vi "Query_source_settings_menu.vi"(8 "error in (no error)":errorcluster) -> (0 "error out":errorcluster, 1 "Cancelled?":bool, 3 "Output cluster":T1={"Integer Timestamp"=0, "Einzel Voltage"=0.0, "Needle Voltage"=0.0, "Frequency"=1.0, "Width (ms) : 0.1 "=0.05, "Desired Amplitude (V)"=0.0, "X Voltage"=0.0, "Y Voltage"=0.0, "Settings ID"="", "ID#"=0} {"Needle Voltage" min=0.0 max=10.0 step=0.01 format="%.2g"; "Y Voltage" min=0.0 max=9.0 step=0.01 format="%.2g"; "X Voltage" min=0.0 max=9.0 step=0.01 format="%.2g"; "Einzel Voltage" min=0.0 max=10.0 step=0.01 format="%.2g"; "Desired Amplitude (V)" min=0.0 max=10.0 step=0.01 format="%5.2f"; "Width (ms) : 0.1" min=0.05 max=5.0 step=0.01 format="%6.2f"; "Frequency" min=1.0 max=100.0 step=0.01 format="%.1f"})   [LabVIEW 2015]
doc: "Displays a standard dialog box that prompts users to enter information, such as a user name and password.\n--------------------\n\nThis Express VI is configured as follows:\n\nMessage to Display to the User:\nThe inputs are: \nNumber: Upper Timestamp Range\nNumber: Lower Timestamp Range\nNumber: Settings ID"
uses:
  Controls/dust_source_control.ctl
  Controls/Source_settings_select.ctl
  <vilib>/Utility/miscctls.llb/LVPointTypeDef.ctl
  <userlib>/_OpenG.lib/array/array.llb/Conditional Auto-Indexing Tunnel (I32)__ogtk.vi
  <vilib>/addons/database/_DB Variant To Data/Database Variant To Data.xnode
panel:
  out "Shooting Freq":dbl
  in  "Last Run Start":bool
  out "Source Control Array":T1[](array[typedef]) {"Needle Voltage" min=0.0 max=10.0 step=0.01 format="%.2g"; "Y Voltage" min=0.0 max=9.0 step=0.01 format="%.2g"; "X Voltage" min=0.0 max=9.0 step=0.01 format="%.2g"; "Einzel Voltage" min=0.0 max=10.0 step=0.01 format="%.2g"; "Desired Amplitude (V)" min=0.0 max=10.0 step=0.01 format="%5.2f"; "Width (ms) : 0.1" min=0.05 max=5.0 step=0.01 format="%6.2f"; "Frequency" min=1.0 max=100.0 step=0.01 format="%.1f"}
  in  "Settings Type":T2
  in  "Clear Filter":bool
  in  "Tag Filter":T3
  in  "Load Settings":bool caption="OK2"
  in  "Cancel":bool
  in  "Settings ID":i32(ring) items=["Automatic Update (DT: Iron-1E+1-3; HV: 2.2; Time: 7/23/2019 9:58:43 AM)"=11777, "Automatic Update (DT: Iron-1E+1-3; HV: 2.2; Time: 7/23/2019 10:03:43 AM)"=11778, "Automatic Update (DT: Iron-1E+1-3; HV: 2.2; Time: 7/23/2019 10:08:43 AM)"=11779, "Automatic Update (DT: Iron-1E+1-3; HV: 2.2; Time: 7/23/2019 10:18:43 AM)"=11780, "Automatic Update (DT: Iron-1E+1-3; HV: 2.2; Time: 7/23/2019 10:28:43 AM)"=11781, "Automatic Update (DT: Iron-1E+1-3; HV: 2.2; Time: 7/23/2019 10:48:43 AM)"=11782, "Automatic Update (DT: Iron-1E+1-3; HV: 2.2; Time: 7/23/2019 2:54:37 PM)"=11783, "Automatic Update (DT: Iron-1E+1-3; HV: 2.2; Time: 7/23/2019 3:03:12 PM)"=11784, "Automatic Update (DT: Iron-1E+1-3; HV: 2.2; Time: 7/23/2019 3:08:12 PM)"=11785, "Automatic Update (DT: Iron-1E+1-3; HV: 2.2; Time: 7/23/2019 3:13:12 PM)"=11786, "Automatic Update (DT: Iron-1E+1-3; HV: 2.2; Time: 7/23/2019 3:18:12 PM)"=11787, "Automatic Update (DT: Iron-1E+1-3; HV: 2.2; Time: 7/23/2019 3:23:13 PM)"=11788, "Automatic Update (DT: Iron-1E+1-3; HV: 2.2; Time: 7/23/2019 3:38:13 PM)"=11789, "Automatic Update (DT: Iron-1E+1-3; HV: 2.2; Time: 7/23/2019 3:53:13 PM)"=11790, "Automatic Update (DT: Iron-1E+1-3; HV: 2.2; Time: 7/23/2019 3:58:13 PM)"=11791, "Automatic Update (DT: Iron-1E+1-3; HV: 2.2; Time: 7/23/2019 4:03:13 PM)"=11792, "Automatic Update (DT: Iron-1E+1-3; HV: 2.2; Time: 7/23/2019 4:43:13 PM)"=11793, "Automatic Update (DT: Iron-1E+1-3; HV: 2.2; Time: 7/23/2019 4:58:13 PM)"=11794, "Automatic Update (DT: Iron-1E+1-3; HV: 2.2; Time: 7/24/2019 3:57:41 PM)"=11795, "Automatic Update (DT: Iron-1E+1-3; HV: 2.2; Time: 7/24/2019 4:02:41 PM)"=11796, "Automatic Update (DT: Iron-1E+1-3; HV: 2.2; Time: 7/24/2019 4:07:41 PM)"=11797, "Automatic Update (DT: Iron-1E+1-3; HV: 2.2; Time: 7/24/2019 4:12:41 PM)"=11798, "Automatic Update (DT: Iron-1E+1-3; HV: 2.2; Time: 7/24/2019 4:17:41 PM)"=11799, "Automatic Update (DT: Iron-1E+1-3; HV: 2.2; Time: 7/24/2019 4:22:41 PM)"=11800, "Automatic Update (DT: Iron-1E+1-3; HV: 2.2; Time: 7/24/2019 4:32:41 PM)"=11801, "Automatic Update (DT: Iron-1E+1-3; HV: 2.2; Time: 7/25/2019 8:48:47 AM)"=11802, "Automatic Update (DT: Iron-1E+1-3; HV: 2.2; Time: 7/25/2019 8:53:47 AM)"=11803, "Automatic Update (DT: Iron-1E+1-3; HV: 2.2; Time: 7/25/2019 9:13:47 AM)"=11804, "Automatic Update (DT: Iron-1E+1-3; HV: 2.2; Time: 7/25/2019 9:18:47 AM)"=11805, "Automatic Update (DT: Iron-1E+1-3; HV: 2.2; Time: 7/25/2019 9:23:47 AM)"=11806, "Automatic Update (DT: Iron-1E+1-3; HV: 2.2; Time: 7/25/2019 9:28:48 AM)"=11807, "Automatic Update (DT: Iron-1E+1-3; HV: 2.2; Time: 7/25/2019 9:38:48 AM)"=11808, "Automatic Update (DT: Iron-1E+1-3; HV: 2.2; Time: 7/25/2019 9:43:48 AM)"=11809, "Automatic Update (DT: Iron-1E+1-3; HV: 2.2; Time: 7/25/2019 9:48:48 AM)"=11810, "Automatic Update (DT: Iron-1E+1-3; HV: 2.2; Time: 7/25/2019 9:53:48 AM)"=11811, "Automatic Update (DT: Iron-1E+1-3; HV: 2.2; Time: 7/25/2019 9:58:48 AM)"=11812, "Automatic Update (DT: Iron-1E+1-3; HV: 2.2; Time: 7/25/2019 10:03:48 AM)"=11813, "Automatic Update (DT: Iron-1E+1-3; HV: 2.2; Time: 7/25/2019 10:13:48 AM)"=11814, "Automatic Update (DT: Iron-1E+1-3; HV: 2.2; Time: 7/25/2019 10:23:48 AM)"=11815, "Automatic Update (DT: Iron-1E+1-3; HV: 2.2; Time: 7/25/2019 10:28:48 AM)"=11816, "Automatic Update (DT: Iron-1E+1-3; HV: 2.2; Time: 7/25/2019 10:33:48 AM)"=11817, "Automatic Update (DT: Iron-1E+1-3; HV: 2.2; Time: 7/25/2019 10:43:49 AM)"=11818, "Automatic Update (DT: Iron-1E+1-3; HV: 2.2; Time: 7/25/2019 10:48:49 AM)"=11819, "Automatic Update (DT: Iron-1E+1-3; HV: 2.2; Time: 7/25/2019 10:53:49 AM)"=11820, "Automatic Update (DT: Iron-1E+1-3; HV: 2.2; Time: 7/25/2019 11:03:49 AM)"=11821, "Automatic Update (DT: Iron-1E+1-3; HV: 2.2; Time: 7/25/2019 11:08:49 AM)"=11822, "Automatic Update (DT: Iron-1E+1-3; HV: 2.2; Time: 8/8/2019 12:53:48 PM)"=11823, "Automatic Update (DT: Iron-1E+1-3; HV: 2.2; Time: 8/8/2019 1:08:48 PM)"=11824, "Automatic Update (DT: Iron-1E+1-3; HV: 2.2; Time: 8/21/2019 10:56:07 AM)"=11825, "Automatic Update (DT: Iron-1E+1-3; HV: 2.2; Time: 8/21/2019 11:01:07 AM)"=11826, "Automatic Update (DT: Iron-1E+1-3; HV: 2.2; Time: 8/21/2019 11:11:11 AM)"=11827, "Automatic Update (DT: Iron-1E+1-3; HV: 2.2; Time: 8/21/2019 11:16:11 AM)"=11828, "Automatic Update (DT: Iron-1E+1-3; HV: 2.2; Time: 8/21/2019 11:26:12 AM)"=11829, "Automatic Update (DT: Iron-1E+1-3; HV: 2.2; Time: 8/21/2019 11:31:12 AM)"=11830, "Automatic Update (DT: Iron-1E+1-3; HV: 2.2; Time: 8/21/2019 11:36:14 AM)"=11831, "Automatic Update (DT: Iron-1E+1-3; HV: 2.2; Time: 8/21/2019 11:41:22 AM)"=11832, "Automatic Update (DT: Iron-1E+1-3; HV: 2.2; Time: 8/21/2019 11:46:23 AM)"=11833, "Automatic Update (DT: Iron-1E+1-3; HV: 2.2; Time: 8/21/2019 12:47:37 PM)"=11834, "Automatic Update (DT: Iron-1E+1-3; HV: 2.2; Time: 8/21/2019 12:52:37 PM)"=11835, "Automatic Update (DT: Iron-1E+1-3; HV: 2.2; Time: 8/21/2019 12:57:37 PM)"=11836, "Automatic Update (DT: Iron-1E+1-3; HV: 2.2; Time: 8/21/2019 1:02:37 PM)"=11837, "Automatic Update (DT: Iron-1E+1-3; HV: 2.2; Time: 8/21/2019 1:07:37 PM)"=11838, "Automatic Update (DT: Iron-1E+1-3; HV: 2.2; Time: 8/21/2019 1:12:37 PM)"=11839, "Automatic Update (DT: Iron-1E+1-3; HV: 2.2; Time: 8/21/2019 1:17:38 PM)"=11840, "Automatic Update (DT: Iron-1E+1-3; HV: 2.2; Time: 8/21/2019 1:22:38 PM)"=11841, "Automatic Update (DT: Iron-1E+1-3; HV: 2.2; Time: 8/21/2019 1:32:38 PM)"=11842, "Automatic Update (DT: Iron-1E+1-3; HV: 2.2; Time: 8/21/2019 1:37:38 PM)"=11843, "Automatic Update (DT: Iron-1E+1-3; HV: 2.2; Time: 8/21/2019 1:42:38 PM)"=11844, "Automatic Update (DT: Iron-1E+1-3; HV: 2.2; Time: 8/21/2019 1:47:38 PM)"=11845, "Automatic Update (DT: Aluminum-4-2; HV: 2.2; Time: 9/3/2019 3:06:52 PM)"=11846, "Automatic Update (DT: Aluminum-4-2; HV: 2.2; Time: 9/3/2019 3:11:52 PM)"=11847, "Automatic Update (DT: Aluminum-4-2; HV: 2.2; Time: 9/3/2019 3:16:52 PM)"=11848, "Automatic Update (DT: Aluminum-4-2; HV: 2.2; Time: 9/9/2019 11:23:47 AM)"=11849, "Automatic Update (DT: Aluminum-4-2; HV: 2.2; Time: 9/9/2019 11:28:49 AM)"=11850, "Automatic Update (DT: Aluminum-4-2; HV: 2.2; Time: 9/9/2019 11:33:49 AM)"=11851, "Automatic Update (DT: Aluminum-4-2; HV: 2.2; Time: 9/9/2019 11:43:49 AM)"=11852, "Automatic Update (DT: Aluminum-4-2; HV: 2.2; Time: 9/9/2019 11:48:49 AM)"=11853, "Automatic Update (DT: Aluminum-4-2; HV: 2.2; Time: 9/9/2019 11:58:49 AM)"=11854, "Automatic Update (DT: Aluminum-4-2; HV: 2.2; Time: 9/9/2019 12:03:50 PM)"=11855, "Automatic Update (DT: Aluminum-4-2; HV: 2.2; Time: 9/9/2019 12:08:50 PM)"=11856, "Automatic Update (DT: Aluminum-4-2; HV: 2.2; Time: 9/9/2019 12:18:50 PM)"=11857, "Automatic Update (DT: Aluminum-4-2; HV: 2.2; Time: 9/9/2019 12:28:50 PM)"=11858, "Automatic Update (DT: Aluminum-4-2; HV: 2.2; Time: 9/9/2019 12:48:50 PM)"=11859, "Automatic Update (DT: Aluminum-4-2; HV: 2.2; Time: 9/9/2019 12:53:50 PM)"=11860, "Automatic Update (DT: Aluminum-4-2; HV: 2.2; Time: 9/9/2019 12:58:51 PM)"=11861, "Automatic Update (DT: Aluminum-4-2; HV: 2.2; Time: 9/9/2019 1:03:51 PM)"=11862, "Automatic Update (DT: Aluminum-4-2; HV: 2.2; Time: 9/9/2019 1:08:57 PM)"=11863, "Automatic Update (DT: Aluminum-4-2; HV: 2.2; Time: 9/9/2019 1:13:57 PM)"=11864, "Automatic Update (DT: Aluminum-4-2; HV: 2.2; Time: 9/9/2019 1:18:58 PM)"=11865, "Automatic Update (DT: Aluminum-4-2; HV: 2.2; Time: 9/9/2019 1:28:58 PM)"=11866, "Automatic Update (DT: Aluminum-4-2; HV: 2.2; Time: 9/9/2019 1:33:58 PM)"=11867, "Automatic Update (DT: Aluminum-4-2; HV: 2.2; Time: 9/13/2019 8:25:20 AM)"=11868, "Automatic Update (DT: Aluminum-4-2; HV: 2.2; Time: 9/13/2019 8:30:20 AM)"=11869, "Automatic Update (DT: Aluminum-4-2; HV: 2.2; Time: 9/13/2019 8:40:20 AM)"=11870, "Automatic Update (DT: Aluminum-4-2; HV: 2.2; Time: 9/13/2019 8:45:20 AM)"=11871, "Automatic Update (DT: Aluminum-4-2; HV: 2.2; Time: 9/13/2019 8:50:21 AM)"=11872, "Automatic Update (DT: Aluminum-4-2; HV: 2.2; Time: 9/13/2019 9:05:21 AM)"=11873, "Automatic Update (DT: Aluminum-4-2; HV: 2.2; Time: 9/13/2019 9:10:21 AM)"=11874, "Automatic Update (DT: Aluminum-4-2; HV: 2.2; Time: 9/13/2019 10:00:21 AM)"=11875, "Automatic Update (DT: Aluminum-4-2; HV: 2.2; Time: 9/13/2019 10:05:21 AM)"=11876, "Automatic Update (DT: Aluminum-4-2; HV: 2.2; Time: 9/13/2019 10:10:21 AM)"=11877, "Automatic Update (DT: Aluminum-4-2; HV: 2.2; Time: 9/13/2019 10:15:22 AM)"=11878, "Automatic Update (DT: Aluminum-4-2; HV: 2.2; Time: 9/13/2019 10:20:22 AM)"=11879, "Automatic Update (DT: Aluminum-4-2; HV: 2.2; Time: 9/13/2019 10:25:22 AM)"=11880, "Automatic Update (DT: Aluminum-4-2; HV: 2.2; Time: 9/13/2019 10:30:22 AM)"=11881, "Automatic Update (DT: Aluminum-4-2; HV: 2.2; Time: 9/13/2019 10:45:22 AM)"=11882, "Automatic Update (DT: Aluminum-4-2; HV: 2.2; Time: 9/13/2019 10:50:22 AM)"=11883, "Automatic Update (DT: Aluminum-4-2; HV: 2.2; Time: 9/13/2019 11:05:23 AM)"=11884, "Automatic Update (DT: Aluminum-4-2; HV: 2.2; Time: 9/13/2019 11:10:23 AM)"=11885, "Automatic Update (DT: Aluminum-4-2; HV: 2.2; Time: 9/13/2019 11:15:23 AM)"=11886, "Automatic Update (DT: Aluminum-4-2; HV: 2.2; Time: 9/13/2019 11:20:23 AM)"=11887, "Automatic Update (DT: Aluminum-4-2; HV: 2.2; Time: 9/13/2019 11:30:23 AM)"=11888, "Automatic Update (DT: Aluminum-4-2; HV: 2.2; Time: 9/13/2019 11:40:23 AM)"=11889, "Automatic Update (DT: Iron-1E+1-3; HV: 2.2; Time: 9/19/2019 11:43:00 AM)"=11890, "Automatic Update (DT: Iron-1E+1-3; HV: 2.2; Time: 9/19/2019 2:59:33 PM)"=11891, "Automatic Update (DT: Iron-1E+1-3; HV: 2.2; Time: 9/19/2019 3:14:33 PM)"=11892, "Automatic Update (DT: Iron-1E+1-3; HV: 2.2; Time: 9/19/2019 3:24:33 PM)"=11893, "Automatic Update (DT: Iron-1E+1-3; HV: 2.2; Time: 9/19/2019 3:29:34 PM)"=11894, "Automatic Update (DT: Iron-1E+1-3; HV: 2.2; Time: 9/19/2019 3:34:34 PM)"=11895, "Automatic Update (DT: Iron-1E+1-3; HV: 2.2; Time: 9/19/2019 3:39:34 PM)"=11896, "Automatic Update (DT: Iron-1E+1-3; HV: 2.2; Time: 9/19/2019 4:00:45 PM)"=11897, "Automatic Update (DT: Iron-1E+1-3; HV: 2.2; Time: 9/19/2019 4:10:45 PM)"=11898, "Automatic Update (DT: Iron-1E+1-3; HV: 2.2; Time: 9/19/2019 4:15:45 PM)"=11899, "Automatic Update (DT: Iron-1E+1-3; HV: 2.2; Time: 9/19/2019 4:50:45 PM)"=11900, "Automatic Update (DT: Iron-1E+1-3; HV: 2.2; Time: 9/19/2019 4:55:45 PM)"=11901, "Automatic Update (DT: Iron-1E+1-3; HV: 2.2; Time: 9/19/2019 5:00:45 PM)"=11902, "Automatic Update (DT: Iron-1E+1-3; HV: 2.2; Time: 9/19/2019 5:15:45 PM)"=11903, "Automatic Update (DT: Iron-1E+1-3; HV: 2.2; Time: 9/20/2019 3:19:41 PM)"=11904, "Automatic Update (DT: Iron-1E+1-3; HV: 2.2; Time: 9/20/2019 3:24:41 PM)"=11905, "Automatic Update (DT: Iron-1E+1-3; HV: 2.2; Time: 9/20/2019 3:29:41 PM)"=11906, "Automatic Update (DT: Iron-1E+1-3; HV: 2.2; Time: 9/20/2019 3:34:41 PM)"=11907, "Automatic Update (DT: Iron-1E+1-3; HV: 2.2; Time: 9/20/2019 3:39:42 PM)"=11908, "Automatic Update (DT: Iron-1E+1-3; HV: 2.2; Time: 9/20/2019 3:44:42 PM)"=11909, "Automatic Update (DT: Iron-1E+1-3; HV: 2.2; Time: 10/22/2019 10:59:09 AM)"=11910, "Automatic Update (DT: Iron-1E+1-3; HV: 2.2; Time: 10/22/2019 3:48:31 PM)"=11911, "Automatic Update (DT: Iron-1E+1-3; HV: 2.2; Time: 10/22/2019 3:53:31 PM)"=11912, "Automatic Update (DT: Iron-1E+1-3; HV: 2.2; Time: 10/30/2019 10:47:14 AM)"=11913, "Automatic Update (DT: Iron-1E+1-3; HV: 2.2; Time: 10/30/2019 10:52:14 AM)"=11914, "Automatic Update (DT: Iron-1E+1-3; HV: 2.2; Time: 10/30/2019 10:57:14 AM)"=11915, "Automatic Update (DT: Iron-1E+1-3; HV: 2.2; Time: 10/30/2019 11:02:14 AM)"=11916, "Automatic Update (DT: Iron-1E+1-3; HV: 2.2; Time: 10/30/2019 11:07:14 AM)"=11917, "Automatic Update (DT: Iron-1E+1-3; HV: 2.2; Time: 11/1/2019 4:11:29 PM)"=11918, "Automatic Update (DT: Iron-1E+1-3; HV: 2.2; Time: 11/1/2019 4:16:29 PM)"=11919, "Automatic Update (DT: Iron-1E+1-3; HV: 2.2; Time: 11/1/2019 4:21:29 PM)"=11920, "Automatic Update (DT: Iron-1E+1-3; HV: 2.2; Time: 11/4/2019 9:42:25 AM)"=11921, "Automatic Update (DT: Iron-1E+1-3; HV: 2.2; Time: 11/4/2019 9:47:25 AM)"=11922, "Automatic Update (DT: Iron-1E+1-3; HV: 2.2; Time: 11/4/2019 9:52:25 AM)"=11923, "Automatic Update (DT: Iron-1E+1-3; HV: 2.2; Time: 11/4/2019 9:57:25 AM)"=11924, "Automatic Update (DT: Iron-1E+1-3; HV: 2.2; Time: 11/4/2019 10:07:25 AM)"=11925, "Automatic Update (DT: Iron-1E+1-3; HV: 2.2; Time: 11/4/2019 10:32:25 AM)"=11926, "Automatic Update (DT: Iron-1E+1-3; HV: 2.2; Time: 11/4/2019 10:37:25 AM)"=11927, "Automatic Update (DT: Iron-1E+1-3; HV: 2.2; Time: 11/4/2019 10:42:25 AM)"=11928, "Automatic Update (DT: Iron-1E+1-3; HV: 2.2; Time: 11/5/2019 3:56:20 PM)"=11929, "Automatic Update (DT: Iron-1E+1-3; HV: 2.2; Time: 11/5/2019 4:01:20 PM)"=11930, "Automatic Update (DT: Iron-1E+1-3; HV: 2.2; Time: 11/5/2019 4:16:20 PM)"=11931, "Automatic Update (DT: Iron-1E+1-3; HV: 2.2; Time: 11/13/2019 5:58:37 PM)"=11932, "Automatic Update (DT: Iron-1E+1-3; HV: 2.2; Time: 11/13/2019 6:13:37 PM)"=11933, "Automatic Update (DT: Iron-1E+1-3; HV: 2.2; Time: 11/13/2019 6:43:38 PM)"=11934, "Automatic Update (DT: Iron-1E+1-3; HV: 2.2; Time: 11/18/2019 9:50:35 AM)"=11935, "Automatic Update (DT: Iron-1E+1-3; HV: 2.2; Time: 11/18/2019 10:00:35 AM)"=11936, "Automatic Update (DT: Iron-1E+1-3; HV: 2.2; Time: 11/18/2019 10:05:35 AM)"=11937, "Automatic Update (DT: Iron-1E+1-3; HV: 2.2; Time: 11/18/2019 10:30:35 AM)"=11938, "Automatic Update (DT: Iron-1E+1-3; HV: 2.2; Time: 11/18/2019 10:35:35 AM)"=11939, "Automatic Update (DT: Iron-1E+1-3; HV: 2.2; Time: 11/18/2019 10:50:36 AM)"=11940, "Automatic Update (DT: Iron-1E+1-3; HV: 2.2; Time: 11/18/2019 10:55:36 AM)"=11941, "Automatic Update (DT: Iron-1E+1-3; HV: 2.2; Time: 11/18/2019 11:05:36 AM)"=11942, "Automatic Update (DT: Iron-1E+1-3; HV: 2.2; Time: 11/18/2019 11:15:36 AM)"=11943, "Automatic Update (DT: Iron-1E+1-3; HV: 2.2; Time: 11/18/2019 11:20:36 AM)"=11944, "Automatic Update (DT: Iron-1E+1-3; HV: 2.2; Time: 11/18/2019 11:25:36 AM)"=11945, "Automatic Update (DT: Iron-1E+1-3; HV: 2.2; Time: 11/18/2019 11:40:37 AM)"=11946, "Automatic Update (DT: Iron-1E+1-3; HV: 2.2; Time: 11/18/2019 11:45:37 AM)"=11947, "Automatic Update (DT: Iron-1E+1-3; HV: 2.2; Time: 11/18/2019 11:50:37 AM)"=11948, "Automatic Update (DT: Iron-1E+1-3; HV: 2.2; Time: 11/18/2019 11:55:37 AM)"=11949, "Automatic Update (DT: Iron-1E+1-3; HV: 2.2; Time: 11/18/2019 12:10:37 PM)"=11950, "Automatic Update (DT: Iron-1E+1-3; HV: 2.2; Time: 11/18/2019 12:15:37 PM)"=11951, "Automatic Update (DT: Iron-1E+1-3; HV: 2.2; Time: 11/18/2019 12:25:37 PM)"=11952, "Automatic Update (DT: Iron-1E+1-3; HV: 2.2; Time: 11/18/2019 12:30:37 PM)"=11953, "Automatic Update (DT: Iron-1E+1-3; HV: 2.2; Time: 11/18/2019 12:40:38 PM)"=11954, "Automatic Update (DT: Iron-1E+1-3; HV: 2.2; Time: 11/18/2019 12:55:38 PM)"=11955, "Automatic Update (DT: Iron-1E+1-3; HV: 2.2; Time: 11/18/2019 1:00:38 PM)"=11956, "Automatic Update (DT: Iron-1E+1-3; HV: 2.2; Time: 11/18/2019 1:10:38 PM)"=11957, "Automatic Update (DT: Iron-1E+1-3; HV: 2.2; Time: 11/18/2019 1:30:38 PM)"=11958, "Automatic Update (DT: Iron-1E+1-3; HV: 2.2; Time: 11/18/2019 1:35:38 PM)"=11959, "Automatic Update (DT: Iron-1E+1-3; HV: 2.2; Time: 11/18/2019 1:45:38 PM)"=11960, "Automatic Update (DT: Iron-1E+1-3; HV: 2.2; Time: 11/19/2019 9:44:18 AM)"=11961, "Automatic Update (DT: Iron-1E+1-3; HV: 2.2; Time: 11/19/2019 9:49:18 AM)"=11962, "Automatic Update (DT: Iron-1E+1-3; HV: 2.2; Time: 11/19/2019 9:54:18 AM)"=11963, "Automatic Update (DT: Iron-1E+1-3; HV: 2.2; Time: 11/19/2019 10:04:18 AM)"=11964, "Automatic Update (DT: Iron-1E+1-3; HV: 2.2; Time: 11/19/2019 10:19:18 AM)"=11965, "Automatic Update (DT: Iron-1E+1-3; HV: 2.2; Time: 11/19/2019 10:29:18 AM)"=11966, "Automatic Update (DT: Iron-1E+1-3; HV: 2.2; Time: 11/19/2019 10:34:18 AM)"=11967, "Automatic Update (DT: Iron-1E+1-3; HV: 2.2; Time: 11/19/2019 10:39:18 AM)"=11968, "Automatic Update (DT: Iron-1E+1-3; HV: 2.2; Time: 11/19/2019 10:44:18 AM)"=11969, "Automatic Update (DT: Iron-1E+1-3; HV: 2.2; Time: 11/19/2019 11:09:18 AM)"=11970, "Automatic Update (DT: Iron-1E+1-3; HV: 2.2; Time: 11/19/2019 11:24:18 AM)"=11971, "Automatic Update (DT: Iron-1E+1-3; HV: 2.2; Time: 11/19/2019 11:29:19 AM)"=11972, "Automatic Update (DT: Iron-1E+1-3; HV: 2.2; Time: 11/19/2019 2:23:10 PM)"=11973, "Automatic Update (DT: Iron-1E+1-3; HV: 2.2; Time: 11/20/2019 11:46:10 AM)"=11974, "Automatic Update (DT: Iron-1E+1-3; HV: 2.2; Time: 11/20/2019 11:56:10 AM)"=11975, "Automatic Update (DT: Iron-1E+1-3; HV: 2.2; Time: 11/20/2019 12:26:10 PM)"=11976, "Automatic Update (DT: Iron-1E+1-3; HV: 2.2; Time: 11/20/2019 12:41:15 PM)"=11977, "Automatic Update (DT: Iron-1E+1-3; HV: 2.2; Time: 11/20/2019 2:44:09 PM)"=11978, "Automatic Update (DT: Iron-1E+1-3; HV: 2.2; Time: 11/20/2019 3:14:10 PM)"=11979, "Automatic Update (DT: Iron-1E+1-3; HV: 2.2; Time: 11/21/2019 10:04:15 AM)"=11980, "Automatic Update (DT: Iron-1E+1-3; HV: 2.2; Time: 11/21/2019 10:09:15 AM)"=11981, "Automatic Update (DT: Iron-1E+1-3; HV: 2.2; Time: 11/21/2019 10:19:15 AM)"=11982, "Automatic Update (DT: Iron-1E+1-3; HV: 2.2; Time: 11/21/2019 10:29:15 AM)"=11983, "Automatic Update (DT: Iron-1E+1-3; HV: 2.2; Time: 11/21/2019 10:34:15 AM)"=11984, "Automatic Update (DT: Iron-1E+1-3; HV: 2.2; Time: 11/21/2019 10:39:15 AM)"=11985, "Automatic Update (DT: Iron-1E+1-3; HV: 2.2; Time: 11/21/2019 10:44:15 AM)"=11986, "Automatic Update (DT: Iron-1E+1-3; HV: 2.2; Time: 11/21/2019 10:49:16 AM)"=11987, "Automatic Update (DT: Iron-1E+1-3; HV: 2.2; Time: 11/21/2019 10:54:16 AM)"=11988, "Automatic Update (DT: Iron-1E+1-3; HV: 2.2; Time: 11/21/2019 11:34:32 AM)"=11989, "Automatic Update (DT: Iron-1E+1-3; HV: 2.2; Time: 11/21/2019 11:39:32 AM)"=11990, "Automatic Update (DT: Iron-1E+1-3; HV: 2.2; Time: 11/21/2019 1:39:16 PM)"=11991, "Automatic Update (DT: Iron-1E+1-3; HV: 2.2; Time: 11/21/2019 1:49:16 PM)"=11992, "Automatic Update (DT: Iron-1E+1-3; HV: 2.2; Time: 11/21/2019 1:54:16 PM)"=11993, "Automatic Update (DT: Iron-1E+1-3; HV: 2.2; Time: 11/21/2019 1:59:16 PM)"=11994, "Automatic Update (DT: Iron-1E+1-3; HV: 2.2; Time: 11/21/2019 2:04:16 PM)"=11995, "Automatic Update (DT: Iron-1E+1-3; HV: 2.2; Time: 11/21/2019 2:09:16 PM)"=11996, "Automatic Update (DT: Iron-1E+1-3; HV: 2.2; Time: 11/21/2019 2:14:16 PM)"=11997, "Automatic Update (DT: Iron-1E+1-3; HV: 2.2; Time: 11/21/2019 2:19:16 PM)"=11998, "Automatic Update (DT: Iron-1E+1-3; HV: 2.2; Time: 11/21/2019 3:24:56 PM)"=11999, "Automatic Update (DT: Iron-1E+1-3; HV: 2.2; Time: 11/21/2019 3:39:56 PM)"=12000, "Automatic Update (DT: Iron-1E+1-3; HV: 2.2; Time: 11/26/2019 11:29:20 AM)"=12001, "Automatic Update (DT: Iron-1E+1-3; HV: 2.2; Time: 11/26/2019 11:39:20 AM)"=12002, "Automatic Update (DT: Iron-1E+1-3; HV: 2.2; Time: 11/26/2019 11:49:21 AM)"=12003, "Automatic Update (DT: Iron-1E+1-3; HV: 2.2; Time: 11/26/2019 11:54:21 AM)"=12004, "Automatic Update (DT: Iron-1E+1-3; HV: 2.2; Time: 11/26/2019 11:59:21 AM)"=12005, "Automatic Update (DT: Iron-1E+1-3; HV: 2.2; Time: 11/26/2019 12:04:21 PM)"=12006, "Automatic Update (DT: Iron-1E+1-3; HV: 2.2; Time: 11/26/2019 12:19:21 PM)"=12007, "Automatic Update (DT: Iron-1E+1-3; HV: 2.2; Time: 11/26/2019 12:49:21 PM)"=12008, "Automatic Update (DT: Iron-1E+1-3; HV: 2.2; Time: 11/27/2019 11:00:10 AM)"=12009, "Automatic Update (DT: Iron-1E+1-3; HV: 2.2; Time: 11/29/2019 4:06:14 PM)"=12010, "Automatic Update (DT: Iron-1E+1-3; HV: 2.2; Time: 11/29/2019 4:11:15 PM)"=12011, "Automatic Update (DT: Iron-1E+1-3; HV: 2.2; Time: 11/29/2019 4:16:15 PM)"=12012, "Automatic Update (DT: Iron-1E+1-3; HV: 2.2; Time: 11/29/2019 4:21:15 PM)"=12013, "Automatic Update (DT: Iron-1E+1-3; HV: 2.2; Time: 12/3/2019 10:05:08 AM)"=12014, "Automatic Update (DT: Iron-1E+1-3; HV: 2.2; Time: 12/3/2019 10:10:08 AM)"=12015, "Automatic Update (DT: Iron-1E+1-3; HV: 2.2; Time: 12/3/2019 10:15:08 AM)"=12016, "Automatic Update (DT: Iron-1E+1-3; HV: 2.2; Time: 12/3/2019 10:25:08 AM)"=12017, "Automatic Update (DT: Iron-1E+1-3; HV: 2.2; Time: 12/3/2019 10:35:08 AM)"=12018, "Automatic Update (DT: Iron-1E+1-3; HV: 2.2; Time: 12/3/2019 10:40:08 AM)"=12019, "Automatic Update (DT: Iron-1E+1-3; HV: 2.2; Time: 12/3/2019 10:55:08 AM)"=12020, "Automatic Update (DT: Iron-1E+1-3; HV: 2.2; Time: 12/3/2019 11:15:09 AM)"=12021, "Automatic Update (DT: Iron-1E+1-3; HV: 2.2; Time: 12/3/2019 11:20:09 AM)"=12022, "Automatic Update (DT: Iron-1E+1-3; HV: 2.2; Time: 12/3/2019 11:50:09 AM)"=12023, "Automatic Update (DT: Iron-1E+1-3; HV: 2.2; Time: 12/3/2019 12:00:09 PM)"=12024, "Automatic Update (DT: Iron-1E+1-3; HV: 2.2; Time: 12/3/2019 12:51:48 PM)"=12025, "Automatic Update (DT: Iron-1E+1-3; HV: 2.2; Time: 12/3/2019 12:56:48 PM)"=12026, "Automatic Update (DT: Iron-1E+1-3; HV: 2.2; Time: 12/3/2019 1:11:48 PM)"=12027, "Automatic Update (DT: Iron-1E+1-3; HV: 2.2; Time: 12/3/2019 1:16:48 PM)"=12028, "Automatic Update (DT: Iron-1E+1-3; HV: 2.2; Time: 12/3/2019 1:41:48 PM)"=12029, "Automatic Update (DT: Iron-1E+1-3; HV: 2.2; Time: 12/3/2019 3:11:49 PM)"=12030, "Automatic Update (DT: Iron-1E+1-3; HV: 2.2; Time: 12/4/2019 8:55:58 AM)"=12031, "Automatic Update (DT: Iron-1E+1-3; HV: 2.2; Time: 12/4/2019 9:00:59 AM)"=12032, "Automatic Update (DT: Iron-1E+1-3; HV: 2.2; Time: 12/4/2019 9:30:59 AM)"=12033, "Automatic Update (DT: Iron-1E+1-3; HV: 2.2; Time: 12/4/2019 10:05:59 AM)"=12034, "Automatic Update (DT: Iron-1E+1-3; HV: 2.2; Time: 12/4/2019 10:10:59 AM)"=12035, "Automatic Update (DT: Iron-1E+1-3; HV: 2.2; Time: 12/4/2019 11:10:59 AM)"=12036, "Automatic Update (DT: Iron-1E+1-3; HV: 2.2; Time: 12/4/2019 11:15:59 AM)"=12037, "Automatic Update (DT: Iron-1E+1-3; HV: 2.2; Time: 12/4/2019 11:50:59 AM)"=12038, "Automatic Update (DT: Iron-1E+1-3; HV: 2.2; Time: 12/4/2019 11:56:00 AM)"=12039, "Automatic Update (DT: Iron-1E+1-3; HV: 2.2; Time: 12/4/2019 12:01:00 PM)"=12040, "Automatic Update (DT: Iron-1E+1-3; HV: 2.2; Time: 12/4/2019 2:04:46 PM)"=12041, "Automatic Update (DT: Iron-1E+1-3; HV: 2.2; Time: 12/4/2019 2:54:46 PM)"=12042, "Automatic Update (DT: Iron-1E+1-3; HV: 2.2; Time: 12/4/2019 3:09:47 PM)"=12043, "Automatic Update (DT: Iron-1E+1-3; HV: 2.2; Time: 12/4/2019 3:14:47 PM)"=12044, "Automatic Update (DT: Iron-1E+1-3; HV: 2.2; Time: 12/4/2019 3:34:47 PM)"=12045, "Automatic Update (DT: Iron-1E+1-3; HV: 2.2; Time: 12/4/2019 3:39:47 PM)"=12046, "Automatic Update (DT: Iron-1E+1-3; HV: 2.2; Time: 12/4/2019 3:44:47 PM)"=12047, "Automatic Update (DT: Iron-1E+1-3; HV: 2.2; Time: 12/5/2019 9:41:35 AM)"=12048, "Automatic Update (DT: Iron-1E+1-3; HV: 2.2; Time: 12/5/2019 10:06:35 AM)"=12049, "Automatic Update (DT: Iron-1E+1-3; HV: 2.2; Time: 12/5/2019 10:31:35 AM)"=12050, "Automatic Update (DT: Iron-1E+1-3; HV: 2.2; Time: 12/5/2019 10:36:36 AM)"=12051, "Automatic Update (DT: Iron-1E+1-3; HV: 2.2; Time: 12/5/2019 11:01:36 AM)"=12052, "Automatic Update (DT: Iron-1E+1-3; HV: 2.2; Time: 12/5/2019 11:16:36 AM)"=12053, "Automatic Update (DT: Iron-1E+1-3; HV: 2.2; Time: 12/5/2019 11:21:36 AM)"=12054, "Automatic Update (DT: Iron-1E+1-3; HV: 2.2; Time: 12/5/2019 1:37:40 PM)"=12055, "Automatic Update (DT: Iron-1E+1-3; HV: 2.2; Time: 12/5/2019 2:57:41 PM)"=12056, "Automatic Update (DT: Iron-1E+1-3; HV: 2.2; Time: 12/5/2019 3:37:41 PM)"=12057, "Automatic Update (DT: Iron-1E+1-3; HV: 2.2; Time: 12/5/2019 3:47:41 PM)"=12058, "Automatic Update (DT: Iron-1E+1-3; HV: 2.2; Time: 12/5/2019 4:07:41 PM)"=12059, "Automatic Update (DT: Iron-1E+1-3; HV: 2.2; Time: 12/5/2019 4:17:41 PM)"=12060, "Automatic Update (DT: Iron-1E+1-3; HV: 2.2; Time: 12/6/2019 9:08:40 AM)"=12061, "Automatic Update (DT: Iron-1E+1-3; HV: 2.2; Time: 12/6/2019 9:48:40 AM)"=12062, "Automatic Update (DT: Iron-1E+1-3; HV: 2.2; Time: 12/6/2019 10:03:40 AM)"=12063, "Automatic Update (DT: Olivine-3-1; HV: 2.2; Time: 12/9/2019 2:38:17 PM)"=12064, "Automatic Update (DT: Olivine-3-1; HV: 2.2; Time: 12/9/2019 2:43:17 PM)"=12065, "Automatic Update (DT: Olivine-3-1; HV: 2.2; Time: 12/9/2019 2:48:17 PM)"=12066, "Automatic Update (DT: Olivine-3-1; HV: 2.2; Time: 12/9/2019 2:53:17 PM)"=12067, "Automatic Update (DT: Olivine-3-1; HV: 2.2; Time: 12/9/2019 2:58:17 PM)"=12068, "Automatic Update (DT: Olivine-3-1; HV: 2.2; Time: 12/9/2019 3:13:13 PM)"=12069, "Automatic Update (DT: Olivine-3-1; HV: 2.2; Time: 12/9/2019 3:18:13 PM)"=12070, "Automatic Update (DT: Olivine-3-1; HV: 2.2; Time: 12/9/2019 3:23:13 PM)"=12071, "Automatic Update (DT: Olivine-3-1; HV: 2.2; Time: 12/9/2019 3:28:13 PM)"=12072, "Automatic Update (DT: Olivine-3-1; HV: 2.2; Time: 12/9/2019 3:33:14 PM)"=12073, "Automatic Update (DT: Olivine-3-1; HV: 2.2; Time: 12/9/2019 3:38:14 PM)"=12074, "Automatic Update (DT: Olivine-3-1; HV: 2.2; Time: 12/9/2019 3:43:14 PM)"=12075, "Automatic Update (DT: Olivine-3-1; HV: 2.2; Time: 12/9/2019 3:48:14 PM)"=12076, "Automatic Update (DT: Olivine-3-1; HV: 2.2; Time: 12/9/2019 3:53:14 PM)"=12077, "Automatic Update (DT: Olivine-3-1; HV: 0.8; Time: 12/13/2019 2:43:54 PM)"=12078, "Automatic Update (DT: Olivine-3-1; HV: 2.2; Time: 12/14/2019 10:23:31 AM)"=12079, "Automatic Update (DT: Olivine-3-1; HV: 2.2; Time: 12/14/2019 10:28:31 AM)"=12080, "Automatic Update (DT: Olivine-3-1; HV: 2.2; Time: 12/14/2019 10:33:31 AM)"=12081, "Automatic Update (DT: Olivine-3-1; HV: 2.2; Time: 12/14/2019 10:38:31 AM)"=12082, "Automatic Update (DT: Olivine-3-1; HV: 2.2; Time: 12/14/2019 10:43:32 AM)"=12083, "Automatic Update (DT: Olivine-3-1; HV: 2.2; Time: 12/14/2019 10:48:32 AM)"=12084, "Automatic Update (DT: Olivine-3-1; HV: 2.2; Time: 12/14/2019 10:53:36 AM)"=12085, "Automatic Update (DT: Olivine-3-1; HV: 2.2; Time: 12/17/2019 9:16:58 AM)"=12086, "Automatic Update (DT: Olivine-3-1; HV: 2.2; Time: 12/17/2019 9:21:58 AM)"=12087, "Automatic Update (DT: Olivine-3-1; HV: 2.2; Time: 12/17/2019 9:31:58 AM)"=12088, "Automatic Update (DT: Olivine-3-1; HV: 2.2; Time: 12/17/2019 9:41:58 AM)"=12089, "Automatic Update (DT: Olivine-3-1; HV: 2.2; Time: 12/17/2019 9:51:58 AM)"=12090, "Automatic Update (DT: Olivine-3-1; HV: 2.2; Time: 12/17/2019 10:01:58 AM)"=12091, "Automatic Update (DT: Olivine-3-1; HV: 2.2; Time: 12/17/2019 10:06:58 AM)"=12092, "Automatic Update (DT: Olivine-3-1; HV: 2.2; Time: 12/17/2019 10:21:58 AM)"=12093, "Automatic Update (DT: Olivine-3-1; HV: 2.2; Time: 12/17/2019 10:26:59 AM)"=12094, "Automatic Update (DT: Olivine-3-1; HV: 2.2; Time: 12/17/2019 10:31:59 AM)"=12095, "Automatic Update (DT: Olivine-3-1; HV: 2.2; Time: 12/17/2019 10:36:59 AM)"=12096, "Automatic Update (DT: Olivine-3-1; HV: 2.2; Time: 12/17/2019 10:56:59 AM)"=12097, "Automatic Update (DT: Olivine-3-1; HV: 2.2; Time: 12/17/2019 11:01:59 AM)"=12098, "Automatic Update (DT: Olivine-3-1; HV: 2.2; Time: 12/17/2019 11:11:59 AM)"=12099, "Automatic Update (DT: Olivine-3-1; HV: 2.2; Time: 12/17/2019 11:16:59 AM)"=12100, "Automatic Update (DT: Olivine-3-1; HV: 2.2; Time: 12/17/2019 11:21:59 AM)"=12101, "Automatic Update (DT: Olivine-3-1; HV: 2.2; Time: 12/17/2019 11:32:00 AM)"=12102, "Automatic Update (DT: Olivine-3-1; HV: 2.2; Time: 12/17/2019 11:37:00 AM)"=12103, "Automatic Update (DT: Olivine-3-1; HV: 2.2; Time: 12/17/2019 12:02:00 PM)"=12104, "Automatic Update (DT: Olivine-3-1; HV: 2.2; Time: 12/17/2019 12:22:00 PM)"=12105, "Automatic Update (DT: Olivine-3-1; HV: 2.2; Time: 12/17/2019 12:37:00 PM)"=12106, "Automatic Update (DT: Olivine-3-1; HV: 2.2; Time: 12/17/2019 12:42:00 PM)"=12107, "Automatic Update (DT: Olivine-3-1; HV: 2.2; Time: 12/17/2019 12:47:00 PM)"=12108, "Automatic Update (DT: Olivine-3-1; HV: 2.2; Time: 12/17/2019 12:52:00 PM)"=12109, "Automatic Update (DT: Olivine-3-1; HV: 2.2; Time: 12/17/2019 1:02:00 PM)"=12110, "Automatic Update (DT: Olivine-3-1; HV: 2.2; Time: 12/17/2019 1:07:00 PM)"=12111, "Automatic Update (DT: Olivine-3-1; HV: 2.2; Time: 12/17/2019 1:12:00 PM)"=12112, "Automatic Update (DT: Olivine-3-1; HV: 2.2; Time: 12/17/2019 1:17:01 PM)"=12113, "Automatic Update (DT: Olivine-3-1; HV: 2.2; Time: 12/17/2019 1:22:01 PM)"=12114, "Automatic Update (DT: Olivine-3-1; HV: 2.2; Time: 12/17/2019 1:27:01 PM)"=12115, "Automatic Update (DT: Olivine-3-1; HV: 2.2; Time: 12/17/2019 1:32:01 PM)"=12116, "Automatic Update (DT: Olivine-3-1; HV: 2.2; Time: 12/17/2019 1:37:01 PM)"=12117, "Automatic Update (DT: Olivine-3-1; HV: 2.2; Time: 12/17/2019 1:42:01 PM)"=12118, "Automatic Update (DT: Olivine-3-1; HV: 2.2; Time: 12/17/2019 1:52:01 PM)"=12119, "Automatic Update (DT: Olivine-3-1; HV: 2.2; Time: 12/17/2019 1:57:01 PM)"=12120, "Automatic Update (DT: Olivine-3-1; HV: 2.2; Time: 12/17/2019 2:02:01 PM)"=12121, "Automatic Update (DT: Olivine-3-1; HV: 2.2; Time: 12/17/2019 2:07:01 PM)"=12122, "Automatic Update (DT: Olivine-3-1; HV: 2.2; Time: 12/17/2019 2:12:01 PM)"=12123, "Automatic Update (DT: Olivine-3-1; HV: 2.2; Time: 12/17/2019 2:17:02 PM)"=12124, "Automatic Update (DT: Olivine-3-1; HV: 2.2; Time: 12/17/2019 2:32:02 PM)"=12125, "Automatic Update (DT: Olivine-3-1; HV: 2.2; Time: 12/17/2019 2:42:02 PM)"=12126, "Automatic Update (DT: Olivine-3-1; HV: 2.2; Time: 12/17/2019 3:22:02 PM)"=12127, "Automatic Update (DT: Olivine-3-1; HV: 2.2; Time: 12/17/2019 3:27:02 PM)"=12128, "Automatic Update (DT: Olivine-3-1; HV: 2.2; Time: 12/17/2019 3:42:02 PM)"=12129, "Automatic Update (DT: Olivine-3-1; HV: 2.2; Time: 12/17/2019 4:07:02 PM)"=12130, "Automatic Update (DT: Olivine-3-1; HV: 2.2; Time: 12/17/2019 4:12:02 PM)"=12131, "Automatic Update (DT: Olivine-3-1; HV: 2.2; Time: 12/17/2019 4:17:02 PM)"=12132, "Automatic Update (DT: Olivine-3-1; HV: 2.2; Time: 12/17/2019 4:27:02 PM)"=12133, "Automatic Update (DT: Olivine-3-1; HV: 2.2; Time: 12/17/2019 4:32:03 PM)"=12134, "Automatic Update (DT: Olivine-3-1; HV: 2.2; Time: 12/17/2019 4:37:03 PM)"=12135, "Automatic Update (DT: Olivine-3-1; HV: 2.2; Time: 12/17/2019 4:52:03 PM)"=12136, "Automatic Update (DT: Olivine-3-1; HV: 2.2; Time: 12/17/2019 4:57:03 PM)"=12137, "Automatic Update (DT: Olivine-3-1; HV: 2.2; Time: 12/17/2019 5:07:03 PM)"=12138, "Automatic Update (DT: Olivine-3-1; HV: 2.2; Time: 12/17/2019 5:12:03 PM)"=12139, "Automatic Update (DT: Olivine-3-1; HV: 2.2; Time: 12/17/2019 5:22:03 PM)"=12140, "Automatic Update (DT: Olivine-3-1; HV: 2.2; Time: 12/17/2019 5:27:04 PM)"=12141, "Automatic Update (DT: Olivine-3-1; HV: 2.2; Time: 12/17/2019 5:42:04 PM)"=12142, "Automatic Update (DT: Olivine-3-1; HV: 2.2; Time: 12/17/2019 5:57:04 PM)"=12143, "Automatic Update (DT: Olivine-3-1; HV: 2.2; Time: 12/17/2019 6:02:04 PM)"=12144, "Automatic Update (DT: Olivine-3-1; HV: 2.2; Time: 12/17/2019 6:37:04 PM)"=12145, "Automatic Update (DT: Olivine-3-1; HV: 2.2; Time: 12/17/2019 7:02:04 PM)"=12146, "Automatic Update (DT: Olivine-3-1; HV: 2.2; Time: 12/17/2019 7:07:04 PM)"=12147, "Automatic Update (DT: Olivine-3-1; HV: 2.2; Time: 12/17/2019 7:12:04 PM)"=12148, "Automatic Update (DT: Olivine-3-1; HV: 2.2; Time: 12/17/2019 7:22:04 PM)"=12149, "Automatic Update (DT: Olivine-3-1; HV: 2.2; Time: 12/17/2019 7:47:05 PM)"=12150, "Automatic Update (DT: Olivine-3-1; HV: 2.2; Time: 12/17/2019 7:52:05 PM)"=12151, "Automatic Update (DT: Olivine-3-1; HV: 2.2; Time: 12/17/2019 8:07:05 PM)"=12152, "Automatic Update (DT: Olivine-3-1; HV: 2.2; Time: 12/17/2019 8:12:05 PM)"=12153, "Automatic Update (DT: Olivine-3-1; HV: 2.2; Time: 12/17/2019 8:22:05 PM)"=12154, "Automatic Update (DT: Olivine-3-1; HV: 2.2; Time: 12/17/2019 8:27:05 PM)"=12155, "Automatic Update (DT: Olivine-3-1; HV: 2.2; Time: 12/17/2019 8:57:05 PM)"=12156, "Automatic Update (DT: Olivine-3-1; HV: 2.2; Time: 12/17/2019 9:17:05 PM)"=12157, "Automatic Update (DT: Olivine-3-1; HV: 2.2; Time: 12/17/2019 9:27:05 PM)"=12158, "Automatic Update (DT: Olivine-3-1; HV: 2.2; Time: 12/17/2019 9:32:06 PM)"=12159, "Automatic Update (DT: Olivine-3-1; HV: 2.2; Time: 12/17/2019 9:37:06 PM)"=12160, "Automatic Update (DT: Olivine-3-1; HV: 2.2; Time: 12/17/2019 9:42:06 PM)"=12161, "Automatic Update (DT: Olivine-3-1; HV: 2.2; Time: 12/17/2019 9:47:06 PM)"=12162, "Automatic Update (DT: Olivine-3-1; HV: 2.2; Time: 12/17/2019 9:52:06 PM)"=12163, "Automatic Update (DT: Olivine-3-1; HV: 2.2; Time: 12/17/2019 9:57:06 PM)"=12164, "Automatic Update (DT: Olivine-3-1; HV: 2.2; Time: 12/17/2019 10:02:06 PM)"=12165, "Automatic Update (DT: Olivine-3-1; HV: 2.2; Time: 12/17/2019 10:12:06 PM)"=12166, "Automatic Update (DT: Olivine-3-1; HV: 2.2; Time: 12/17/2019 10:17:06 PM)"=12167, "Automatic Update (DT: Olivine-3-1; HV: 2.2; Time: 12/17/2019 10:27:07 PM)"=12168, "Automatic Update (DT: Olivine-3-1; HV: 2.2; Time: 12/17/2019 10:32:07 PM)"=12169, "Automatic Update (DT: Olivine-3-1; HV: 2.2; Time: 12/17/2019 10:37:07 PM)"=12170, "Automatic Update (DT: Olivine-3-1; HV: 2.2; Time: 12/17/2019 10:42:07 PM)"=12171, "Automatic Update (DT: Olivine-3-1; HV: 2.2; Time: 12/17/2019 10:47:07 PM)"=12172, "Automatic Update (DT: Olivine-3-1; HV: 2.2; Time: 12/17/2019 10:52:07 PM)"=12173, "Automatic Update (DT: Olivine-3-1; HV: 2.2; Time: 12/17/2019 10:57:07 PM)"=12174, "Automatic Update (DT: Olivine-3-1; HV: 2.2; Time: 12/17/2019 11:02:07 PM)"=12175, "Automatic Update (DT: Olivine-3-1; HV: 2.2; Time: 12/17/2019 11:07:07 PM)"=12176, "Automatic Update (DT: Olivine-3-1; HV: 2.2; Time: 12/17/2019 11:17:08 PM)"=12177, "Automatic Update (DT: Olivine-3-1; HV: 2.2; Time: 12/17/2019 11:22:08 PM)"=12178, "Automatic Update (DT: Olivine-3-1; HV: 2.2; Time: 12/17/2019 11:27:08 PM)"=12179, "Automatic Update (DT: Olivine-3-1; HV: 2.2; Time: 12/17/2019 11:32:08 PM)"=12180, "Automatic Update (DT: Olivine-3-1; HV: 2.2; Time: 12/17/2019 11:37:08 PM)"=12181, "Automatic Update (DT: Olivine-3-1; HV: 2.2; Time: 12/17/2019 11:42:08 PM)"=12182, "Automatic Update (DT: Olivine-3-1; HV: 2.2; Time: 12/17/2019 11:47:09 PM)"=12183, "Automatic Update (DT: Olivine-3-1; HV: 2.2; Time: 12/17/2019 11:52:09 PM)"=12184, "Automatic Update (DT: Olivine-3-1; HV: 2.2; Time: 12/17/2019 11:57:09 PM)"=12185, "Automatic Update (DT: Olivine-3-1; HV: 2.2; Time: 12/18/2019 12:07:09 AM)"=12186, "Automatic Update (DT: Olivine-3-1; HV: 2.2; Time: 12/18/2019 12:12:09 AM)"=12187, "Automatic Update (DT: Olivine-3-1; HV: 2.2; Time: 12/18/2019 12:17:09 AM)"=12188, "Automatic Update (DT: Olivine-3-1; HV: 2.2; Time: 12/18/2019 12:22:09 AM)"=12189, "Automatic Update (DT: Olivine-3-1; HV: 2.2; Time: 12/18/2019 12:27:09 AM)"=12190, "Automatic Update (DT: Olivine-3-1; HV: 2.2; Time: 12/18/2019 12:32:10 AM)"=12191, "Automatic Update (DT: Olivine-3-1; HV: 2.2; Time: 12/18/2019 12:37:10 AM)"=12192, "Automatic Update (DT: Olivine-3-1; HV: 2.2; Time: 12/18/2019 12:42:10 AM)"=12193, "Automatic Update (DT: Olivine-3-1; HV: 2.2; Time: 12/18/2019 12:47:10 AM)"=12194, "Automatic Update (DT: Olivine-3-1; HV: 2.2; Time: 12/18/2019 12:52:10 AM)"=12195, "Automatic Update (DT: Olivine-3-1; HV: 2.2; Time: 12/18/2019 12:57:10 AM)"=12196, "Automatic Update (DT: Olivine-3-1; HV: 2.2; Time: 12/18/2019 1:02:11 AM)"=12197, "Automatic Update (DT: Olivine-3-1; HV: 2.2; Time: 12/18/2019 1:12:24 AM)"=12198, "Automatic Update (DT: Olivine-3-1; HV: 2.2; Time: 12/18/2019 7:24:46 AM)"=12199, "Automatic Update (DT: Olivine-3-1; HV: 2.2; Time: 12/18/2019 7:29:46 AM)"=12200, "Automatic Update (DT: Olivine-3-1; HV: 2.2; Time: 12/18/2019 7:34:46 AM)"=12201, "Automatic Update (DT: Olivine-3-1; HV: 2.2; Time: 12/18/2019 7:39:46 AM)"=12202, "Automatic Update (DT: Olivine-3-1; HV: 2.2; Time: 12/18/2019 7:44:46 AM)"=12203, "Automatic Update (DT: Olivine-3-1; HV: 2.2; Time: 12/18/2019 8:09:47 AM)"=12204, "Automatic Update (DT: Olivine-3-1; HV: 2.2; Time: 12/18/2019 8:19:47 AM)"=12205, "Automatic Update (DT: Olivine-3-1; HV: 2.2; Time: 12/18/2019 8:24:47 AM)"=12206, "Automatic Update (DT: Olivine-3-1; HV: 2.2; Time: 12/18/2019 8:29:47 AM)"=12207, "Automatic Update (DT: Olivine-3-1; HV: 2.2; Time: 12/18/2019 8:34:47 AM)"=12208, "Automatic Update (DT: Olivine-3-1; HV: 2.2; Time: 12/18/2019 8:39:47 AM)"=12209, "Automatic Update (DT: Olivine-3-1; HV: 2.2; Time: 12/18/2019 8:44:47 AM)"=12210, "Automatic Update (DT: Olivine-3-1; HV: 2.2; Time: 12/18/2019 8:49:47 AM)"=12211, "Automatic Update (DT: Olivine-3-1; HV: 2.2; Time: 12/18/2019 8:54:47 AM)"=12212, "Automatic Update (DT: Olivine-3-1; HV: 2.2; Time: 12/18/2019 8:59:47 AM)"=12213, "Automatic Update (DT: Olivine-3-1; HV: 2.2; Time: 12/18/2019 9:04:47 AM)"=12214, "Automatic Update (DT: Olivine-3-1; HV: 2.2; Time: 12/18/2019 9:09:47 AM)"=12215, "Automatic Update (DT: Olivine-3-1; HV: 2.2; Time: 12/18/2019 9:14:48 AM)"=12216, "Automatic Update (DT: Olivine-3-1; HV: 2.2; Time: 12/18/2019 9:19:48 AM)"=12217, "Automatic Update (DT: Olivine-3-1; HV: 2.2; Time: 12/18/2019 9:24:48 AM)"=12218, "Automatic Update (DT: Olivine-3-1; HV: 2.2; Time: 12/18/2019 9:29:48 AM)"=12219, "Automatic Update (DT: Olivine-3-1; HV: 2.2; Time: 12/18/2019 9:34:48 AM)"=12220, "Automatic Update (DT: Olivine-3-1; HV: 2.2; Time: 12/18/2019 9:39:48 AM)"=12221, "Automatic Update (DT: Olivine-3-1; HV: 2.2; Time: 12/18/2019 9:44:48 AM)"=12222, "Automatic Update (DT: Olivine-3-1; HV: 2.2; Time: 1/3/2020 3:35:09 AM)"=12223, "Automatic Update (DT: Olivine-3-1; HV: 2.2; Time: 1/3/2020 3:35:10 AM)"=12224, "Automatic Update (DT: Olivine-3-1; HV: 2.2; Time: 1/3/2020 3:35:12 AM)"=12225, "Automatic Update (DT: Olivine-3-1; HV: 2.2; Time: 1/3/2020 3:35:14 AM)"=12226, "Automatic Update (DT: Olivine-3-1; HV: 2.2; Time: 1/3/2020 3:35:15 AM)"=12227, "Automatic Update (DT: Olivine-3-1; HV: 2.2; Time: 1/3/2020 3:35:16 AM)"=12228, "Automatic Update (DT: Olivine-3-1; HV: 2.2; Time: 1/3/2020 3:35:17 AM)"=12229, "Automatic Update (DT: Olivine-3-1; HV: 2.2; Time: 1/3/2020 3:35:18 AM)"=12230, "Automatic Update (DT: Olivine-3-1; HV: 2.2; Time: 1/3/2020 3:35:19 AM)"=12231, "Automatic Update (DT: Olivine-3-1; HV: 2.2; Time: 1/3/2020 3:35:20 AM)"=12232, "Automatic Update (DT: Olivine-3-1; HV: 2.2; Time: 1/3/2020 3:35:21 AM)"=12233, "Automatic Update (DT: Olivine-3-1; HV: 2.2; Time: 1/3/2020 3:35:22 AM)"=12234, "Automatic Update (DT: Olivine-3-1; HV: 2.2; Time: 1/3/2020 3:35:23 AM)"=12235, "Automatic Update (DT: Olivine-3-1; HV: 2.2; Time: 1/3/2020 3:35:24 AM)"=12236, "Automatic Update (DT: Olivine-3-1; HV: 2.2; Time: 1/3/2020 3:35:25 AM)"=12237, "Automatic Update (DT: Olivine-3-1; HV: 2.2; Time: 1/3/2020 3:35:26 AM)"=12238, "Automatic Update (DT: Olivine-3-1; HV: 2.2; Time: 1/3/2020 3:35:28 AM)"=12239, "Automatic Update (DT: Olivine-3-1; HV: 2.2; Time: 1/3/2020 3:35:29 AM)"=12240, "Automatic Update (DT: Olivine-3-1; HV: 2.2; Time: 1/3/2020 3:35:30 AM)"=12241, "Automatic Update (DT: Olivine-3-1; HV: 2.2; Time: 1/3/2020 3:35:31 AM)"=12242, "Automatic Update (DT: Olivine-3-1; HV: 2.2; Time: 1/3/2020 3:35:32 AM)"=12243, "Automatic Update (DT: Olivine-3-1; HV: 2.2; Time: 1/3/2020 3:35:33 AM)"=12244, "Automatic Update (DT: Olivine-3-1; HV: 2.2; Time: 1/3/2020 3:35:34 AM)"=12245, "Automatic Update (DT: Olivine-3-1; HV: 2.2; Time: 1/3/2020 3:35:35 AM)"=12246, "Automatic Update (DT: Olivine-3-1; HV: 2.2; Time: 1/3/2020 3:35:36 AM)"=12247, "Automatic Update (DT: Olivine-3-1; HV: 2.2; Time: 1/3/2020 3:35:37 AM)"=12248, "Automatic Update (DT: Olivine-3-1; HV: 2.2; Time: 1/3/2020 3:35:38 AM)"=12249, "Automatic Update (DT: Olivine-3-1; HV: 2.2; Time: 1/3/2020 3:35:39 AM)"=12250, "Automatic Update (DT: Olivine-3-1; HV: 2.2; Time: 1/3/2020 3:35:40 AM)"=12251, "Automatic Update (DT: Olivine-3-1; HV: 2.2; Time: 1/3/2020 3:35:41 AM)"=12252, "Automatic Update (DT: Olivine-3-1; HV: 2.2; Time: 1/3/2020 3:35:42 AM)"=12253, "Automatic Update (DT: Olivine-3-1; HV: 2.2; Time: 1/3/2020 3:35:43 AM)"=12254, "Automatic Update (DT: Olivine-3-1; HV: 2.2; Time: 1/3/2020 3:35:44 AM)"=12255, "Automatic Update (DT: Olivine-3-1; HV: 2.2; Time: 1/3/2020 3:35:45 AM)"=12256, "Automatic Update (DT: Olivine-3-1; HV: 2.2; Time: 1/3/2020 3:35:46 AM)"=12257, "Automatic Update (DT: Olivine-3-1; HV: 2.2; Time: 1/3/2020 3:35:47 AM)"=12258, "Automatic Update (DT: Olivine-3-1; HV: 2.2; Time: 1/3/2020 3:35:48 AM)"=12259, "Automatic Update (DT: Olivine-3-1; HV: 2.2; Time: 1/3/2020 3:35:50 AM)"=12260, "Automatic Update (DT: Olivine-3-1; HV: 2.2; Time: 1/3/2020 3:35:51 AM)"=12261, "Automatic Update (DT: Olivine-3-1; HV: 2.2; Time: 1/3/2020 3:35:52 AM)"=12262, "Automatic Update (DT: Olivine-3-1; HV: 2.2; Time: 1/3/2020 3:35:54 AM)"=12263, "Automatic Update (DT: Olivine-3-1; HV: 2.2; Time: 1/3/2020 3:35:55 AM)"=12264, "Automatic Update (DT: Olivine-3-1; HV: 2.2; Time: 1/3/2020 3:35:56 AM)"=12265, "Automatic Update (DT: Olivine-3-1; HV: 2.2; Time: 1/3/2020 3:35:57 AM)"=12266, "Automatic Update (DT: Olivine-3-1; HV: 2.2; Time: 1/3/2020 3:35:58 AM)"=12267, "Automatic Update (DT: Olivine-3-1; HV: 2.2; Time: 1/3/2020 3:35:59 AM)"=12268, "Automatic Update (DT: Olivine-3-1; HV: 2.2; Time: 1/3/2020 3:36:00 AM)"=12269, "Automatic Update (DT: Olivine-3-1; HV: 2.2; Time: 1/3/2020 3:36:01 AM)"=12270, "Automatic Update (DT: Olivine-3-1; HV: 2.2; Time: 1/3/2020 3:36:02 AM)"=12271, "Automatic Update (DT: Olivine-3-1; HV: 2.2; Time: 1/3/2020 3:36:03 AM)"=12272, "Automatic Update (DT: Olivine-3-1; HV: 2.2; Time: 1/3/2020 3:36:04 AM)"=12273, "Automatic Update (DT: Olivine-3-1; HV: 2.2; Time: 1/3/2020 3:36:05 AM)"=12274, "Automatic Update (DT: Olivine-3-1; HV: 2.2; Time: 1/3/2020 3:36:06 AM)"=12275, "Automatic Update (DT: Olivine-3-1; HV: 2.2; Time: 1/3/2020 3:36:07 AM)"=12276, "Automatic Update (DT: Olivine-3-1; HV: 2.2; Time: 1/3/2020 3:36:09 AM)"=12277, "Automatic Update (DT: Olivine-3-1; HV: 2.2; Time: 1/3/2020 3:36:10 AM)"=12278, "Automatic Update (DT: Olivine-3-1; HV: 2.2; Time: 1/3/2020 3:49:45 AM)"=12279, "Automatic Update (DT: Olivine-3-1; HV: 2.2; Time: 1/3/2020 3:49:46 AM)"=12280, "Automatic Update (DT: Olivine-3-1; HV: 2.2; Time: 1/3/2020 3:49:47 AM)"=12281, "Automatic Update (DT: Olivine-3-1; HV: 2.2; Time: 1/3/2020 3:49:48 AM)"=12282, "Automatic Update (DT: Olivine-3-1; HV: 2.2; Time: 1/3/2020 3:49:49 AM)"=12283, "Automatic Update (DT: Olivine-3-1; HV: 2.2; Time: 1/3/2020 3:49:50 AM)"=12284, "Automatic Update (DT: Olivine-3-1; HV: 2.2; Time: 1/3/2020 3:49:51 AM)"=12285, "Automatic Update (DT: Olivine-3-1; HV: 2.2; Time: 1/3/2020 3:49:52 AM)"=12286, "Automatic Update (DT: Olivine-3-1; HV: 2.2; Time: 1/3/2020 3:49:53 AM)"=12287, "Automatic Update (DT: Olivine-3-1; HV: 2.2; Time: 1/3/2020 3:49:54 AM)"=12288, "Automatic Update (DT: Olivine-3-1; HV: 2.2; Time: 1/3/2020 3:49:55 AM)"=12289, "Automatic Update (DT: Olivine-3-1; HV: 2.2; Time: 1/3/2020 3:49:56 AM)"=12290, "Automatic Update (DT: Olivine-3-1; HV: 2.2; Time: 1/3/2020 3:49:57 AM)"=12291, "Automatic Update (DT: Olivine-3-1; HV: 2.2; Time: 1/3/2020 3:51:13 AM)"=12292, "Automatic Update (DT: Olivine-3-1; HV: 2.2; Time: 1/3/2020 3:51:14 AM)"=12293, "Automatic Update (DT: Olivine-3-1; HV: 2.2; Time: 1/3/2020 3:51:15 AM)"=12294, "Automatic Update (DT: Olivine-3-1; HV: 2.2; Time: 1/3/2020 3:51:16 AM)"=12295, "Automatic Update (DT: Olivine-3-1; HV: 2.2; Time: 1/3/2020 3:51:17 AM)"=12296, "Automatic Update (DT: Olivine-3-1; HV: 2.2; Time: 1/3/2020 3:51:18 AM)"=12297, "Automatic Update (DT: Olivine-3-1; HV: 2.2; Time: 1/3/2020 3:51:19 AM)"=12298, "Automatic Update (DT: Olivine-3-1; HV: 2.2; Time: 1/3/2020 3:51:20 AM)"=12299, "Automatic Update (DT: Olivine-3-1; HV: 2.2; Time: 1/3/2020 3:51:21 AM)"=12300, "Automatic Update (DT: Olivine-3-1; HV: 2.2; Time: 1/3/2020 3:51:22 AM)"=12301, "Automatic Update (DT: Olivine-3-1; HV: 2.2; Time: 1/3/2020 3:51:23 AM)"=12302, "Automatic Update (DT: Olivine-3-1; HV: 2.2; Time: 1/3/2020 3:51:24 AM)"=12303, "Automatic Update (DT: Olivine-3-1; HV: 2.2; Time: 1/3/2020 3:51:25 AM)"=12304, "Automatic Update (DT: Olivine-3-1; HV: 2.2; Time: 1/3/2020 3:51:27 AM)"=12305, "Automatic Update (DT: Olivine-3-1; HV: 2.2; Time: 1/3/2020 3:51:28 AM)"=12306, "Automatic Update (DT: Olivine-3-1; HV: 2.2; Time: 1/3/2020 3:51:29 AM)"=12307, "Automatic Update (DT: Olivine-3-1; HV: 2.2; Time: 1/3/2020 3:51:30 AM)"=12308, "Automatic Update (DT: Olivine-3-1; HV: 2.2; Time: 1/3/2020 3:51:31 AM)"=12309, "Automatic Update (DT: Olivine-3-1; HV: 2.2; Time: 1/3/2020 3:51:32 AM)"=12310, "Automatic Update (DT: Olivine-3-1; HV: 2.2; Time: 1/3/2020 3:51:34 AM)"=12311, "Automatic Update (DT: Olivine-3-1; HV: 2.2; Time: 1/3/2020 3:51:35 AM)"=12312, "Automatic Update (DT: Olivine-3-1; HV: 2.2; Time: 1/3/2020 3:51:36 AM)"=12313, "Automatic Update (DT: Olivine-3-1; HV: 2.2; Time: 1/3/2020 3:51:37 AM)"=12314, "Automatic Update (DT: Olivine-3-1; HV: 2.2; Time: 1/3/2020 3:51:38 AM)"=12315, "Automatic Update (DT: Olivine-3-1; HV: 2.2; Time: 1/3/2020 3:51:39 AM)"=12316, "Automatic Update (DT: Olivine-3-1; HV: 2.2; Time: 1/3/2020 3:51:40 AM)"=12317, "Automatic Update (DT: Olivine-3-1; HV: 2.2; Time: 1/3/2020 3:51:41 AM)"=12318, "Automatic Update (DT: Olivine-3-1; HV: 2.2; Time: 1/3/2020 3:51:42 AM)"=12319, "Automatic Update (DT: Olivine-3-1; HV: 2.2; Time: 1/3/2020 3:51:43 AM)"=12320, "Automatic Update (DT: Olivine-3-1; HV: 2.2; Time: 1/3/2020 3:51:44 AM)"=12321, "Automatic Update (DT: Olivine-3-1; HV: 2.2; Time: 1/3/2020 3:51:45 AM)"=12322, "Automatic Update (DT: Olivine-3-1; HV: 2.2; Time: 1/3/2020 3:51:46 AM)"=12323, "Automatic Update (DT: Olivine-3-1; HV: 2.2; Time: 1/3/2020 3:51:47 AM)"=12324, "Automatic Update (DT: Olivine-3-1; HV: 2.2; Time: 1/3/2020 3:51:48 AM)"=12325, "Automatic Update (DT: Olivine-3-1; HV: 2.2; Time: 1/3/2020 3:51:49 AM)"=12326, "Automatic Update (DT: Olivine-3-1; HV: 2.2; Time: 1/3/2020 3:51:50 AM)"=12327, "Automatic Update (DT: Olivine-3-1; HV: 2.2; Time: 1/3/2020 3:51:51 AM)"=12328, "Automatic Update (DT: Olivine-3-1; HV: 2.2; Time: 1/3/2020 3:51:52 AM)"=12329, "Automatic Update (DT: Olivine-3-1; HV: 2.2; Time: 1/3/2020 3:51:53 AM)"=12330, "Automatic Update (DT: Olivine-3-1; HV: 2.2; Time: 1/3/2020 3:51:54 AM)"=12331, "Automatic Update (DT: Olivine-3-1; HV: 2.2; Time: 1/3/2020 3:51:55 AM)"=12332, "Automatic Update (DT: Olivine-3-1; HV: 2.2; Time: 1/3/2020 3:51:57 AM)"=12333, "Automatic Update (DT: Olivine-3-1; HV: 2.2; Time: 1/3/2020 3:51:58 AM)"=12334, "Automatic Update (DT: Olivine-3-1; HV: 2.2; Time: 1/3/2020 3:51:59 AM)"=12335, "Automatic Update (DT: Olivine-3-1; HV: 2.2; Time: 1/3/2020 3:52:00 AM)"=12336, "Automatic Update (DT: Olivine-3-1; HV: 2.2; Time: 1/3/2020 3:52:01 AM)"=12337, "Automatic Update (DT: Olivine-3-1; HV: 2.2; Time: 1/3/2020 3:52:02 AM)"=12338, "Automatic Update (DT: Olivine-3-1; HV: 2.2; Time: 1/3/2020 3:52:03 AM)"=12339, "Automatic Update (DT: Olivine-3-1; HV: 2.2; Time: 1/3/2020 3:52:04 AM)"=12340, "Automatic Update (DT: Olivine-3-1; HV: 2.2; Time: 1/3/2020 3:52:07 AM)"=12341, "Automatic Update (DT: Olivine-3-1; HV: 2.2; Time: 1/3/2020 3:52:08 AM)"=12342, "Automatic Update (DT: Olivine-3-1; HV: 2.2; Time: 1/3/2020 3:52:09 AM)"=12343, "Automatic Update (DT: Olivine-3-1; HV: 2.2; Time: 1/3/2020 3:52:10 AM)"=12344, "Automatic Update (DT: Olivine-3-1; HV: 2.2; Time: 1/3/2020 3:52:11 AM)"=12345, "Automatic Update (DT: Olivine-3-1; HV: 2.2; Time: 1/3/2020 3:52:12 AM)"=12346, "Automatic Update (DT: Olivine-3-1; HV: 2.2; Time: 1/3/2020 3:52:13 AM)"=12347, "Automatic Update (DT: Olivine-3-1; HV: 2.2; Time: 1/3/2020 3:52:14 AM)"=12348, "Automatic Update (DT: Olivine-3-1; HV: 2.2; Time: 1/3/2020 3:52:15 AM)"=12349, "Automatic Update (DT: Olivine-3-1; HV: 2.2; Time: 1/3/2020 3:52:17 AM)"=12350, "Automatic Update (DT: Olivine-3-1; HV: 2.2; Time: 1/3/2020 3:52:18 AM)"=12351, "Automatic Update (DT: Olivine-3-1; HV: 2.2; Time: 1/3/2020 3:52:21 AM)"=12352, "Automatic Update (DT: Olivine-3-1; HV: 2.2; Time: 1/3/2020 3:52:22 AM)"=12353, "Automatic Update (DT: Olivine-3-1; HV: 2.2; Time: 1/3/2020 3:52:23 AM)"=12354, "Automatic Update (DT: Olivine-3-1; HV: 2.2; Time: 1/3/2020 3:52:24 AM)"=12355, "Automatic Update (DT: Olivine-3-1; HV: 2.2; Time: 1/3/2020 3:52:25 AM)"=12356, "Automatic Update (DT: Olivine-3-1; HV: 2.2; Time: 1/3/2020 3:52:26 AM)"=12357, "Automatic Update (DT: Olivine-3-1; HV: 2.2; Time: 1/3/2020 3:52:27 AM)"=12358, "Automatic Update (DT: Olivine-3-1; HV: 2.2; Time: 1/3/2020 3:52:28 AM)"=12359, "Automatic Update (DT: Olivine-3-1; HV: 2.2; Time: 1/3/2020 3:52:29 AM)"=12360, "Automatic Update (DT: Olivine-3-1; HV: 2.2; Time: 1/3/2020 3:52:30 AM)"=12361, "Automatic Update (DT: Olivine-3-1; HV: 2.2; Time: 1/3/2020 3:52:31 AM)"=12362, "Automatic Update (DT: Olivine-3-1; HV: 2.2; Time: 1/3/2020 3:52:32 AM)"=12363, "Automatic Update (DT: Olivine-3-1; HV: 2.2; Time: 1/3/2020 3:52:33 AM)"=12364, "Automatic Update (DT: Olivine-3-1; HV: 2.2; Time: 1/3/2020 3:52:34 AM)"=12365, "Automatic Update (DT: Olivine-3-1; HV: 2.2; Time: 1/3/2020 3:52:35 AM)"=12366, "Automatic Update (DT: Olivine-3-1; HV: 2.2; Time: 1/3/2020 3:52:36 AM)"=12367, "Automatic Update (DT: Olivine-3-1; HV: 2.2; Time: 1/3/2020 3:52:37 AM)"=12368, "Automatic Update (DT: Olivine-3-1; HV: 2.2; Time: 1/3/2020 3:52:41 AM)"=12369, "Automatic Update (DT: Olivine-3-1; HV: 2.2; Time: 1/3/2020 3:52:42 AM)"=12370, "Automatic Update (DT: Olivine-3-1; HV: 2.2; Time: 1/3/2020 3:52:43 AM)"=12371, "Automatic Update (DT: Olivine-3-1; HV: 2.2; Time: 1/3/2020 3:52:44 AM)"=12372, "Automatic Update (DT: Olivine-3-1; HV: 2.2; Time: 1/3/2020 3:52:45 AM)"=12373, "Automatic Update (DT: Olivine-3-1; HV: 2.2; Time: 1/3/2020 3:52:46 AM)"=12374, "Automatic Update (DT: Olivine-3-1; HV: 2.2; Time: 1/3/2020 3:52:47 AM)"=12375, "Automatic Update (DT: Olivine-3-1; HV: 2.2; Time: 1/3/2020 3:52:48 AM)"=12376, "Automatic Update (DT: Olivine-3-1; HV: 2.2; Time: 1/3/2020 3:52:49 AM)"=12377, "Automatic Update (DT: Olivine-3-1; HV: 2.2; Time: 1/3/2020 3:52:50 AM)"=12378, "Automatic Update (DT: Olivine-3-1; HV: 2.2; Time: 1/3/2020 3:52:51 AM)"=12379, "Automatic Update (DT: Olivine-3-1; HV: 2.2; Time: 1/3/2020 3:52:52 AM)"=12380, "Automatic Update (DT: Olivine-3-1; HV: 2.2; Time: 1/3/2020 3:52:53 AM)"=12381, "Automatic Update (DT: Olivine-3-1; HV: 2.2; Time: 1/3/2020 3:52:54 AM)"=12382, "Automatic Update (DT: Olivine-3-1; HV: 2.2; Time: 1/3/2020 3:52:55 AM)"=12383, "Automatic Update (DT: Olivine-3-1; HV: 2.2; Time: 1/3/2020 3:53:00 AM)"=12384, "Automatic Update (DT: Olivine-3-1; HV: 2.2; Time: 1/3/2020 3:53:01 AM)"=12385, "Automatic Update (DT: Olivine-3-1; HV: 2.2; Time: 1/3/2020 3:53:02 AM)"=12386, "Automatic Update (DT: Olivine-3-1; HV: 2.2; Time: 1/3/2020 3:53:03 AM)"=12387, "Automatic Update (DT: Olivine-3-1; HV: 2.2; Time: 1/3/2020 3:53:04 AM)"=12388, "Automatic Update (DT: Olivine-3-1; HV: 2.2; Time: 1/3/2020 3:53:06 AM)"=12389, "Automatic Update (DT: Olivine-3-1; HV: 2.2; Time: 1/3/2020 3:53:07 AM)"=12390, "Automatic Update (DT: Olivine-3-1; HV: 2.2; Time: 1/3/2020 3:53:08 AM)"=12391, "Automatic Update (DT: Olivine-3-1; HV: 2.2; Time: 1/3/2020 3:53:09 AM)"=12392, "Automatic Update (DT: Olivine-3-1; HV: 2.2; Time: 1/3/2020 3:53:10 AM)"=12393, "Automatic Update (DT: Olivine-3-1; HV: 2.2; Time: 1/3/2020 3:53:11 AM)"=12394, "Automatic Update (DT: Olivine-3-1; HV: 2.2; Time: 1/3/2020 3:53:12 AM)"=12395, "Automatic Update (DT: Olivine-3-1; HV: 2.2; Time: 1/3/2020 3:53:13 AM)"=12396, "Automatic Update (DT: Olivine-3-1; HV: 2.2; Time: 1/3/2020 3:53:14 AM)"=12397, "Automatic Update (DT: Olivine-3-1; HV: 2.2; Time: 1/3/2020 3:53:15 AM)"=12398, "Automatic Update (DT: Olivine-3-1; HV: 2.2; Time: 1/3/2020 3:53:16 AM)"=12399, "Automatic Update (DT: Olivine-3-1; HV: 2.2; Time: 1/3/2020 3:53:18 AM)"=12400, "Automatic Update (DT: Olivine-3-1; HV: 2.2; Time: 1/3/2020 3:53:19 AM)"=12401, "Automatic Update (DT: Olivine-3-1; HV: 2.2; Time: 1/3/2020 3:53:20 AM)"=12402, "Automatic Update (DT: Olivine-3-1; HV: 2.2; Time: 1/3/2020 3:53:21 AM)"=12403, "Automatic Update (DT: Olivine-3-1; HV: 2.2; Time: 1/3/2020 3:53:22 AM)"=12404, "Automatic Update (DT: Olivine-3-1; HV: 2.2; Time: 1/3/2020 3:53:23 AM)"=12405, "Automatic Update (DT: Olivine-3-1; HV: 2.2; Time: 1/3/2020 3:53:24 AM)"=12406, "Automatic Update (DT: Olivine-3-1; HV: 2.2; Time: 1/3/2020 3:53:26 AM)"=12407, "Automatic Update (DT: Olivine-3-1; HV: 2.2; Time: 1/3/2020 3:53:27 AM)"=12408, "Automatic Update (DT: Olivine-3-1; HV: 2.2; Time: 1/3/2020 3:53:28 AM)"=12409, "Automatic Update (DT: Olivine-3-1; HV: 2.2; Time: 1/3/2020 3:53:29 AM)"=12410, "Automatic Update (DT: Olivine-3-1; HV: 2.2; Time: 1/3/2020 3:53:31 AM)"=12411, "Automatic Update (DT: Olivine-3-1; HV: 2.2; Time: 1/3/2020 3:53:32 AM)"=12412, "Automatic Update (DT: Olivine-3-1; HV: 2.2; Time: 1/3/2020 3:53:33 AM)"=12413, "Automatic Update (DT: Olivine-3-1; HV: 2.2; Time: 1/3/2020 3:53:34 AM)"=12414, "Automatic Update (DT: Olivine-3-1; HV: 2.2; Time: 1/3/2020 3:53:35 AM)"=12415, "Automatic Update (DT: Olivine-3-1; HV: 2.2; Time: 1/3/2020 3:53:36 AM)"=12416, "Automatic Update (DT: Olivine-3-1; HV: 2.2; Time: 1/3/2020 3:53:42 AM)"=12417, "Automatic Update (DT: Olivine-3-1; HV: 2.2; Time: 1/3/2020 3:53:43 AM)"=12418, "Automatic Update (DT: Olivine-3-1; HV: 2.2; Time: 1/3/2020 3:53:44 AM)"=12419, "Automatic Update (DT: Olivine-3-1; HV: 2.2; Time: 1/3/2020 3:53:45 AM)"=12420, "Automatic Update (DT: Olivine-3-1; HV: 2.2; Time: 1/3/2020 3:53:46 AM)"=12421, "Automatic Update (DT: Olivine-3-1; HV: 2.2; Time: 1/3/2020 3:53:47 AM)"=12422, "Automatic Update (DT: Olivine-3-1; HV: 2.2; Time: 1/3/2020 3:53:48 AM)"=12423, "Automatic Update (DT: Olivine-3-1; HV: 2.2; Time: 1/3/2020 3:53:49 AM)"=12424, "Automatic Update (DT: Olivine-3-1; HV: 2.2; Time: 1/3/2020 3:53:50 AM)"=12425, "Automatic Update (DT: Olivine-3-1; HV: 2.2; Time: 1/3/2020 3:53:51 AM)"=12426, "Automatic Update (DT: Olivine-3-1; HV: 2.2; Time: 1/3/2020 3:53:52 AM)"=12427, "Automatic Update (DT: Olivine-3-1; HV: 2.2; Time: 1/3/2020 3:53:53 AM)"=12428, "Automatic Update (DT: Olivine-3-1; HV: 2.2; Time: 1/3/2020 3:53:54 AM)"=12429, "Automatic Update (DT: Olivine-3-1; HV: 2.2; Time: 1/3/2020 3:53:56 AM)"=12430, "Automatic Update (DT: Olivine-3-1; HV: 2.2; Time: 1/3/2020 3:53:57 AM)"=12431, "Automatic Update (DT: Olivine-3-1; HV: 2.2; Time: 1/3/2020 3:53:59 AM)"=12432, "Automatic Update (DT: Olivine-3-1; HV: 2.2; Time: 1/3/2020 3:54:00 AM)"=12433, "Automatic Update (DT: Olivine-3-1; HV: 2.2; Time: 1/3/2020 3:54:01 AM)"=12434, "Automatic Update (DT: Olivine-3-1; HV: 2.2; Time: 1/3/2020 3:54:02 AM)"=12435, "Automatic Update (DT: Olivine-3-1; HV: 2.2; Time: 1/3/2020 3:54:05 AM)"=12436, "Automatic Update (DT: Olivine-3-1; HV: 2.2; Time: 1/3/2020 3:54:06 AM)"=12437, "Automatic Update (DT: Olivine-3-1; HV: 2.2; Time: 1/3/2020 3:54:07 AM)"=12438, "Automatic Update (DT: Olivine-3-1; HV: 2.2; Time: 1/3/2020 3:54:08 AM)"=12439, "Automatic Update (DT: Olivine-3-1; HV: 2.2; Time: 1/3/2020 3:54:09 AM)"=12440, "Automatic Update (DT: Olivine-3-1; HV: 2.2; Time: 1/3/2020 3:54:10 AM)"=12441, "Automatic Update (DT: Olivine-3-1; HV: 2.2; Time: 1/3/2020 3:54:11 AM)"=12442, "Automatic Update (DT: Olivine-3-1; HV: 2.2; Time: 1/3/2020 3:54:12 AM)"=12443, "Automatic Update (DT: Olivine-3-1; HV: 2.2; Time: 1/3/2020 3:54:13 AM)"=12444, "Automatic Update (DT: Olivine-3-1; HV: 2.2; Time: 1/3/2020 3:54:14 AM)"=12445, "Automatic Update (DT: Olivine-3-1; HV: 2.2; Time: 1/3/2020 3:54:15 AM)"=12446, "Automatic Update (DT: Olivine-3-1; HV: 2.2; Time: 1/3/2020 3:54:16 AM)"=12447, "Automatic Update (DT: Olivine-3-1; HV: 2.2; Time: 1/3/2020 3:54:17 AM)"=12448, "Automatic Update (DT: Olivine-3-1; HV: 2.2; Time: 1/3/2020 3:54:18 AM)"=12449, "Automatic Update (DT: Olivine-3-1; HV: 2.2; Time: 1/3/2020 3:54:19 AM)"=12450, "Automatic Update (DT: Olivine-3-1; HV: 2.2; Time: 1/3/2020 3:54:20 AM)"=12451, "Automatic Update (DT: Olivine-3-1; HV: 2.2; Time: 1/3/2020 3:54:22 AM)"=12452, "Automatic Update (DT: Olivine-3-1; HV: 2.2; Time: 1/3/2020 3:54:23 AM)"=12453, "Automatic Update (DT: Olivine-3-1; HV: 2.2; Time: 1/3/2020 3:54:24 AM)"=12454, "Automatic Update (DT: Olivine-3-1; HV: 2.2; Time: 1/3/2020 3:54:25 AM)"=12455, "Automatic Update (DT: Olivine-3-1; HV: 2.2; Time: 1/3/2020 3:54:26 AM)"=12456, "Automatic Update (DT: Olivine-3-1; HV: 2.2; Time: 1/3/2020 3:54:27 AM)"=12457, "Automatic Update (DT: Olivine-3-1; HV: 2.2; Time: 1/3/2020 3:54:28 AM)"=12458, "Automatic Update (DT: Olivine-3-1; HV: 2.2; Time: 1/3/2020 3:54:29 AM)"=12459, "Automatic Update (DT: Olivine-3-1; HV: 2.2; Time: 1/3/2020 3:54:30 AM)"=12460, "Automatic Update (DT: Olivine-3-1; HV: 2.2; Time: 1/3/2020 3:54:31 AM)"=12461, "Automatic Update (DT: Olivine-3-1; HV: 2.2; Time: 1/3/2020 3:54:32 AM)"=12462, "Automatic Update (DT: Olivine-3-1; HV: 2.2; Time: 1/3/2020 3:54:33 AM)"=12463, "Automatic Update (DT: Olivine-3-1; HV: 2.2; Time: 1/3/2020 3:54:34 AM)"=12464, "Automatic Update (DT: Olivine-3-1; HV: 2.2; Time: 1/3/2020 3:54:35 AM)"=12465, "Automatic Update (DT: Olivine-3-1; HV: 2.2; Time: 1/3/2020 3:54:36 AM)"=12466, "Automatic Update (DT: Olivine-3-1; HV: 2.2; Time: 1/3/2020 3:54:37 AM)"=12467, "Automatic Update (DT: Olivine-3-1; HV: 2.2; Time: 1/3/2020 3:54:38 AM)"=12468, "Automatic Update (DT: Olivine-3-1; HV: 2.2; Time: 1/3/2020 3:54:39 AM)"=12469, "Automatic Update (DT: Olivine-3-1; HV: 2.2; Time: 1/3/2020 3:54:40 AM)"=12470, "Automatic Update (DT: Olivine-3-1; HV: 2.2; Time: 1/3/2020 3:54:46 AM)"=12471, "Automatic Update (DT: Olivine-3-1; HV: 2.2; Time: 1/3/2020 3:54:47 AM)"=12472, "Automatic Update (DT: Olivine-3-1; HV: 2.2; Time: 1/3/2020 3:54:49 AM)"=12473, "Automatic Update (DT: Olivine-3-1; HV: 2.2; Time: 1/3/2020 3:55:37 AM)"=12474, "Automatic Update (DT: Olivine-3-1; HV: 2.2; Time: 1/3/2020 3:55:38 AM)"=12475, "Automatic Update (DT: Olivine-3-1; HV: 2.2; Time: 1/3/2020 3:55:39 AM)"=12476, "Automatic Update (DT: Olivine-3-1; HV: 2.2; Time: 1/3/2020 3:55:40 AM)"=12477, "Automatic Update (DT: Olivine-3-1; HV: 2.2; Time: 1/3/2020 3:55:41 AM)"=12478, "Automatic Update (DT: Olivine-3-1; HV: 2.2; Time: 1/3/2020 3:55:42 AM)"=12479, "Automatic Update (DT: Olivine-3-1; HV: 2.2; Time: 1/3/2020 3:55:43 AM)"=12480, "Automatic Update (DT: Olivine-3-1; HV: 2.2; Time: 1/3/2020 3:55:49 AM)"=12481, "Automatic Update (DT: Olivine-3-1; HV: 2.2; Time: 1/3/2020 3:55:50 AM)"=12482, "Automatic Update (DT: Olivine-3-1; HV: 2.2; Time: 1/3/2020 3:55:51 AM)"=12483, "Automatic Update (DT: Olivine-3-1; HV: 2.2; Time: 1/3/2020 3:55:52 AM)"=12484, "Automatic Update (DT: Olivine-3-1; HV: 2.2; Time: 1/3/2020 3:55:53 AM)"=12485, "Automatic Update (DT: Olivine-3-1; HV: 2.2; Time: 1/3/2020 3:55:54 AM)"=12486, "Automatic Update (DT: Olivine-3-1; HV: 2.2; Time: 1/3/2020 3:55:56 AM)"=12487, "Automatic Update (DT: Olivine-3-1; HV: 2.2; Time: 1/3/2020 3:55:57 AM)"=12488, "Automatic Update (DT: Olivine-3-1; HV: 2.2; Time: 1/3/2020 3:55:58 AM)"=12489, "Automatic Update (DT: Olivine-3-1; HV: 2.2; Time: 1/3/2020 3:55:59 AM)"=12490, "Automatic Update (DT: Olivine-3-1; HV: 2.2; Time: 1/3/2020 3:56:00 AM)"=12491, "Automatic Update (DT: Olivine-3-1; HV: 2.2; Time: 1/3/2020 3:56:01 AM)"=12492, "Automatic Update (DT: Olivine-3-1; HV: 2.2; Time: 1/3/2020 3:56:02 AM)"=12493, "Automatic Update (DT: Olivine-3-1; HV: 2.2; Time: 1/3/2020 3:56:04 AM)"=12494, "Automatic Update (DT: Olivine-3-1; HV: 2.2; Time: 1/3/2020 3:56:05 AM)"=12495, "Automatic Update (DT: Olivine-3-1; HV: 2.2; Time: 1/3/2020 3:56:06 AM)"=12496, "Automatic Update (DT: Olivine-3-1; HV: 2.2; Time: 1/3/2020 3:56:07 AM)"=12497, "Automatic Update (DT: Olivine-3-1; HV: 2.2; Time: 1/3/2020 3:56:08 AM)"=12498, "Automatic Update (DT: Olivine-3-1; HV: 2.2; Time: 1/3/2020 3:56:09 AM)"=12499, "Automatic Update (DT: Olivine-3-1; HV: 2.2; Time: 1/3/2020 3:56:10 AM)"=12500, "Automatic Update (DT: Olivine-3-1; HV: 2.2; Time: 1/3/2020 3:56:11 AM)"=12501, "Automatic Update (DT: Olivine-3-1; HV: 2.2; Time: 1/3/2020 3:56:12 AM)"=12502, "Automatic Update (DT: Olivine-3-1; HV: 2.2; Time: 1/3/2020 3:56:13 AM)"=12503, "Automatic Update (DT: Olivine-3-1; HV: 2.2; Time: 1/3/2020 3:56:14 AM)"=12504, "Automatic Update (DT: Olivine-3-1; HV: 2.2; Time: 1/3/2020 3:56:15 AM)"=12505, "Automatic Update (DT: Olivine-3-1; HV: 2.2; Time: 1/3/2020 3:56:16 AM)"=12506, "Automatic Update (DT: Olivine-3-1; HV: 2.2; Time: 1/3/2020 3:56:17 AM)"=12507, "Automatic Update (DT: Olivine-3-1; HV: 2.2; Time: 1/3/2020 3:56:18 AM)"=12508, "Automatic Update (DT: Olivine-3-1; HV: 2.2; Time: 1/3/2020 3:56:19 AM)"=12509, "Automatic Update (DT: Olivine-3-1; HV: 2.2; Time: 1/3/2020 3:56:20 AM)"=12510, "Automatic Update (DT: Olivine-3-1; HV: 2.2; Time: 1/3/2020 3:56:22 AM)"=12511, "Automatic Update (DT: Olivine-3-1; HV: 2.2; Time: 1/3/2020 3:56:23 AM)"=12512, "Automatic Update (DT: Olivine-3-1; HV: 2.2; Time: 1/3/2020 3:56:25 AM)"=12513, "Automatic Update (DT: Olivine-3-1; HV: 2.2; Time: 1/3/2020 3:56:26 AM)"=12514, "Automatic Update (DT: Olivine-3-1; HV: 2.2; Time: 1/3/2020 3:56:27 AM)"=12515, "Automatic Update (DT: Olivine-3-1; HV: 2.2; Time: 1/3/2020 3:56:28 AM)"=12516, "Automatic Update (DT: Olivine-3-1; HV: 2.2; Time: 1/3/2020 3:56:29 AM)"=12517, "Automatic Update (DT: Olivine-3-1; HV: 2.2; Time: 1/3/2020 3:56:30 AM)"=12518, "Automatic Update (DT: Olivine-3-1; HV: 2.2; Time: 1/3/2020 3:56:31 AM)"=12519, "Automatic Update (DT: Olivine-3-1; HV: 2.2; Time: 1/3/2020 3:56:32 AM)"=12520, "Automatic Update (DT: Olivine-3-1; HV: 2.2; Time: 1/3/2020 3:56:33 AM)"=12521, "Automatic Update (DT: Olivine-3-1; HV: 2.2; Time: 1/3/2020 3:56:34 AM)"=12522, "Automatic Update (DT: Olivine-3-1; HV: 2.2; Time: 1/3/2020 3:56:35 AM)"=12523, "Automatic Update (DT: Olivine-3-1; HV: 2.2; Time: 1/3/2020 3:56:36 AM)"=12524, "Automatic Update (DT: Olivine-3-1; HV: 2.2; Time: 1/3/2020 3:56:38 AM)"=12525, "Automatic Update (DT: Olivine-3-1; HV: 2.2; Time: 1/3/2020 3:56:39 AM)"=12526, "Automatic Update (DT: Olivine-3-1; HV: 2.2; Time: 1/3/2020 3:56:42 AM)"=12527, "Automatic Update (DT: Olivine-3-1; HV: 2.2; Time: 1/3/2020 3:56:43 AM)"=12528, "Automatic Update (DT: Olivine-3-1; HV: 2.2; Time: 1/3/2020 3:56:44 AM)"=12529, "Automatic Update (DT: Olivine-3-1; HV: 2.2; Time: 1/3/2020 3:56:47 AM)"=12530, "Automatic Update (DT: Olivine-3-1; HV: 2.2; Time: 1/3/2020 3:56:48 AM)"=12531, "Automatic Update (DT: Olivine-3-1; HV: 2.2; Time: 1/3/2020 3:56:49 AM)"=12532, "Automatic Update (DT: Olivine-3-1; HV: 2.2; Time: 1/3/2020 3:56:51 AM)"=12533, "Automatic Update (DT: Olivine-3-1; HV: 2.2; Time: 1/3/2020 3:56:52 AM)"=12534, "Automatic Update (DT: Olivine-3-1; HV: 2.2; Time: 1/3/2020 3:56:53 AM)"=12535, "Automatic Update (DT: Olivine-3-1; HV: 2.2; Time: 1/3/2020 3:56:54 AM)"=12536, "Automatic Update (DT: Olivine-3-1; HV: 2.2; Time: 1/3/2020 3:56:55 AM)"=12537, "Automatic Update (DT: Olivine-3-1; HV: 2.2; Time: 1/3/2020 3:56:56 AM)"=12538, "Automatic Update (DT: Olivine-3-1; HV: 2.2; Time: 1/3/2020 3:56:57 AM)"=12539, "Automatic Update (DT: Olivine-3-1; HV: 2.2; Time: 1/3/2020 3:56:58 AM)"=12540, "Automatic Update (DT: Olivine-3-1; HV: 2.2; Time: 1/3/2020 3:56:59 AM)"=12541, "Automatic Update (DT: Olivine-3-1; HV: 2.2; Time: 1/3/2020 3:57:00 AM)"=12542, "Automatic Update (DT: Olivine-3-1; HV: 2.2; Time: 1/3/2020 3:57:02 AM)"=12543, "Automatic Update (DT: Olivine-3-1; HV: 2.2; Time: 1/3/2020 3:57:03 AM)"=12544, "Automatic Update (DT: Olivine-3-1; HV: 2.2; Time: 1/3/2020 3:57:04 AM)"=12545, "Automatic Update (DT: Olivine-3-1; HV: 2.2; Time: 1/3/2020 3:57:05 AM)"=12546, "Automatic Update (DT: Olivine-3-1; HV: 2.2; Time: 1/3/2020 3:57:06 AM)"=12547, "Automatic Update (DT: Olivine-3-1; HV: 2.2; Time: 1/3/2020 3:57:10 AM)"=12548, "Automatic Update (DT: Olivine-3-1; HV: 2.2; Time: 1/3/2020 3:57:12 AM)"=12549, "Automatic Update (DT: Olivine-3-1; HV: 2.2; Time: 1/3/2020 3:57:14 AM)"=12550, "Automatic Update (DT: Olivine-3-1; HV: 2.2; Time: 1/3/2020 3:57:15 AM)"=12551, "Automatic Update (DT: Olivine-3-1; HV: 2.2; Time: 1/3/2020 3:57:16 AM)"=12552, "Automatic Update (DT: Olivine-3-1; HV: 2.2; Time: 1/3/2020 3:57:18 AM)"=12553, "Automatic Update (DT: Olivine-3-1; HV: 2.2; Time: 1/3/2020 3:57:19 AM)"=12554, "Automatic Update (DT: Olivine-3-1; HV: 2.2; Time: 1/3/2020 3:57:21 AM)"=12555, "Automatic Update (DT: Olivine-3-1; HV: 2.2; Time: 1/3/2020 3:57:24 AM)"=12556, "Automatic Update (DT: Olivine-3-1; HV: 2.2; Time: 1/3/2020 3:57:25 AM)"=12557, "Automatic Update (DT: Olivine-3-1; HV: 2.2; Time: 1/3/2020 3:57:26 AM)"=12558, "Automatic Update (DT: Olivine-3-1; HV: 2.2; Time: 1/3/2020 3:57:27 AM)"=12559, "Automatic Update (DT: Olivine-3-1; HV: 2.2; Time: 1/3/2020 3:57:28 AM)"=12560, "Automatic Update (DT: Olivine-3-1; HV: 2.2; Time: 1/3/2020 3:57:29 AM)"=12561, "Automatic Update (DT: Olivine-3-1; HV: 2.2; Time: 1/3/2020 3:57:30 AM)"=12562, "Automatic Update (DT: Olivine-3-1; HV: 2.2; Time: 1/3/2020 3:57:31 AM)"=12563, "Automatic Update (DT: Olivine-3-1; HV: 2.2; Time: 1/3/2020 3:57:32 AM)"=12564, "Automatic Update (DT: Olivine-3-1; HV: 2.2; Time: 1/3/2020 3:57:33 AM)"=12565, "Automatic Update (DT: Olivine-3-1; HV: 2.2; Time: 1/3/2020 3:57:34 AM)"=12566, "Automatic Update (DT: Olivine-3-1; HV: 2.2; Time: 1/3/2020 3:57:35 AM)"=12567, "Automatic Update (DT: Olivine-3-1; HV: 2.2; Time: 1/3/2020 3:57:36 AM)"=12568, "Automatic Update (DT: Olivine-3-1; HV: 2.2; Time: 1/3/2020 3:57:37 AM)"=12569, "Automatic Update (DT: Olivine-3-1; HV: 2.2; Time: 1/3/2020 3:57:38 AM)"=12570, "Automatic Update (DT: Olivine-3-1; HV: 2.2; Time: 1/3/2020 3:57:39 AM)"=12571, "Automatic Update (DT: Olivine-3-1; HV: 2.2; Time: 1/3/2020 3:57:40 AM)"=12572, "Automatic Update (DT: Olivine-3-1; HV: 2.2; Time: 1/3/2020 3:57:41 AM)"=12573, "Automatic Update (DT: Olivine-3-1; HV: 2.2; Time: 1/3/2020 3:57:42 AM)"=12574, "Automatic Update (DT: Olivine-3-1; HV: 2.2; Time: 1/3/2020 3:57:44 AM)"=12575, "Automatic Update (DT: Olivine-3-1; HV: 2.2; Time: 1/3/2020 3:57:45 AM)"=12576, "Automatic Update (DT: Olivine-3-1; HV: 2.2; Time: 1/3/2020 3:57:46 AM)"=12577, "Automatic Update (DT: Olivine-3-1; HV: 2.2; Time: 1/3/2020 3:57:47 AM)"=12578, "Automatic Update (DT: Olivine-3-1; HV: 2.2; Time: 1/3/2020 3:57:48 AM)"=12579, "Automatic Update (DT: Olivine-3-1; HV: 2.2; Time: 1/3/2020 3:57:49 AM)"=12580, "Automatic Update (DT: Olivine-3-1; HV: 2.2; Time: 1/3/2020 3:57:52 AM)"=12581, "Automatic Update (DT: Olivine-3-1; HV: 2.2; Time: 1/3/2020 3:57:53 AM)"=12582, "Automatic Update (DT: Olivine-3-1; HV: 2.2; Time: 1/3/2020 3:57:54 AM)"=12583, "Automatic Update (DT: Olivine-3-1; HV: 2.2; Time: 1/3/2020 3:57:55 AM)"=12584, "Automatic Update (DT: Olivine-3-1; HV: 2.2; Time: 1/3/2020 3:57:56 AM)"=12585, "Automatic Update (DT: Olivine-3-1; HV: 2.2; Time: 1/3/2020 3:57:57 AM)"=12586, "Automatic Update (DT: Olivine-3-1; HV: 2.2; Time: 1/3/2020 3:57:58 AM)"=12587, "Automatic Update (DT: Olivine-3-1; HV: 2.2; Time: 1/3/2020 3:57:59 AM)"=12588, "Automatic Update (DT: Olivine-3-1; HV: 2.2; Time: 1/3/2020 3:58:00 AM)"=12589, "Automatic Update (DT: Olivine-3-1; HV: 2.2; Time: 1/3/2020 3:58:01 AM)"=12590, "Automatic Update (DT: Olivine-3-1; HV: 2.2; Time: 1/3/2020 3:58:02 AM)"=12591, "Automatic Update (DT: Olivine-3-1; HV: 2.2; Time: 1/3/2020 3:58:03 AM)"=12592, "Automatic Update (DT: Olivine-3-1; HV: 2.2; Time: 1/3/2020 3:58:04 AM)"=12593, "Automatic Update (DT: Olivine-3-1; HV: 2.2; Time: 1/3/2020 3:58:06 AM)"=12594, "Automatic Update (DT: Olivine-3-1; HV: 2.2; Time: 1/3/2020 3:58:07 AM)"=12595, "Automatic Update (DT: Olivine-3-1; HV: 2.2; Time: 1/3/2020 3:58:08 AM)"=12596, "Automatic Update (DT: Olivine-3-1; HV: 2.2; Time: 1/3/2020 3:58:09 AM)"=12597, "Automatic Update (DT: Olivine-3-1; HV: 2.2; Time: 1/3/2020 3:58:10 AM)"=12598, "Automatic Update (DT: Olivine-3-1; HV: 2.2; Time: 1/3/2020 3:58:11 AM)"=12599, "Automatic Update (DT: Olivine-3-1; HV: 2.2; Time: 1/3/2020 3:58:12 AM)"=12600, "Automatic Update (DT: Olivine-3-1; HV: 2.2; Time: 1/3/2020 3:58:13 AM)"=12601, "Automatic Update (DT: Olivine-3-1; HV: 2.2; Time: 1/3/2020 3:58:14 AM)"=12602, "Automatic Update (DT: Olivine-3-1; HV: 2.2; Time: 1/3/2020 3:58:15 AM)"=12603, "Automatic Update (DT: Olivine-3-1; HV: 2.2; Time: 1/3/2020 3:58:16 AM)"=12604, "Automatic Update (DT: Olivine-3-1; HV: 2.2; Time: 1/3/2020 3:58:17 AM)"=12605, "Automatic Update (DT: Olivine-3-1; HV: 2.2; Time: 1/3/2020 3:58:18 AM)"=12606, "Automatic Update (DT: Olivine-3-1; HV: 2.2; Time: 1/3/2020 3:58:19 AM)"=12607, "Automatic Update (DT: Olivine-3-1; HV: 2.2; Time: 1/3/2020 3:58:20 AM)"=12608, "Automatic Update (DT: Olivine-3-1; HV: 2.2; Time: 1/3/2020 3:58:21 AM)"=12609, "Automatic Update (DT: Olivine-3-1; HV: 2.2; Time: 1/3/2020 3:58:22 AM)"=12610, "Automatic Update (DT: Olivine-3-1; HV: 2.2; Time: 1/3/2020 3:58:23 AM)"=12611, "Automatic Update (DT: Olivine-3-1; HV: 2.2; Time: 1/3/2020 3:58:24 AM)"=12612, "Automatic Update (DT: Olivine-3-1; HV: 2.2; Time: 1/3/2020 3:58:25 AM)"=12613, "Automatic Update (DT: Olivine-3-1; HV: 2.2; Time: 1/3/2020 3:58:26 AM)"=12614, "Automatic Update (DT: Olivine-3-1; HV: 2.2; Time: 1/3/2020 3:58:28 AM)"=12615, "Automatic Update (DT: Olivine-3-1; HV: 2.2; Time: 1/3/2020 3:58:29 AM)"=12616, "Automatic Update (DT: Olivine-3-1; HV: 2.2; Time: 1/3/2020 3:58:30 AM)"=12617, "Automatic Update (DT: Olivine-3-1; HV: 2.2; Time: 1/3/2020 3:58:31 AM)"=12618, "Automatic Update (DT: Olivine-3-1; HV: 2.2; Time: 1/3/2020 3:58:32 AM)"=12619, "Automatic Update (DT: Olivine-3-1; HV: 2.2; Time: 1/3/2020 3:58:33 AM)"=12620, "Automatic Update (DT: Olivine-3-1; HV: 2.2; Time: 1/3/2020 3:58:35 AM)"=12621, "Automatic Update (DT: Olivine-3-1; HV: 2.2; Time: 1/3/2020 3:58:37 AM)"=12622, "Automatic Update (DT: Olivine-3-1; HV: 2.2; Time: 1/3/2020 3:58:38 AM)"=12623, "Automatic Update (DT: Olivine-3-1; HV: 2.2; Time: 1/3/2020 3:58:39 AM)"=12624, "Automatic Update (DT: Olivine-3-1; HV: 2.2; Time: 1/3/2020 3:58:40 AM)"=12625, "Automatic Update (DT: Olivine-3-1; HV: 2.2; Time: 1/3/2020 3:58:45 AM)"=12626, "Automatic Update (DT: Olivine-3-1; HV: 2.2; Time: 1/3/2020 3:58:46 AM)"=12627, "Automatic Update (DT: Olivine-3-1; HV: 2.2; Time: 1/3/2020 3:58:47 AM)"=12628, "Automatic Update (DT: Olivine-3-1; HV: 2.2; Time: 1/3/2020 3:58:48 AM)"=12629, "Automatic Update (DT: Olivine-3-1; HV: 2.2; Time: 1/3/2020 3:58:49 AM)"=12630, "Automatic Update (DT: Olivine-3-1; HV: 2.2; Time: 1/3/2020 3:58:50 AM)"=12631, "Automatic Update (DT: Olivine-3-1; HV: 2.2; Time: 1/3/2020 3:58:51 AM)"=12632, "Automatic Update (DT: Olivine-3-1; HV: 2.2; Time: 1/3/2020 3:58:52 AM)"=12633, "Automatic Update (DT: Olivine-3-1; HV: 2.2; Time: 1/3/2020 3:58:53 AM)"=12634, "Automatic Update (DT: Olivine-3-1; HV: 2.2; Time: 1/3/2020 3:58:54 AM)"=12635, "Automatic Update (DT: Olivine-3-1; HV: 2.2; Time: 1/3/2020 3:58:55 AM)"=12636, "Automatic Update (DT: Olivine-3-1; HV: 2.2; Time: 1/3/2020 3:59:48 AM)"=12637, "Automatic Update (DT: Olivine-3-1; HV: 2.2; Time: 1/3/2020 3:59:49 AM)"=12638, "Automatic Update (DT: Olivine-3-1; HV: 2.2; Time: 1/3/2020 3:59:50 AM)"=12639, "Automatic Update (DT: Olivine-3-1; HV: 2.2; Time: 1/3/2020 3:59:51 AM)"=12640, "Automatic Update (DT: Olivine-3-1; HV: 2.2; Time: 1/3/2020 3:59:52 AM)"=12641, "Automatic Update (DT: Olivine-3-1; HV: 2.2; Time: 1/3/2020 3:59:53 AM)"=12642, "Automatic Update (DT: Olivine-3-1; HV: 2.2; Time: 1/3/2020 3:59:54 AM)"=12643, "Automatic Update (DT: Olivine-3-1; HV: 2.2; Time: 1/3/2020 3:59:55 AM)"=12644, "Automatic Update (DT: Olivine-3-1; HV: 2.2; Time: 1/3/2020 3:59:56 AM)"=12645, "Automatic Update (DT: Olivine-3-1; HV: 2.2; Time: 1/3/2020 3:59:57 AM)"=12646, "Automatic Update (DT: Olivine-3-1; HV: 2.2; Time: 1/3/2020 3:59:58 AM)"=12647, "Automatic Update (DT: Olivine-3-1; HV: 2.2; Time: 1/3/2020 4:00:00 AM)"=12648, "Automatic Update (DT: Olivine-3-1; HV: 2.2; Time: 1/3/2020 4:00:01 AM)"=12649, "Automatic Update (DT: Olivine-3-1; HV: 2.2; Time: 1/3/2020 4:00:02 AM)"=12650, "Automatic Update (DT: Olivine-3-1; HV: 2.2; Time: 1/3/2020 4:00:03 AM)"=12651, "Automatic Update (DT: Olivine-3-1; HV: 2.2; Time: 1/3/2020 4:00:04 AM)"=12652, "Automatic Update (DT: Olivine-3-1; HV: 2.2; Time: 1/3/2020 4:00:05 AM)"=12653, "Automatic Update (DT: Olivine-3-1; HV: 2.2; Time: 1/3/2020 4:00:08 AM)"=12654, "Automatic Update (DT: Olivine-3-1; HV: 2.2; Time: 1/3/2020 4:00:09 AM)"=12655, "Automatic Update (DT: Olivine-3-1; HV: 2.2; Time: 1/3/2020 4:00:10 AM)"=12656, "Automatic Update (DT: Olivine-3-1; HV: 2.2; Time: 1/3/2020 4:00:11 AM)"=12657, "Automatic Update (DT: Olivine-3-1; HV: 2.2; Time: 1/3/2020 4:00:12 AM)"=12658, "Automatic Update (DT: Olivine-3-1; HV: 2.2; Time: 1/3/2020 4:00:14 AM)"=12659, "Automatic Update (DT: Olivine-3-1; HV: 2.2; Time: 1/3/2020 4:00:15 AM)"=12660, "Automatic Update (DT: Olivine-3-1; HV: 2.2; Time: 1/3/2020 4:00:16 AM)"=12661, "Automatic Update (DT: Olivine-3-1; HV: 2.2; Time: 1/3/2020 4:00:17 AM)"=12662, "Automatic Update (DT: Olivine-3-1; HV: 2.2; Time: 1/3/2020 4:00:18 AM)"=12663, "Automatic Update (DT: Olivine-3-1; HV: 2.2; Time: 1/3/2020 4:00:19 AM)"=12664, "Automatic Update (DT: Olivine-3-1; HV: 2.2; Time: 1/3/2020 4:00:20 AM)"=12665, "Automatic Update (DT: Olivine-3-1; HV: 2.2; Time: 1/3/2020 4:00:21 AM)"=12666, "Automatic Update (DT: Olivine-3-1; HV: 2.2; Time: 1/3/2020 4:00:22 AM)"=12667, "Automatic Update (DT: Olivine-3-1; HV: 2.2; Time: 1/3/2020 4:00:23 AM)"=12668, "Automatic Update (DT: Olivine-3-1; HV: 2.2; Time: 1/3/2020 4:00:24 AM)"=12669, "Automatic Update (DT: Olivine-3-1; HV: 2.2; Time: 1/3/2020 4:00:25 AM)"=12670, "Automatic Update (DT: Olivine-3-1; HV: 2.2; Time: 1/3/2020 4:00:26 AM)"=12671, "Automatic Update (DT: Olivine-3-1; HV: 2.2; Time: 1/3/2020 4:00:27 AM)"=12672, "Automatic Update (DT: Olivine-3-1; HV: 2.2; Time: 1/3/2020 4:00:28 AM)"=12673, "Automatic Update (DT: Olivine-3-1; HV: 2.2; Time: 1/3/2020 4:00:29 AM)"=12674, "Automatic Update (DT: Olivine-3-1; HV: 2.2; Time: 1/3/2020 4:00:30 AM)"=12675, "Automatic Update (DT: Olivine-3-1; HV: 2.2; Time: 1/3/2020 4:00:31 AM)"=12676, "Automatic Update (DT: Olivine-3-1; HV: 2.2; Time: 1/3/2020 4:00:32 AM)"=12677, "Automatic Update (DT: Olivine-3-1; HV: 2.2; Time: 1/3/2020 4:00:33 AM)"=12678, "Automatic Update (DT: Olivine-3-1; HV: 2.2; Time: 1/3/2020 4:00:35 AM)"=12679, "Automatic Update (DT: Olivine-3-1; HV: 2.2; Time: 1/3/2020 4:00:36 AM)"=12680, "Automatic Update (DT: Olivine-3-1; HV: 2.2; Time: 1/3/2020 4:00:38 AM)"=12681, "Automatic Update (DT: Olivine-3-1; HV: 2.2; Time: 1/3/2020 4:00:39 AM)"=12682, "Automatic Update (DT: Olivine-3-1; HV: 2.2; Time: 1/3/2020 4:00:42 AM)"=12683, "Automatic Update (DT: Olivine-3-1; HV: 2.2; Time: 1/3/2020 4:00:43 AM)"=12684, "Automatic Update (DT: Olivine-3-1; HV: 2.2; Time: 1/3/2020 4:00:44 AM)"=12685, "Automatic Update (DT: Olivine-3-1; HV: 2.2; Time: 1/3/2020 4:00:45 AM)"=12686, "Automatic Update (DT: Olivine-3-1; HV: 2.2; Time: 1/3/2020 4:00:46 AM)"=12687, "Automatic Update (DT: Olivine-3-1; HV: 2.2; Time: 1/3/2020 4:00:47 AM)"=12688, "Automatic Update (DT: Olivine-3-1; HV: 2.2; Time: 1/3/2020 4:00:48 AM)"=12689, "Automatic Update (DT: Olivine-3-1; HV: 2.2; Time: 1/3/2020 4:00:49 AM)"=12690, "Automatic Update (DT: Olivine-3-1; HV: 2.2; Time: 1/3/2020 4:00:50 AM)"=12691, "Automatic Update (DT: Olivine-3-1; HV: 2.2; Time: 1/3/2020 4:00:51 AM)"=12692, "Automatic Update (DT: Olivine-3-1; HV: 2.2; Time: 1/3/2020 4:00:52 AM)"=12693, "Automatic Update (DT: Olivine-3-1; HV: 2.2; Time: 1/3/2020 4:00:53 AM)"=12694, "Automatic Update (DT: Olivine-3-1; HV: 2.2; Time: 1/3/2020 4:00:54 AM)"=12695, "Automatic Update (DT: Olivine-3-1; HV: 2.2; Time: 1/3/2020 4:00:55 AM)"=12696, "Automatic Update (DT: Olivine-3-1; HV: 2.2; Time: 1/3/2020 4:00:57 AM)"=12697, "Automatic Update (DT: Olivine-3-1; HV: 2.2; Time: 1/3/2020 4:00:58 AM)"=12698, "Automatic Update (DT: Olivine-3-1; HV: 2.2; Time: 1/3/2020 4:00:59 AM)"=12699, "Automatic Update (DT: Olivine-3-1; HV: 2.2; Time: 1/3/2020 4:01:00 AM)"=12700, "Automatic Update (DT: Olivine-3-1; HV: 2.2; Time: 1/3/2020 4:01:01 AM)"=12701, "Automatic Update (DT: Olivine-3-1; HV: 2.2; Time: 1/3/2020 4:01:03 AM)"=12702, "Automatic Update (DT: Olivine-3-1; HV: 2.2; Time: 1/3/2020 4:01:04 AM)"=12703, "Automatic Update (DT: Olivine-3-1; HV: 2.2; Time: 1/3/2020 4:01:05 AM)"=12704, "Automatic Update (DT: Olivine-3-1; HV: 2.2; Time: 1/3/2020 4:01:06 AM)"=12705, "Automatic Update (DT: Olivine-3-1; HV: 2.2; Time: 1/3/2020 4:01:08 AM)"=12706, "Automatic Update (DT: Olivine-3-1; HV: 2.2; Time: 1/3/2020 4:01:10 AM)"=12707, "Automatic Update (DT: Olivine-3-1; HV: 2.2; Time: 1/3/2020 4:01:11 AM)"=12708, "Automatic Update (DT: Olivine-3-1; HV: 2.2; Time: 1/3/2020 4:01:12 AM)"=12709, "Automatic Update (DT: Olivine-3-1; HV: 2.2; Time: 1/3/2020 4:01:13 AM)"=12710, "Automatic Update (DT: Olivine-3-1; HV: 2.2; Time: 1/3/2020 4:01:14 AM)"=12711, "Automatic Update (DT: Olivine-3-1; HV: 2.2; Time: 1/3/2020 4:01:15 AM)"=12712, "Automatic Update (DT: Olivine-3-1; HV: 2.2; Time: 1/3/2020 4:01:16 AM)"=12713, "Automatic Update (DT: Olivine-3-1; HV: 2.2; Time: 1/3/2020 4:01:17 AM)"=12714, "Automatic Update (DT: Olivine-3-1; HV: 2.2; Time: 1/3/2020 4:01:18 AM)"=12715, "Automatic Update (DT: Olivine-3-1; HV: 2.2; Time: 1/3/2020 4:01:19 AM)"=12716, "Automatic Update (DT: Olivine-3-1; HV: 2.2; Time: 1/3/2020 4:01:20 AM)"=12717, "Automatic Update (DT: Olivine-3-1; HV: 2.2; Time: 1/3/2020 4:01:21 AM)"=12718, "Automatic Update (DT: Olivine-3-1; HV: 2.2; Time: 1/3/2020 4:01:22 AM)"=12719, "Automatic Update (DT: Olivine-3-1; HV: 2.2; Time: 1/3/2020 4:01:23 AM)"=12720, "Automatic Update (DT: Olivine-3-1; HV: 2.2; Time: 1/3/2020 4:01:24 AM)"=12721, "Automatic Update (DT: Olivine-3-1; HV: 2.2; Time: 1/3/2020 4:01:27 AM)"=12722, "Automatic Update (DT: Olivine-3-1; HV: 2.2; Time: 1/3/2020 4:01:28 AM)"=12723, "Automatic Update (DT: Olivine-3-1; HV: 2.2; Time: 1/3/2020 4:01:29 AM)"=12724, "Automatic Update (DT: Olivine-3-1; HV: 2.2; Time: 1/3/2020 4:01:31 AM)"=12725, "Automatic Update (DT: Olivine-3-1; HV: 2.2; Time: 1/3/2020 4:01:32 AM)"=12726, "Automatic Update (DT: Olivine-3-1; HV: 2.2; Time: 1/3/2020 4:01:33 AM)"=12727, "Automatic Update (DT: Olivine-3-1; HV: 2.2; Time: 1/3/2020 4:01:34 AM)"=12728, "Automatic Update (DT: Olivine-3-1; HV: 2.2; Time: 1/3/2020 4:01:36 AM)"=12729, "Automatic Update (DT: Olivine-3-1; HV: 2.2; Time: 1/3/2020 4:01:38 AM)"=12730, "Automatic Update (DT: Olivine-3-1; HV: 2.2; Time: 1/3/2020 4:01:39 AM)"=12731, "Automatic Update (DT: Olivine-3-1; HV: 2.2; Time: 1/3/2020 4:01:40 AM)"=12732, "Automatic Update (DT: Olivine-3-1; HV: 2.2; Time: 1/3/2020 4:01:41 AM)"=12733, "Automatic Update (DT: Olivine-3-1; HV: 2.2; Time: 1/3/2020 4:01:42 AM)"=12734, "Automatic Update (DT: Olivine-3-1; HV: 2.2; Time: 1/3/2020 4:01:43 AM)"=12735, "Automatic Update (DT: Olivine-3-1; HV: 2.2; Time: 1/3/2020 4:01:44 AM)"=12736, "Automatic Update (DT: Olivine-3-1; HV: 2.2; Time: 1/3/2020 4:01:45 AM)"=12737, "Automatic Update (DT: Olivine-3-1; HV: 2.2; Time: 1/3/2020 4:01:46 AM)"=12738, "Automatic Update (DT: Olivine-3-1; HV: 2.2; Time: 1/3/2020 4:01:47 AM)"=12739, "Automatic Update (DT: Olivine-3-1; HV: 2.2; Time: 1/3/2020 4:01:48 AM)"=12740, "Automatic Update (DT: Olivine-3-1; HV: 2.2; Time: 1/3/2020 4:01:50 AM)"=12741, "Automatic Update (DT: Olivine-3-1; HV: 2.2; Time: 1/3/2020 4:01:51 AM)"=12742, "Automatic Update (DT: Olivine-3-1; HV: 2.2; Time: 1/3/2020 4:01:52 AM)"=12743, "Automatic Update (DT: Olivine-3-1; HV: 2.2; Time: 1/3/2020 4:01:53 AM)"=12744, "Automatic Update (DT: Olivine-3-1; HV: 2.2; Time: 1/3/2020 4:01:54 AM)"=12745, "Automatic Update (DT: Olivine-3-1; HV: 2.2; Time: 1/3/2020 4:01:55 AM)"=12746, "Automatic Update (DT: Olivine-3-1; HV: 2.2; Time: 1/3/2020 4:01:56 AM)"=12747, "Automatic Update (DT: Olivine-3-1; HV: 2.2; Time: 1/3/2020 4:01:57 AM)"=12748, "Automatic Update (DT: Olivine-3-1; HV: 2.2; Time: 1/3/2020 4:01:58 AM)"=12749, "Automatic Update (DT: Olivine-3-1; HV: 2.2; Time: 1/3/2020 4:01:59 AM)"=12750, "Automatic Update (DT: Olivine-3-1; HV: 2.2; Time: 1/3/2020 4:02:01 AM)"=12751, "Automatic Update (DT: Olivine-3-1; HV: 2.2; Time: 1/3/2020 4:02:02 AM)"=12752, "Automatic Update (DT: Olivine-3-1; HV: 2.2; Time: 1/3/2020 4:02:03 AM)"=12753, "Automatic Update (DT: Olivine-3-1; HV: 2.2; Time: 1/3/2020 4:02:04 AM)"=12754, "Automatic Update (DT: Olivine-3-1; HV: 2.2; Time: 1/3/2020 4:02:05 AM)"=12755, "Automatic Update (DT: Olivine-3-1; HV: 2.2; Time: 1/3/2020 4:02:06 AM)"=12756, "Automatic Update (DT: Olivine-3-1; HV: 2.2; Time: 1/3/2020 4:02:07 AM)"=12757, "Automatic Update (DT: Olivine-3-1; HV: 2.2; Time: 1/3/2020 4:02:08 AM)"=12758, "Automatic Update (DT: Olivine-3-1; HV: 2.2; Time: 1/3/2020 4:02:09 AM)"=12759, "Automatic Update (DT: Olivine-3-1; HV: 2.2; Time: 1/3/2020 4:02:10 AM)"=12760, "Automatic Update (DT: Olivine-3-1; HV: 2.2; Time: 1/3/2020 4:02:11 AM)"=12761, "Automatic Update (DT: Olivine-3-1; HV: 2.2; Time: 1/3/2020 4:02:13 AM)"=12762, "Automatic Update (DT: Olivine-3-1; HV: 2.2; Time: 1/3/2020 4:02:14 AM)"=12763, "Automatic Update (DT: Olivine-3-1; HV: 2.2; Time: 1/3/2020 4:02:15 AM)"=12764, "Automatic Update (DT: Olivine-3-1; HV: 2.2; Time: 1/3/2020 4:02:16 AM)"=12765, "Automatic Update (DT: Olivine-3-1; HV: 2.2; Time: 1/3/2020 4:02:17 AM)"=12766, "Automatic Update (DT: Olivine-3-1; HV: 2.2; Time: 1/3/2020 4:02:18 AM)"=12767, "Automatic Update (DT: Olivine-3-1; HV: 2.2; Time: 1/3/2020 4:02:19 AM)"=12768, "Automatic Update (DT: Olivine-3-1; HV: 2.2; Time: 1/3/2020 4:02:20 AM)"=12769, "Automatic Update (DT: Olivine-3-1; HV: 2.2; Time: 1/3/2020 4:02:21 AM)"=12770, "Automatic Update (DT: Olivine-3-1; HV: 2.2; Time: 1/3/2020 4:02:22 AM)"=12771, "Automatic Update (DT: Olivine-3-1; HV: 2.2; Time: 1/3/2020 4:02:23 AM)"=12772, "Automatic Update (DT: Olivine-3-1; HV: 2.2; Time: 1/3/2020 4:02:24 AM)"=12773, "Automatic Update (DT: Olivine-3-1; HV: 2.2; Time: 1/3/2020 4:02:25 AM)"=12774, "Automatic Update (DT: Olivine-3-1; HV: 2.2; Time: 1/3/2020 4:02:26 AM)"=12775, "Automatic Update (DT: Olivine-3-1; HV: 2.2; Time: 1/3/2020 4:02:27 AM)"=12776, "Automatic Update (DT: Olivine-3-1; HV: 2.2; Time: 1/3/2020 4:02:28 AM)"=12777, "Automatic Update (DT: Olivine-3-1; HV: 2.2; Time: 1/3/2020 4:02:29 AM)"=12778, "Automatic Update (DT: Olivine-3-1; HV: 2.2; Time: 1/3/2020 4:02:30 AM)"=12779, "Automatic Update (DT: Olivine-3-1; HV: 2.2; Time: 1/3/2020 4:02:31 AM)"=12780, "Automatic Update (DT: Olivine-3-1; HV: 2.2; Time: 1/3/2020 4:02:33 AM)"=12781, "Automatic Update (DT: Olivine-3-1; HV: 2.2; Time: 1/3/2020 4:02:34 AM)"=12782, "Automatic Update (DT: Olivine-3-1; HV: 2.2; Time: 1/3/2020 4:02:35 AM)"=12783, "Automatic Update (DT: Olivine-3-1; HV: 2.2; Time: 1/3/2020 4:02:36 AM)"=12784, "Automatic Update (DT: Olivine-3-1; HV: 2.2; Time: 1/3/2020 4:02:37 AM)"=12785, "Automatic Update (DT: Olivine-3-1; HV: 2.2; Time: 1/3/2020 4:02:38 AM)"=12786, "Automatic Update (DT: Olivine-3-1; HV: 2.2; Time: 1/3/2020 4:02:39 AM)"=12787, "Automatic Update (DT: Olivine-3-1; HV: 2.2; Time: 1/3/2020 4:02:40 AM)"=12788, "Automatic Update (DT: Olivine-3-1; HV: 2.2; Time: 1/3/2020 4:02:44 AM)"=12789, "Automatic Update (DT: Olivine-3-1; HV: 2.2; Time: 1/3/2020 4:02:45 AM)"=12790, "Automatic Update (DT: Olivine-3-1; HV: 2.2; Time: 1/3/2020 4:02:46 AM)"=12791, "Automatic Update (DT: Olivine-3-1; HV: 2.2; Time: 1/3/2020 4:02:47 AM)"=12792, "Automatic Update (DT: Olivine-3-1; HV: 2.2; Time: 1/3/2020 4:02:48 AM)"=12793, "Automatic Update (DT: Olivine-3-1; HV: 2.2; Time: 1/3/2020 4:02:49 AM)"=12794, "Automatic Update (DT: Olivine-3-1; HV: 2.2; Time: 1/3/2020 4:02:50 AM)"=12795, "Automatic Update (DT: Olivine-3-1; HV: 2.2; Time: 1/3/2020 4:02:51 AM)"=12796, "Automatic Update (DT: Olivine-3-1; HV: 2.2; Time: 1/3/2020 4:02:52 AM)"=12797, "Automatic Update (DT: Olivine-3-1; HV: 2.2; Time: 1/3/2020 4:02:53 AM)"=12798, "Automatic Update (DT: Olivine-3-1; HV: 2.2; Time: 1/3/2020 4:02:55 AM)"=12799, "Automatic Update (DT: Olivine-3-1; HV: 2.2; Time: 1/3/2020 4:02:56 AM)"=12800, "Automatic Update (DT: Olivine-3-1; HV: 2.2; Time: 1/3/2020 4:02:57 AM)"=12801, "Automatic Update (DT: Olivine-3-1; HV: 2.2; Time: 1/3/2020 4:02:58 AM)"=12802, "Automatic Update (DT: Olivine-3-1; HV: 2.2; Time: 1/3/2020 4:02:59 AM)"=12803, "Automatic Update (DT: Olivine-3-1; HV: 2.2; Time: 1/3/2020 4:03:00 AM)"=12804, "Automatic Update (DT: Olivine-3-1; HV: 2.2; Time: 1/3/2020 4:03:01 AM)"=12805, "Automatic Update (DT: Olivine-3-1; HV: 2.2; Time: 1/3/2020 4:03:02 AM)"=12806, "Automatic Update (DT: Olivine-3-1; HV: 2.2; Time: 1/3/2020 4:03:03 AM)"=12807, "Automatic Update (DT: Olivine-3-1; HV: 2.2; Time: 1/3/2020 4:03:04 AM)"=12808, "Automatic Update (DT: Olivine-3-1; HV: 2.2; Time: 1/3/2020 4:03:05 AM)"=12809, "Automatic Update (DT: Olivine-3-1; HV: 2.2; Time: 1/3/2020 4:03:06 AM)"=12810, "Automatic Update (DT: Olivine-3-1; HV: 2.2; Time: 1/3/2020 4:03:07 AM)"=12811, "Automatic Update (DT: Olivine-3-1; HV: 2.2; Time: 1/3/2020 4:03:08 AM)"=12812, "Automatic Update (DT: Olivine-3-1; HV: 2.2; Time: 1/3/2020 4:03:09 AM)"=12813, "Automatic Update (DT: Olivine-3-1; HV: 2.2; Time: 1/3/2020 4:03:10 AM)"=12814, "Automatic Update (DT: Olivine-3-1; HV: 2.2; Time: 1/3/2020 4:03:11 AM)"=12815, "Automatic Update (DT: Olivine-3-1; HV: 2.2; Time: 1/3/2020 4:03:12 AM)"=12816, "Automatic Update (DT: Olivine-3-1; HV: 2.2; Time: 1/3/2020 4:03:14 AM)"=12817, "Automatic Update (DT: Olivine-3-1; HV: 2.2; Time: 1/3/2020 4:03:15 AM)"=12818, "Automatic Update (DT: Olivine-3-1; HV: 2.2; Time: 1/3/2020 4:03:16 AM)"=12819, "Automatic Update (DT: Olivine-3-1; HV: 2.2; Time: 1/3/2020 4:03:17 AM)"=12820, "Automatic Update (DT: Olivine-3-1; HV: 2.2; Time: 1/3/2020 4:03:18 AM)"=12821, "Automatic Update (DT: Olivine-3-1; HV: 2.2; Time: 1/3/2020 4:03:19 AM)"=12822, "Automatic Update (DT: Olivine-3-1; HV: 2.2; Time: 1/3/2020 4:03:20 AM)"=12823, "Automatic Update (DT: Olivine-3-1; HV: 2.2; Time: 1/3/2020 4:03:21 AM)"=12824, "Automatic Update (DT: Olivine-3-1; HV: 2.2; Time: 1/3/2020 4:03:22 AM)"=12825, "Automatic Update (DT: Olivine-3-1; HV: 2.2; Time: 1/3/2020 4:03:23 AM)"=12826, "Automatic Update (DT: Olivine-3-1; HV: 2.2; Time: 1/3/2020 4:03:24 AM)"=12827, "Automatic Update (DT: Olivine-3-1; HV: 2.2; Time: 1/3/2020 4:03:25 AM)"=12828, "Automatic Update (DT: Olivine-3-1; HV: 2.2; Time: 1/3/2020 4:03:26 AM)"=12829, "Automatic Update (DT: Olivine-3-1; HV: 2.2; Time: 1/3/2020 4:03:27 AM)"=12830, "Automatic Update (DT: Olivine-3-1; HV: 2.2; Time: 1/3/2020 4:03:28 AM)"=12831, "Automatic Update (DT: Olivine-3-1; HV: 2.2; Time: 1/3/2020 4:03:29 AM)"=12832, "Automatic Update (DT: Olivine-3-1; HV: 2.2; Time: 1/3/2020 4:03:30 AM)"=12833, "Automatic Update (DT: Olivine-3-1; HV: 2.2; Time: 1/3/2020 4:03:31 AM)"=12834, "Automatic Update (DT: Olivine-3-1; HV: 2.2; Time: 1/3/2020 4:03:33 AM)"=12835, "Automatic Update (DT: Olivine-3-1; HV: 2.2; Time: 1/3/2020 4:03:34 AM)"=12836, "Automatic Update (DT: Olivine-3-1; HV: 2.2; Time: 1/3/2020 4:03:35 AM)"=12837, "Automatic Update (DT: Olivine-3-1; HV: 2.2; Time: 1/3/2020 4:03:36 AM)"=12838, "Automatic Update (DT: Olivine-3-1; HV: 2.2; Time: 1/3/2020 4:03:37 AM)"=12839, "Automatic Update (DT: Olivine-3-1; HV: 2.2; Time: 1/3/2020 4:03:38 AM)"=12840, "Automatic Update (DT: Olivine-3-1; HV: 2.2; Time: 1/3/2020 4:03:39 AM)"=12841, "Automatic Update (DT: Olivine-3-1; HV: 2.2; Time: 1/3/2020 4:03:40 AM)"=12842, "Automatic Update (DT: Olivine-3-1; HV: 2.2; Time: 1/3/2020 4:03:41 AM)"=12843, "Automatic Update (DT: Olivine-3-1; HV: 2.2; Time: 1/3/2020 4:03:42 AM)"=12844, "Automatic Update (DT: Olivine-3-1; HV: 2.2; Time: 1/3/2020 4:03:43 AM)"=12845, "Automatic Update (DT: Olivine-3-1; HV: 2.2; Time: 1/3/2020 4:03:44 AM)"=12846, "Automatic Update (DT: Olivine-3-1; HV: 2.2; Time: 1/3/2020 4:03:45 AM)"=12847, "Automatic Update (DT: Olivine-3-1; HV: 2.2; Time: 1/3/2020 4:03:46 AM)"=12848, "Automatic Update (DT: Olivine-3-1; HV: 2.2; Time: 1/3/2020 4:03:47 AM)"=12849, "Automatic Update (DT: Olivine-3-1; HV: 2.2; Time: 1/3/2020 4:03:48 AM)"=12850, "Automatic Update (DT: Olivine-3-1; HV: 2.2; Time: 1/3/2020 4:03:54 AM)"=12851, "Automatic Update (DT: Olivine-3-1; HV: 2.2; Time: 1/3/2020 4:03:55 AM)"=12852, "Automatic Update (DT: Olivine-3-1; HV: 2.2; Time: 1/3/2020 4:03:56 AM)"=12853, "Automatic Update (DT: Olivine-3-1; HV: 2.2; Time: 1/3/2020 4:04:05 AM)"=12854, "Automatic Update (DT: Olivine-3-1; HV: 2.2; Time: 1/3/2020 4:04:07 AM)"=12855, "Automatic Update (DT: Olivine-3-1; HV: 2.2; Time: 1/3/2020 4:04:08 AM)"=12856, "Automatic Update (DT: Olivine-3-1; HV: 2.2; Time: 1/3/2020 4:04:10 AM)"=12857, "Automatic Update (DT: Olivine-3-1; HV: 2.2; Time: 1/3/2020 4:04:11 AM)"=12858, "Automatic Update (DT: Olivine-3-1; HV: 2.2; Time: 1/3/2020 4:04:12 AM)"=12859, "Automatic Update (DT: Olivine-3-1; HV: 2.2; Time: 1/3/2020 4:04:13 AM)"=12860, "Automatic Update (DT: Olivine-3-1; HV: 2.2; Time: 1/3/2020 4:04:14 AM)"=12861, "Automatic Update (DT: Olivine-3-1; HV: 2.2; Time: 1/3/2020 4:04:15 AM)"=12862, "Automatic Update (DT: Olivine-3-1; HV: 2.2; Time: 1/3/2020 4:04:17 AM)"=12863, "Automatic Update (DT: Olivine-3-1; HV: 2.2; Time: 1/3/2020 4:04:18 AM)"=12864, "Automatic Update (DT: Olivine-3-1; HV: 2.2; Time: 1/3/2020 4:04:19 AM)"=12865, "Automatic Update (DT: Olivine-3-1; HV: 2.2; Time: 1/3/2020 4:04:20 AM)"=12866, "Automatic Update (DT: Olivine-3-1; HV: 2.2; Time: 1/3/2020 4:04:21 AM)"=12867, "Automatic Update (DT: Olivine-3-1; HV: 2.2; Time: 1/3/2020 4:04:22 AM)"=12868, "Automatic Update (DT: Olivine-3-1; HV: 2.2; Time: 1/3/2020 4:04:23 AM)"=12869, "Automatic Update (DT: Olivine-3-1; HV: 2.2; Time: 1/3/2020 4:04:24 AM)"=12870, "Automatic Update (DT: Olivine-3-1; HV: 2.2; Time: 1/3/2020 4:04:25 AM)"=12871, "Automatic Update (DT: Olivine-3-1; HV: 2.2; Time: 1/3/2020 4:04:27 AM)"=12872, "Automatic Update (DT: Olivine-3-1; HV: 2.2; Time: 1/3/2020 4:04:28 AM)"=12873, "Automatic Update (DT: Olivine-3-1; HV: 2.2; Time: 1/3/2020 4:04:29 AM)"=12874, "Automatic Update (DT: Olivine-3-1; HV: 2.2; Time: 1/3/2020 4:04:31 AM)"=12875, "Automatic Update (DT: Olivine-3-1; HV: 2.2; Time: 1/3/2020 4:04:32 AM)"=12876, "Automatic Update (DT: Olivine-3-1; HV: 2.2; Time: 1/3/2020 4:04:34 AM)"=12877, "Automatic Update (DT: Olivine-3-1; HV: 2.2; Time: 1/3/2020 4:04:35 AM)"=12878, "Automatic Update (DT: Olivine-3-1; HV: 2.2; Time: 1/3/2020 4:04:36 AM)"=12879, "Automatic Update (DT: Olivine-3-1; HV: 2.2; Time: 1/3/2020 4:04:37 AM)"=12880, "Automatic Update (DT: Olivine-3-1; HV: 2.2; Time: 1/3/2020 4:04:38 AM)"=12881, "Automatic Update (DT: Olivine-3-1; HV: 2.2; Time: 1/3/2020 4:04:40 AM)"=12882, "Automatic Update (DT: Olivine-3-1; HV: 2.2; Time: 1/3/2020 4:04:41 AM)"=12883, "Automatic Update (DT: Olivine-3-1; HV: 2.2; Time: 1/3/2020 4:04:42 AM)"=12884, "Automatic Update (DT: Olivine-3-1; HV: 2.2; Time: 1/3/2020 4:04:43 AM)"=12885, "Automatic Update (DT: Olivine-3-1; HV: 2.2; Time: 1/3/2020 4:04:44 AM)"=12886, "Automatic Update (DT: Olivine-3-1; HV: 2.2; Time: 1/3/2020 4:04:46 AM)"=12887, "Automatic Update (DT: Olivine-3-1; HV: 2.2; Time: 1/3/2020 4:04:47 AM)"=12888, "Automatic Update (DT: Olivine-3-1; HV: 2.2; Time: 1/3/2020 4:04:49 AM)"=12889, "Automatic Update (DT: Olivine-3-1; HV: 2.2; Time: 1/3/2020 4:04:50 AM)"=12890, "Automatic Update (DT: Olivine-3-1; HV: 2.2; Time: 1/3/2020 4:04:52 AM)"=12891, "Automatic Update (DT: Olivine-3-1; HV: 2.2; Time: 1/3/2020 4:05:03 AM)"=12892, "Automatic Update (DT: Olivine-3-1; HV: 2.2; Time: 1/3/2020 4:05:04 AM)"=12893, "Automatic Update (DT: Olivine-3-1; HV: 2.2; Time: 1/3/2020 4:05:05 AM)"=12894, "Automatic Update (DT: Olivine-3-1; HV: 2.2; Time: 1/3/2020 4:05:07 AM)"=12895, "Automatic Update (DT: Olivine-3-1; HV: 2.2; Time: 1/3/2020 4:05:08 AM)"=12896, "Automatic Update (DT: Olivine-3-1; HV: 2.2; Time: 1/3/2020 4:05:09 AM)"=12897, "Automatic Update (DT: Olivine-3-1; HV: 2.2; Time: 1/3/2020 4:05:13 AM)"=12898, "Automatic Update (DT: Olivine-3-1; HV: 2.2; Time: 1/3/2020 4:05:17 AM)"=12899, "Automatic Update (DT: Olivine-3-1; HV: 2.2; Time: 1/3/2020 4:05:18 AM)"=12900, "Automatic Update (DT: Olivine-3-1; HV: 2.2; Time: 1/3/2020 4:05:24 AM)"=12901, "Automatic Update (DT: Olivine-3-1; HV: 2.2; Time: 1/3/2020 4:05:26 AM)"=12902, "Automatic Update (DT: Olivine-3-1; HV: 2.2; Time: 1/3/2020 4:05:29 AM)"=12903, "Automatic Update (DT: Olivine-3-1; HV: 2.2; Time: 1/3/2020 4:05:31 AM)"=12904, "Automatic Update (DT: Olivine-3-1; HV: 2.2; Time: 1/3/2020 4:05:32 AM)"=12905, "Automatic Update (DT: Olivine-3-1; HV: 2.2; Time: 1/3/2020 4:05:33 AM)"=12906, "Automatic Update (DT: Olivine-3-1; HV: 2.2; Time: 1/3/2020 4:05:38 AM)"=12907, "Automatic Update (DT: Olivine-3-1; HV: 2.2; Time: 1/3/2020 4:05:39 AM)"=12908, "Automatic Update (DT: Olivine-3-1; HV: 2.2; Time: 1/3/2020 4:05:42 AM)"=12909, "Automatic Update (DT: Olivine-3-1; HV: 2.2; Time: 1/3/2020 4:05:45 AM)"=12910, "Automatic Update (DT: Olivine-3-1; HV: 2.2; Time: 1/3/2020 4:05:46 AM)"=12911, "Automatic Update (DT: Olivine-3-1; HV: 2.2; Time: 1/3/2020 4:05:47 AM)"=12912, "Automatic Update (DT: Olivine-3-1; HV: 2.2; Time: 1/3/2020 4:05:55 AM)"=12913, "Automatic Update (DT: Olivine-3-1; HV: 2.2; Time: 1/3/2020 4:05:56 AM)"=12914, "Automatic Update (DT: Olivine-3-1; HV: 2.2; Time: 1/3/2020 4:05:58 AM)"=12915, "Automatic Update (DT: Olivine-3-1; HV: 2.2; Time: 1/3/2020 4:06:00 AM)"=12916, "Automatic Update (DT: Olivine-3-1; HV: 2.2; Time: 1/3/2020 4:06:01 AM)"=12917, "Automatic Update (DT: Olivine-3-1; HV: 2.2; Time: 1/3/2020 4:06:02 AM)"=12918, "Automatic Update (DT: Olivine-3-1; HV: 2.2; Time: 1/3/2020 4:06:03 AM)"=12919, "Automatic Update (DT: Olivine-3-1; HV: 2.2; Time: 1/3/2020 4:06:04 AM)"=12920, "Automatic Update (DT: Olivine-3-1; HV: 2.2; Time: 1/3/2020 4:06:05 AM)"=12921, "Automatic Update (DT: Olivine-3-1; HV: 2.2; Time: 1/3/2020 4:06:06 AM)"=12922, "Automatic Update (DT: Olivine-3-1; HV: 2.2; Time: 1/3/2020 4:06:07 AM)"=12923, "Automatic Update (DT: Olivine-3-1; HV: 2.2; Time: 1/3/2020 4:06:08 AM)"=12924, "Automatic Update (DT: Olivine-3-1; HV: 2.2; Time: 1/3/2020 4:06:09 AM)"=12925, "Automatic Update (DT: Olivine-3-1; HV: 2.2; Time: 1/3/2020 4:06:10 AM)"=12926, "Automatic Update (DT: Olivine-3-1; HV: 2.2; Time: 1/3/2020 4:06:11 AM)"=12927, "Automatic Update (DT: Olivine-3-1; HV: 2.2; Time: 1/3/2020 4:06:12 AM)"=12928, "Automatic Update (DT: Olivine-3-1; HV: 2.2; Time: 1/3/2020 4:06:14 AM)"=12929, "Automatic Update (DT: Olivine-3-1; HV: 2.2; Time: 1/3/2020 4:06:15 AM)"=12930, "Automatic Update (DT: Olivine-3-1; HV: 2.2; Time: 1/3/2020 4:06:16 AM)"=12931, "Automatic Update (DT: Olivine-3-1; HV: 2.2; Time: 1/3/2020 4:06:17 AM)"=12932, "Automatic Update (DT: Olivine-3-1; HV: 2.2; Time: 1/3/2020 4:06:18 AM)"=12933, "Automatic Update (DT: Olivine-3-1; HV: 2.2; Time: 1/3/2020 4:06:19 AM)"=12934, "Automatic Update (DT: Olivine-3-1; HV: 2.2; Time: 1/3/2020 4:06:21 AM)"=12935, "Automatic Update (DT: Olivine-3-1; HV: 2.2; Time: 1/3/2020 4:06:22 AM)"=12936, "Automatic Update (DT: Olivine-3-1; HV: 2.2; Time: 1/3/2020 4:06:27 AM)"=12937, "Automatic Update (DT: Olivine-3-1; HV: 2.2; Time: 1/3/2020 4:06:28 AM)"=12938, "Automatic Update (DT: Olivine-3-1; HV: 2.2; Time: 1/3/2020 4:06:29 AM)"=12939, "Automatic Update (DT: Olivine-3-1; HV: 2.2; Time: 1/3/2020 4:06:30 AM)"=12940, "Automatic Update (DT: Olivine-3-1; HV: 2.2; Time: 1/3/2020 4:06:31 AM)"=12941, "Automatic Update (DT: Olivine-3-1; HV: 2.2; Time: 1/3/2020 4:06:32 AM)"=12942, "Automatic Update (DT: Olivine-3-1; HV: 2.2; Time: 1/3/2020 4:06:33 AM)"=12943, "Automatic Update (DT: Olivine-3-1; HV: 2.2; Time: 1/3/2020 4:06:34 AM)"=12944, "Automatic Update (DT: Olivine-3-1; HV: 2.2; Time: 1/3/2020 4:06:35 AM)"=12945, "Automatic Update (DT: Olivine-3-1; HV: 2.2; Time: 1/3/2020 4:06:36 AM)"=12946, "Automatic Update (DT: Olivine-3-1; HV: 2.2; Time: 1/3/2020 4:06:37 AM)"=12947, "Automatic Update (DT: Olivine-3-1; HV: 2.2; Time: 1/3/2020 4:06:38 AM)"=12948, "Automatic Update (DT: Olivine-3-1; HV: 2.2; Time: 1/3/2020 4:06:41 AM)"=12949, "Automatic Update (DT: Olivine-3-1; HV: 2.2; Time: 1/3/2020 4:06:42 AM)"=12950, "Automatic Update (DT: Olivine-3-1; HV: 2.2; Time: 1/3/2020 4:06:43 AM)"=12951, "Automatic Update (DT: Olivine-3-1; HV: 2.2; Time: 1/3/2020 4:06:44 AM)"=12952, "Automatic Update (DT: Olivine-3-1; HV: 2.2; Time: 1/3/2020 4:06:45 AM)"=12953, "Automatic Update (DT: Olivine-3-1; HV: 2.2; Time: 1/3/2020 4:06:46 AM)"=12954, "Automatic Update (DT: Olivine-3-1; HV: 2.2; Time: 1/3/2020 4:06:47 AM)"=12955, "Automatic Update (DT: Olivine-3-1; HV: 2.2; Time: 1/3/2020 4:06:48 AM)"=12956, "Automatic Update (DT: Olivine-3-1; HV: 2.2; Time: 1/3/2020 4:06:50 AM)"=12957, "Automatic Update (DT: Olivine-3-1; HV: 2.2; Time: 1/3/2020 4:06:51 AM)"=12958, "Automatic Update (DT: Olivine-3-1; HV: 2.2; Time: 1/3/2020 4:06:52 AM)"=12959, "Automatic Update (DT: Olivine-3-1; HV: 2.2; Time: 1/3/2020 4:06:53 AM)"=12960, "Automatic Update (DT: Olivine-3-1; HV: 2.2; Time: 1/3/2020 4:06:54 AM)"=12961, "Automatic Update (DT: Olivine-3-1; HV: 2.2; Time: 1/3/2020 4:06:55 AM)"=12962, "Automatic Update (DT: Olivine-3-1; HV: 2.2; Time: 1/3/2020 4:06:56 AM)"=12963, "Automatic Update (DT: Olivine-3-1; HV: 2.2; Time: 1/3/2020 4:06:57 AM)"=12964, "Automatic Update (DT: Olivine-3-1; HV: 2.2; Time: 1/3/2020 4:06:58 AM)"=12965, "Automatic Update (DT: Olivine-3-1; HV: 2.2; Time: 1/3/2020 4:06:59 AM)"=12966, "Automatic Update (DT: Olivine-3-1; HV: 2.2; Time: 1/3/2020 4:07:00 AM)"=12967, "Automatic Update (DT: Olivine-3-1; HV: 2.2; Time: 1/3/2020 4:07:01 AM)"=12968, "Automatic Update (DT: Olivine-3-1; HV: 2.2; Time: 1/3/2020 4:07:02 AM)"=12969, "Automatic Update (DT: Olivine-3-1; HV: 2.2; Time: 1/3/2020 4:07:03 AM)"=12970, "Automatic Update (DT: Olivine-3-1; HV: 2.2; Time: 1/3/2020 4:07:04 AM)"=12971, "Automatic Update (DT: Olivine-3-1; HV: 2.2; Time: 1/3/2020 4:07:05 AM)"=12972, "Automatic Update (DT: Olivine-3-1; HV: 2.2; Time: 1/3/2020 4:07:06 AM)"=12973, "Automatic Update (DT: Olivine-3-1; HV: 2.2; Time: 1/3/2020 4:07:07 AM)"=12974, "Automatic Update (DT: Olivine-3-1; HV: 2.2; Time: 1/3/2020 4:07:08 AM)"=12975, "Automatic Update (DT: Olivine-3-1; HV: 2.2; Time: 1/3/2020 4:07:13 AM)"=12976, "Automatic Update (DT: Olivine-3-1; HV: 2.2; Time: 1/3/2020 4:07:15 AM)"=12977, "Automatic Update (DT: Olivine-3-1; HV: 2.2; Time: 1/3/2020 4:07:16 AM)"=12978, "Automatic Update (DT: Olivine-3-1; HV: 2.2; Time: 1/3/2020 4:07:19 AM)"=12979, "Automatic Update (DT: Olivine-3-1; HV: 2.2; Time: 1/3/2020 4:07:20 AM)"=12980, "Automatic Update (DT: Olivine-3-1; HV: 2.2; Time: 1/3/2020 4:07:21 AM)"=12981, "Automatic Update (DT: Olivine-3-1; HV: 2.2; Time: 1/3/2020 4:07:22 AM)"=12982, "Automatic Update (DT: Olivine-3-1; HV: 2.2; Time: 1/3/2020 4:07:23 AM)"=12983, "Automatic Update (DT: Olivine-3-1; HV: 2.2; Time: 1/3/2020 4:07:24 AM)"=12984, "Automatic Update (DT: Olivine-3-1; HV: 2.2; Time: 1/3/2020 4:07:25 AM)"=12985, "Automatic Update (DT: Olivine-3-1; HV: 2.2; Time: 1/3/2020 4:07:26 AM)"=12986, "Automatic Update (DT: Olivine-3-1; HV: 2.2; Time: 1/3/2020 4:07:27 AM)"=12987, "Automatic Update (DT: Olivine-3-1; HV: 2.2; Time: 1/3/2020 4:07:29 AM)"=12988, "Automatic Update (DT: Olivine-3-1; HV: 2.2; Time: 1/3/2020 4:07:30 AM)"=12989, "Automatic Update (DT: Olivine-3-1; HV: 2.2; Time: 1/3/2020 4:07:31 AM)"=12990, "Automatic Update (DT: Olivine-3-1; HV: 2.2; Time: 1/3/2020 4:07:32 AM)"=12991, "Automatic Update (DT: Olivine-3-1; HV: 2.2; Time: 1/3/2020 4:07:33 AM)"=12992, "Automatic Update (DT: Olivine-3-1; HV: 2.2; Time: 1/3/2020 4:07:34 AM)"=12993, "Automatic Update (DT: Olivine-3-1; HV: 2.2; Time: 1/3/2020 4:07:35 AM)"=12994, "Automatic Update (DT: Olivine-3-1; HV: 2.2; Time: 1/3/2020 4:07:36 AM)"=12995, "Automatic Update (DT: Olivine-3-1; HV: 2.2; Time: 1/3/2020 4:07:37 AM)"=12996, "Automatic Update (DT: Olivine-3-1; HV: 2.2; Time: 1/3/2020 4:07:39 AM)"=12997, "Automatic Update (DT: Olivine-3-1; HV: 2.2; Time: 1/3/2020 4:07:40 AM)"=12998, "Automatic Update (DT: Olivine-3-1; HV: 2.2; Time: 1/3/2020 4:07:41 AM)"=12999, "Automatic Update (DT: Olivine-3-1; HV: 2.2; Time: 1/3/2020 4:07:42 AM)"=13000, "Automatic Update (DT: Olivine-3-1; HV: 2.2; Time: 1/3/2020 4:07:44 AM)"=13001, "Automatic Update (DT: Olivine-3-1; HV: 2.2; Time: 1/3/2020 4:07:45 AM)"=13002, "Automatic Update (DT: Olivine-3-1; HV: 2.2; Time: 1/3/2020 4:07:46 AM)"=13003, "Automatic Update (DT: Olivine-3-1; HV: 2.2; Time: 1/3/2020 4:07:47 AM)"=13004, "Automatic Update (DT: Olivine-3-1; HV: 2.2; Time: 1/3/2020 4:07:48 AM)"=13005, "Automatic Update (DT: Olivine-3-1; HV: 2.2; Time: 1/3/2020 4:07:49 AM)"=13006, "Automatic Update (DT: Olivine-3-1; HV: 2.2; Time: 1/3/2020 4:07:50 AM)"=13007, "Automatic Update (DT: Olivine-3-1; HV: 2.2; Time: 1/3/2020 4:07:51 AM)"=13008, "Automatic Update (DT: Olivine-3-1; HV: 2.2; Time: 1/3/2020 4:07:52 AM)"=13009, "Automatic Update (DT: Olivine-3-1; HV: 2.2; Time: 1/3/2020 4:07:53 AM)"=13010, "Automatic Update (DT: Olivine-3-1; HV: 2.2; Time: 1/3/2020 4:07:54 AM)"=13011, "Automatic Update (DT: Olivine-3-1; HV: 2.2; Time: 1/3/2020 4:07:55 AM)"=13012, "Automatic Update (DT: Olivine-3-1; HV: 2.2; Time: 1/3/2020 4:07:56 AM)"=13013, "Automatic Update (DT: Olivine-3-1; HV: 2.2; Time: 1/3/2020 4:07:57 AM)"=13014, "Automatic Update (DT: Olivine-3-1; HV: 2.2; Time: 1/3/2020 4:07:58 AM)"=13015, "Automatic Update (DT: Olivine-3-1; HV: 2.2; Time: 1/3/2020 4:07:59 AM)"=13016, "Automatic Update (DT: Olivine-3-1; HV: 2.2; Time: 1/3/2020 4:08:00 AM)"=13017, "Automatic Update (DT: Olivine-3-1; HV: 2.2; Time: 1/3/2020 4:08:01 AM)"=13018, "Automatic Update (DT: Olivine-3-1; HV: 2.2; Time: 1/3/2020 4:08:04 AM)"=13019, "Automatic Update (DT: Olivine-3-1; HV: 2.2; Time: 1/3/2020 4:08:05 AM)"=13020, "Automatic Update (DT: Olivine-3-1; HV: 2.2; Time: 1/3/2020 4:08:07 AM)"=13021, "Automatic Update (DT: Olivine-3-1; HV: 2.2; Time: 1/3/2020 4:08:08 AM)"=13022, "Automatic Update (DT: Olivine-3-1; HV: 2.2; Time: 1/3/2020 4:08:09 AM)"=13023, "Automatic Update (DT: Olivine-3-1; HV: 2.2; Time: 1/3/2020 4:08:10 AM)"=13024, "Automatic Update (DT: Olivine-3-1; HV: 2.2; Time: 1/3/2020 4:08:12 AM)"=13025, "Automatic Update (DT: Olivine-3-1; HV: 2.2; Time: 1/3/2020 4:08:13 AM)"=13026, "Automatic Update (DT: Olivine-3-1; HV: 2.2; Time: 1/3/2020 4:08:14 AM)"=13027, "Automatic Update (DT: Olivine-3-1; HV: 2.2; Time: 1/3/2020 4:08:15 AM)"=13028, "Automatic Update (DT: Olivine-3-1; HV: 2.2; Time: 1/3/2020 4:08:16 AM)"=13029, "Automatic Update (DT: Olivine-3-1; HV: 2.2; Time: 1/3/2020 4:08:17 AM)"=13030, "Automatic Update (DT: Olivine-3-1; HV: 2.2; Time: 1/3/2020 4:08:18 AM)"=13031, "Automatic Update (DT: Olivine-3-1; HV: 2.2; Time: 1/3/2020 4:08:19 AM)"=13032, "Automatic Update (DT: Olivine-3-1; HV: 2.2; Time: 1/3/2020 4:08:20 AM)"=13033, "Automatic Update (DT: Olivine-3-1; HV: 2.2; Time: 1/3/2020 4:08:23 AM)"=13034, "Automatic Update (DT: Olivine-3-1; HV: 2.2; Time: 1/3/2020 4:08:24 AM)"=13035, "Automatic Update (DT: Olivine-3-1; HV: 2.2; Time: 1/3/2020 4:08:25 AM)"=13036, "Automatic Update (DT: Olivine-3-1; HV: 2.2; Time: 1/3/2020 4:08:26 AM)"=13037, "Automatic Update (DT: Olivine-3-1; HV: 2.2; Time: 1/3/2020 4:08:27 AM)"=13038, "Automatic Update (DT: Olivine-3-1; HV: 2.2; Time: 1/3/2020 4:08:33 AM)"=13039, "Automatic Update (DT: Olivine-3-1; HV: 2.2; Time: 1/3/2020 4:08:34 AM)"=13040, "Automatic Update (DT: Olivine-3-1; HV: 2.2; Time: 1/3/2020 4:08:35 AM)"=13041, "Automatic Update (DT: Olivine-3-1; HV: 2.2; Time: 1/3/2020 4:08:36 AM)"=13042, "Automatic Update (DT: Olivine-3-1; HV: 2.2; Time: 1/3/2020 4:08:38 AM)"=13043, "Automatic Update (DT: Olivine-3-1; HV: 2.2; Time: 1/3/2020 4:08:40 AM)"=13044, "Automatic Update (DT: Olivine-3-1; HV: 2.2; Time: 1/3/2020 4:08:42 AM)"=13045, "Automatic Update (DT: Olivine-3-1; HV: 2.2; Time: 1/3/2020 4:08:44 AM)"=13046, "Automatic Update (DT: Olivine-3-1; HV: 2.2; Time: 1/3/2020 4:08:45 AM)"=13047, "Automatic Update (DT: Olivine-3-1; HV: 2.2; Time: 1/3/2020 4:08:47 AM)"=13048, "Automatic Update (DT: Olivine-3-1; HV: 2.2; Time: 1/3/2020 4:08:48 AM)"=13049, "Automatic Update (DT: Olivine-3-1; HV: 2.2; Time: 1/3/2020 4:08:50 AM)"=13050, "Automatic Update (DT: Olivine-3-1; HV: 2.2; Time: 1/3/2020 4:08:51 AM)"=13051, "Automatic Update (DT: Olivine-3-1; HV: 2.2; Time: 1/3/2020 4:08:53 AM)"=13052, "Automatic Update (DT: Olivine-3-1; HV: 2.2; Time: 1/3/2020 4:08:54 AM)"=13053, "Automatic Update (DT: Olivine-3-1; HV: 2.2; Time: 1/3/2020 4:08:55 AM)"=13054, "Automatic Update (DT: Olivine-3-1; HV: 2.2; Time: 1/3/2020 4:08:56 AM)"=13055, "Automatic Update (DT: Olivine-3-1; HV: 2.2; Time: 1/3/2020 4:08:57 AM)"=13056, "Automatic Update (DT: Olivine-3-1; HV: 2.2; Time: 1/3/2020 4:08:58 AM)"=13057, "Automatic Update (DT: Olivine-3-1; HV: 2.2; Time: 1/3/2020 4:08:59 AM)"=13058, "Automatic Update (DT: Olivine-3-1; HV: 2.2; Time: 1/3/2020 4:09:01 AM)"=13059, "Automatic Update (DT: Olivine-3-1; HV: 2.2; Time: 1/3/2020 4:09:02 AM)"=13060, "Automatic Update (DT: Olivine-3-1; HV: 2.2; Time: 1/3/2020 4:09:03 AM)"=13061, "Automatic Update (DT: Olivine-3-1; HV: 2.2; Time: 1/3/2020 4:09:04 AM)"=13062, "Automatic Update (DT: Olivine-3-1; HV: 2.2; Time: 1/3/2020 4:09:05 AM)"=13063, "Automatic Update (DT: Olivine-3-1; HV: 2.2; Time: 1/3/2020 4:09:06 AM)"=13064, "Automatic Update (DT: Olivine-3-1; HV: 2.2; Time: 1/3/2020 4:09:07 AM)"=13065, "Automatic Update (DT: Olivine-3-1; HV: 2.2; Time: 1/3/2020 4:09:08 AM)"=13066, "Automatic Update (DT: Olivine-3-1; HV: 2.2; Time: 1/3/2020 4:09:09 AM)"=13067, "Automatic Update (DT: Olivine-3-1; HV: 2.2; Time: 1/3/2020 4:09:10 AM)"=13068, "Automatic Update (DT: Olivine-3-1; HV: 2.2; Time: 1/3/2020 4:09:11 AM)"=13069, "Automatic Update (DT: Olivine-3-1; HV: 2.2; Time: 1/3/2020 4:09:12 AM)"=13070, "Automatic Update (DT: Olivine-3-1; HV: 2.2; Time: 1/3/2020 4:09:13 AM)"=13071, "Automatic Update (DT: Olivine-3-1; HV: 2.2; Time: 1/3/2020 4:09:14 AM)"=13072, "Automatic Update (DT: Olivine-3-1; HV: 2.2; Time: 1/3/2020 4:09:15 AM)"=13073, "Automatic Update (DT: Olivine-3-1; HV: 2.2; Time: 1/3/2020 4:09:16 AM)"=13074, "Automatic Update (DT: Olivine-3-1; HV: 2.2; Time: 1/3/2020 4:09:17 AM)"=13075, "Automatic Update (DT: Olivine-3-1; HV: 2.2; Time: 1/3/2020 4:09:18 AM)"=13076, "Automatic Update (DT: Olivine-3-1; HV: 2.2; Time: 1/3/2020 4:09:19 AM)"=13077, "Automatic Update (DT: Olivine-3-1; HV: 2.2; Time: 1/3/2020 4:09:20 AM)"=13078, "Automatic Update (DT: Olivine-3-1; HV: 2.2; Time: 1/3/2020 4:09:22 AM)"=13079, "Automatic Update (DT: Olivine-3-1; HV: 2.2; Time: 1/3/2020 4:09:24 AM)"=13080, "Automatic Update (DT: Olivine-3-1; HV: 2.2; Time: 1/3/2020 4:09:25 AM)"=13081, "Automatic Update (DT: Olivine-3-1; HV: 2.2; Time: 1/3/2020 4:09:26 AM)"=13082, "Automatic Update (DT: Olivine-3-1; HV: 2.2; Time: 1/3/2020 4:09:27 AM)"=13083, "Automatic Update (DT: Olivine-3-1; HV: 2.2; Time: 1/3/2020 4:09:28 AM)"=13084, "Automatic Update (DT: Olivine-3-1; HV: 2.2; Time: 1/3/2020 4:09:29 AM)"=13085, "Automatic Update (DT: Olivine-3-1; HV: 2.2; Time: 1/3/2020 4:09:30 AM)"=13086, "Automatic Update (DT: Olivine-3-1; HV: 2.2; Time: 1/3/2020 4:09:31 AM)"=13087, "Automatic Update (DT: Olivine-3-1; HV: 2.2; Time: 1/3/2020 4:09:32 AM)"=13088, "Automatic Update (DT: Olivine-3-1; HV: 2.2; Time: 1/3/2020 4:09:34 AM)"=13089, "Automatic Update (DT: Olivine-3-1; HV: 2.2; Time: 1/3/2020 4:09:35 AM)"=13090, "Automatic Update (DT: Olivine-3-1; HV: 2.2; Time: 1/3/2020 4:09:36 AM)"=13091, "Automatic Update (DT: Olivine-3-1; HV: 2.2; Time: 1/3/2020 4:09:37 AM)"=13092, "Automatic Update (DT: Olivine-3-1; HV: 2.2; Time: 1/3/2020 4:09:38 AM)"=13093, "Automatic Update (DT: Olivine-3-1; HV: 2.2; Time: 1/3/2020 4:09:39 AM)"=13094, "Automatic Update (DT: Olivine-3-1; HV: 2.2; Time: 1/3/2020 4:09:40 AM)"=13095, "Automatic Update (DT: Olivine-3-1; HV: 2.2; Time: 1/3/2020 4:09:41 AM)"=13096, "Automatic Update (DT: Olivine-3-1; HV: 2.2; Time: 1/3/2020 4:09:42 AM)"=13097, "Automatic Update (DT: Olivine-3-1; HV: 2.2; Time: 1/3/2020 4:09:43 AM)"=13098, "Automatic Update (DT: Olivine-3-1; HV: 2.2; Time: 1/3/2020 4:09:44 AM)"=13099, "Automatic Update (DT: Olivine-3-1; HV: 2.2; Time: 1/3/2020 4:09:46 AM)"=13100, "Automatic Update (DT: Olivine-3-1; HV: 2.2; Time: 1/3/2020 4:09:47 AM)"=13101, "Automatic Update (DT: Olivine-3-1; HV: 2.2; Time: 1/3/2020 4:09:48 AM)"=13102, "Automatic Update (DT: Olivine-3-1; HV: 2.2; Time: 1/3/2020 4:09:49 AM)"=13103, "Automatic Update (DT: Olivine-3-1; HV: 2.2; Time: 1/3/2020 4:09:50 AM)"=13104, "Automatic Update (DT: Olivine-3-1; HV: 2.2; Time: 1/3/2020 4:09:51 AM)"=13105, "Automatic Update (DT: Olivine-3-1; HV: 2.2; Time: 1/3/2020 4:09:52 AM)"=13106, "Automatic Update (DT: Olivine-3-1; HV: 2.2; Time: 1/3/2020 4:09:53 AM)"=13107, "Automatic Update (DT: Olivine-3-1; HV: 2.2; Time: 1/3/2020 4:09:54 AM)"=13108, "Automatic Update (DT: Olivine-3-1; HV: 2.2; Time: 1/3/2020 4:09:55 AM)"=13109, "Automatic Update (DT: Olivine-3-1; HV: 2.2; Time: 1/3/2020 4:09:56 AM)"=13110, "Automatic Update (DT: Olivine-3-1; HV: 2.2; Time: 1/3/2020 4:09:57 AM)"=13111, "Automatic Update (DT: Olivine-3-1; HV: 2.2; Time: 1/3/2020 4:09:58 AM)"=13112, "Automatic Update (DT: Olivine-3-1; HV: 2.2; Time: 1/3/2020 4:09:59 AM)"=13113, "Automatic Update (DT: Olivine-3-1; HV: 2.2; Time: 1/3/2020 4:10:00 AM)"=13114, "Automatic Update (DT: Olivine-3-1; HV: 2.2; Time: 1/3/2020 4:10:01 AM)"=13115, "Automatic Update (DT: Olivine-3-1; HV: 2.2; Time: 1/3/2020 4:10:02 AM)"=13116, "Automatic Update (DT: Olivine-3-1; HV: 2.2; Time: 1/3/2020 4:10:03 AM)"=13117, "Automatic Update (DT: Olivine-3-1; HV: 2.2; Time: 1/3/2020 4:10:04 AM)"=13118, "Automatic Update (DT: Olivine-3-1; HV: 2.2; Time: 1/3/2020 4:10:05 AM)"=13119, "Automatic Update (DT: Olivine-3-1; HV: 2.2; Time: 1/3/2020 4:10:07 AM)"=13120, "Automatic Update (DT: Olivine-3-1; HV: 2.2; Time: 1/3/2020 4:10:09 AM)"=13121, "Automatic Update (DT: Olivine-3-1; HV: 2.2; Time: 1/3/2020 4:10:10 AM)"=13122, "Automatic Update (DT: Olivine-3-1; HV: 2.2; Time: 1/3/2020 4:10:11 AM)"=13123, "Automatic Update (DT: Olivine-3-1; HV: 2.2; Time: 1/3/2020 4:10:12 AM)"=13124, "Automatic Update (DT: Olivine-3-1; HV: 2.2; Time: 1/3/2020 4:10:13 AM)"=13125, "Automatic Update (DT: Olivine-3-1; HV: 2.2; Time: 1/3/2020 4:10:14 AM)"=13126, "Automatic Update (DT: Olivine-3-1; HV: 2.2; Time: 1/3/2020 4:10:15 AM)"=13127, "Automatic Update (DT: Olivine-3-1; HV: 2.2; Time: 1/3/2020 4:10:16 AM)"=13128, "Automatic Update (DT: Olivine-3-1; HV: 2.2; Time: 1/3/2020 4:10:17 AM)"=13129, "Automatic Update (DT: Olivine-3-1; HV: 2.2; Time: 1/3/2020 4:10:18 AM)"=13130, "Automatic Update (DT: Olivine-3-1; HV: 2.2; Time: 1/3/2020 4:10:20 AM)"=13131, "Automatic Update (DT: Olivine-3-1; HV: 2.2; Time: 1/3/2020 4:10:21 AM)"=13132, "Automatic Update (DT: Olivine-3-1; HV: 2.2; Time: 1/3/2020 4:10:22 AM)"=13133, "Automatic Update (DT: Olivine-3-1; HV: 2.2; Time: 1/3/2020 4:10:23 AM)"=13134, "Automatic Update (DT: Olivine-3-1; HV: 2.2; Time: 1/3/2020 4:10:28 AM)"=13135, "Automatic Update (DT: Olivine-3-1; HV: 2.2; Time: 1/3/2020 4:10:29 AM)"=13136, "Automatic Update (DT: Olivine-3-1; HV: 2.2; Time: 1/3/2020 4:10:30 AM)"=13137, "Automatic Update (DT: Olivine-3-1; HV: 2.2; Time: 1/3/2020 4:10:33 AM)"=13138, "Automatic Update (DT: Olivine-3-1; HV: 2.2; Time: 1/3/2020 4:10:34 AM)"=13139, "Automatic Update (DT: Olivine-3-1; HV: 2.2; Time: 1/3/2020 4:10:35 AM)"=13140, "Automatic Update (DT: Olivine-3-1; HV: 2.2; Time: 1/3/2020 4:10:37 AM)"=13141, "Automatic Update (DT: Olivine-3-1; HV: 2.2; Time: 1/3/2020 4:10:38 AM)"=13142, "Automatic Update (DT: Olivine-3-1; HV: 2.2; Time: 1/3/2020 4:10:40 AM)"=13143, "Automatic Update (DT: Olivine-3-1; HV: 2.2; Time: 1/3/2020 4:10:42 AM)"=13144, "Automatic Update (DT: Olivine-3-1; HV: 2.2; Time: 1/3/2020 4:10:43 AM)"=13145, "Automatic Update (DT: Olivine-3-1; HV: 2.2; Time: 1/3/2020 4:10:44 AM)"=13146, "Automatic Update (DT: Olivine-3-1; HV: 2.2; Time: 1/3/2020 4:10:46 AM)"=13147, "Automatic Update (DT: Olivine-3-1; HV: 2.2; Time: 1/3/2020 4:10:47 AM)"=13148, "Automatic Update (DT: Olivine-3-1; HV: 2.2; Time: 1/3/2020 4:10:48 AM)"=13149, "Automatic Update (DT: Olivine-3-1; HV: 2.2; Time: 1/3/2020 4:10:49 AM)"=13150, "Automatic Update (DT: Olivine-3-1; HV: 2.2; Time: 1/3/2020 4:10:50 AM)"=13151, "Automatic Update (DT: Olivine-3-1; HV: 2.2; Time: 1/3/2020 4:10:51 AM)"=13152, "Automatic Update (DT: Olivine-3-1; HV: 2.2; Time: 1/3/2020 4:10:52 AM)"=13153, "Automatic Update (DT: Olivine-3-1; HV: 2.2; Time: 1/3/2020 4:10:53 AM)"=13154, "Automatic Update (DT: Olivine-3-1; HV: 2.2; Time: 1/3/2020 4:10:54 AM)"=13155, "Automatic Update (DT: Olivine-3-1; HV: 2.2; Time: 1/3/2020 4:10:55 AM)"=13156, "Automatic Update (DT: Olivine-3-1; HV: 2.2; Time: 1/3/2020 4:10:56 AM)"=13157, "Automatic Update (DT: Olivine-3-1; HV: 2.2; Time: 1/3/2020 4:10:57 AM)"=13158, "Automatic Update (DT: Olivine-3-1; HV: 2.2; Time: 1/3/2020 4:10:58 AM)"=13159, "Automatic Update (DT: Olivine-3-1; HV: 2.2; Time: 1/3/2020 4:10:59 AM)"=13160, "Automatic Update (DT: Olivine-3-1; HV: 2.2; Time: 1/3/2020 4:11:00 AM)"=13161, "Automatic Update (DT: Olivine-3-1; HV: 2.2; Time: 1/3/2020 4:11:01 AM)"=13162, "Automatic Update (DT: Olivine-3-1; HV: 2.2; Time: 1/3/2020 4:11:03 AM)"=13163, "Automatic Update (DT: Olivine-3-1; HV: 2.2; Time: 1/3/2020 4:11:04 AM)"=13164, "Automatic Update (DT: Olivine-3-1; HV: 2.2; Time: 1/3/2020 4:11:05 AM)"=13165, "Automatic Update (DT: Olivine-3-1; HV: 2.2; Time: 1/3/2020 4:11:07 AM)"=13166, "Automatic Update (DT: Olivine-3-1; HV: 2.2; Time: 1/3/2020 4:11:08 AM)"=13167, "Automatic Update (DT: Olivine-3-1; HV: 2.2; Time: 1/3/2020 4:11:09 AM)"=13168, "Automatic Update (DT: Olivine-3-1; HV: 2.2; Time: 1/3/2020 4:11:10 AM)"=13169, "Automatic Update (DT: Olivine-3-1; HV: 2.2; Time: 1/3/2020 4:11:11 AM)"=13170, "Automatic Update (DT: Olivine-3-1; HV: 2.2; Time: 1/3/2020 4:11:12 AM)"=13171, "Automatic Update (DT: Olivine-3-1; HV: 2.2; Time: 1/3/2020 4:11:13 AM)"=13172, "Automatic Update (DT: Olivine-3-1; HV: 2.2; Time: 1/3/2020 4:11:14 AM)"=13173, "Automatic Update (DT: Olivine-3-1; HV: 2.2; Time: 1/3/2020 4:11:15 AM)"=13174, "Automatic Update (DT: Olivine-3-1; HV: 2.2; Time: 1/3/2020 4:11:16 AM)"=13175, "Automatic Update (DT: Olivine-3-1; HV: 2.2; Time: 1/3/2020 4:11:17 AM)"=13176, "Automatic Update (DT: Olivine-3-1; HV: 2.2; Time: 1/3/2020 4:11:18 AM)"=13177, "Automatic Update (DT: Olivine-3-1; HV: 2.2; Time: 1/3/2020 4:11:19 AM)"=13178, "Automatic Update (DT: Olivine-3-1; HV: 2.2; Time: 1/3/2020 4:11:20 AM)"=13179, "Automatic Update (DT: Olivine-3-1; HV: 2.2; Time: 1/3/2020 4:11:21 AM)"=13180, "Automatic Update (DT: Olivine-3-1; HV: 2.2; Time: 1/3/2020 4:11:22 AM)"=13181, "Automatic Update (DT: Olivine-3-1; HV: 2.2; Time: 1/3/2020 4:11:23 AM)"=13182, "Automatic Update (DT: Olivine-3-1; HV: 2.2; Time: 1/3/2020 4:11:25 AM)"=13183, "Automatic Update (DT: Olivine-3-1; HV: 2.2; Time: 1/3/2020 4:11:26 AM)"=13184, "Automatic Update (DT: Olivine-3-1; HV: 2.2; Time: 1/3/2020 4:11:27 AM)"=13185, "Automatic Update (DT: Olivine-3-1; HV: 2.2; Time: 1/3/2020 4:11:28 AM)"=13186, "Automatic Update (DT: Olivine-3-1; HV: 2.2; Time: 1/3/2020 4:11:29 AM)"=13187, "Automatic Update (DT: Olivine-3-1; HV: 2.2; Time: 1/3/2020 4:11:30 AM)"=13188, "Automatic Update (DT: Olivine-3-1; HV: 2.2; Time: 1/3/2020 4:11:31 AM)"=13189, "Automatic Update (DT: Olivine-3-1; HV: 2.2; Time: 1/3/2020 4:11:32 AM)"=13190, "Automatic Update (DT: Olivine-3-1; HV: 2.2; Time: 1/3/2020 4:11:33 AM)"=13191, "Automatic Update (DT: Olivine-3-1; HV: 2.2; Time: 1/3/2020 4:11:34 AM)"=13192, "Automatic Update (DT: Olivine-3-1; HV: 2.2; Time: 1/3/2020 4:11:35 AM)"=13193, "Automatic Update (DT: Olivine-3-1; HV: 2.2; Time: 1/3/2020 4:11:36 AM)"=13194, "Automatic Update (DT: Olivine-3-1; HV: 2.2; Time: 1/3/2020 4:11:37 AM)"=13195, "Automatic Update (DT: Olivine-3-1; HV: 2.2; Time: 1/3/2020 4:11:38 AM)"=13196, "Automatic Update (DT: Olivine-3-1; HV: 2.2; Time: 1/3/2020 4:11:40 AM)"=13197, "Automatic Update (DT: Olivine-3-1; HV: 2.2; Time: 1/3/2020 4:11:41 AM)"=13198, "Automatic Update (DT: Olivine-3-1; HV: 2.2; Time: 1/3/2020 4:11:42 AM)"=13199, "Automatic Update (DT: Olivine-3-1; HV: 2.2; Time: 1/3/2020 4:11:43 AM)"=13200, "Automatic Update (DT: Olivine-3-1; HV: 2.2; Time: 1/3/2020 4:11:44 AM)"=13201, "Automatic Update (DT: Olivine-3-1; HV: 2.2; Time: 1/3/2020 4:11:45 AM)"=13202, "Automatic Update (DT: Olivine-3-1; HV: 2.2; Time: 1/3/2020 4:11:46 AM)"=13203, "Automatic Update (DT: Olivine-3-1; HV: 2.2; Time: 1/3/2020 4:11:48 AM)"=13204, "Automatic Update (DT: Olivine-3-1; HV: 2.2; Time: 1/3/2020 4:11:49 AM)"=13205, "Automatic Update (DT: Olivine-3-1; HV: 2.2; Time: 1/3/2020 4:11:58 AM)"=13206, "Automatic Update (DT: Olivine-3-1; HV: 2.2; Time: 1/3/2020 4:11:59 AM)"=13207, "Automatic Update (DT: Olivine-3-1; HV: 2.2; Time: 1/3/2020 4:12:00 AM)"=13208, "Automatic Update (DT: Olivine-3-1; HV: 2.2; Time: 1/3/2020 4:12:02 AM)"=13209, "Automatic Update (DT: Olivine-3-1; HV: 2.2; Time: 1/3/2020 4:12:03 AM)"=13210, "Automatic Update (DT: Olivine-3-1; HV: 2.2; Time: 1/3/2020 4:13:05 AM)"=13211, "Automatic Update (DT: Olivine-3-1; HV: 2.2; Time: 1/3/2020 4:13:06 AM)"=13212, "Automatic Update (DT: Olivine-3-1; HV: 2.2; Time: 1/3/2020 4:13:07 AM)"=13213, "Automatic Update (DT: Olivine-3-1; HV: 2.2; Time: 1/3/2020 4:13:08 AM)"=13214, "Automatic Update (DT: Olivine-3-1; HV: 2.2; Time: 1/3/2020 4:13:09 AM)"=13215, "Automatic Update (DT: Olivine-3-1; HV: 2.2; Time: 1/3/2020 4:13:10 AM)"=13216, "Automatic Update (DT: Olivine-3-1; HV: 2.2; Time: 1/3/2020 4:13:11 AM)"=13217, "Automatic Update (DT: Olivine-3-1; HV: 2.2; Time: 1/3/2020 4:13:12 AM)"=13218, "Automatic Update (DT: Olivine-3-1; HV: 2.2; Time: 1/3/2020 4:13:13 AM)"=13219, "Automatic Update (DT: Olivine-3-1; HV: 2.2; Time: 1/3/2020 4:13:14 AM)"=13220, "Automatic Update (DT: Olivine-3-1; HV: 2.2; Time: 1/3/2020 4:13:15 AM)"=13221, "Automatic Update (DT: Olivine-3-1; HV: 2.2; Time: 1/3/2020 4:13:16 AM)"=13222, "Automatic Update (DT: Olivine-3-1; HV: 2.2; Time: 1/3/2020 4:13:17 AM)"=13223, "Automatic Update (DT: Olivine-3-1; HV: 2.2; Time: 1/3/2020 4:13:18 AM)"=13224, "Automatic Update (DT: Olivine-3-1; HV: 2.2; Time: 1/3/2020 4:13:19 AM)"=13225, "Automatic Update (DT: Olivine-3-1; HV: 2.2; Time: 1/3/2020 4:13:21 AM)"=13226, "Automatic Update (DT: Olivine-3-1; HV: 2.2; Time: 1/3/2020 4:13:22 AM)"=13227, "Automatic Update (DT: Olivine-3-1; HV: 2.2; Time: 1/3/2020 4:13:23 AM)"=13228, "Automatic Update (DT: Olivine-3-1; HV: 2.2; Time: 1/3/2020 4:13:24 AM)"=13229, "Automatic Update (DT: Olivine-3-1; HV: 2.2; Time: 1/3/2020 4:13:25 AM)"=13230, "Automatic Update (DT: Olivine-3-1; HV: 2.2; Time: 1/3/2020 4:13:26 AM)"=13231, "Automatic Update (DT: Olivine-3-1; HV: 2.2; Time: 1/3/2020 4:13:27 AM)"=13232, "Automatic Update (DT: Olivine-3-1; HV: 2.2; Time: 1/3/2020 4:13:28 AM)"=13233, "Automatic Update (DT: Olivine-3-1; HV: 2.2; Time: 1/3/2020 4:13:29 AM)"=13234, "Automatic Update (DT: Olivine-3-1; HV: 2.2; Time: 1/3/2020 4:13:30 AM)"=13235, "Automatic Update (DT: Olivine-3-1; HV: 2.2; Time: 1/3/2020 4:13:31 AM)"=13236, "Automatic Update (DT: Olivine-3-1; HV: 2.2; Time: 1/3/2020 4:13:32 AM)"=13237, "Automatic Update (DT: Olivine-3-1; HV: 2.2; Time: 1/3/2020 4:13:33 AM)"=13238, "Automatic Update (DT: Olivine-3-1; HV: 2.2; Time: 1/3/2020 4:13:34 AM)"=13239, "Automatic Update (DT: Olivine-3-1; HV: 2.2; Time: 1/3/2020 4:13:35 AM)"=13240, "Automatic Update (DT: Olivine-3-1; HV: 2.2; Time: 1/3/2020 4:13:36 AM)"=13241, "Automatic Update (DT: Olivine-3-1; HV: 2.2; Time: 1/3/2020 4:13:37 AM)"=13242, "Automatic Update (DT: Olivine-3-1; HV: 2.2; Time: 1/3/2020 4:13:38 AM)"=13243, "Automatic Update (DT: Olivine-3-1; HV: 2.2; Time: 1/3/2020 4:13:47 AM)"=13244, "Automatic Update (DT: Olivine-3-1; HV: 2.2; Time: 1/3/2020 4:13:48 AM)"=13245, "Automatic Update (DT: Olivine-3-1; HV: 2.2; Time: 1/3/2020 4:13:49 AM)"=13246, "Automatic Update (DT: Olivine-3-1; HV: 2.2; Time: 1/3/2020 4:13:51 AM)"=13247, "Automatic Update (DT: Olivine-3-1; HV: 2.2; Time: 1/3/2020 4:13:53 AM)"=13248, "Automatic Update (DT: Olivine-3-1; HV: 2.2; Time: 1/3/2020 4:13:57 AM)"=13249, "Automatic Update (DT: Olivine-3-1; HV: 2.2; Time: 1/3/2020 4:13:58 AM)"=13250, "Automatic Update (DT: Olivine-3-1; HV: 2.2; Time: 1/3/2020 4:13:59 AM)"=13251, "Automatic Update (DT: Olivine-3-1; HV: 2.2; Time: 1/3/2020 4:14:00 AM)"=13252, "Automatic Update (DT: Olivine-3-1; HV: 2.2; Time: 1/3/2020 4:14:01 AM)"=13253, "Automatic Update (DT: Olivine-3-1; HV: 2.2; Time: 1/3/2020 4:14:02 AM)"=13254, "Automatic Update (DT: Olivine-3-1; HV: 2.2; Time: 1/3/2020 4:14:03 AM)"=13255, "Automatic Update (DT: Olivine-3-1; HV: 2.2; Time: 1/3/2020 4:14:04 AM)"=13256, "Automatic Update (DT: Olivine-3-1; HV: 2.2; Time: 1/3/2020 4:14:05 AM)"=13257, "Automatic Update (DT: Olivine-3-1; HV: 2.2; Time: 1/3/2020 4:14:06 AM)"=13258, "Automatic Update (DT: Olivine-3-1; HV: 2.2; Time: 1/3/2020 4:14:08 AM)"=13259, "Automatic Update (DT: Olivine-3-1; HV: 2.2; Time: 1/3/2020 4:14:09 AM)"=13260, "Automatic Update (DT: Olivine-3-1; HV: 2.2; Time: 1/3/2020 4:14:10 AM)"=13261, "Automatic Update (DT: Olivine-3-1; HV: 2.2; Time: 1/3/2020 4:14:11 AM)"=13262, "Automatic Update (DT: Olivine-3-1; HV: 2.2; Time: 1/3/2020 4:14:12 AM)"=13263, "Automatic Update (DT: Olivine-3-1; HV: 2.2; Time: 1/3/2020 4:14:13 AM)"=13264, "Automatic Update (DT: Olivine-3-1; HV: 2.2; Time: 1/3/2020 4:14:14 AM)"=13265, "Automatic Update (DT: Olivine-3-1; HV: 2.2; Time: 1/3/2020 4:14:15 AM)"=13266, "Automatic Update (DT: Olivine-3-1; HV: 2.2; Time: 1/3/2020 4:14:16 AM)"=13267, "Automatic Update (DT: Olivine-3-1; HV: 2.2; Time: 1/3/2020 4:14:22 AM)"=13268, "Automatic Update (DT: Olivine-3-1; HV: 2.2; Time: 1/3/2020 4:14:24 AM)"=13269, "Automatic Update (DT: Olivine-3-1; HV: 2.2; Time: 1/3/2020 4:14:25 AM)"=13270, "Automatic Update (DT: Olivine-3-1; HV: 2.2; Time: 1/3/2020 4:14:26 AM)"=13271, "Automatic Update (DT: Olivine-3-1; HV: 2.2; Time: 1/3/2020 4:14:30 AM)"=13272, "Automatic Update (DT: Olivine-3-1; HV: 2.2; Time: 1/3/2020 4:14:31 AM)"=13273, "Automatic Update (DT: Olivine-3-1; HV: 2.2; Time: 1/3/2020 4:14:32 AM)"=13274, "Automatic Update (DT: Olivine-3-1; HV: 2.2; Time: 1/3/2020 4:14:33 AM)"=13275, "Automatic Update (DT: Olivine-3-1; HV: 2.2; Time: 1/3/2020 4:14:35 AM)"=13276, "Automatic Update (DT: Olivine-3-1; HV: 2.2; Time: 1/3/2020 4:14:36 AM)"=13277, "Automatic Update (DT: Olivine-3-1; HV: 2.2; Time: 1/3/2020 4:14:37 AM)"=13278, "Automatic Update (DT: Olivine-3-1; HV: 2.2; Time: 1/3/2020 4:14:39 AM)"=13279, "Automatic Update (DT: Olivine-3-1; HV: 2.2; Time: 1/3/2020 4:14:40 AM)"=13280, "Automatic Update (DT: Olivine-3-1; HV: 2.2; Time: 1/3/2020 4:14:41 AM)"=13281, "Automatic Update (DT: Olivine-3-1; HV: 2.2; Time: 1/3/2020 4:14:50 AM)"=13282, "Automatic Update (DT: Olivine-3-1; HV: 2.2; Time: 1/3/2020 4:14:54 AM)"=13283, "Automatic Update (DT: Olivine-3-1; HV: 2.2; Time: 1/3/2020 4:14:55 AM)"=13284, "Automatic Update (DT: Olivine-3-1; HV: 2.2; Time: 1/3/2020 4:14:57 AM)"=13285, "Automatic Update (DT: Olivine-3-1; HV: 2.2; Time: 1/3/2020 4:14:58 AM)"=13286, "Automatic Update (DT: Olivine-3-1; HV: 2.2; Time: 1/3/2020 4:14:59 AM)"=13287, "Automatic Update (DT: Olivine-3-1; HV: 2.2; Time: 1/3/2020 4:15:00 AM)"=13288, "Automatic Update (DT: Olivine-3-1; HV: 2.2; Time: 1/3/2020 4:15:21 AM)"=13289, "Automatic Update (DT: Olivine-3-1; HV: 2.2; Time: 1/3/2020 4:15:24 AM)"=13290, "Automatic Update (DT: Olivine-3-1; HV: 2.2; Time: 1/3/2020 4:15:27 AM)"=13291, "Automatic Update (DT: Olivine-3-1; HV: 2.2; Time: 1/3/2020 4:15:28 AM)"=13292, "Automatic Update (DT: Olivine-3-1; HV: 2.2; Time: 1/3/2020 4:15:29 AM)"=13293, "Automatic Update (DT: Olivine-3-1; HV: 2.2; Time: 1/3/2020 4:15:30 AM)"=13294, "Automatic Update (DT: Olivine-3-1; HV: 2.2; Time: 1/3/2020 4:15:31 AM)"=13295, "Automatic Update (DT: Olivine-3-1; HV: 2.2; Time: 1/3/2020 4:15:39 AM)"=13296, "Automatic Update (DT: Olivine-3-1; HV: 2.2; Time: 1/3/2020 4:15:40 AM)"=13297, "Automatic Update (DT: Olivine-3-1; HV: 2.2; Time: 1/3/2020 4:15:41 AM)"=13298, "Automatic Update (DT: Olivine-3-1; HV: 2.2; Time: 1/3/2020 4:15:43 AM)"=13299, "Automatic Update (DT: Olivine-3-1; HV: 2.2; Time: 1/3/2020 4:15:44 AM)"=13300, "Automatic Update (DT: Olivine-3-1; HV: 2.2; Time: 1/3/2020 4:15:45 AM)"=13301, "Automatic Update (DT: Olivine-3-1; HV: 2.2; Time: 1/3/2020 4:15:47 AM)"=13302, "Automatic Update (DT: Olivine-3-1; HV: 2.2; Time: 1/3/2020 4:15:48 AM)"=13303, "Automatic Update (DT: Olivine-3-1; HV: 2.2; Time: 1/3/2020 4:15:49 AM)"=13304, "Automatic Update (DT: Olivine-3-1; HV: 2.2; Time: 1/3/2020 4:15:50 AM)"=13305, "Automatic Update (DT: Olivine-3-1; HV: 2.2; Time: 1/3/2020 4:15:51 AM)"=13306, "Automatic Update (DT: Olivine-3-1; HV: 2.2; Time: 1/3/2020 4:15:52 AM)"=13307, "Automatic Update (DT: Olivine-3-1; HV: 2.2; Time: 1/3/2020 4:15:53 AM)"=13308, "Automatic Update (DT: Olivine-3-1; HV: 2.2; Time: 1/3/2020 4:15:54 AM)"=13309, "Automatic Update (DT: Olivine-3-1; HV: 2.2; Time: 1/3/2020 4:15:56 AM)"=13310, "Automatic Update (DT: Olivine-3-1; HV: 2.2; Time: 1/3/2020 4:15:57 AM)"=13311, "Automatic Update (DT: Olivine-3-1; HV: 2.2; Time: 1/3/2020 4:15:58 AM)"=13312, "Automatic Update (DT: Olivine-3-1; HV: 2.2; Time: 1/3/2020 4:15:59 AM)"=13313, "Automatic Update (DT: Olivine-3-1; HV: 2.2; Time: 1/3/2020 4:16:00 AM)"=13314, "Automatic Update (DT: Olivine-3-1; HV: 2.2; Time: 1/3/2020 4:16:01 AM)"=13315, "Automatic Update (DT: Olivine-3-1; HV: 2.2; Time: 1/3/2020 4:16:02 AM)"=13316, "Automatic Update (DT: Olivine-3-1; HV: 2.2; Time: 1/3/2020 4:17:10 AM)"=13317, "Automatic Update (DT: Olivine-3-1; HV: 2.2; Time: 1/3/2020 4:17:11 AM)"=13318, "Automatic Update (DT: Olivine-3-1; HV: 2.2; Time: 1/3/2020 4:17:12 AM)"=13319, "Automatic Update (DT: Olivine-3-1; HV: 2.2; Time: 1/3/2020 4:17:13 AM)"=13320, "Automatic Update (DT: Olivine-3-1; HV: 2.2; Time: 1/3/2020 4:17:14 AM)"=13321, "Automatic Update (DT: Olivine-3-1; HV: 2.2; Time: 1/3/2020 4:17:15 AM)"=13322, "Automatic Update (DT: Olivine-3-1; HV: 2.2; Time: 1/3/2020 4:17:16 AM)"=13323, "Automatic Update (DT: Olivine-3-1; HV: 2.2; Time: 1/3/2020 4:17:17 AM)"=13324, "Automatic Update (DT: Olivine-3-1; HV: 2.2; Time: 1/3/2020 4:17:18 AM)"=13325, "Automatic Update (DT: Olivine-3-1; HV: 2.2; Time: 1/3/2020 4:17:19 AM)"=13326, "Automatic Update (DT: Olivine-3-1; HV: 2.2; Time: 1/3/2020 4:17:20 AM)"=13327, "Automatic Update (DT: Olivine-3-1; HV: 2.2; Time: 1/3/2020 4:17:21 AM)"=13328, "Automatic Update (DT: Olivine-3-1; HV: 2.2; Time: 1/3/2020 4:17:22 AM)"=13329, "Automatic Update (DT: Olivine-3-1; HV: 2.2; Time: 1/3/2020 4:17:23 AM)"=13330, "Automatic Update (DT: Olivine-3-1; HV: 2.2; Time: 1/3/2020 4:17:25 AM)"=13331, "Automatic Update (DT: Olivine-3-1; HV: 2.2; Time: 1/3/2020 4:17:26 AM)"=13332, "Automatic Update (DT: Olivine-3-1; HV: 2.2; Time: 1/3/2020 4:17:27 AM)"=13333, "Automatic Update (DT: Olivine-3-1; HV: 2.2; Time: 1/3/2020 4:17:28 AM)"=13334, "Automatic Update (DT: Olivine-3-1; HV: 2.2; Time: 1/3/2020 4:17:29 AM)"=13335, "Automatic Update (DT: Olivine-3-1; HV: 2.2; Time: 1/3/2020 4:17:30 AM)"=13336, "Automatic Update (DT: Olivine-3-1; HV: 2.2; Time: 1/3/2020 4:17:31 AM)"=13337, "Automatic Update (DT: Olivine-3-1; HV: 2.2; Time: 1/3/2020 4:17:32 AM)"=13338, "Automatic Update (DT: Olivine-3-1; HV: 2.2; Time: 1/3/2020 4:17:34 AM)"=13339, "Automatic Update (DT: Olivine-3-1; HV: 2.2; Time: 1/3/2020 4:17:35 AM)"=13340, "Automatic Update (DT: Olivine-3-1; HV: 2.2; Time: 1/3/2020 4:17:36 AM)"=13341, "Automatic Update (DT: Olivine-3-1; HV: 2.2; Time: 1/3/2020 4:17:37 AM)"=13342, "Automatic Update (DT: Olivine-3-1; HV: 2.2; Time: 1/3/2020 4:17:38 AM)"=13343, "Automatic Update (DT: Olivine-3-1; HV: 2.2; Time: 1/3/2020 4:17:39 AM)"=13344, "Automatic Update (DT: Olivine-3-1; HV: 2.2; Time: 1/3/2020 4:17:40 AM)"=13345, "Automatic Update (DT: Olivine-3-1; HV: 2.2; Time: 1/3/2020 4:17:41 AM)"=13346, "Automatic Update (DT: Olivine-3-1; HV: 2.2; Time: 1/3/2020 4:17:42 AM)"=13347, "Automatic Update (DT: Olivine-3-1; HV: 2.2; Time: 1/3/2020 4:17:43 AM)"=13348, "Automatic Update (DT: Olivine-3-1; HV: 2.2; Time: 1/3/2020 4:17:44 AM)"=13349, "Automatic Update (DT: Olivine-3-1; HV: 2.2; Time: 1/3/2020 4:17:45 AM)"=13350, "Automatic Update (DT: Olivine-3-1; HV: 2.2; Time: 1/3/2020 4:17:46 AM)"=13351, "Automatic Update (DT: Olivine-3-1; HV: 2.2; Time: 1/3/2020 4:17:48 AM)"=13352, "Automatic Update (DT: Olivine-3-1; HV: 2.2; Time: 1/3/2020 4:17:49 AM)"=13353, "Automatic Update (DT: Olivine-3-1; HV: 2.2; Time: 1/3/2020 4:17:50 AM)"=13354, "Automatic Update (DT: Olivine-3-1; HV: 2.2; Time: 1/3/2020 4:17:53 AM)"=13355, "Automatic Update (DT: Olivine-3-1; HV: 2.2; Time: 1/3/2020 4:17:54 AM)"=13356, "Automatic Update (DT: Olivine-3-1; HV: 2.2; Time: 1/3/2020 4:17:59 AM)"=13357, "Automatic Update (DT: Olivine-3-1; HV: 2.2; Time: 1/3/2020 4:18:00 AM)"=13358, "Automatic Update (DT: Olivine-3-1; HV: 2.2; Time: 1/3/2020 4:18:01 AM)"=13359, "Automatic Update (DT: Olivine-3-1; HV: 2.2; Time: 1/3/2020 4:18:02 AM)"=13360, "Automatic Update (DT: Olivine-3-1; HV: 2.2; Time: 1/3/2020 4:18:03 AM)"=13361, "Automatic Update (DT: Olivine-3-1; HV: 2.2; Time: 1/3/2020 4:18:04 AM)"=13362, "Automatic Update (DT: Olivine-3-1; HV: 2.2; Time: 1/3/2020 4:18:05 AM)"=13363, "Automatic Update (DT: Olivine-3-1; HV: 2.2; Time: 1/3/2020 4:18:06 AM)"=13364, "Automatic Update (DT: Olivine-3-1; HV: 2.2; Time: 1/3/2020 4:18:07 AM)"=13365, "Automatic Update (DT: Olivine-3-1; HV: 2.2; Time: 1/3/2020 4:18:08 AM)"=13366, "Automatic Update (DT: Olivine-3-1; HV: 2.2; Time: 1/3/2020 4:18:09 AM)"=13367, "Automatic Update (DT: Olivine-3-1; HV: 2.2; Time: 1/3/2020 4:18:10 AM)"=13368, "Automatic Update (DT: Olivine-3-1; HV: 2.2; Time: 1/3/2020 4:18:11 AM)"=13369, "Automatic Update (DT: Olivine-3-1; HV: 2.2; Time: 1/3/2020 4:18:12 AM)"=13370, "Automatic Update (DT: Olivine-3-1; HV: 2.2; Time: 1/3/2020 4:18:13 AM)"=13371, "Automatic Update (DT: Olivine-3-1; HV: 2.2; Time: 1/3/2020 4:18:14 AM)"=13372, "Automatic Update (DT: Olivine-3-1; HV: 2.2; Time: 1/3/2020 4:18:15 AM)"=13373, "Automatic Update (DT: Olivine-3-1; HV: 2.2; Time: 1/3/2020 4:18:16 AM)"=13374, "Automatic Update (DT: Olivine-3-1; HV: 2.2; Time: 1/3/2020 4:18:18 AM)"=13375, "Automatic Update (DT: Olivine-3-1; HV: 2.2; Time: 1/3/2020 4:18:19 AM)"=13376, "Automatic Update (DT: Olivine-3-1; HV: 2.2; Time: 1/3/2020 4:18:20 AM)"=13377, "Automatic Update (DT: Olivine-3-1; HV: 2.2; Time: 1/3/2020 4:18:22 AM)"=13378, "Automatic Update (DT: Olivine-3-1; HV: 2.2; Time: 1/3/2020 4:18:23 AM)"=13379, "Automatic Update (DT: Olivine-3-1; HV: 2.2; Time: 1/3/2020 4:18:24 AM)"=13380, "Automatic Update (DT: Olivine-3-1; HV: 2.2; Time: 1/3/2020 4:18:25 AM)"=13381, "Automatic Update (DT: Olivine-3-1; HV: 2.2; Time: 1/3/2020 4:18:26 AM)"=13382, "Automatic Update (DT: Olivine-3-1; HV: 2.2; Time: 1/3/2020 4:18:27 AM)"=13383, "Automatic Update (DT: Olivine-3-1; HV: 2.2; Time: 1/3/2020 4:18:28 AM)"=13384, "Automatic Update (DT: Olivine-3-1; HV: 2.2; Time: 1/3/2020 4:18:29 AM)"=13385, "Automatic Update (DT: Olivine-3-1; HV: 2.2; Time: 1/3/2020 4:18:30 AM)"=13386, "Automatic Update (DT: Olivine-3-1; HV: 2.2; Time: 1/3/2020 4:18:31 AM)"=13387, "Automatic Update (DT: Olivine-3-1; HV: 2.2; Time: 1/3/2020 4:18:32 AM)"=13388, "Automatic Update (DT: Olivine-3-1; HV: 2.2; Time: 1/3/2020 4:18:34 AM)"=13389, "Automatic Update (DT: Olivine-3-1; HV: 2.2; Time: 1/3/2020 4:18:35 AM)"=13390, "Automatic Update (DT: Olivine-3-1; HV: 2.2; Time: 1/3/2020 4:18:37 AM)"=13391, "Automatic Update (DT: Olivine-3-1; HV: 2.2; Time: 1/3/2020 4:18:38 AM)"=13392, "Automatic Update (DT: Olivine-3-1; HV: 2.2; Time: 1/3/2020 4:18:39 AM)"=13393, "Automatic Update (DT: Olivine-3-1; HV: 2.2; Time: 1/3/2020 4:18:40 AM)"=13394, "Automatic Update (DT: Olivine-3-1; HV: 2.2; Time: 1/3/2020 4:18:41 AM)"=13395, "Automatic Update (DT: Olivine-3-1; HV: 2.2; Time: 1/3/2020 4:18:43 AM)"=13396, "Automatic Update (DT: Olivine-3-1; HV: 2.2; Time: 1/3/2020 4:18:45 AM)"=13397, "Automatic Update (DT: Olivine-3-1; HV: 2.2; Time: 1/3/2020 4:18:46 AM)"=13398, "Automatic Update (DT: Olivine-3-1; HV: 2.2; Time: 1/3/2020 4:18:48 AM)"=13399, "Automatic Update (DT: Olivine-3-1; HV: 2.2; Time: 1/3/2020 4:18:49 AM)"=13400, "Automatic Update (DT: Olivine-3-1; HV: 2.2; Time: 1/3/2020 4:18:51 AM)"=13401, "Automatic Update (DT: Olivine-3-1; HV: 2.2; Time: 1/3/2020 4:18:52 AM)"=13402, "Automatic Update (DT: Olivine-3-1; HV: 2.2; Time: 1/3/2020 4:18:53 AM)"=13403, "Automatic Update (DT: Olivine-3-1; HV: 2.2; Time: 1/3/2020 4:18:54 AM)"=13404, "Automatic Update (DT: Olivine-3-1; HV: 2.2; Time: 1/3/2020 4:18:55 AM)"=13405, "Automatic Update (DT: Olivine-3-1; HV: 2.2; Time: 1/3/2020 4:18:56 AM)"=13406, "Automatic Update (DT: Olivine-3-1; HV: 2.2; Time: 1/3/2020 4:18:57 AM)"=13407, "Automatic Update (DT: Olivine-3-1; HV: 2.2; Time: 1/3/2020 4:18:58 AM)"=13408, "Automatic Update (DT: Olivine-3-1; HV: 2.2; Time: 1/3/2020 4:18:59 AM)"=13409, "Automatic Update (DT: Olivine-3-1; HV: 2.2; Time: 1/3/2020 4:19:00 AM)"=13410, "Automatic Update (DT: Olivine-3-1; HV: 2.2; Time: 1/3/2020 4:19:02 AM)"=13411, "Automatic Update (DT: Olivine-3-1; HV: 2.2; Time: 1/3/2020 4:19:03 AM)"=13412, "Automatic Update (DT: Olivine-3-1; HV: 2.2; Time: 1/3/2020 4:19:05 AM)"=13413, "Automatic Update (DT: Olivine-3-1; HV: 2.2; Time: 1/3/2020 4:19:06 AM)"=13414, "Automatic Update (DT: Olivine-3-1; HV: 2.2; Time: 1/3/2020 4:19:07 AM)"=13415, "Automatic Update (DT: Olivine-3-1; HV: 2.2; Time: 1/3/2020 4:19:08 AM)"=13416, "Automatic Update (DT: Olivine-3-1; HV: 2.2; Time: 1/3/2020 4:19:10 AM)"=13417, "Automatic Update (DT: Olivine-3-1; HV: 2.2; Time: 1/3/2020 4:19:11 AM)"=13418, "Automatic Update (DT: Olivine-3-1; HV: 2.2; Time: 1/3/2020 4:19:12 AM)"=13419, "Automatic Update (DT: Olivine-3-1; HV: 2.2; Time: 1/3/2020 4:19:13 AM)"=13420, "Automatic Update (DT: Olivine-3-1; HV: 2.2; Time: 1/3/2020 4:19:24 AM)"=13421, "Automatic Update (DT: Olivine-3-1; HV: 2.2; Time: 1/3/2020 4:19:25 AM)"=13422, "Automatic Update (DT: Olivine-3-1; HV: 2.2; Time: 1/3/2020 4:19:26 AM)"=13423, "Automatic Update (DT: Olivine-3-1; HV: 2.2; Time: 1/3/2020 4:19:29 AM)"=13424, "Automatic Update (DT: Olivine-3-1; HV: 2.2; Time: 1/3/2020 4:19:30 AM)"=13425, "Automatic Update (DT: Olivine-3-1; HV: 2.2; Time: 1/3/2020 4:19:31 AM)"=13426, "Automatic Update (DT: Olivine-3-1; HV: 2.2; Time: 1/3/2020 4:19:32 AM)"=13427, "Automatic Update (DT: Olivine-3-1; HV: 2.2; Time: 1/3/2020 4:19:33 AM)"=13428, "Automatic Update (DT: Olivine-3-1; HV: 2.2; Time: 1/3/2020 4:19:34 AM)"=13429, "Automatic Update (DT: Olivine-3-1; HV: 2.2; Time: 1/3/2020 4:19:35 AM)"=13430, "Automatic Update (DT: Olivine-3-1; HV: 2.2; Time: 1/3/2020 4:19:36 AM)"=13431, "Automatic Update (DT: Olivine-3-1; HV: 2.2; Time: 1/3/2020 4:19:38 AM)"=13432, "Automatic Update (DT: Olivine-3-1; HV: 2.2; Time: 1/3/2020 4:19:39 AM)"=13433, "Automatic Update (DT: Olivine-3-1; HV: 2.2; Time: 1/3/2020 4:19:40 AM)"=13434, "Automatic Update (DT: Olivine-3-1; HV: 2.2; Time: 1/3/2020 4:19:41 AM)"=13435, "Automatic Update (DT: Olivine-3-1; HV: 2.2; Time: 1/3/2020 4:19:42 AM)"=13436, "Automatic Update (DT: Olivine-3-1; HV: 2.2; Time: 1/3/2020 4:19:43 AM)"=13437, "Automatic Update (DT: Olivine-3-1; HV: 2.2; Time: 1/3/2020 4:19:44 AM)"=13438, "Automatic Update (DT: Olivine-3-1; HV: 2.2; Time: 1/3/2020 4:19:45 AM)"=13439, "Automatic Update (DT: Olivine-3-1; HV: 2.2; Time: 1/3/2020 4:19:46 AM)"=13440, "Automatic Update (DT: Olivine-3-1; HV: 2.2; Time: 1/3/2020 4:19:47 AM)"=13441, "Automatic Update (DT: Olivine-3-1; HV: 2.2; Time: 1/3/2020 4:19:48 AM)"=13442, "Automatic Update (DT: Olivine-3-1; HV: 2.2; Time: 1/3/2020 4:19:49 AM)"=13443, "Automatic Update (DT: Olivine-3-1; HV: 2.2; Time: 1/3/2020 4:19:50 AM)"=13444, "Automatic Update (DT: Olivine-3-1; HV: 2.2; Time: 1/3/2020 4:19:51 AM)"=13445, "Automatic Update (DT: Olivine-3-1; HV: 2.2; Time: 1/3/2020 4:19:52 AM)"=13446, "Automatic Update (DT: Olivine-3-1; HV: 2.2; Time: 1/3/2020 4:19:53 AM)"=13447, "Automatic Update (DT: Olivine-3-1; HV: 2.2; Time: 1/3/2020 4:19:54 AM)"=13448, "Automatic Update (DT: Olivine-3-1; HV: 2.2; Time: 1/3/2020 4:19:55 AM)"=13449, "Automatic Update (DT: Olivine-3-1; HV: 2.2; Time: 1/3/2020 4:19:56 AM)"=13450, "Automatic Update (DT: Olivine-3-1; HV: 2.2; Time: 1/3/2020 4:19:57 AM)"=13451, "Automatic Update (DT: Olivine-3-1; HV: 2.2; Time: 1/3/2020 4:19:58 AM)"=13452, "Automatic Update (DT: Olivine-3-1; HV: 2.2; Time: 1/3/2020 4:19:59 AM)"=13453, "Automatic Update (DT: Olivine-3-1; HV: 2.2; Time: 1/3/2020 4:20:01 AM)"=13454, "Automatic Update (DT: Olivine-3-1; HV: 2.2; Time: 1/3/2020 4:20:02 AM)"=13455, "Automatic Update (DT: Olivine-3-1; HV: 2.2; Time: 1/3/2020 4:20:03 AM)"=13456, "Automatic Update (DT: Olivine-3-1; HV: 2.2; Time: 1/3/2020 4:20:04 AM)"=13457, "Automatic Update (DT: Olivine-3-1; HV: 2.2; Time: 1/3/2020 4:20:05 AM)"=13458, "Automatic Update (DT: Olivine-3-1; HV: 2.2; Time: 1/3/2020 4:20:06 AM)"=13459, "Automatic Update (DT: Olivine-3-1; HV: 2.2; Time: 1/3/2020 4:20:07 AM)"=13460, "Automatic Update (DT: Olivine-3-1; HV: 2.2; Time: 1/3/2020 4:20:08 AM)"=13461, "Automatic Update (DT: Olivine-3-1; HV: 2.2; Time: 1/3/2020 4:20:09 AM)"=13462, "Automatic Update (DT: Olivine-3-1; HV: 2.2; Time: 1/3/2020 4:20:10 AM)"=13463, "Automatic Update (DT: Olivine-3-1; HV: 2.2; Time: 1/3/2020 4:20:11 AM)"=13464, "Automatic Update (DT: Olivine-3-1; HV: 2.2; Time: 1/3/2020 4:20:12 AM)"=13465, "Automatic Update (DT: Olivine-3-1; HV: 2.2; Time: 1/3/2020 4:20:13 AM)"=13466, "Automatic Update (DT: Olivine-3-1; HV: 2.2; Time: 1/3/2020 4:20:14 AM)"=13467, "Automatic Update (DT: Olivine-3-1; HV: 2.2; Time: 1/3/2020 4:20:15 AM)"=13468, "Automatic Update (DT: Olivine-3-1; HV: 2.2; Time: 1/3/2020 4:20:16 AM)"=13469, "Automatic Update (DT: Olivine-3-1; HV: 2.2; Time: 1/3/2020 4:20:17 AM)"=13470, "Automatic Update (DT: Olivine-3-1; HV: 2.2; Time: 1/3/2020 4:20:18 AM)"=13471, "Automatic Update (DT: Olivine-3-1; HV: 2.2; Time: 1/3/2020 4:20:19 AM)"=13472, "Automatic Update (DT: Olivine-3-1; HV: 2.2; Time: 1/3/2020 4:20:20 AM)"=13473, "Automatic Update (DT: Olivine-3-1; HV: 2.2; Time: 1/3/2020 4:20:22 AM)"=13474, "Automatic Update (DT: Olivine-3-1; HV: 2.2; Time: 1/3/2020 4:20:24 AM)"=13475, "Automatic Update (DT: Olivine-3-1; HV: 2.2; Time: 1/3/2020 4:20:25 AM)"=13476, "Automatic Update (DT: Olivine-3-1; HV: 2.2; Time: 1/3/2020 4:20:26 AM)"=13477, "Automatic Update (DT: Olivine-3-1; HV: 2.2; Time: 1/3/2020 4:20:27 AM)"=13478, "Automatic Update (DT: Olivine-3-1; HV: 2.2; Time: 1/3/2020 4:20:28 AM)"=13479, "Automatic Update (DT: Olivine-3-1; HV: 2.2; Time: 1/3/2020 4:20:29 AM)"=13480, "Automatic Update (DT: Olivine-3-1; HV: 2.2; Time: 1/3/2020 4:20:30 AM)"=13481, "Automatic Update (DT: Olivine-3-1; HV: 2.2; Time: 1/3/2020 4:20:31 AM)"=13482, "Automatic Update (DT: Olivine-3-1; HV: 2.2; Time: 1/3/2020 4:20:32 AM)"=13483, "Automatic Update (DT: Olivine-3-1; HV: 2.2; Time: 1/3/2020 4:20:33 AM)"=13484, "Automatic Update (DT: Olivine-3-1; HV: 2.2; Time: 1/3/2020 4:20:34 AM)"=13485, "Automatic Update (DT: Olivine-3-1; HV: 2.2; Time: 1/3/2020 4:20:35 AM)"=13486, "Automatic Update (DT: Olivine-3-1; HV: 2.2; Time: 1/3/2020 4:20:36 AM)"=13487, "Automatic Update (DT: Olivine-3-1; HV: 2.2; Time: 1/3/2020 4:20:37 AM)"=13488, "Automatic Update (DT: Olivine-3-1; HV: 2.2; Time: 1/3/2020 4:20:38 AM)"=13489, "Automatic Update (DT: Olivine-3-1; HV: 2.2; Time: 1/3/2020 4:20:39 AM)"=13490, "Automatic Update (DT: Olivine-3-1; HV: 2.2; Time: 1/3/2020 4:20:40 AM)"=13491, "Automatic Update (DT: Olivine-3-1; HV: 2.2; Time: 1/3/2020 4:20:41 AM)"=13492, "Automatic Update (DT: Olivine-3-1; HV: 2.2; Time: 1/3/2020 4:20:42 AM)"=13493, "Automatic Update (DT: Olivine-3-1; HV: 2.2; Time: 1/3/2020 4:20:43 AM)"=13494, "Automatic Update (DT: Olivine-3-1; HV: 2.2; Time: 1/3/2020 4:20:44 AM)"=13495, "Automatic Update (DT: Olivine-3-1; HV: 2.2; Time: 1/3/2020 4:20:45 AM)"=13496, "Automatic Update (DT: Olivine-3-1; HV: 2.2; Time: 1/3/2020 4:20:47 AM)"=13497, "Automatic Update (DT: Olivine-3-1; HV: 2.2; Time: 1/3/2020 4:20:48 AM)"=13498, "Automatic Update (DT: Olivine-3-1; HV: 2.2; Time: 1/3/2020 4:20:49 AM)"=13499, "Automatic Update (DT: Olivine-3-1; HV: 2.2; Time: 1/3/2020 4:20:50 AM)"=13500, "Automatic Update (DT: Olivine-3-1; HV: 2.2; Time: 1/3/2020 4:20:51 AM)"=13501, "Automatic Update (DT: Olivine-3-1; HV: 2.2; Time: 1/3/2020 4:20:52 AM)"=13502, "Automatic Update (DT: Olivine-3-1; HV: 2.2; Time: 1/3/2020 4:20:53 AM)"=13503, "Automatic Update (DT: Olivine-3-1; HV: 2.2; Time: 1/3/2020 4:20:54 AM)"=13504, "Automatic Update (DT: Olivine-3-1; HV: 2.2; Time: 1/3/2020 4:20:55 AM)"=13505, "Automatic Update (DT: Olivine-3-1; HV: 2.2; Time: 1/3/2020 4:20:56 AM)"=13506, "Automatic Update (DT: Olivine-3-1; HV: 2.2; Time: 1/3/2020 4:20:57 AM)"=13507, "Automatic Update (DT: Olivine-3-1; HV: 2.2; Time: 1/3/2020 4:20:58 AM)"=13508, "Automatic Update (DT: Olivine-3-1; HV: 2.2; Time: 1/3/2020 4:20:59 AM)"=13509, "Automatic Update (DT: Olivine-3-1; HV: 2.2; Time: 1/3/2020 4:21:00 AM)"=13510, "Automatic Update (DT: Olivine-3-1; HV: 2.2; Time: 1/3/2020 4:21:01 AM)"=13511, "Automatic Update (DT: Olivine-3-1; HV: 2.2; Time: 1/3/2020 4:21:02 AM)"=13512, "Automatic Update (DT: Olivine-3-1; HV: 2.2; Time: 1/3/2020 4:21:03 AM)"=13513, "Automatic Update (DT: Olivine-3-1; HV: 2.2; Time: 1/3/2020 4:21:04 AM)"=13514, "Automatic Update (DT: Olivine-3-1; HV: 2.2; Time: 1/3/2020 4:21:05 AM)"=13515, "Automatic Update (DT: Olivine-3-1; HV: 2.2; Time: 1/3/2020 4:21:07 AM)"=13516, "Automatic Update (DT: Olivine-3-1; HV: 2.2; Time: 1/3/2020 4:21:08 AM)"=13517, "Automatic Update (DT: Olivine-3-1; HV: 2.2; Time: 1/3/2020 4:21:09 AM)"=13518, "Automatic Update (DT: Olivine-3-1; HV: 2.2; Time: 1/3/2020 4:21:14 AM)"=13519, "Automatic Update (DT: Olivine-3-1; HV: 2.2; Time: 1/3/2020 4:21:15 AM)"=13520, "Automatic Update (DT: Olivine-3-1; HV: 2.2; Time: 1/3/2020 4:21:16 AM)"=13521, "Automatic Update (DT: Olivine-3-1; HV: 2.2; Time: 1/3/2020 4:21:18 AM)"=13522, "Automatic Update (DT: Olivine-3-1; HV: 2.2; Time: 1/3/2020 4:21:19 AM)"=13523, "Automatic Update (DT: Olivine-3-1; HV: 2.2; Time: 1/3/2020 4:21:20 AM)"=13524, "Automatic Update (DT: Olivine-3-1; HV: 2.2; Time: 1/3/2020 4:21:21 AM)"=13525, "Automatic Update (DT: Olivine-3-1; HV: 2.2; Time: 1/3/2020 4:21:22 AM)"=13526, "Automatic Update (DT: Olivine-3-1; HV: 2.2; Time: 1/3/2020 4:21:23 AM)"=13527, "Automatic Update (DT: Olivine-3-1; HV: 2.2; Time: 1/3/2020 4:21:24 AM)"=13528, "Automatic Update (DT: Olivine-3-1; HV: 2.2; Time: 1/3/2020 4:21:25 AM)"=13529, "Automatic Update (DT: Olivine-3-1; HV: 2.2; Time: 1/3/2020 4:21:26 AM)"=13530, "Automatic Update (DT: Olivine-3-1; HV: 2.2; Time: 1/3/2020 4:21:27 AM)"=13531, "Automatic Update (DT: Olivine-3-1; HV: 2.2; Time: 1/3/2020 4:21:28 AM)"=13532, "Automatic Update (DT: Olivine-3-1; HV: 2.2; Time: 1/3/2020 4:21:29 AM)"=13533, "Automatic Update (DT: Olivine-3-1; HV: 2.2; Time: 1/3/2020 4:21:30 AM)"=13534, "Automatic Update (DT: Olivine-3-1; HV: 2.2; Time: 1/3/2020 4:21:31 AM)"=13535, "Automatic Update (DT: Olivine-3-1; HV: 2.2; Time: 1/3/2020 4:21:33 AM)"=13536, "Automatic Update (DT: Olivine-3-1; HV: 2.2; Time: 1/3/2020 4:21:34 AM)"=13537, "Automatic Update (DT: Olivine-3-1; HV: 2.2; Time: 1/3/2020 4:21:35 AM)"=13538, "Automatic Update (DT: Olivine-3-1; HV: 2.2; Time: 1/3/2020 4:21:36 AM)"=13539, "Automatic Update (DT: Olivine-3-1; HV: 2.2; Time: 1/3/2020 4:21:37 AM)"=13540, "Automatic Update (DT: Olivine-3-1; HV: 2.2; Time: 1/3/2020 4:21:38 AM)"=13541, "Automatic Update (DT: Olivine-3-1; HV: 2.2; Time: 1/3/2020 4:21:39 AM)"=13542, "Automatic Update (DT: Olivine-3-1; HV: 2.2; Time: 1/3/2020 4:21:40 AM)"=13543, "Automatic Update (DT: Olivine-3-1; HV: 2.2; Time: 1/3/2020 4:21:41 AM)"=13544, "Automatic Update (DT: Olivine-3-1; HV: 2.2; Time: 1/3/2020 4:21:42 AM)"=13545, "Automatic Update (DT: Olivine-3-1; HV: 2.2; Time: 1/3/2020 4:21:43 AM)"=13546, "Automatic Update (DT: Olivine-3-1; HV: 2.2; Time: 1/3/2020 4:21:44 AM)"=13547, "Automatic Update (DT: Olivine-3-1; HV: 2.2; Time: 1/3/2020 4:21:45 AM)"=13548, "Automatic Update (DT: Olivine-3-1; HV: 2.2; Time: 1/3/2020 4:21:46 AM)"=13549, "Automatic Update (DT: Olivine-3-1; HV: 2.2; Time: 1/3/2020 4:21:47 AM)"=13550, "Automatic Update (DT: Olivine-3-1; HV: 2.2; Time: 1/3/2020 4:21:48 AM)"=13551, "Automatic Update (DT: Olivine-3-1; HV: 2.2; Time: 1/3/2020 4:21:49 AM)"=13552, "Automatic Update (DT: Olivine-3-1; HV: 2.2; Time: 1/3/2020 4:21:50 AM)"=13553, "Automatic Update (DT: Olivine-3-1; HV: 2.2; Time: 1/3/2020 4:21:51 AM)"=13554, "Automatic Update (DT: Olivine-3-1; HV: 2.2; Time: 1/3/2020 4:21:52 AM)"=13555, "Automatic Update (DT: Olivine-3-1; HV: 2.2; Time: 1/3/2020 4:21:53 AM)"=13556, "Automatic Update (DT: Olivine-3-1; HV: 2.2; Time: 1/3/2020 4:21:55 AM)"=13557, "Automatic Update (DT: Olivine-3-1; HV: 2.2; Time: 1/3/2020 4:21:56 AM)"=13558, "Automatic Update (DT: Olivine-3-1; HV: 2.2; Time: 1/3/2020 4:21:57 AM)"=13559, "Automatic Update (DT: Olivine-3-1; HV: 2.2; Time: 1/3/2020 4:21:58 AM)"=13560, "Automatic Update (DT: Olivine-3-1; HV: 2.2; Time: 1/3/2020 4:21:59 AM)"=13561, "Automatic Update (DT: Olivine-3-1; HV: 2.2; Time: 1/3/2020 4:22:00 AM)"=13562, "Automatic Update (DT: Olivine-3-1; HV: 2.2; Time: 1/3/2020 4:22:01 AM)"=13563, "Automatic Update (DT: Olivine-3-1; HV: 2.2; Time: 1/3/2020 4:22:02 AM)"=13564, "Automatic Update (DT: Olivine-3-1; HV: 2.2; Time: 1/3/2020 4:22:03 AM)"=13565, "Automatic Update (DT: Olivine-3-1; HV: 2.2; Time: 1/3/2020 4:22:04 AM)"=13566, "Automatic Update (DT: Olivine-3-1; HV: 2.2; Time: 1/3/2020 4:22:05 AM)"=13567, "Automatic Update (DT: Olivine-3-1; HV: 2.2; Time: 1/3/2020 4:22:08 AM)"=13568, "Automatic Update (DT: Olivine-3-1; HV: 2.2; Time: 1/3/2020 4:22:09 AM)"=13569, "Automatic Update (DT: Olivine-3-1; HV: 2.2; Time: 1/3/2020 4:22:10 AM)"=13570, "Automatic Update (DT: Olivine-3-1; HV: 2.2; Time: 1/3/2020 4:22:11 AM)"=13571, "Automatic Update (DT: Olivine-3-1; HV: 2.2; Time: 1/3/2020 4:22:12 AM)"=13572, "Automatic Update (DT: Olivine-3-1; HV: 2.2; Time: 1/3/2020 4:22:13 AM)"=13573, "Automatic Update (DT: Olivine-3-1; HV: 2.2; Time: 1/3/2020 4:22:15 AM)"=13574, "Automatic Update (DT: Olivine-3-1; HV: 2.2; Time: 1/3/2020 4:22:16 AM)"=13575, "Automatic Update (DT: Olivine-3-1; HV: 2.2; Time: 1/3/2020 4:22:18 AM)"=13576, "Automatic Update (DT: Olivine-3-1; HV: 2.2; Time: 1/3/2020 4:22:19 AM)"=13577, "Automatic Update (DT: Olivine-3-1; HV: 2.2; Time: 1/3/2020 4:22:21 AM)"=13578, "Automatic Update (DT: Olivine-3-1; HV: 2.2; Time: 1/3/2020 4:22:22 AM)"=13579, "Automatic Update (DT: Olivine-3-1; HV: 2.2; Time: 1/3/2020 4:22:23 AM)"=13580, "Automatic Update (DT: Olivine-3-1; HV: 2.2; Time: 1/3/2020 4:22:24 AM)"=13581, "Automatic Update (DT: Olivine-3-1; HV: 2.2; Time: 1/3/2020 4:22:25 AM)"=13582, "Automatic Update (DT: Olivine-3-1; HV: 2.2; Time: 1/3/2020 4:22:26 AM)"=13583, "Automatic Update (DT: Olivine-3-1; HV: 2.2; Time: 1/3/2020 4:22:27 AM)"=13584, "Automatic Update (DT: Olivine-3-1; HV: 2.2; Time: 1/3/2020 4:22:28 AM)"=13585, "Automatic Update (DT: Olivine-3-1; HV: 2.2; Time: 1/3/2020 4:22:29 AM)"=13586, "Automatic Update (DT: Olivine-3-1; HV: 2.2; Time: 1/3/2020 4:22:30 AM)"=13587, "Automatic Update (DT: Olivine-3-1; HV: 2.2; Time: 1/3/2020 4:22:31 AM)"=13588, "Automatic Update (DT: Olivine-3-1; HV: 2.2; Time: 1/3/2020 4:22:32 AM)"=13589, "Automatic Update (DT: Olivine-3-1; HV: 2.2; Time: 1/3/2020 4:22:33 AM)"=13590, "Automatic Update (DT: Olivine-3-1; HV: 2.2; Time: 1/3/2020 4:22:34 AM)"=13591, "Automatic Update (DT: Olivine-3-1; HV: 2.2; Time: 1/3/2020 4:22:35 AM)"=13592, "Automatic Update (DT: Olivine-3-1; HV: 2.2; Time: 1/3/2020 4:22:36 AM)"=13593, "Automatic Update (DT: Olivine-3-1; HV: 2.2; Time: 1/3/2020 4:22:37 AM)"=13594, "Automatic Update (DT: Olivine-3-1; HV: 2.2; Time: 1/3/2020 4:22:38 AM)"=13595, "Automatic Update (DT: Olivine-3-1; HV: 2.2; Time: 1/3/2020 4:22:39 AM)"=13596, "Automatic Update (DT: Olivine-3-1; HV: 2.2; Time: 1/3/2020 4:22:41 AM)"=13597, "Automatic Update (DT: Olivine-3-1; HV: 2.2; Time: 1/3/2020 4:22:42 AM)"=13598, "Automatic Update (DT: Olivine-3-1; HV: 2.2; Time: 1/3/2020 4:22:43 AM)"=13599, "Automatic Update (DT: Olivine-3-1; HV: 2.2; Time: 1/3/2020 4:22:44 AM)"=13600, "Automatic Update (DT: Olivine-3-1; HV: 2.2; Time: 1/3/2020 4:22:45 AM)"=13601, "Automatic Update (DT: Olivine-3-1; HV: 2.2; Time: 1/3/2020 4:22:46 AM)"=13602, "Automatic Update (DT: Olivine-3-1; HV: 2.2; Time: 1/3/2020 4:22:47 AM)"=13603, "Automatic Update (DT: Olivine-3-1; HV: 2.2; Time: 1/3/2020 4:22:48 AM)"=13604, "Automatic Update (DT: Olivine-3-1; HV: 2.2; Time: 1/3/2020 4:22:49 AM)"=13605, "Automatic Update (DT: Olivine-3-1; HV: 2.2; Time: 1/3/2020 4:22:50 AM)"=13606, "Automatic Update (DT: Olivine-3-1; HV: 2.2; Time: 1/3/2020 4:22:51 AM)"=13607, "Automatic Update (DT: Olivine-3-1; HV: 2.2; Time: 1/3/2020 4:22:52 AM)"=13608, "Automatic Update (DT: Olivine-3-1; HV: 2.2; Time: 1/3/2020 4:22:53 AM)"=13609, "Automatic Update (DT: Olivine-3-1; HV: 2.2; Time: 1/3/2020 4:22:54 AM)"=13610, "Automatic Update (DT: Olivine-3-1; HV: 2.2; Time: 1/3/2020 4:22:55 AM)"=13611, "Automatic Update (DT: Olivine-3-1; HV: 2.2; Time: 1/3/2020 4:22:56 AM)"=13612, "Automatic Update (DT: Olivine-3-1; HV: 2.2; Time: 1/3/2020 4:22:57 AM)"=13613, "Automatic Update (DT: Olivine-3-1; HV: 2.2; Time: 1/3/2020 4:22:58 AM)"=13614, "Automatic Update (DT: Olivine-3-1; HV: 2.2; Time: 1/3/2020 4:22:59 AM)"=13615, "Automatic Update (DT: Olivine-3-1; HV: 2.2; Time: 1/3/2020 4:23:00 AM)"=13616, "Automatic Update (DT: Olivine-3-1; HV: 2.2; Time: 1/3/2020 4:23:01 AM)"=13617, "Automatic Update (DT: Olivine-3-1; HV: 2.2; Time: 1/3/2020 4:23:02 AM)"=13618, "Automatic Update (DT: Olivine-3-1; HV: 2.2; Time: 1/3/2020 4:23:04 AM)"=13619, "Automatic Update (DT: Olivine-3-1; HV: 2.2; Time: 1/3/2020 4:23:05 AM)"=13620, "Automatic Update (DT: Olivine-3-1; HV: 2.2; Time: 1/3/2020 4:23:06 AM)"=13621, "Automatic Update (DT: Olivine-3-1; HV: 2.2; Time: 1/3/2020 4:23:07 AM)"=13622, "Automatic Update (DT: Olivine-3-1; HV: 2.2; Time: 1/3/2020 4:23:08 AM)"=13623, "Automatic Update (DT: Olivine-3-1; HV: 2.2; Time: 1/3/2020 4:23:09 AM)"=13624, "Automatic Update (DT: Olivine-3-1; HV: 2.2; Time: 1/3/2020 4:23:10 AM)"=13625, "Automatic Update (DT: Olivine-3-1; HV: 2.2; Time: 1/3/2020 4:23:11 AM)"=13626, "Automatic Update (DT: Olivine-3-1; HV: 2.2; Time: 1/3/2020 4:23:12 AM)"=13627, "Automatic Update (DT: Olivine-3-1; HV: 2.2; Time: 1/3/2020 4:23:13 AM)"=13628, "Automatic Update (DT: Olivine-3-1; HV: 2.2; Time: 1/3/2020 4:23:28 AM)"=13629, "Automatic Update (DT: Olivine-3-1; HV: 2.2; Time: 1/3/2020 10:09:46 AM)"=13630, "Automatic Update (DT: Olivine-3-1; HV: 2.2; Time: 1/3/2020 10:09:53 AM)"=13631, "Automatic Update (DT: Olivine-3-1; HV: 2.2; Time: 1/3/2020 10:09:56 AM)"=13632, "Automatic Update (DT: Olivine-3-1; HV: 2.2; Time: 1/3/2020 10:10:15 AM)"=13633, "Automatic Update (DT: Olivine-3-1; HV: 2.2; Time: 1/3/2020 10:10:24 AM)"=13634, "Automatic Update (DT: Olivine-3-1; HV: 2.2; Time: 1/3/2020 10:10:28 AM)"=13635, "Automatic Update (DT: Olivine-3-1; HV: 2.2; Time: 1/3/2020 10:10:30 AM)"=13636, "Automatic Update (DT: Olivine-3-1; HV: 2.2; Time: 1/3/2020 10:10:32 AM)"=13637, "Automatic Update (DT: Olivine-3-1; HV: 2.2; Time: 1/3/2020 10:10:34 AM)"=13638, "Automatic Update (DT: Olivine-3-1; HV: 2.2; Time: 1/3/2020 10:10:36 AM)"=13639, "Automatic Update (DT: Olivine-3-1; HV: 2.2; Time: 1/3/2020 10:10:37 AM)"=13640, "Automatic Update (DT: Olivine-3-1; HV: 2.2; Time: 1/3/2020 10:10:39 AM)"=13641, "Automatic Update (DT: Olivine-3-1; HV: 2.2; Time: 1/3/2020 10:10:41 AM)"=13642, "Automatic Update (DT: Olivine-3-1; HV: 2.2; Time: 1/3/2020 10:10:42 AM)"=13643, "Automatic Update (DT: Olivine-3-1; HV: 2.2; Time: 1/3/2020 10:10:43 AM)"=13644, "Automatic Update (DT: Olivine-3-1; HV: 2.2; Time: 1/3/2020 10:10:47 AM)"=13645, "Automatic Update (DT: Olivine-3-1; HV: 2.2; Time: 1/3/2020 10:10:49 AM)"=13646, "Automatic Update (DT: Olivine-3-1; HV: 2.2; Time: 1/3/2020 10:10:50 AM)"=13647, "Automatic Update (DT: Olivine-3-1; HV: 2.2; Time: 1/3/2020 10:10:52 AM)"=13648, "Automatic Update (DT: Olivine-3-1; HV: 2.2; Time: 1/3/2020 10:10:55 AM)"=13649, "Automatic Update (DT: Olivine-3-1; HV: 2.2; Time: 1/3/2020 10:10:58 AM)"=13650, "Automatic Update (DT: Olivine-3-1; HV: 2.2; Time: 1/3/2020 10:11:00 AM)"=13651, "Automatic Update (DT: Olivine-3-1; HV: 2.2; Time: 1/3/2020 10:11:01 AM)"=13652, "Automatic Update (DT: Olivine-3-1; HV: 2.2; Time: 1/3/2020 10:11:03 AM)"=13653, "Automatic Update (DT: Olivine-3-1; HV: 2.2; Time: 1/3/2020 10:11:05 AM)"=13654, "Automatic Update (DT: Olivine-3-1; HV: 2.2; Time: 1/3/2020 10:11:08 AM)"=13655, "Automatic Update (DT: Olivine-3-1; HV: 2.2; Time: 1/3/2020 10:11:09 AM)"=13656, "Automatic Update (DT: Olivine-3-1; HV: 2.2; Time: 1/3/2020 10:11:10 AM)"=13657, "Automatic Update (DT: Olivine-3-1; HV: 2.2; Time: 1/3/2020 10:11:11 AM)"=13658, "Automatic Update (DT: Olivine-3-1; HV: 2.2; Time: 1/3/2020 10:11:12 AM)"=13659, "Automatic Update (DT: Olivine-3-1; HV: 2.2; Time: 1/3/2020 10:11:13 AM)"=13660, "Automatic Update (DT: Olivine-3-1; HV: 2.2; Time: 1/3/2020 10:11:15 AM)"=13661, "Automatic Update (DT: Olivine-3-1; HV: 2.2; Time: 1/3/2020 10:11:16 AM)"=13662, "Automatic Update (DT: Olivine-3-1; HV: 2.2; Time: 1/3/2020 10:11:17 AM)"=13663, "Automatic Update (DT: Olivine-3-1; HV: 2.2; Time: 1/3/2020 10:11:18 AM)"=13664, "Automatic Update (DT: Olivine-3-1; HV: 2.2; Time: 1/3/2020 10:11:19 AM)"=13665, "Automatic Update (DT: Olivine-3-1; HV: 2.2; Time: 1/3/2020 10:11:20 AM)"=13666, "Automatic Update (DT: Olivine-3-1; HV: 2.2; Time: 1/3/2020 10:11:21 AM)"=13667, "Automatic Update (DT: Olivine-3-1; HV: 2.2; Time: 1/3/2020 10:11:22 AM)"=13668, "Automatic Update (DT: Olivine-3-1; HV: 2.2; Time: 1/3/2020 10:11:23 AM)"=13669, "Automatic Update (DT: Olivine-3-1; HV: 2.2; Time: 1/3/2020 10:11:24 AM)"=13670, "Automatic Update (DT: Olivine-3-1; HV: 2.2; Time: 1/3/2020 10:11:25 AM)"=13671, "Automatic Update (DT: Olivine-3-1; HV: 2.2; Time: 1/3/2020 10:11:26 AM)"=13672, "Automatic Update (DT: Olivine-3-1; HV: 2.2; Time: 1/3/2020 10:11:27 AM)"=13673, "Automatic Update (DT: Olivine-3-1; HV: 2.2; Time: 1/3/2020 10:11:28 AM)"=13674, "Automatic Update (DT: Olivine-3-1; HV: 2.2; Time: 1/3/2020 10:11:29 AM)"=13675, "Automatic Update (DT: Olivine-3-1; HV: 2.2; Time: 1/3/2020 10:11:30 AM)"=13676, "Automatic Update (DT: Olivine-3-1; HV: 2.2; Time: 1/3/2020 10:11:31 AM)"=13677, "Automatic Update (DT: Olivine-3-1; HV: 2.2; Time: 1/3/2020 10:11:32 AM)"=13678, "Automatic Update (DT: Olivine-3-1; HV: 2.2; Time: 1/3/2020 10:11:34 AM)"=13679, "Automatic Update (DT: Olivine-3-1; HV: 2.2; Time: 1/3/2020 10:11:35 AM)"=13680, "Automatic Update (DT: Olivine-3-1; HV: 2.2; Time: 1/3/2020 10:11:36 AM)"=13681, "Automatic Update (DT: Olivine-3-1; HV: 2.2; Time: 1/3/2020 10:11:37 AM)"=13682, "Automatic Update (DT: Olivine-3-1; HV: 2.2; Time: 1/3/2020 10:11:39 AM)"=13683, "Automatic Update (DT: Olivine-3-1; HV: 2.2; Time: 1/3/2020 10:11:40 AM)"=13684, "Automatic Update (DT: Olivine-3-1; HV: 2.2; Time: 1/3/2020 10:11:41 AM)"=13685, "Automatic Update (DT: Olivine-3-1; HV: 2.2; Time: 1/3/2020 10:11:42 AM)"=13686, "Automatic Update (DT: Olivine-3-1; HV: 2.2; Time: 1/3/2020 10:11:43 AM)"=13687, "Automatic Update (DT: Olivine-3-1; HV: 2.2; Time: 1/3/2020 10:11:44 AM)"=13688, "Automatic Update (DT: Olivine-3-1; HV: 2.2; Time: 1/3/2020 10:11:45 AM)"=13689, "Automatic Update (DT: Olivine-3-1; HV: 2.2; Time: 1/3/2020 10:11:50 AM)"=13690, "Automatic Update (DT: Olivine-3-1; HV: 2.2; Time: 1/3/2020 10:11:52 AM)"=13691, "Automatic Update (DT: Olivine-3-1; HV: 2.2; Time: 1/3/2020 10:11:56 AM)"=13692, "Automatic Update (DT: Olivine-3-1; HV: 2.2; Time: 1/3/2020 10:11:57 AM)"=13693, "Automatic Update (DT: Olivine-3-1; HV: 2.2; Time: 1/3/2020 10:11:58 AM)"=13694, "Automatic Update (DT: Olivine-3-1; HV: 2.2; Time: 1/3/2020 10:11:59 AM)"=13695, "Automatic Update (DT: Olivine-3-1; HV: 2.2; Time: 1/3/2020 10:12:00 AM)"=13696, "Automatic Update (DT: Olivine-3-1; HV: 2.2; Time: 1/3/2020 10:12:01 AM)"=13697, "Automatic Update (DT: Olivine-3-1; HV: 2.2; Time: 1/3/2020 10:12:02 AM)"=13698, "Automatic Update (DT: Olivine-3-1; HV: 2.2; Time: 1/3/2020 10:12:03 AM)"=13699, "Automatic Update (DT: Olivine-3-1; HV: 2.2; Time: 1/3/2020 10:12:04 AM)"=13700, "Automatic Update (DT: Olivine-3-1; HV: 2.2; Time: 1/3/2020 10:12:05 AM)"=13701, "Automatic Update (DT: Olivine-3-1; HV: 2.2; Time: 1/3/2020 10:12:06 AM)"=13702, "Automatic Update (DT: Olivine-3-1; HV: 2.2; Time: 1/3/2020 10:12:08 AM)"=13703, "Automatic Update (DT: Olivine-3-1; HV: 2.2; Time: 1/3/2020 10:12:09 AM)"=13704, "Automatic Update (DT: Olivine-3-1; HV: 2.2; Time: 1/3/2020 10:12:10 AM)"=13705, "Automatic Update (DT: Olivine-3-1; HV: 2.2; Time: 1/3/2020 10:12:12 AM)"=13706, "Automatic Update (DT: Olivine-3-1; HV: 2.2; Time: 1/3/2020 10:12:13 AM)"=13707, "Automatic Update (DT: Olivine-3-1; HV: 2.2; Time: 1/3/2020 10:12:19 AM)"=13708, "Automatic Update (DT: Olivine-3-1; HV: 2.2; Time: 1/3/2020 10:12:25 AM)"=13709, "Automatic Update (DT: Olivine-3-1; HV: 2.2; Time: 1/3/2020 10:12:28 AM)"=13710, "Automatic Update (DT: Olivine-3-1; HV: 2.2; Time: 1/3/2020 10:12:30 AM)"=13711, "Automatic Update (DT: Olivine-3-1; HV: 2.2; Time: 1/3/2020 10:12:34 AM)"=13712, "Automatic Update (DT: Olivine-3-1; HV: 2.2; Time: 1/3/2020 10:12:47 AM)"=13713, "Automatic Update (DT: Olivine-3-1; HV: 2.2; Time: 1/3/2020 10:12:48 AM)"=13714, "Automatic Update (DT: Olivine-3-1; HV: 2.2; Time: 1/3/2020 10:12:49 AM)"=13715, "Automatic Update (DT: Olivine-3-1; HV: 2.2; Time: 1/3/2020 10:12:50 AM)"=13716, "Automatic Update (DT: Olivine-3-1; HV: 2.2; Time: 1/3/2020 10:12:51 AM)"=13717, "Automatic Update (DT: Olivine-3-1; HV: 2.2; Time: 1/3/2020 10:12:52 AM)"=13718, "Automatic Update (DT: Olivine-3-1; HV: 2.2; Time: 1/3/2020 10:12:53 AM)"=13719, "Automatic Update (DT: Olivine-3-1; HV: 2.2; Time: 1/3/2020 10:12:54 AM)"=13720, "Automatic Update (DT: Olivine-3-1; HV: 2.2; Time: 1/3/2020 10:12:55 AM)"=13721, "Automatic Update (DT: Olivine-3-1; HV: 2.2; Time: 1/3/2020 10:12:58 AM)"=13722, "Automatic Update (DT: Olivine-3-1; HV: 2.2; Time: 1/3/2020 10:12:59 AM)"=13723, "Automatic Update (DT: Olivine-3-1; HV: 2.2; Time: 1/3/2020 10:13:00 AM)"=13724, "Automatic Update (DT: Olivine-3-1; HV: 2.2; Time: 1/3/2020 10:13:01 AM)"=13725, "Automatic Update (DT: Olivine-3-1; HV: 2.2; Time: 1/3/2020 10:13:02 AM)"=13726, "Automatic Update (DT: Olivine-3-1; HV: 2.2; Time: 1/3/2020 10:13:03 AM)"=13727, "Automatic Update (DT: Olivine-3-1; HV: 2.2; Time: 1/3/2020 10:13:04 AM)"=13728, "Automatic Update (DT: Olivine-3-1; HV: 2.2; Time: 1/3/2020 10:13:05 AM)"=13729, "Automatic Update (DT: Olivine-3-1; HV: 2.2; Time: 1/3/2020 10:13:06 AM)"=13730, "Automatic Update (DT: Olivine-3-1; HV: 2.2; Time: 1/3/2020 10:13:07 AM)"=13731, "Automatic Update (DT: Olivine-3-1; HV: 2.2; Time: 1/3/2020 10:13:08 AM)"=13732, "Automatic Update (DT: Olivine-3-1; HV: 2.2; Time: 1/3/2020 10:13:09 AM)"=13733, "Automatic Update (DT: Olivine-3-1; HV: 2.2; Time: 1/3/2020 10:13:11 AM)"=13734, "Automatic Update (DT: Olivine-3-1; HV: 2.2; Time: 1/3/2020 10:13:12 AM)"=13735, "Automatic Update (DT: Olivine-3-1; HV: 2.2; Time: 1/3/2020 10:13:13 AM)"=13736, "Automatic Update (DT: Olivine-3-1; HV: 2.2; Time: 1/3/2020 10:13:14 AM)"=13737, "Automatic Update (DT: Olivine-3-1; HV: 2.2; Time: 1/3/2020 10:13:16 AM)"=13738, "Automatic Update (DT: Olivine-3-1; HV: 2.2; Time: 1/3/2020 10:13:17 AM)"=13739, "Automatic Update (DT: Olivine-3-1; HV: 2.2; Time: 1/3/2020 10:13:18 AM)"=13740, "Automatic Update (DT: Olivine-3-1; HV: 2.2; Time: 1/3/2020 10:13:19 AM)"=13741, "Automatic Update (DT: Olivine-3-1; HV: 2.2; Time: 1/3/2020 10:13:20 AM)"=13742, "Automatic Update (DT: Olivine-3-1; HV: 2.2; Time: 1/3/2020 10:13:21 AM)"=13743, "Automatic Update (DT: Olivine-3-1; HV: 2.2; Time: 1/3/2020 10:13:23 AM)"=13744, "Automatic Update (DT: Olivine-3-1; HV: 2.2; Time: 1/3/2020 10:13:24 AM)"=13745, "Automatic Update (DT: Olivine-3-1; HV: 2.2; Time: 1/3/2020 10:13:25 AM)"=13746, "Automatic Update (DT: Olivine-3-1; HV: 2.2; Time: 1/3/2020 10:13:26 AM)"=13747, "Automatic Update (DT: Olivine-3-1; HV: 2.2; Time: 1/3/2020 10:13:27 AM)"=13748, "Automatic Update (DT: Olivine-3-1; HV: 2.2; Time: 1/3/2020 10:13:28 AM)"=13749, "Automatic Update (DT: Olivine-3-1; HV: 2.2; Time: 1/3/2020 10:13:29 AM)"=13750, "Automatic Update (DT: Olivine-3-1; HV: 2.2; Time: 1/3/2020 10:13:30 AM)"=13751, "Automatic Update (DT: Olivine-3-1; HV: 2.2; Time: 1/3/2020 10:13:31 AM)"=13752, "Automatic Update (DT: Olivine-3-1; HV: 2.2; Time: 1/3/2020 10:13:32 AM)"=13753, "Automatic Update (DT: Olivine-3-1; HV: 2.2; Time: 1/3/2020 10:13:33 AM)"=13754, "Automatic Update (DT: Olivine-3-1; HV: 2.2; Time: 1/3/2020 10:13:34 AM)"=13755, "Automatic Update (DT: Olivine-3-1; HV: 2.2; Time: 1/3/2020 10:13:35 AM)"=13756, "Automatic Update (DT: Olivine-3-1; HV: 2.2; Time: 1/3/2020 10:13:37 AM)"=13757, "Automatic Update (DT: Olivine-3-1; HV: 2.2; Time: 1/3/2020 10:13:41 AM)"=13758, "Automatic Update (DT: Olivine-3-1; HV: 2.2; Time: 1/3/2020 10:13:42 AM)"=13759, "Automatic Update (DT: Olivine-3-1; HV: 2.2; Time: 1/3/2020 10:13:43 AM)"=13760, "Automatic Update (DT: Olivine-3-1; HV: 2.2; Time: 1/3/2020 10:13:49 AM)"=13761, "Automatic Update (DT: Olivine-3-1; HV: 2.2; Time: 1/3/2020 10:13:50 AM)"=13762, "Automatic Update (DT: Olivine-3-1; HV: 2.2; Time: 1/3/2020 10:13:51 AM)"=13763, "Automatic Update (DT: Olivine-3-1; HV: 2.2; Time: 1/3/2020 10:13:53 AM)"=13764, "Automatic Update (DT: Olivine-3-1; HV: 2.2; Time: 1/3/2020 10:13:58 AM)"=13765, "Automatic Update (DT: Olivine-3-1; HV: 2.2; Time: 1/3/2020 10:13:59 AM)"=13766, "Automatic Update (DT: Olivine-3-1; HV: 2.2; Time: 1/3/2020 10:14:00 AM)"=13767, "Automatic Update (DT: Olivine-3-1; HV: 2.2; Time: 1/3/2020 10:14:01 AM)"=13768, "Automatic Update (DT: Olivine-3-1; HV: 2.2; Time: 1/3/2020 10:14:04 AM)"=13769, "Automatic Update (DT: Olivine-3-1; HV: 2.2; Time: 1/3/2020 10:14:05 AM)"=13770, "Automatic Update (DT: Olivine-3-1; HV: 2.2; Time: 1/3/2020 10:14:06 AM)"=13771, "Automatic Update (DT: Olivine-3-1; HV: 2.2; Time: 1/3/2020 10:14:07 AM)"=13772, "Automatic Update (DT: Olivine-3-1; HV: 2.2; Time: 1/3/2020 10:14:28 AM)"=13773, "Automatic Update (DT: Olivine-3-1; HV: 2.2; Time: 1/3/2020 10:14:29 AM)"=13774, "Automatic Update (DT: Olivine-3-1; HV: 2.2; Time: 1/3/2020 10:14:30 AM)"=13775, "Automatic Update (DT: Olivine-3-1; HV: 2.2; Time: 1/3/2020 10:14:37 AM)"=13776, "Automatic Update (DT: Olivine-3-1; HV: 2.2; Time: 1/3/2020 10:14:38 AM)"=13777, "Automatic Update (DT: Olivine-3-1; HV: 2.2; Time: 1/3/2020 10:14:39 AM)"=13778, "Automatic Update (DT: Olivine-3-1; HV: 2.2; Time: 1/3/2020 10:14:40 AM)"=13779, "Automatic Update (DT: Olivine-3-1; HV: 2.2; Time: 1/3/2020 10:14:43 AM)"=13780, "Automatic Update (DT: Olivine-3-1; HV: 2.2; Time: 1/3/2020 10:14:44 AM)"=13781, "Automatic Update (DT: Olivine-3-1; HV: 2.2; Time: 1/3/2020 10:14:45 AM)"=13782, "Automatic Update (DT: Olivine-3-1; HV: 2.2; Time: 1/3/2020 10:14:46 AM)"=13783, "Automatic Update (DT: Olivine-3-1; HV: 2.2; Time: 1/3/2020 10:14:49 AM)"=13784, "Automatic Update (DT: Olivine-3-1; HV: 2.2; Time: 1/3/2020 10:14:50 AM)"=13785, "Automatic Update (DT: Olivine-3-1; HV: 2.2; Time: 1/3/2020 10:14:51 AM)"=13786, "Automatic Update (DT: Olivine-3-1; HV: 2.2; Time: 1/3/2020 10:14:52 AM)"=13787, "Automatic Update (DT: Olivine-3-1; HV: 2.2; Time: 1/3/2020 10:15:02 AM)"=13788, "Automatic Update (DT: Olivine-3-1; HV: 2.2; Time: 1/3/2020 10:15:03 AM)"=13789, "Automatic Update (DT: Olivine-3-1; HV: 2.2; Time: 1/3/2020 10:15:04 AM)"=13790, "Automatic Update (DT: Olivine-3-1; HV: 2.2; Time: 1/3/2020 10:15:14 AM)"=13791, "Automatic Update (DT: Olivine-3-1; HV: 2.2; Time: 1/3/2020 10:15:15 AM)"=13792, "Automatic Update (DT: Olivine-3-1; HV: 2.2; Time: 1/3/2020 10:15:16 AM)"=13793, "Automatic Update (DT: Olivine-3-1; HV: 2.2; Time: 1/3/2020 10:15:17 AM)"=13794, "Automatic Update (DT: Olivine-3-1; HV: 2.2; Time: 1/3/2020 10:15:21 AM)"=13795, "Automatic Update (DT: Olivine-3-1; HV: 2.2; Time: 1/3/2020 10:15:22 AM)"=13796, "Automatic Update (DT: Olivine-3-1; HV: 2.2; Time: 1/3/2020 10:15:23 AM)"=13797, "Automatic Update (DT: Olivine-3-1; HV: 2.2; Time: 1/3/2020 10:15:24 AM)"=13798, "Automatic Update (DT: Olivine-3-1; HV: 2.2; Time: 1/3/2020 10:15:25 AM)"=13799, "Automatic Update (DT: Olivine-3-1; HV: 2.2; Time: 1/3/2020 10:15:26 AM)"=13800, "Automatic Update (DT: Olivine-3-1; HV: 2.2; Time: 1/3/2020 10:15:27 AM)"=13801, "Automatic Update (DT: Olivine-3-1; HV: 2.2; Time: 1/3/2020 10:15:28 AM)"=13802, "Automatic Update (DT: Olivine-3-1; HV: 2.2; Time: 1/3/2020 10:15:29 AM)"=13803, "Automatic Update (DT: Olivine-3-1; HV: 2.2; Time: 1/3/2020 10:15:31 AM)"=13804, "Automatic Update (DT: Olivine-3-1; HV: 2.2; Time: 1/3/2020 10:15:32 AM)"=13805, "Automatic Update (DT: Olivine-3-1; HV: 2.2; Time: 1/3/2020 10:15:33 AM)"=13806, "Automatic Update (DT: Olivine-3-1; HV: 2.2; Time: 1/3/2020 10:15:34 AM)"=13807, "Automatic Update (DT: Olivine-3-1; HV: 2.2; Time: 1/3/2020 10:15:38 AM)"=13808, "Automatic Update (DT: Olivine-3-1; HV: 2.2; Time: 1/3/2020 10:15:39 AM)"=13809, "Automatic Update (DT: Olivine-3-1; HV: 2.2; Time: 1/3/2020 10:15:40 AM)"=13810, "Automatic Update (DT: Olivine-3-1; HV: 2.2; Time: 1/3/2020 10:15:41 AM)"=13811, "Automatic Update (DT: Olivine-3-1; HV: 2.2; Time: 1/3/2020 10:15:42 AM)"=13812, "Automatic Update (DT: Olivine-3-1; HV: 2.2; Time: 1/3/2020 10:15:43 AM)"=13813, "Automatic Update (DT: Olivine-3-1; HV: 2.2; Time: 1/3/2020 10:15:44 AM)"=13814, "Automatic Update (DT: Olivine-3-1; HV: 2.2; Time: 1/3/2020 10:15:45 AM)"=13815, "Automatic Update (DT: Olivine-3-1; HV: 2.2; Time: 1/3/2020 10:15:46 AM)"=13816, "Automatic Update (DT: Olivine-3-1; HV: 2.2; Time: 1/3/2020 10:15:47 AM)"=13817, "Automatic Update (DT: Olivine-3-1; HV: 2.2; Time: 1/3/2020 10:15:48 AM)"=13818, "Automatic Update (DT: Olivine-3-1; HV: 2.2; Time: 1/3/2020 10:15:49 AM)"=13819, "Automatic Update (DT: Olivine-3-1; HV: 2.2; Time: 1/3/2020 10:15:50 AM)"=13820, "Automatic Update (DT: Olivine-3-1; HV: 2.2; Time: 1/3/2020 10:15:52 AM)"=13821, "Automatic Update (DT: Olivine-3-1; HV: 2.2; Time: 1/3/2020 10:15:53 AM)"=13822, "Automatic Update (DT: Olivine-3-1; HV: 2.2; Time: 1/3/2020 10:15:54 AM)"=13823, "Automatic Update (DT: Olivine-3-1; HV: 2.2; Time: 1/3/2020 10:15:55 AM)"=13824, "Automatic Update (DT: Olivine-3-1; HV: 2.2; Time: 1/3/2020 10:15:57 AM)"=13825, "Automatic Update (DT: Olivine-3-1; HV: 2.2; Time: 1/3/2020 10:15:58 AM)"=13826, "Automatic Update (DT: Olivine-3-1; HV: 2.2; Time: 1/3/2020 10:16:05 AM)"=13827, "Automatic Update (DT: Olivine-3-1; HV: 2.2; Time: 1/3/2020 10:16:06 AM)"=13828, "Automatic Update (DT: Olivine-3-1; HV: 2.2; Time: 1/3/2020 10:16:07 AM)"=13829, "Automatic Update (DT: Olivine-3-1; HV: 2.2; Time: 1/3/2020 10:16:08 AM)"=13830, "Automatic Update (DT: Olivine-3-1; HV: 2.2; Time: 1/3/2020 10:16:09 AM)"=13831, "Automatic Update (DT: Olivine-3-1; HV: 2.2; Time: 1/3/2020 10:16:10 AM)"=13832, "Automatic Update (DT: Olivine-3-1; HV: 2.2; Time: 1/3/2020 10:16:11 AM)"=13833, "Automatic Update (DT: Olivine-3-1; HV: 2.2; Time: 1/3/2020 10:16:12 AM)"=13834, "Automatic Update (DT: Olivine-3-1; HV: 2.2; Time: 1/3/2020 10:16:13 AM)"=13835, "Automatic Update (DT: Olivine-3-1; HV: 2.2; Time: 1/3/2020 10:16:14 AM)"=13836, "Automatic Update (DT: Olivine-3-1; HV: 2.2; Time: 1/3/2020 10:16:15 AM)"=13837, "Automatic Update (DT: Olivine-3-1; HV: 2.2; Time: 1/3/2020 10:16:16 AM)"=13838, "Automatic Update (DT: Olivine-3-1; HV: 2.2; Time: 1/3/2020 10:16:17 AM)"=13839, "Automatic Update (DT: Olivine-3-1; HV: 2.2; Time: 1/3/2020 10:16:21 AM)"=13840, "Automatic Update (DT: Olivine-3-1; HV: 2.2; Time: 1/3/2020 10:16:22 AM)"=13841, "Automatic Update (DT: Olivine-3-1; HV: 2.2; Time: 1/3/2020 10:16:23 AM)"=13842, "Automatic Update (DT: Olivine-3-1; HV: 2.2; Time: 1/3/2020 10:16:24 AM)"=13843, "Automatic Update (DT: Olivine-3-1; HV: 2.2; Time: 1/3/2020 10:16:27 AM)"=13844, "Automatic Update (DT: Olivine-3-1; HV: 2.2; Time: 1/3/2020 10:16:28 AM)"=13845, "Automatic Update (DT: Olivine-3-1; HV: 2.2; Time: 1/3/2020 10:16:30 AM)"=13846, "Automatic Update (DT: Olivine-3-1; HV: 2.2; Time: 1/3/2020 10:16:55 AM)"=13847, "Automatic Update (DT: Olivine-3-1; HV: 2.2; Time: 1/3/2020 10:16:56 AM)"=13848, "Automatic Update (DT: Olivine-3-1; HV: 2.2; Time: 1/3/2020 10:16:57 AM)"=13849, "Automatic Update (DT: Olivine-3-1; HV: 2.2; Time: 1/3/2020 10:17:04 AM)"=13850, "Automatic Update (DT: Olivine-3-1; HV: 2.2; Time: 1/3/2020 10:17:05 AM)"=13851, "Automatic Update (DT: Olivine-3-1; HV: 2.2; Time: 1/3/2020 10:17:06 AM)"=13852, "Automatic Update (DT: Olivine-3-1; HV: 2.2; Time: 1/3/2020 10:17:08 AM)"=13853, "Automatic Update (DT: Olivine-3-1; HV: 2.2; Time: 1/3/2020 10:17:09 AM)"=13854, "Automatic Update (DT: Olivine-3-1; HV: 2.2; Time: 1/3/2020 10:17:34 AM)"=13855, "Automatic Update (DT: Olivine-3-1; HV: 2.2; Time: 1/3/2020 10:17:35 AM)"=13856, "Automatic Update (DT: Olivine-3-1; HV: 2.2; Time: 1/3/2020 10:17:36 AM)"=13857, "Automatic Update (DT: Olivine-3-1; HV: 2.2; Time: 1/3/2020 10:17:47 AM)"=13858, "Automatic Update (DT: Olivine-3-1; HV: 2.2; Time: 1/3/2020 10:17:48 AM)"=13859, "Automatic Update (DT: Olivine-3-1; HV: 2.2; Time: 1/3/2020 10:17:49 AM)"=13860, "Automatic Update (DT: Olivine-3-1; HV: 2.2; Time: 1/3/2020 10:17:50 AM)"=13861, "Automatic Update (DT: Olivine-3-1; HV: 2.2; Time: 1/3/2020 10:17:51 AM)"=13862, "Automatic Update (DT: Olivine-3-1; HV: 2.2; Time: 1/3/2020 10:17:52 AM)"=13863, "Automatic Update (DT: Olivine-3-1; HV: 2.2; Time: 1/3/2020 10:17:53 AM)"=13864, "Automatic Update (DT: Olivine-3-1; HV: 2.2; Time: 1/3/2020 10:17:55 AM)"=13865, "Automatic Update (DT: Olivine-3-1; HV: 2.2; Time: 1/3/2020 10:18:06 AM)"=13866, "Automatic Update (DT: Olivine-3-1; HV: 2.2; Time: 1/3/2020 10:18:33 AM)"=13867, "Automatic Update (DT: Olivine-3-1; HV: 2.2; Time: 1/3/2020 10:18:34 AM)"=13868, "Automatic Update (DT: Olivine-3-1; HV: 2.2; Time: 1/3/2020 10:18:35 AM)"=13869, "Automatic Update (DT: Olivine-3-1; HV: 2.2; Time: 1/3/2020 10:18:36 AM)"=13870, "Automatic Update (DT: Olivine-3-1; HV: 2.2; Time: 1/3/2020 10:18:37 AM)"=13871, "Automatic Update (DT: Olivine-3-1; HV: 2.2; Time: 1/3/2020 10:18:38 AM)"=13872, "Automatic Update (DT: Olivine-3-1; HV: 2.2; Time: 1/3/2020 10:18:39 AM)"=13873, "Automatic Update (DT: Olivine-3-1; HV: 2.2; Time: 1/3/2020 10:18:40 AM)"=13874, "Automatic Update (DT: Olivine-3-1; HV: 2.2; Time: 1/3/2020 10:18:41 AM)"=13875, "Automatic Update (DT: Olivine-3-1; HV: 2.2; Time: 1/3/2020 10:19:30 AM)"=13876, "Automatic Update (DT: Olivine-3-1; HV: 2.2; Time: 1/3/2020 10:19:32 AM)"=13877, "Automatic Update (DT: Olivine-3-1; HV: 2.2; Time: 1/3/2020 10:19:33 AM)"=13878, "Automatic Update (DT: Olivine-3-1; HV: 2.2; Time: 1/3/2020 10:19:35 AM)"=13879, "Automatic Update (DT: Olivine-3-1; HV: 2.2; Time: 1/3/2020 10:19:36 AM)"=13880, "Automatic Update (DT: Olivine-3-1; HV: 2.2; Time: 1/3/2020 10:19:43 AM)"=13881, "Automatic Update (DT: Olivine-3-1; HV: 2.2; Time: 1/3/2020 10:19:44 AM)"=13882, "Automatic Update (DT: Olivine-3-1; HV: 2.2; Time: 1/3/2020 10:19:45 AM)"=13883, "Automatic Update (DT: Olivine-3-1; HV: 2.2; Time: 1/3/2020 10:19:46 AM)"=13884, "Automatic Update (DT: Olivine-3-1; HV: 2.2; Time: 1/3/2020 10:19:47 AM)"=13885, "Automatic Update (DT: Olivine-3-1; HV: 2.2; Time: 1/3/2020 10:19:48 AM)"=13886, "Automatic Update (DT: Olivine-3-1; HV: 2.2; Time: 1/3/2020 10:19:50 AM)"=13887, "Automatic Update (DT: Olivine-3-1; HV: 2.2; Time: 1/3/2020 10:19:51 AM)"=13888, "Automatic Update (DT: Olivine-3-1; HV: 2.2; Time: 1/3/2020 10:19:52 AM)"=13889, "Automatic Update (DT: Olivine-3-1; HV: 2.2; Time: 1/3/2020 10:19:54 AM)"=13890, "Automatic Update (DT: Olivine-3-1; HV: 2.2; Time: 1/3/2020 10:19:55 AM)"=13891, "Automatic Update (DT: Olivine-3-1; HV: 2.2; Time: 1/3/2020 10:19:56 AM)"=13892, "Automatic Update (DT: Olivine-3-1; HV: 2.2; Time: 1/3/2020 10:19:57 AM)"=13893, "Automatic Update (DT: Olivine-3-1; HV: 2.2; Time: 1/3/2020 10:19:58 AM)"=13894, "Automatic Update (DT: Olivine-3-1; HV: 2.2; Time: 1/3/2020 10:20:00 AM)"=13895, "Automatic Update (DT: Olivine-3-1; HV: 2.2; Time: 1/3/2020 10:20:18 AM)"=13896, "Automatic Update (DT: Olivine-3-1; HV: 2.2; Time: 1/3/2020 10:20:19 AM)"=13897, "Automatic Update (DT: Olivine-3-1; HV: 2.2; Time: 1/3/2020 10:20:31 AM)"=13898, "Automatic Update (DT: Olivine-3-1; HV: 2.2; Time: 1/3/2020 10:20:32 AM)"=13899, "Automatic Update (DT: Olivine-3-1; HV: 2.2; Time: 1/3/2020 10:20:33 AM)"=13900, "Automatic Update (DT: Olivine-3-1; HV: 2.2; Time: 1/3/2020 10:20:34 AM)"=13901, "Automatic Update (DT: Olivine-3-1; HV: 2.2; Time: 1/3/2020 10:20:42 AM)"=13902, "Automatic Update (DT: Olivine-3-1; HV: 2.2; Time: 1/3/2020 10:20:43 AM)"=13903, "Automatic Update (DT: Olivine-3-1; HV: 2.2; Time: 1/3/2020 10:21:00 AM)"=13904, "Automatic Update (DT: Olivine-3-1; HV: 2.2; Time: 1/3/2020 10:21:04 AM)"=13905, "Automatic Update (DT: Olivine-3-1; HV: 2.2; Time: 1/3/2020 10:21:05 AM)"=13906, "Automatic Update (DT: Olivine-3-1; HV: 2.2; Time: 1/3/2020 10:21:07 AM)"=13907, "Automatic Update (DT: Olivine-3-1; HV: 2.2; Time: 1/3/2020 10:21:31 AM)"=13908, "Automatic Update (DT: Olivine-3-1; HV: 2.2; Time: 1/3/2020 10:21:32 AM)"=13909, "Automatic Update (DT: Olivine-3-1; HV: 2.2; Time: 1/3/2020 10:21:33 AM)"=13910, "Automatic Update (DT: Olivine-3-1; HV: 2.2; Time: 1/3/2020 10:21:34 AM)"=13911, "Automatic Update (DT: Olivine-3-1; HV: 2.2; Time: 1/3/2020 10:21:35 AM)"=13912, "Automatic Update (DT: Olivine-3-1; HV: 2.2; Time: 1/3/2020 10:21:36 AM)"=13913, "Automatic Update (DT: Olivine-3-1; HV: 2.2; Time: 1/3/2020 10:21:38 AM)"=13914, "Automatic Update (DT: Olivine-3-1; HV: 2.2; Time: 1/3/2020 10:21:40 AM)"=13915, "Automatic Update (DT: Olivine-3-1; HV: 2.2; Time: 1/3/2020 10:21:41 AM)"=13916, "Automatic Update (DT: Olivine-3-1; HV: 2.2; Time: 1/3/2020 10:21:51 AM)"=13917, "Automatic Update (DT: Olivine-3-1; HV: 2.2; Time: 1/3/2020 10:21:52 AM)"=13918, "Automatic Update (DT: Olivine-3-1; HV: 2.2; Time: 1/3/2020 10:21:53 AM)"=13919, "Automatic Update (DT: Olivine-3-1; HV: 2.2; Time: 1/3/2020 10:21:59 AM)"=13920, "Automatic Update (DT: Olivine-3-1; HV: 2.2; Time: 1/3/2020 10:22:00 AM)"=13921, "Automatic Update (DT: Olivine-3-1; HV: 2.2; Time: 1/3/2020 10:22:01 AM)"=13922, "Automatic Update (DT: Olivine-3-1; HV: 2.2; Time: 1/3/2020 10:22:02 AM)"=13923, "Automatic Update (DT: Olivine-3-1; HV: 2.2; Time: 1/3/2020 10:22:03 AM)"=13924, "Automatic Update (DT: Olivine-3-1; HV: 2.2; Time: 1/3/2020 10:22:04 AM)"=13925, "Automatic Update (DT: Olivine-3-1; HV: 2.2; Time: 1/3/2020 10:22:07 AM)"=13926, "Automatic Update (DT: Olivine-3-1; HV: 2.2; Time: 1/3/2020 10:22:08 AM)"=13927, "Automatic Update (DT: Olivine-3-1; HV: 2.2; Time: 1/3/2020 10:22:09 AM)"=13928, "Automatic Update (DT: Olivine-3-1; HV: 2.2; Time: 1/3/2020 10:22:10 AM)"=13929, "Automatic Update (DT: Olivine-3-1; HV: 2.2; Time: 1/3/2020 10:22:11 AM)"=13930, "Automatic Update (DT: Olivine-3-1; HV: 2.2; Time: 1/3/2020 10:22:12 AM)"=13931, "Automatic Update (DT: Olivine-3-1; HV: 2.2; Time: 1/3/2020 10:22:13 AM)"=13932, "Automatic Update (DT: Olivine-3-1; HV: 2.2; Time: 1/3/2020 10:22:14 AM)"=13933, "Automatic Update (DT: Olivine-3-1; HV: 2.2; Time: 1/3/2020 10:22:15 AM)"=13934, "Automatic Update (DT: Olivine-3-1; HV: 2.2; Time: 1/3/2020 10:22:16 AM)"=13935, "Automatic Update (DT: Olivine-3-1; HV: 2.2; Time: 1/3/2020 10:22:17 AM)"=13936, "Automatic Update (DT: Olivine-3-1; HV: 2.2; Time: 1/3/2020 10:22:18 AM)"=13937, "Automatic Update (DT: Olivine-3-1; HV: 2.2; Time: 1/3/2020 10:22:19 AM)"=13938, "Automatic Update (DT: Olivine-3-1; HV: 2.2; Time: 1/3/2020 10:22:25 AM)"=13939, "Automatic Update (DT: Olivine-3-1; HV: 2.2; Time: 1/3/2020 10:22:26 AM)"=13940, "Automatic Update (DT: Olivine-3-1; HV: 2.2; Time: 1/3/2020 10:22:29 AM)"=13941, "Automatic Update (DT: Olivine-3-1; HV: 2.2; Time: 1/3/2020 10:22:30 AM)"=13942, "Automatic Update (DT: Olivine-3-1; HV: 2.2; Time: 1/3/2020 10:22:32 AM)"=13943, "Automatic Update (DT: Olivine-3-1; HV: 2.2; Time: 1/3/2020 10:22:34 AM)"=13944, "Automatic Update (DT: Olivine-3-1; HV: 2.2; Time: 1/3/2020 10:22:48 AM)"=13945, "Automatic Update (DT: Olivine-3-1; HV: 2.2; Time: 1/3/2020 10:22:49 AM)"=13946, "Automatic Update (DT: Olivine-3-1; HV: 2.2; Time: 1/3/2020 10:22:55 AM)"=13947, "Automatic Update (DT: Olivine-3-1; HV: 2.2; Time: 1/3/2020 10:23:00 AM)"=13948, "Automatic Update (DT: Olivine-3-1; HV: 2.2; Time: 1/3/2020 10:23:01 AM)"=13949, "Automatic Update (DT: Olivine-3-1; HV: 2.2; Time: 1/3/2020 10:23:02 AM)"=13950, "Automatic Update (DT: Olivine-3-1; HV: 2.2; Time: 1/3/2020 10:23:03 AM)"=13951, "Automatic Update (DT: Olivine-3-1; HV: 2.2; Time: 1/3/2020 10:23:04 AM)"=13952, "Automatic Update (DT: Olivine-3-1; HV: 2.2; Time: 1/3/2020 10:23:05 AM)"=13953, "Automatic Update (DT: Olivine-3-1; HV: 2.2; Time: 1/3/2020 10:23:06 AM)"=13954, "Automatic Update (DT: Olivine-3-1; HV: 2.2; Time: 1/3/2020 10:23:07 AM)"=13955, "Automatic Update (DT: Olivine-3-1; HV: 2.2; Time: 1/3/2020 10:23:08 AM)"=13956, "Automatic Update (DT: Olivine-3-1; HV: 2.2; Time: 1/3/2020 10:23:10 AM)"=13957, "Automatic Update (DT: Olivine-3-1; HV: 2.2; Time: 1/3/2020 10:23:11 AM)"=13958, "Automatic Update (DT: Olivine-3-1; HV: 2.2; Time: 1/3/2020 10:23:12 AM)"=13959, "Automatic Update (DT: Olivine-3-1; HV: 2.2; Time: 1/3/2020 10:23:27 AM)"=13960, "Automatic Update (DT: Olivine-3-1; HV: 2.2; Time: 1/3/2020 10:23:28 AM)"=13961, "Automatic Update (DT: Olivine-3-1; HV: 2.2; Time: 1/3/2020 10:23:29 AM)"=13962, "Automatic Update (DT: Olivine-3-1; HV: 2.2; Time: 1/3/2020 10:23:30 AM)"=13963, "Automatic Update (DT: Olivine-3-1; HV: 2.2; Time: 1/3/2020 10:23:32 AM)"=13964, "Automatic Update (DT: Olivine-3-1; HV: 2.2; Time: 1/3/2020 10:23:33 AM)"=13965, "Automatic Update (DT: Olivine-3-1; HV: 2.2; Time: 1/3/2020 10:23:34 AM)"=13966, "Automatic Update (DT: Olivine-3-1; HV: 2.2; Time: 1/3/2020 10:23:35 AM)"=13967, "Automatic Update (DT: Olivine-3-1; HV: 2.2; Time: 1/3/2020 10:23:36 AM)"=13968, "Automatic Update (DT: Olivine-3-1; HV: 2.2; Time: 1/3/2020 10:23:39 AM)"=13969, "Automatic Update (DT: Olivine-3-1; HV: 2.2; Time: 1/3/2020 10:23:40 AM)"=13970, "Automatic Update (DT: Olivine-3-1; HV: 2.2; Time: 1/3/2020 10:23:41 AM)"=13971, "Automatic Update (DT: Olivine-3-1; HV: 2.2; Time: 1/3/2020 10:23:42 AM)"=13972, "Automatic Update (DT: Olivine-3-1; HV: 2.2; Time: 1/3/2020 10:23:43 AM)"=13973, "Automatic Update (DT: Olivine-3-1; HV: 2.2; Time: 1/3/2020 10:24:24 AM)"=13974, "Automatic Update (DT: Olivine-3-1; HV: 0.8; Time: 1/7/2020 10:53:34 AM)"=13975, "Automatic Update (DT: Olivine-3-1; HV: 0.8; Time: 1/7/2020 10:53:36 AM)"=13976, "Automatic Update (DT: Olivine-3-1; HV: 0.8; Time: 1/7/2020 11:24:52 AM)"=13977, "Automatic Update (DT: Olivine-3-1; HV: 0.8; Time: 1/7/2020 11:24:56 AM)"=13978, "Automatic Update (DT: Olivine-3-1; HV: 0.8; Time: 1/7/2020 11:25:00 AM)"=13979, "Automatic Update (DT: Olivine-3-1; HV: 0.8; Time: 1/7/2020 11:25:17 AM)"=13980, "Automatic Update (DT: Olivine-3-1; HV: 0.8; Time: 1/7/2020 11:25:23 AM)"=13981, "Automatic Update (DT: Olivine-3-1; HV: 0.8; Time: 1/7/2020 11:25:34 AM)"=13982, "Automatic Update (DT: Olivine-3-1; HV: 0.8; Time: 1/7/2020 11:25:35 AM)"=13983, "Automatic Update (DT: Olivine-3-1; HV: 0.8; Time: 1/7/2020 11:25:36 AM)"=13984, "Automatic Update (DT: Olivine-3-1; HV: 0.8; Time: 1/7/2020 11:25:37 AM)"=13985, "Automatic Update (DT: Olivine-3-1; HV: 0.8; Time: 1/7/2020 11:25:38 AM)"=13986, "Automatic Update (DT: Olivine-3-1; HV: 0.8; Time: 1/7/2020 11:25:39 AM)"=13987, "Automatic Update (DT: Olivine-3-1; HV: 0.8; Time: 1/7/2020 11:25:41 AM)"=13988, "Automatic Update (DT: Olivine-3-1; HV: 0.8; Time: 1/7/2020 11:26:00 AM)"=13989, "Automatic Update (DT: Olivine-3-1; HV: 2.2; Time: 1/9/2020 1:24:14 PM)"=13990, "Automatic Update (DT: Olivine-3-1; HV: 2.2; Time: 1/9/2020 1:24:20 PM)"=13991, "Automatic Update (DT: Olivine-3-1; HV: 2.2; Time: 1/9/2020 1:24:26 PM)"=13992, "Automatic Update (DT: Olivine-3-1; HV: 2.2; Time: 1/9/2020 1:24:30 PM)"=13993, "Automatic Update (DT: Olivine-3-1; HV: 2.2; Time: 1/9/2020 1:24:33 PM)"=13994, "Automatic Update (DT: Olivine-3-1; HV: 2.2; Time: 1/9/2020 1:24:37 PM)"=13995, "Automatic Update (DT: Olivine-3-1; HV: 2.2; Time: 1/9/2020 1:24:41 PM)"=13996, "Automatic Update (DT: Olivine-3-1; HV: 2.2; Time: 1/9/2020 1:24:45 PM)"=13997, "Automatic Update (DT: Olivine-3-1; HV: 2.2; Time: 1/9/2020 1:24:48 PM)"=13998, "Automatic Update (DT: Olivine-3-1; HV: 2.2; Time: 1/9/2020 1:24:50 PM)"=13999, "Automatic Update (DT: Olivine-3-1; HV: 2.2; Time: 1/9/2020 1:24:54 PM)"=14000, "Automatic Update (DT: Olivine-3-1; HV: 2.2; Time: 1/9/2020 1:24:57 PM)"=14001, "Automatic Update (DT: Olivine-3-1; HV: 2.2; Time: 1/9/2020 1:24:59 PM)"=14002, "Automatic Update (DT: Olivine-3-1; HV: 2.2; Time: 1/9/2020 1:25:00 PM)"=14003, "Automatic Update (DT: Olivine-3-1; HV: 2.2; Time: 1/9/2020 1:25:03 PM)"=14004, "Automatic Update (DT: Olivine-3-1; HV: 2.2; Time: 1/9/2020 1:25:04 PM)"=14005, "Automatic Update (DT: Olivine-3-1; HV: 2.2; Time: 1/9/2020 1:25:05 PM)"=14006, "Automatic Update (DT: Olivine-3-1; HV: 2.2; Time: 1/9/2020 1:25:07 PM)"=14007, "Automatic Update (DT: Olivine-3-1; HV: 2.2; Time: 1/9/2020 1:25:08 PM)"=14008, "Automatic Update (DT: Olivine-3-1; HV: 2.2; Time: 1/9/2020 1:25:10 PM)"=14009, "Automatic Update (DT: Olivine-3-1; HV: 2.2; Time: 1/9/2020 1:25:12 PM)"=14010, "Automatic Update (DT: Olivine-3-1; HV: 2.2; Time: 1/9/2020 1:25:13 PM)"=14011, "Automatic Update (DT: Olivine-3-1; HV: 2.2; Time: 1/9/2020 1:25:14 PM)"=14012, "Automatic Update (DT: Olivine-3-1; HV: 2.2; Time: 1/9/2020 1:25:15 PM)"=14013, "Automatic Update (DT: Olivine-3-1; HV: 2.2; Time: 1/9/2020 1:25:16 PM)"=14014, "Automatic Update (DT: Olivine-3-1; HV: 2.2; Time: 1/9/2020 1:25:17 PM)"=14015, "Automatic Update (DT: Olivine-3-1; HV: 2.2; Time: 1/9/2020 1:25:18 PM)"=14016, "Automatic Update (DT: Olivine-3-1; HV: 2.2; Time: 1/9/2020 1:25:20 PM)"=14017, "Automatic Update (DT: Olivine-3-1; HV: 2.2; Time: 1/9/2020 1:25:21 PM)"=14018, "Automatic Update (DT: Olivine-3-1; HV: 2.2; Time: 1/9/2020 1:25:22 PM)"=14019, "Automatic Update (DT: Olivine-3-1; HV: 2.2; Time: 1/9/2020 1:25:23 PM)"=14020, "Automatic Update (DT: Olivine-3-1; HV: 2.2; Time: 1/9/2020 1:25:24 PM)"=14021, "Automatic Update (DT: Olivine-3-1; HV: 2.2; Time: 1/9/2020 1:25:25 PM)"=14022, "Automatic Update (DT: Olivine-3-1; HV: 2.2; Time: 1/9/2020 1:25:26 PM)"=14023, "Automatic Update (DT: Olivine-3-1; HV: 2.2; Time: 1/9/2020 1:25:27 PM)"=14024, "Automatic Update (DT: Olivine-3-1; HV: 2.2; Time: 1/9/2020 1:25:28 PM)"=14025, "Automatic Update (DT: Olivine-3-1; HV: 2.2; Time: 1/9/2020 1:25:29 PM)"=14026, "Automatic Update (DT: Olivine-3-1; HV: 2.2; Time: 1/9/2020 1:25:30 PM)"=14027, "Automatic Update (DT: Olivine-3-1; HV: 2.2; Time: 1/9/2020 1:25:31 PM)"=14028, "Automatic Update (DT: Olivine-3-1; HV: 2.2; Time: 1/9/2020 1:25:32 PM)"=14029, "Automatic Update (DT: Olivine-3-1; HV: 2.2; Time: 1/9/2020 1:25:34 PM)"=14030, "Automatic Update (DT: Olivine-3-1; HV: 2.2; Time: 1/9/2020 1:25:35 PM)"=14031, "Automatic Update (DT: Olivine-3-1; HV: 2.2; Time: 1/9/2020 1:25:36 PM)"=14032, "Automatic Update (DT: Olivine-3-1; HV: 2.2; Time: 1/9/2020 1:25:37 PM)"=14033, "Automatic Update (DT: Olivine-3-1; HV: 2.2; Time: 1/9/2020 1:25:38 PM)"=14034, "Automatic Update (DT: Olivine-3-1; HV: 2.2; Time: 1/9/2020 1:25:39 PM)"=14035, "Automatic Update (DT: Olivine-3-1; HV: 2.2; Time: 1/9/2020 1:25:40 PM)"=14036, "Automatic Update (DT: Olivine-3-1; HV: 2.2; Time: 1/9/2020 1:25:41 PM)"=14037, "Automatic Update (DT: Olivine-3-1; HV: 2.2; Time: 1/9/2020 1:25:42 PM)"=14038, "Automatic Update (DT: Olivine-3-1; HV: 2.2; Time: 1/9/2020 1:25:44 PM)"=14039, "Automatic Update (DT: Olivine-3-1; HV: 2.2; Time: 1/9/2020 1:25:46 PM)"=14040, "Automatic Update (DT: Olivine-3-1; HV: 2.2; Time: 1/9/2020 1:25:47 PM)"=14041, "Automatic Update (DT: Olivine-3-1; HV: 2.2; Time: 1/9/2020 1:25:48 PM)"=14042, "Automatic Update (DT: Olivine-3-1; HV: 2.2; Time: 1/9/2020 1:25:49 PM)"=14043, "Automatic Update (DT: Olivine-3-1; HV: 2.2; Time: 1/9/2020 1:25:51 PM)"=14044, "Automatic Update (DT: Olivine-3-1; HV: 2.2; Time: 1/9/2020 1:25:52 PM)"=14045, "Automatic Update (DT: Olivine-3-1; HV: 2.2; Time: 1/9/2020 1:25:53 PM)"=14046, "Automatic Update (DT: Olivine-3-1; HV: 2.2; Time: 1/9/2020 1:25:54 PM)"=14047, "Automatic Update (DT: Olivine-3-1; HV: 2.2; Time: 1/9/2020 1:25:55 PM)"=14048, "Automatic Update (DT: Olivine-3-1; HV: 2.2; Time: 1/9/2020 1:25:56 PM)"=14049, "Automatic Update (DT: Olivine-3-1; HV: 2.2; Time: 1/9/2020 1:26:00 PM)"=14050, "Automatic Update (DT: Olivine-3-1; HV: 2.2; Time: 1/9/2020 1:26:01 PM)"=14051, "Automatic Update (DT: Olivine-3-1; HV: 2.2; Time: 1/9/2020 1:26:02 PM)"=14052, "Automatic Update (DT: Olivine-3-1; HV: 2.2; Time: 1/9/2020 1:26:03 PM)"=14053, "Automatic Update (DT: Olivine-3-1; HV: 2.2; Time: 1/9/2020 1:26:04 PM)"=14054, "Automatic Update (DT: Olivine-3-1; HV: 2.2; Time: 1/9/2020 1:26:06 PM)"=14055, "Automatic Update (DT: Olivine-3-1; HV: 2.2; Time: 1/9/2020 1:26:08 PM)"=14056, "Automatic Update (DT: Olivine-3-1; HV: 2.2; Time: 1/9/2020 1:26:09 PM)"=14057, "Automatic Update (DT: Olivine-3-1; HV: 2.2; Time: 1/9/2020 1:26:10 PM)"=14058, "Automatic Update (DT: Olivine-3-1; HV: 2.2; Time: 1/9/2020 1:26:11 PM)"=14059, "Automatic Update (DT: Olivine-3-1; HV: 2.2; Time: 1/9/2020 1:26:12 PM)"=14060, "Automatic Update (DT: Olivine-3-1; HV: 2.2; Time: 1/9/2020 1:26:13 PM)"=14061, "Automatic Update (DT: Olivine-3-1; HV: 2.2; Time: 1/9/2020 1:26:14 PM)"=14062, "Automatic Update (DT: Olivine-3-1; HV: 2.2; Time: 1/9/2020 1:26:15 PM)"=14063, "Automatic Update (DT: Olivine-3-1; HV: 2.2; Time: 1/9/2020 1:26:16 PM)"=14064, "Automatic Update (DT: Olivine-3-1; HV: 2.2; Time: 1/9/2020 1:26:17 PM)"=14065, "Automatic Update (DT: Olivine-3-1; HV: 2.2; Time: 1/9/2020 1:26:18 PM)"=14066, "Automatic Update (DT: Olivine-3-1; HV: 2.2; Time: 1/9/2020 1:26:22 PM)"=14067, "Automatic Update (DT: Olivine-3-1; HV: 2.2; Time: 1/9/2020 1:26:23 PM)"=14068, "Automatic Update (DT: Olivine-3-1; HV: 2.2; Time: 1/9/2020 1:26:24 PM)"=14069, "Automatic Update (DT: Olivine-3-1; HV: 2.2; Time: 1/9/2020 1:26:25 PM)"=14070, "Automatic Update (DT: Olivine-3-1; HV: 2.2; Time: 1/9/2020 1:26:26 PM)"=14071, "Automatic Update (DT: Olivine-3-1; HV: 2.2; Time: 1/9/2020 1:26:27 PM)"=14072, "Automatic Update (DT: Olivine-3-1; HV: 2.2; Time: 1/9/2020 1:26:28 PM)"=14073, "Automatic Update (DT: Olivine-3-1; HV: 2.2; Time: 1/9/2020 1:26:29 PM)"=14074, "Automatic Update (DT: Olivine-3-1; HV: 2.2; Time: 1/9/2020 1:26:30 PM)"=14075, "Automatic Update (DT: Olivine-3-1; HV: 2.2; Time: 1/9/2020 1:26:31 PM)"=14076, "Automatic Update (DT: Olivine-3-1; HV: 2.2; Time: 1/9/2020 1:26:32 PM)"=14077, "Automatic Update (DT: Olivine-3-1; HV: 2.2; Time: 1/9/2020 1:26:33 PM)"=14078, "Automatic Update (DT: Olivine-3-1; HV: 2.2; Time: 1/9/2020 1:26:34 PM)"=14079, "Automatic Update (DT: Olivine-3-1; HV: 2.2; Time: 1/9/2020 1:26:36 PM)"=14080, "Automatic Update (DT: Olivine-3-1; HV: 2.2; Time: 1/9/2020 1:26:37 PM)"=14081, "Automatic Update (DT: Olivine-3-1; HV: 2.2; Time: 1/9/2020 1:26:38 PM)"=14082, "Automatic Update (DT: Olivine-3-1; HV: 2.2; Time: 1/9/2020 1:26:39 PM)"=14083, "Automatic Update (DT: Olivine-3-1; HV: 2.2; Time: 1/9/2020 1:26:43 PM)"=14084, "Automatic Update (DT: Olivine-3-1; HV: 2.2; Time: 1/9/2020 1:26:45 PM)"=14085, "Automatic Update (DT: Olivine-3-1; HV: 2.2; Time: 1/9/2020 1:26:46 PM)"=14086, "Automatic Update (DT: Olivine-3-1; HV: 2.2; Time: 1/9/2020 1:26:47 PM)"=14087, "Automatic Update (DT: Olivine-3-1; HV: 2.2; Time: 1/9/2020 1:26:51 PM)"=14088, "Automatic Update (DT: Olivine-3-1; HV: 2.2; Time: 1/9/2020 1:26:52 PM)"=14089, "Automatic Update (DT: Olivine-3-1; HV: 2.2; Time: 1/9/2020 1:26:53 PM)"=14090, "Automatic Update (DT: Olivine-3-1; HV: 2.2; Time: 1/9/2020 1:26:54 PM)"=14091, "Automatic Update (DT: Olivine-3-1; HV: 2.2; Time: 1/9/2020 1:26:55 PM)"=14092, "Automatic Update (DT: Olivine-3-1; HV: 2.2; Time: 1/9/2020 1:26:56 PM)"=14093, "Automatic Update (DT: Olivine-3-1; HV: 2.2; Time: 1/9/2020 1:26:57 PM)"=14094, "Automatic Update (DT: Olivine-3-1; HV: 2.2; Time: 1/9/2020 1:26:58 PM)"=14095, "Automatic Update (DT: Olivine-3-1; HV: 2.2; Time: 1/9/2020 1:26:59 PM)"=14096, "Automatic Update (DT: Olivine-3-1; HV: 2.2; Time: 1/9/2020 1:27:00 PM)"=14097, "Automatic Update (DT: Olivine-3-1; HV: 2.2; Time: 1/9/2020 1:27:01 PM)"=14098, "Automatic Update (DT: Olivine-3-1; HV: 2.2; Time: 1/9/2020 1:27:02 PM)"=14099, "Automatic Update (DT: Olivine-3-1; HV: 2.2; Time: 1/9/2020 1:27:04 PM)"=14100, "Automatic Update (DT: Olivine-3-1; HV: 2.2; Time: 1/9/2020 1:27:05 PM)"=14101, "Automatic Update (DT: Olivine-3-1; HV: 2.2; Time: 1/9/2020 1:27:07 PM)"=14102, "Automatic Update (DT: Olivine-3-1; HV: 2.2; Time: 1/9/2020 1:27:08 PM)"=14103, "Automatic Update (DT: Olivine-3-1; HV: 2.2; Time: 1/9/2020 1:27:09 PM)"=14104, "Automatic Update (DT: Olivine-3-1; HV: 2.2; Time: 1/9/2020 1:27:10 PM)"=14105, "Automatic Update (DT: Olivine-3-1; HV: 2.2; Time: 1/9/2020 1:27:11 PM)"=14106, "Automatic Update (DT: Olivine-3-1; HV: 2.2; Time: 1/9/2020 1:27:12 PM)"=14107, "Automatic Update (DT: Olivine-3-1; HV: 2.2; Time: 1/9/2020 1:27:14 PM)"=14108, "Automatic Update (DT: Olivine-3-1; HV: 2.2; Time: 1/9/2020 1:27:15 PM)"=14109, "Automatic Update (DT: Olivine-3-1; HV: 2.2; Time: 1/9/2020 1:27:16 PM)"=14110, "Automatic Update (DT: Olivine-3-1; HV: 2.2; Time: 1/9/2020 1:27:17 PM)"=14111, "Automatic Update (DT: Olivine-3-1; HV: 2.2; Time: 1/9/2020 1:27:18 PM)"=14112, "Automatic Update (DT: Olivine-3-1; HV: 2.2; Time: 1/9/2020 1:27:19 PM)"=14113, "Automatic Update (DT: Olivine-3-1; HV: 2.2; Time: 1/9/2020 1:27:20 PM)"=14114, "Automatic Update (DT: Olivine-3-1; HV: 2.2; Time: 1/9/2020 1:27:21 PM)"=14115, "Automatic Update (DT: Olivine-3-1; HV: 2.2; Time: 1/9/2020 1:27:22 PM)"=14116, "Automatic Update (DT: Olivine-3-1; HV: 2.2; Time: 1/9/2020 1:27:23 PM)"=14117, "Automatic Update (DT: Olivine-3-1; HV: 2.2; Time: 1/9/2020 1:27:24 PM)"=14118, "Automatic Update (DT: Olivine-3-1; HV: 2.2; Time: 1/9/2020 1:27:29 PM)"=14119, "Automatic Update (DT: Olivine-3-1; HV: 2.2; Time: 1/9/2020 1:27:31 PM)"=14120, "Automatic Update (DT: Olivine-3-1; HV: 2.2; Time: 1/9/2020 1:27:32 PM)"=14121, "Automatic Update (DT: Olivine-3-1; HV: 2.2; Time: 1/9/2020 1:27:33 PM)"=14122, "Automatic Update (DT: Olivine-3-1; HV: 2.2; Time: 1/9/2020 1:27:34 PM)"=14123, "Automatic Update (DT: Olivine-3-1; HV: 2.2; Time: 1/9/2020 1:27:35 PM)"=14124, "Automatic Update (DT: Olivine-3-1; HV: 2.2; Time: 1/9/2020 1:27:36 PM)"=14125, "Automatic Update (DT: Olivine-3-1; HV: 2.2; Time: 1/9/2020 1:27:37 PM)"=14126, "Automatic Update (DT: Olivine-3-1; HV: 2.2; Time: 1/9/2020 1:27:38 PM)"=14127, "Automatic Update (DT: Olivine-3-1; HV: 2.2; Time: 1/9/2020 1:27:39 PM)"=14128, "Automatic Update (DT: Olivine-3-1; HV: 2.2; Time: 1/9/2020 1:27:40 PM)"=14129, "Automatic Update (DT: Olivine-3-1; HV: 2.2; Time: 1/9/2020 1:27:41 PM)"=14130, "Automatic Update (DT: Olivine-3-1; HV: 2.2; Time: 1/9/2020 1:27:44 PM)"=14131, "Automatic Update (DT: Olivine-3-1; HV: 2.2; Time: 1/9/2020 1:27:45 PM)"=14132, "Automatic Update (DT: Olivine-3-1; HV: 2.2; Time: 1/9/2020 1:27:46 PM)"=14133, "Automatic Update (DT: Olivine-3-1; HV: 2.2; Time: 1/9/2020 1:27:47 PM)"=14134, "Automatic Update (DT: Olivine-3-1; HV: 2.2; Time: 1/9/2020 1:27:48 PM)"=14135, "Automatic Update (DT: Olivine-3-1; HV: 2.2; Time: 1/9/2020 1:27:52 PM)"=14136, "Automatic Update (DT: Olivine-3-1; HV: 2.2; Time: 1/9/2020 1:27:53 PM)"=14137, "Automatic Update (DT: Olivine-3-1; HV: 2.2; Time: 1/9/2020 1:27:54 PM)"=14138, "Automatic Update (DT: Olivine-3-1; HV: 2.2; Time: 1/9/2020 1:27:55 PM)"=14139, "Automatic Update (DT: Olivine-3-1; HV: 2.2; Time: 1/9/2020 1:27:57 PM)"=14140, "Automatic Update (DT: Olivine-3-1; HV: 2.2; Time: 1/9/2020 1:27:58 PM)"=14141, "Automatic Update (DT: Olivine-3-1; HV: 2.2; Time: 1/9/2020 1:27:59 PM)"=14142, "Automatic Update (DT: Olivine-3-1; HV: 2.2; Time: 1/9/2020 1:28:01 PM)"=14143, "Automatic Update (DT: Olivine-3-1; HV: 2.2; Time: 1/9/2020 1:28:02 PM)"=14144, "Automatic Update (DT: Olivine-3-1; HV: 2.2; Time: 1/9/2020 1:28:03 PM)"=14145, "Automatic Update (DT: Olivine-3-1; HV: 2.2; Time: 1/9/2020 1:28:04 PM)"=14146, "Automatic Update (DT: Olivine-3-1; HV: 2.2; Time: 1/9/2020 1:28:05 PM)"=14147, "Automatic Update (DT: Olivine-3-1; HV: 2.2; Time: 1/9/2020 1:28:06 PM)"=14148, "Automatic Update (DT: Olivine-3-1; HV: 2.2; Time: 1/9/2020 1:28:07 PM)"=14149, "Automatic Update (DT: Olivine-3-1; HV: 2.2; Time: 1/9/2020 1:28:08 PM)"=14150, "Automatic Update (DT: Olivine-3-1; HV: 2.2; Time: 1/9/2020 1:28:09 PM)"=14151, "Automatic Update (DT: Olivine-3-1; HV: 2.2; Time: 1/9/2020 1:28:10 PM)"=14152, "Automatic Update (DT: Olivine-3-1; HV: 2.2; Time: 1/9/2020 1:28:11 PM)"=14153, "Automatic Update (DT: Olivine-3-1; HV: 2.2; Time: 1/9/2020 1:28:21 PM)"=14154, "Automatic Update (DT: Olivine-3-1; HV: 2.2; Time: 1/9/2020 1:28:22 PM)"=14155, "Automatic Update (DT: Olivine-3-1; HV: 2.2; Time: 1/9/2020 1:28:23 PM)"=14156, "Automatic Update (DT: Olivine-3-1; HV: 2.2; Time: 1/9/2020 1:28:24 PM)"=14157, "Automatic Update (DT: Olivine-3-1; HV: 2.2; Time: 1/9/2020 1:29:16 PM)"=14158, "Automatic Update (DT: Olivine-3-1; HV: 2.2; Time: 1/9/2020 1:29:17 PM)"=14159, "Automatic Update (DT: Olivine-3-1; HV: 2.2; Time: 1/9/2020 1:29:19 PM)"=14160, "Automatic Update (DT: Olivine-3-1; HV: 2.2; Time: 1/9/2020 1:29:20 PM)"=14161, "Automatic Update (DT: Olivine-3-1; HV: 2.2; Time: 1/9/2020 1:29:21 PM)"=14162, "Automatic Update (DT: Olivine-3-1; HV: 2.2; Time: 1/9/2020 1:29:23 PM)"=14163, "Automatic Update (DT: Olivine-3-1; HV: 2.2; Time: 1/9/2020 1:29:26 PM)"=14164, "Automatic Update (DT: Olivine-3-1; HV: 2.2; Time: 1/9/2020 1:29:44 PM)"=14165, "Automatic Update (DT: Olivine-3-1; HV: 2.2; Time: 1/9/2020 1:29:45 PM)"=14166, "Automatic Update (DT: Olivine-3-1; HV: 2.2; Time: 1/9/2020 1:29:46 PM)"=14167, "Automatic Update (DT: Olivine-3-1; HV: 2.2; Time: 1/9/2020 1:29:50 PM)"=14168, "Automatic Update (DT: Olivine-3-1; HV: 2.2; Time: 1/9/2020 1:29:51 PM)"=14169, "Automatic Update (DT: Olivine-3-1; HV: 2.2; Time: 1/9/2020 1:29:52 PM)"=14170, "Automatic Update (DT: Olivine-3-1; HV: 2.2; Time: 1/9/2020 1:29:57 PM)"=14171, "Automatic Update (DT: Olivine-3-1; HV: 2.2; Time: 1/9/2020 1:29:58 PM)"=14172, "Automatic Update (DT: Olivine-3-1; HV: 2.2; Time: 1/9/2020 1:29:59 PM)"=14173, "Automatic Update (DT: Olivine-3-1; HV: 2.2; Time: 1/9/2020 1:30:00 PM)"=14174, "Automatic Update (DT: Olivine-3-1; HV: 2.2; Time: 1/9/2020 1:30:02 PM)"=14175, "Automatic Update (DT: Olivine-3-1; HV: 2.2; Time: 1/9/2020 1:30:03 PM)"=14176, "Automatic Update (DT: Olivine-3-1; HV: 2.2; Time: 1/9/2020 1:30:09 PM)"=14177, "Automatic Update (DT: Olivine-3-1; HV: 2.2; Time: 1/9/2020 1:30:10 PM)"=14178, "Automatic Update (DT: Olivine-3-1; HV: 2.2; Time: 1/9/2020 1:30:11 PM)"=14179, "Automatic Update (DT: Olivine-3-1; HV: 2.2; Time: 1/9/2020 1:30:12 PM)"=14180, "Automatic Update (DT: Olivine-3-1; HV: 2.2; Time: 1/9/2020 1:30:13 PM)"=14181, "Automatic Update (DT: Olivine-3-1; HV: 2.2; Time: 1/9/2020 1:30:14 PM)"=14182, "Automatic Update (DT: Olivine-3-1; HV: 2.2; Time: 1/9/2020 1:30:15 PM)"=14183, "Automatic Update (DT: Olivine-3-1; HV: 2.2; Time: 1/9/2020 1:30:16 PM)"=14184, "Automatic Update (DT: Olivine-3-1; HV: 2.2; Time: 1/9/2020 1:30:18 PM)"=14185, "Automatic Update (DT: Olivine-3-1; HV: 2.2; Time: 1/9/2020 1:30:19 PM)"=14186, "Automatic Update (DT: Olivine-3-1; HV: 2.2; Time: 1/9/2020 1:30:20 PM)"=14187, "Automatic Update (DT: Olivine-3-1; HV: 2.2; Time: 1/9/2020 1:30:21 PM)"=14188, "Automatic Update (DT: Olivine-3-1; HV: 2.2; Time: 1/9/2020 1:30:22 PM)"=14189, "Automatic Update (DT: Olivine-3-1; HV: 2.2; Time: 1/9/2020 1:30:25 PM)"=14190, "Automatic Update (DT: Olivine-3-1; HV: 2.2; Time: 1/9/2020 1:30:26 PM)"=14191, "Automatic Update (DT: Olivine-3-1; HV: 2.2; Time: 1/9/2020 1:30:27 PM)"=14192, "Automatic Update (DT: Olivine-3-1; HV: 2.2; Time: 1/9/2020 1:30:28 PM)"=14193, "Automatic Update (DT: Olivine-3-1; HV: 2.2; Time: 1/9/2020 1:30:29 PM)"=14194, "Automatic Update (DT: Olivine-3-1; HV: 2.2; Time: 1/9/2020 1:30:30 PM)"=14195, "Automatic Update (DT: Olivine-3-1; HV: 2.2; Time: 1/9/2020 1:30:31 PM)"=14196, "Automatic Update (DT: Olivine-3-1; HV: 2.2; Time: 1/9/2020 1:30:32 PM)"=14197, "Automatic Update (DT: Olivine-3-1; HV: 2.2; Time: 1/9/2020 1:30:33 PM)"=14198, "Automatic Update (DT: Olivine-3-1; HV: 2.2; Time: 1/9/2020 1:30:34 PM)"=14199, "Automatic Update (DT: Olivine-3-1; HV: 2.2; Time: 1/9/2020 1:30:35 PM)"=14200, "Automatic Update (DT: Olivine-3-1; HV: 2.2; Time: 1/9/2020 1:30:37 PM)"=14201, "Automatic Update (DT: Olivine-3-1; HV: 2.2; Time: 1/9/2020 1:30:44 PM)"=14202, "Automatic Update (DT: Olivine-3-1; HV: 2.2; Time: 1/9/2020 1:30:45 PM)"=14203, "Automatic Update (DT: Olivine-3-1; HV: 2.2; Time: 1/9/2020 1:30:46 PM)"=14204, "Automatic Update (DT: Olivine-3-1; HV: 2.2; Time: 1/9/2020 1:30:48 PM)"=14205, "Automatic Update (DT: Olivine-3-1; HV: 2.2; Time: 1/9/2020 1:30:49 PM)"=14206, "Automatic Update (DT: Olivine-3-1; HV: 2.2; Time: 1/9/2020 1:30:50 PM)"=14207, "Automatic Update (DT: Olivine-3-1; HV: 2.2; Time: 1/9/2020 1:30:55 PM)"=14208, "Automatic Update (DT: Olivine-3-1; HV: 2.2; Time: 1/9/2020 1:30:56 PM)"=14209, "Automatic Update (DT: Olivine-3-1; HV: 2.2; Time: 1/9/2020 1:30:57 PM)"=14210, "Automatic Update (DT: Olivine-3-1; HV: 2.2; Time: 1/9/2020 1:30:58 PM)"=14211, "Automatic Update (DT: Olivine-3-1; HV: 2.2; Time: 1/9/2020 1:30:59 PM)"=14212, "Automatic Update (DT: Olivine-3-1; HV: 2.2; Time: 1/9/2020 1:31:00 PM)"=14213, "Automatic Update (DT: Olivine-3-1; HV: 2.2; Time: 1/9/2020 1:31:01 PM)"=14214, "Automatic Update (DT: Olivine-3-1; HV: 2.2; Time: 1/9/2020 1:31:02 PM)"=14215, "Automatic Update (DT: Olivine-3-1; HV: 2.2; Time: 1/9/2020 1:31:03 PM)"=14216, "Automatic Update (DT: Olivine-3-1; HV: 2.2; Time: 1/9/2020 1:31:04 PM)"=14217, "Automatic Update (DT: Olivine-3-1; HV: 2.2; Time: 1/9/2020 1:31:05 PM)"=14218, "Automatic Update (DT: Olivine-3-1; HV: 2.2; Time: 1/9/2020 1:31:14 PM)"=14219, "Automatic Update (DT: Olivine-3-1; HV: 2.2; Time: 1/9/2020 1:31:25 PM)"=14220, "Automatic Update (DT: Olivine-3-1; HV: 2.2; Time: 1/9/2020 1:31:29 PM)"=14221, "Automatic Update (DT: Olivine-3-1; HV: 2.2; Time: 1/9/2020 1:31:38 PM)"=14222, "Automatic Update (DT: Olivine-3-1; HV: 2.2; Time: 1/9/2020 1:31:45 PM)"=14223, "Automatic Update (DT: Olivine-3-1; HV: 2.2; Time: 1/9/2020 1:31:46 PM)"=14224, "Automatic Update (DT: Olivine-3-1; HV: 2.2; Time: 1/9/2020 1:31:47 PM)"=14225, "Automatic Update (DT: Olivine-3-1; HV: 2.2; Time: 1/9/2020 1:31:49 PM)"=14226, "Automatic Update (DT: Olivine-3-1; HV: 2.2; Time: 1/9/2020 1:31:50 PM)"=14227, "Automatic Update (DT: Olivine-3-1; HV: 2.2; Time: 1/9/2020 1:31:51 PM)"=14228, "Automatic Update (DT: Olivine-3-1; HV: 2.2; Time: 1/9/2020 1:31:52 PM)"=14229, "Automatic Update (DT: Olivine-3-1; HV: 2.2; Time: 1/9/2020 1:32:07 PM)"=14230, "Automatic Update (DT: Olivine-3-1; HV: 2.2; Time: 1/9/2020 3:00:21 PM)"=14231, "Automatic Update (DT: Olivine-3-1; HV: 2.2; Time: 1/9/2020 3:00:22 PM)"=14232, "Automatic Update (DT: Olivine-3-1; HV: 2.2; Time: 1/9/2020 3:00:23 PM)"=14233, "Automatic Update (DT: Olivine-3-1; HV: 2.2; Time: 1/9/2020 3:00:24 PM)"=14234, "Automatic Update (DT: Olivine-3-1; HV: 2.2; Time: 1/9/2020 3:00:25 PM)"=14235, "Automatic Update (DT: Olivine-3-1; HV: 2.2; Time: 1/9/2020 3:00:26 PM)"=14236, "Automatic Update (DT: Olivine-3-1; HV: 2.2; Time: 1/9/2020 3:00:28 PM)"=14237, "Automatic Update (DT: Olivine-3-1; HV: 2.2; Time: 1/9/2020 3:00:29 PM)"=14238, "Automatic Update (DT: Olivine-3-1; HV: 2.2; Time: 1/9/2020 3:00:30 PM)"=14239, "Automatic Update (DT: Olivine-3-1; HV: 2.2; Time: 1/9/2020 3:00:31 PM)"=14240, "Automatic Update (DT: Olivine-3-1; HV: 2.2; Time: 1/9/2020 3:00:32 PM)"=14241, "Automatic Update (DT: Olivine-3-1; HV: 2.2; Time: 1/9/2020 3:00:33 PM)"=14242, "Automatic Update (DT: Olivine-3-1; HV: 2.2; Time: 1/9/2020 3:00:34 PM)"=14243, "Automatic Update (DT: Olivine-3-1; HV: 2.2; Time: 1/9/2020 3:00:35 PM)"=14244, "Automatic Update (DT: Olivine-3-1; HV: 2.2; Time: 1/9/2020 3:00:36 PM)"=14245, "Automatic Update (DT: Olivine-3-1; HV: 2.2; Time: 1/9/2020 3:00:42 PM)"=14246, "Automatic Update (DT: Olivine-3-1; HV: 2.2; Time: 1/9/2020 3:00:44 PM)"=14247, "Automatic Update (DT: Olivine-3-1; HV: 2.2; Time: 1/9/2020 3:00:45 PM)"=14248, "Automatic Update (DT: Olivine-3-1; HV: 2.2; Time: 1/9/2020 3:00:46 PM)"=14249, "Automatic Update (DT: Olivine-3-1; HV: 2.2; Time: 1/9/2020 3:00:47 PM)"=14250, "Automatic Update (DT: Olivine-3-1; HV: 2.2; Time: 1/9/2020 3:00:48 PM)"=14251, "Automatic Update (DT: Olivine-3-1; HV: 2.2; Time: 1/9/2020 3:00:49 PM)"=14252, "Automatic Update (DT: Olivine-3-1; HV: 2.2; Time: 1/9/2020 3:00:50 PM)"=14253, "Automatic Update (DT: Olivine-3-1; HV: 2.2; Time: 1/9/2020 3:00:51 PM)"=14254, "Automatic Update (DT: Olivine-3-1; HV: 2.2; Time: 1/9/2020 3:00:52 PM)"=14255, "Automatic Update (DT: Olivine-3-1; HV: 2.2; Time: 1/9/2020 3:00:53 PM)"=14256, "Automatic Update (DT: Olivine-3-1; HV: 2.2; Time: 1/9/2020 3:00:54 PM)"=14257, "Automatic Update (DT: Olivine-3-1; HV: 2.2; Time: 1/9/2020 3:00:57 PM)"=14258, "Automatic Update (DT: Olivine-3-1; HV: 2.2; Time: 1/9/2020 3:00:58 PM)"=14259, "Automatic Update (DT: Olivine-3-1; HV: 2.2; Time: 1/9/2020 3:00:59 PM)"=14260, "Automatic Update (DT: Olivine-3-1; HV: 2.2; Time: 1/9/2020 3:01:00 PM)"=14261, "Automatic Update (DT: Olivine-3-1; HV: 2.2; Time: 1/9/2020 3:01:01 PM)"=14262, "Automatic Update (DT: Olivine-3-1; HV: 2.2; Time: 1/9/2020 3:01:02 PM)"=14263, "Automatic Update (DT: Olivine-3-1; HV: 2.2; Time: 1/9/2020 3:01:03 PM)"=14264, "Automatic Update (DT: Olivine-3-1; HV: 2.2; Time: 1/9/2020 3:01:04 PM)"=14265, "Automatic Update (DT: Olivine-3-1; HV: 2.2; Time: 1/9/2020 3:01:05 PM)"=14266, "Automatic Update (DT: Olivine-3-1; HV: 2.2; Time: 1/9/2020 3:01:06 PM)"=14267, "Automatic Update (DT: Olivine-3-1; HV: 2.2; Time: 1/9/2020 3:01:07 PM)"=14268, "Automatic Update (DT: Olivine-3-1; HV: 2.2; Time: 1/9/2020 3:01:08 PM)"=14269, "Automatic Update (DT: Olivine-3-1; HV: 2.2; Time: 1/9/2020 3:01:10 PM)"=14270, "Automatic Update (DT: Olivine-3-1; HV: 2.2; Time: 1/9/2020 3:01:16 PM)"=14271, "Automatic Update (DT: Olivine-3-1; HV: 2.2; Time: 1/9/2020 3:01:17 PM)"=14272, "Automatic Update (DT: Olivine-3-1; HV: 2.2; Time: 1/9/2020 3:01:18 PM)"=14273, "Automatic Update (DT: Olivine-3-1; HV: 2.2; Time: 1/9/2020 3:01:19 PM)"=14274, "Automatic Update (DT: Olivine-3-1; HV: 2.2; Time: 1/9/2020 3:01:20 PM)"=14275, "Automatic Update (DT: Olivine-3-1; HV: 2.2; Time: 1/9/2020 3:01:21 PM)"=14276, "Automatic Update (DT: Olivine-3-1; HV: 2.2; Time: 1/9/2020 3:01:22 PM)"=14277, "Automatic Update (DT: Olivine-3-1; HV: 2.2; Time: 1/9/2020 3:01:23 PM)"=14278, "Automatic Update (DT: Olivine-3-1; HV: 2.2; Time: 1/9/2020 3:01:24 PM)"=14279, "Automatic Update (DT: Olivine-3-1; HV: 2.2; Time: 1/9/2020 3:01:25 PM)"=14280, "Automatic Update (DT: Olivine-3-1; HV: 2.2; Time: 1/9/2020 3:01:26 PM)"=14281, "Automatic Update (DT: Olivine-3-1; HV: 2.2; Time: 1/9/2020 3:01:30 PM)"=14282, "Automatic Update (DT: Olivine-3-1; HV: 2.2; Time: 1/9/2020 3:01:31 PM)"=14283, "Automatic Update (DT: Olivine-3-1; HV: 2.2; Time: 1/9/2020 3:01:32 PM)"=14284, "Automatic Update (DT: Olivine-3-1; HV: 2.2; Time: 1/9/2020 3:01:33 PM)"=14285, "Automatic Update (DT: Olivine-3-1; HV: 2.2; Time: 1/9/2020 3:01:34 PM)"=14286, "Automatic Update (DT: Olivine-3-1; HV: 2.2; Time: 1/9/2020 3:01:35 PM)"=14287, "Automatic Update (DT: Olivine-3-1; HV: 2.2; Time: 1/9/2020 3:01:36 PM)"=14288, "Automatic Update (DT: Olivine-3-1; HV: 2.2; Time: 1/9/2020 3:01:37 PM)"=14289, "Automatic Update (DT: Olivine-3-1; HV: 2.2; Time: 1/9/2020 3:01:39 PM)"=14290, "Automatic Update (DT: Olivine-3-1; HV: 2.2; Time: 1/9/2020 3:01:40 PM)"=14291, "Automatic Update (DT: Olivine-3-1; HV: 2.2; Time: 1/9/2020 3:01:41 PM)"=14292, "Automatic Update (DT: Olivine-3-1; HV: 2.2; Time: 1/9/2020 3:01:43 PM)"=14293, "Automatic Update (DT: Olivine-3-1; HV: 2.2; Time: 1/9/2020 3:01:44 PM)"=14294, "Automatic Update (DT: Olivine-3-1; HV: 2.2; Time: 1/9/2020 3:01:45 PM)"=14295, "Automatic Update (DT: Olivine-3-1; HV: 2.2; Time: 1/9/2020 3:01:46 PM)"=14296, "Automatic Update (DT: Olivine-3-1; HV: 2.2; Time: 1/9/2020 3:01:47 PM)"=14297, "Automatic Update (DT: Olivine-3-1; HV: 2.2; Time: 1/9/2020 3:01:48 PM)"=14298, "Automatic Update (DT: Olivine-3-1; HV: 2.2; Time: 1/9/2020 3:01:49 PM)"=14299, "Automatic Update (DT: Olivine-3-1; HV: 2.2; Time: 1/9/2020 3:01:50 PM)"=14300, "Automatic Update (DT: Olivine-3-1; HV: 2.2; Time: 1/9/2020 3:01:54 PM)"=14301, "Automatic Update (DT: Olivine-3-1; HV: 2.2; Time: 1/9/2020 3:01:55 PM)"=14302, "Automatic Update (DT: Olivine-3-1; HV: 2.2; Time: 1/9/2020 3:01:56 PM)"=14303, "Automatic Update (DT: Olivine-3-1; HV: 2.2; Time: 1/9/2020 3:01:57 PM)"=14304, "Automatic Update (DT: Olivine-3-1; HV: 2.2; Time: 1/9/2020 3:01:58 PM)"=14305, "Automatic Update (DT: Olivine-3-1; HV: 2.2; Time: 1/9/2020 3:02:00 PM)"=14306, "Automatic Update (DT: Olivine-3-1; HV: 2.2; Time: 1/9/2020 3:02:01 PM)"=14307, "Automatic Update (DT: Olivine-3-1; HV: 2.2; Time: 1/9/2020 3:02:02 PM)"=14308, "Automatic Update (DT: Olivine-3-1; HV: 2.2; Time: 1/9/2020 3:02:03 PM)"=14309, "Automatic Update (DT: Olivine-3-1; HV: 2.2; Time: 1/9/2020 3:02:04 PM)"=14310, "Automatic Update (DT: Olivine-3-1; HV: 2.2; Time: 1/9/2020 3:02:05 PM)"=14311, "Automatic Update (DT: Olivine-3-1; HV: 2.2; Time: 1/9/2020 3:02:06 PM)"=14312, "Automatic Update (DT: Olivine-3-1; HV: 2.2; Time: 1/9/2020 3:02:07 PM)"=14313, "Automatic Update (DT: Olivine-3-1; HV: 2.2; Time: 1/9/2020 3:02:08 PM)"=14314, "Automatic Update (DT: Olivine-3-1; HV: 2.2; Time: 1/9/2020 3:02:09 PM)"=14315, "Automatic Update (DT: Olivine-3-1; HV: 2.2; Time: 1/9/2020 3:02:11 PM)"=14316, "Automatic Update (DT: Olivine-3-1; HV: 2.2; Time: 1/9/2020 3:02:12 PM)"=14317, "Automatic Update (DT: Olivine-3-1; HV: 2.2; Time: 1/9/2020 3:02:14 PM)"=14318, "Automatic Update (DT: Olivine-3-1; HV: 2.2; Time: 1/9/2020 3:02:15 PM)"=14319, "Automatic Update (DT: Olivine-3-1; HV: 2.2; Time: 1/9/2020 3:02:16 PM)"=14320, "Automatic Update (DT: Olivine-3-1; HV: 2.2; Time: 1/9/2020 3:02:17 PM)"=14321, "Automatic Update (DT: Olivine-3-1; HV: 2.2; Time: 1/9/2020 3:02:18 PM)"=14322, "Automatic Update (DT: Olivine-3-1; HV: 2.2; Time: 1/9/2020 3:02:19 PM)"=14323, "Automatic Update (DT: Olivine-3-1; HV: 2.2; Time: 1/9/2020 3:02:20 PM)"=14324, "Automatic Update (DT: Olivine-3-1; HV: 2.2; Time: 1/9/2020 3:02:21 PM)"=14325, "Automatic Update (DT: Olivine-3-1; HV: 2.2; Time: 1/9/2020 3:02:22 PM)"=14326, "Automatic Update (DT: Olivine-3-1; HV: 2.2; Time: 1/9/2020 3:02:23 PM)"=14327, "Automatic Update (DT: Olivine-3-1; HV: 2.2; Time: 1/9/2020 3:02:24 PM)"=14328, "Automatic Update (DT: Olivine-3-1; HV: 2.2; Time: 1/9/2020 3:02:25 PM)"=14329, "Automatic Update (DT: Olivine-3-1; HV: 2.2; Time: 1/9/2020 3:02:26 PM)"=14330, "Automatic Update (DT: Olivine-3-1; HV: 2.2; Time: 1/9/2020 3:02:27 PM)"=14331, "Automatic Update (DT: Olivine-3-1; HV: 2.2; Time: 1/9/2020 3:02:28 PM)"=14332, "Automatic Update (DT: Olivine-3-1; HV: 2.2; Time: 1/9/2020 3:02:29 PM)"=14333, "Automatic Update (DT: Olivine-3-1; HV: 2.2; Time: 1/9/2020 3:02:41 PM)"=14334, "Automatic Update (DT: Olivine-3-1; HV: 2.2; Time: 1/9/2020 3:02:42 PM)"=14335, "Automatic Update (DT: Olivine-3-1; HV: 2.2; Time: 1/9/2020 3:02:43 PM)"=14336, "Automatic Update (DT: Olivine-3-1; HV: 2.2; Time: 1/9/2020 3:02:45 PM)"=14337, "Automatic Update (DT: Olivine-3-1; HV: 2.2; Time: 1/9/2020 3:02:46 PM)"=14338, "Automatic Update (DT: Olivine-3-1; HV: 2.2; Time: 1/9/2020 3:02:47 PM)"=14339, "Automatic Update (DT: Olivine-3-1; HV: 2.2; Time: 1/9/2020 3:02:48 PM)"=14340, "Automatic Update (DT: Olivine-3-1; HV: 2.2; Time: 1/9/2020 3:02:49 PM)"=14341, "Automatic Update (DT: Olivine-3-1; HV: 2.2; Time: 1/9/2020 3:02:50 PM)"=14342, "Automatic Update (DT: Olivine-3-1; HV: 2.2; Time: 1/9/2020 3:02:51 PM)"=14343, "Automatic Update (DT: Olivine-3-1; HV: 2.2; Time: 1/9/2020 3:02:52 PM)"=14344, "Automatic Update (DT: Olivine-3-1; HV: 2.2; Time: 1/9/2020 3:02:53 PM)"=14345, "Automatic Update (DT: Olivine-3-1; HV: 2.2; Time: 1/9/2020 3:02:54 PM)"=14346, "Automatic Update (DT: Olivine-3-1; HV: 2.2; Time: 1/9/2020 3:02:55 PM)"=14347, "Automatic Update (DT: Olivine-3-1; HV: 2.2; Time: 1/9/2020 3:02:56 PM)"=14348, "Automatic Update (DT: Olivine-3-1; HV: 2.2; Time: 1/9/2020 3:02:57 PM)"=14349, "Automatic Update (DT: Olivine-3-1; HV: 2.2; Time: 1/9/2020 3:02:58 PM)"=14350, "Automatic Update (DT: Olivine-3-1; HV: 2.2; Time: 1/9/2020 3:02:59 PM)"=14351, "Automatic Update (DT: Olivine-3-1; HV: 2.2; Time: 1/9/2020 3:03:00 PM)"=14352, "Automatic Update (DT: Olivine-3-1; HV: 2.2; Time: 1/9/2020 3:03:01 PM)"=14353, "Automatic Update (DT: Olivine-3-1; HV: 2.2; Time: 1/9/2020 3:03:02 PM)"=14354, "Automatic Update (DT: Olivine-3-1; HV: 2.2; Time: 1/9/2020 3:03:03 PM)"=14355, "Automatic Update (DT: Olivine-3-1; HV: 2.2; Time: 1/9/2020 3:03:04 PM)"=14356, "Automatic Update (DT: Olivine-3-1; HV: 2.2; Time: 1/9/2020 3:03:05 PM)"=14357, "Automatic Update (DT: Olivine-3-1; HV: 2.2; Time: 1/9/2020 3:03:06 PM)"=14358, "Automatic Update (DT: Olivine-3-1; HV: 2.2; Time: 1/9/2020 3:04:10 PM)"=14359, "Automatic Update (DT: Olivine-3-1; HV: 2.2; Time: 1/9/2020 3:04:11 PM)"=14360, "Automatic Update (DT: Olivine-3-1; HV: 2.2; Time: 1/9/2020 3:04:12 PM)"=14361, "Automatic Update (DT: Olivine-3-1; HV: 2.2; Time: 1/9/2020 3:04:13 PM)"=14362, "Automatic Update (DT: Olivine-3-1; HV: 2.2; Time: 1/9/2020 3:04:14 PM)"=14363, "Automatic Update (DT: Olivine-3-1; HV: 2.2; Time: 1/9/2020 3:04:15 PM)"=14364, "Automatic Update (DT: Olivine-3-1; HV: 2.2; Time: 1/9/2020 3:04:16 PM)"=14365, "Automatic Update (DT: Olivine-3-1; HV: 2.2; Time: 1/9/2020 3:04:17 PM)"=14366, "Automatic Update (DT: Olivine-3-1; HV: 2.2; Time: 1/9/2020 3:04:18 PM)"=14367, "Automatic Update (DT: Olivine-3-1; HV: 2.2; Time: 1/9/2020 3:04:19 PM)"=14368, "Automatic Update (DT: Olivine-3-1; HV: 2.2; Time: 1/9/2020 3:04:20 PM)"=14369, "Automatic Update (DT: Olivine-3-1; HV: 2.2; Time: 1/9/2020 3:04:21 PM)"=14370, "Automatic Update (DT: Olivine-3-1; HV: 2.2; Time: 1/9/2020 3:04:22 PM)"=14371, "Automatic Update (DT: Olivine-3-1; HV: 2.2; Time: 1/9/2020 3:04:23 PM)"=14372, "Automatic Update (DT: Olivine-3-1; HV: 2.2; Time: 1/9/2020 3:04:24 PM)"=14373, "Automatic Update (DT: Olivine-3-1; HV: 2.2; Time: 1/9/2020 3:04:25 PM)"=14374, "Automatic Update (DT: Olivine-3-1; HV: 2.2; Time: 1/9/2020 3:04:26 PM)"=14375, "Automatic Update (DT: Olivine-3-1; HV: 2.2; Time: 1/9/2020 3:04:28 PM)"=14376, "Automatic Update (DT: Olivine-3-1; HV: 2.2; Time: 1/9/2020 3:04:29 PM)"=14377, "Automatic Update (DT: Olivine-3-1; HV: 2.2; Time: 1/9/2020 3:04:30 PM)"=14378, "Automatic Update (DT: Olivine-3-1; HV: 2.2; Time: 1/9/2020 3:04:31 PM)"=14379, "Automatic Update (DT: Olivine-3-1; HV: 2.2; Time: 1/9/2020 3:04:35 PM)"=14380, "Automatic Update (DT: Olivine-3-1; HV: 2.2; Time: 1/9/2020 3:04:36 PM)"=14381, "Automatic Update (DT: Olivine-3-1; HV: 2.2; Time: 1/9/2020 3:04:37 PM)"=14382, "Automatic Update (DT: Olivine-3-1; HV: 2.2; Time: 1/9/2020 3:04:38 PM)"=14383, "Automatic Update (DT: Olivine-3-1; HV: 2.2; Time: 1/9/2020 3:04:39 PM)"=14384, "Automatic Update (DT: Olivine-3-1; HV: 2.2; Time: 1/9/2020 3:04:40 PM)"=14385, "Automatic Update (DT: Olivine-3-1; HV: 2.2; Time: 1/9/2020 3:04:41 PM)"=14386, "Automatic Update (DT: Olivine-3-1; HV: 2.2; Time: 1/9/2020 3:04:42 PM)"=14387, "Automatic Update (DT: Olivine-3-1; HV: 2.2; Time: 1/9/2020 3:04:44 PM)"=14388, "Automatic Update (DT: Olivine-3-1; HV: 2.2; Time: 1/9/2020 3:04:46 PM)"=14389, "Automatic Update (DT: Olivine-3-1; HV: 2.2; Time: 1/9/2020 3:04:47 PM)"=14390, "Automatic Update (DT: Olivine-3-1; HV: 2.2; Time: 1/9/2020 3:04:48 PM)"=14391, "Automatic Update (DT: Olivine-3-1; HV: 2.2; Time: 1/9/2020 3:04:49 PM)"=14392, "Automatic Update (DT: Olivine-3-1; HV: 2.2; Time: 1/9/2020 3:04:56 PM)"=14393, "Automatic Update (DT: Olivine-3-1; HV: 2.2; Time: 1/9/2020 3:04:57 PM)"=14394, "Automatic Update (DT: Olivine-3-1; HV: 2.2; Time: 1/9/2020 3:04:58 PM)"=14395, "Automatic Update (DT: Olivine-3-1; HV: 2.2; Time: 1/9/2020 3:04:59 PM)"=14396, "Automatic Update (DT: Olivine-3-1; HV: 2.2; Time: 1/9/2020 3:05:01 PM)"=14397, "Automatic Update (DT: Olivine-3-1; HV: 2.2; Time: 1/9/2020 3:05:02 PM)"=14398, "Automatic Update (DT: Olivine-3-1; HV: 2.2; Time: 1/9/2020 3:05:03 PM)"=14399, "Automatic Update (DT: Olivine-3-1; HV: 2.2; Time: 1/9/2020 3:05:04 PM)"=14400, "Automatic Update (DT: Olivine-3-1; HV: 2.2; Time: 1/9/2020 3:05:09 PM)"=14401, "Automatic Update (DT: Olivine-3-1; HV: 2.2; Time: 1/9/2020 3:05:10 PM)"=14402, "Automatic Update (DT: Olivine-3-1; HV: 2.2; Time: 1/9/2020 3:05:11 PM)"=14403, "Automatic Update (DT: Olivine-3-1; HV: 2.2; Time: 1/9/2020 3:05:12 PM)"=14404, "Automatic Update (DT: Olivine-3-1; HV: 2.2; Time: 1/9/2020 3:05:13 PM)"=14405, "Automatic Update (DT: Olivine-3-1; HV: 2.2; Time: 1/9/2020 3:05:14 PM)"=14406, "Automatic Update (DT: Olivine-3-1; HV: 2.2; Time: 1/9/2020 3:05:15 PM)"=14407, "Automatic Update (DT: Olivine-3-1; HV: 2.2; Time: 1/9/2020 3:05:19 PM)"=14408, "Automatic Update (DT: Olivine-3-1; HV: 2.2; Time: 1/9/2020 3:05:20 PM)"=14409, "Automatic Update (DT: Olivine-3-1; HV: 2.2; Time: 1/9/2020 3:05:21 PM)"=14410, "Automatic Update (DT: Olivine-3-1; HV: 2.2; Time: 1/9/2020 3:05:22 PM)"=14411, "Automatic Update (DT: Olivine-3-1; HV: 2.2; Time: 1/9/2020 3:05:23 PM)"=14412, "Automatic Update (DT: Olivine-3-1; HV: 2.2; Time: 1/9/2020 3:05:24 PM)"=14413, "Automatic Update (DT: Olivine-3-1; HV: 2.2; Time: 1/9/2020 3:05:25 PM)"=14414, "Automatic Update (DT: Olivine-3-1; HV: 2.2; Time: 1/9/2020 3:05:26 PM)"=14415, "Automatic Update (DT: Olivine-3-1; HV: 2.2; Time: 1/9/2020 3:05:27 PM)"=14416, "Automatic Update (DT: Olivine-3-1; HV: 2.2; Time: 1/9/2020 3:05:28 PM)"=14417, "Automatic Update (DT: Olivine-3-1; HV: 2.2; Time: 1/9/2020 3:05:29 PM)"=14418, "Automatic Update (DT: Olivine-3-1; HV: 2.2; Time: 1/9/2020 3:05:31 PM)"=14419, "Automatic Update (DT: Olivine-3-1; HV: 2.2; Time: 1/9/2020 3:05:36 PM)"=14420, "Automatic Update (DT: Olivine-3-1; HV: 2.2; Time: 1/9/2020 3:05:37 PM)"=14421, "Automatic Update (DT: Olivine-3-1; HV: 2.2; Time: 1/9/2020 3:05:38 PM)"=14422, "Automatic Update (DT: Olivine-3-1; HV: 2.2; Time: 1/9/2020 3:05:41 PM)"=14423, "Automatic Update (DT: Olivine-3-1; HV: 2.2; Time: 1/9/2020 3:05:42 PM)"=14424, "Automatic Update (DT: Olivine-3-1; HV: 2.2; Time: 1/9/2020 3:05:43 PM)"=14425, "Automatic Update (DT: Olivine-3-1; HV: 2.2; Time: 1/9/2020 3:05:53 PM)"=14426, "Automatic Update (DT: Olivine-3-1; HV: 2.2; Time: 1/9/2020 3:05:54 PM)"=14427, "Automatic Update (DT: Olivine-3-1; HV: 2.2; Time: 1/9/2020 3:05:55 PM)"=14428, "Automatic Update (DT: Olivine-3-1; HV: 2.2; Time: 1/9/2020 3:05:56 PM)"=14429, "Automatic Update (DT: Olivine-3-1; HV: 2.2; Time: 1/9/2020 3:06:12 PM)"=14430, "Automatic Update (DT: Olivine-3-1; HV: 2.2; Time: 1/9/2020 3:06:13 PM)"=14431, "Automatic Update (DT: Olivine-3-1; HV: 2.2; Time: 1/9/2020 3:06:14 PM)"=14432, "Automatic Update (DT: Olivine-3-1; HV: 2.2; Time: 1/9/2020 3:06:15 PM)"=14433, "Automatic Update (DT: Olivine-3-1; HV: 2.2; Time: 1/9/2020 3:06:22 PM)"=14434, "Automatic Update (DT: Olivine-3-1; HV: 2.2; Time: 1/9/2020 3:06:23 PM)"=14435, "Automatic Update (DT: Olivine-3-1; HV: 2.2; Time: 1/9/2020 3:06:27 PM)"=14436, "Automatic Update (DT: Olivine-3-1; HV: 2.2; Time: 1/9/2020 3:06:28 PM)"=14437, "Automatic Update (DT: Olivine-3-1; HV: 2.2; Time: 1/9/2020 3:06:29 PM)"=14438, "Automatic Update (DT: Olivine-3-1; HV: 2.2; Time: 1/9/2020 3:06:34 PM)"=14439, "Automatic Update (DT: Olivine-3-1; HV: 2.2; Time: 1/9/2020 3:06:35 PM)"=14440, "Automatic Update (DT: Olivine-3-1; HV: 2.2; Time: 1/9/2020 3:06:36 PM)"=14441, "Automatic Update (DT: Olivine-3-1; HV: 2.2; Time: 1/9/2020 3:06:44 PM)"=14442, "Automatic Update (DT: Olivine-3-1; HV: 2.2; Time: 1/9/2020 3:06:45 PM)"=14443, "Automatic Update (DT: Olivine-3-1; HV: 2.2; Time: 1/9/2020 3:06:46 PM)"=14444, "Automatic Update (DT: Olivine-3-1; HV: 2.2; Time: 1/9/2020 3:06:47 PM)"=14445, "Automatic Update (DT: Olivine-3-1; HV: 2.2; Time: 1/9/2020 3:06:55 PM)"=14446, "Automatic Update (DT: Olivine-3-1; HV: 2.2; Time: 1/9/2020 3:06:56 PM)"=14447, "Automatic Update (DT: Olivine-3-1; HV: 2.2; Time: 1/9/2020 3:07:00 PM)"=14448, "Automatic Update (DT: Olivine-3-1; HV: 2.2; Time: 1/9/2020 3:07:11 PM)"=14449, "Automatic Update (DT: Olivine-3-1; HV: 2.2; Time: 1/9/2020 3:07:12 PM)"=14450, "Automatic Update (DT: Olivine-3-1; HV: 2.2; Time: 1/9/2020 3:10:06 PM)"=14451, "Automatic Update (DT: Olivine-3-1; HV: 2.2; Time: 1/9/2020 3:10:07 PM)"=14452, "Automatic Update (DT: Olivine-3-1; HV: 2.2; Time: 1/9/2020 3:10:08 PM)"=14453, "Automatic Update (DT: Olivine-3-1; HV: 2.2; Time: 1/9/2020 3:10:09 PM)"=14454, "Automatic Update (DT: Olivine-3-1; HV: 2.2; Time: 1/9/2020 3:10:12 PM)"=14455, "Automatic Update (DT: Olivine-3-1; HV: 2.2; Time: 1/9/2020 3:10:13 PM)"=14456, "Automatic Update (DT: Olivine-3-1; HV: 2.2; Time: 1/9/2020 3:10:24 PM)"=14457, "Automatic Update (DT: Olivine-3-1; HV: 2.2; Time: 1/10/2020 12:59:22 AM)"=14458, "Automatic Update (DT: Olivine-3-1; HV: 2.2; Time: 1/10/2020 12:59:23 AM)"=14459, "Automatic Update (DT: Olivine-3-1; HV: 2.2; Time: 1/10/2020 12:59:24 AM)"=14460, "Automatic Update (DT: Olivine-3-1; HV: 2.2; Time: 1/10/2020 12:59:25 AM)"=14461, "Automatic Update (DT: Olivine-3-1; HV: 2.2; Time: 1/10/2020 12:59:27 AM)"=14462, "Automatic Update (DT: Olivine-3-1; HV: 2.2; Time: 1/10/2020 12:59:28 AM)"=14463, "Automatic Update (DT: Olivine-3-1; HV: 2.2; Time: 1/10/2020 12:59:29 AM)"=14464, "Automatic Update (DT: Olivine-3-1; HV: 2.2; Time: 1/10/2020 12:59:30 AM)"=14465, "Automatic Update (DT: Olivine-3-1; HV: 2.2; Time: 1/10/2020 12:59:31 AM)"=14466, "Automatic Update (DT: Olivine-3-1; HV: 2.2; Time: 1/10/2020 12:59:32 AM)"=14467, "Automatic Update (DT: Olivine-3-1; HV: 2.2; Time: 1/10/2020 12:59:33 AM)"=14468, "Automatic Update (DT: Olivine-3-1; HV: 2.2; Time: 1/10/2020 12:59:34 AM)"=14469, "Automatic Update (DT: Olivine-3-1; HV: 2.2; Time: 1/10/2020 12:59:35 AM)"=14470, "Automatic Update (DT: Olivine-3-1; HV: 2.2; Time: 1/10/2020 12:59:36 AM)"=14471, "Automatic Update (DT: Olivine-3-1; HV: 2.2; Time: 1/10/2020 12:59:37 AM)"=14472, "Automatic Update (DT: Olivine-3-1; HV: 2.2; Time: 1/10/2020 12:59:38 AM)"=14473, "Automatic Update (DT: Olivine-3-1; HV: 2.2; Time: 1/10/2020 12:59:39 AM)"=14474, "Automatic Update (DT: Olivine-3-1; HV: 2.2; Time: 1/10/2020 12:59:40 AM)"=14475, "Automatic Update (DT: Olivine-3-1; HV: 2.2; Time: 1/10/2020 12:59:41 AM)"=14476, "Automatic Update (DT: Olivine-3-1; HV: 2.2; Time: 1/10/2020 12:59:42 AM)"=14477, "Automatic Update (DT: Olivine-3-1; HV: 2.2; Time: 1/10/2020 12:59:44 AM)"=14478, "Automatic Update (DT: Olivine-3-1; HV: 2.2; Time: 1/10/2020 12:59:45 AM)"=14479, "Automatic Update (DT: Olivine-3-1; HV: 2.2; Time: 1/10/2020 12:59:46 AM)"=14480, "Automatic Update (DT: Olivine-3-1; HV: 2.2; Time: 1/10/2020 12:59:47 AM)"=14481, "Automatic Update (DT: Olivine-3-1; HV: 2.2; Time: 1/10/2020 12:59:51 AM)"=14482, "Automatic Update (DT: Olivine-3-1; HV: 2.2; Time: 1/10/2020 12:59:52 AM)"=14483, "Automatic Update (DT: Olivine-3-1; HV: 2.2; Time: 1/10/2020 12:59:53 AM)"=14484, "Automatic Update (DT: Olivine-3-1; HV: 2.2; Time: 1/10/2020 12:59:54 AM)"=14485, "Automatic Update (DT: Olivine-3-1; HV: 2.2; Time: 1/10/2020 12:59:55 AM)"=14486, "Automatic Update (DT: Olivine-3-1; HV: 2.2; Time: 1/10/2020 12:59:56 AM)"=14487, "Automatic Update (DT: Olivine-3-1; HV: 2.2; Time: 1/10/2020 12:59:57 AM)"=14488, "Automatic Update (DT: Olivine-3-1; HV: 2.2; Time: 1/10/2020 12:59:58 AM)"=14489, "Automatic Update (DT: Olivine-3-1; HV: 2.2; Time: 1/10/2020 12:59:59 AM)"=14490, "Automatic Update (DT: Olivine-3-1; HV: 2.2; Time: 1/10/2020 1:00:00 AM)"=14491, "Automatic Update (DT: Olivine-3-1; HV: 2.2; Time: 1/10/2020 1:00:01 AM)"=14492, "Automatic Update (DT: Olivine-3-1; HV: 2.2; Time: 1/10/2020 1:00:02 AM)"=14493, "Automatic Update (DT: Olivine-3-1; HV: 2.2; Time: 1/10/2020 1:00:03 AM)"=14494, "Automatic Update (DT: Olivine-3-1; HV: 2.2; Time: 1/10/2020 1:00:04 AM)"=14495, "Automatic Update (DT: Olivine-3-1; HV: 2.2; Time: 1/10/2020 1:00:05 AM)"=14496, "Automatic Update (DT: Olivine-3-1; HV: 2.2; Time: 1/10/2020 1:00:06 AM)"=14497, "Automatic Update (DT: Olivine-3-1; HV: 2.2; Time: 1/10/2020 1:00:07 AM)"=14498, "Automatic Update (DT: Olivine-3-1; HV: 2.2; Time: 1/10/2020 1:00:09 AM)"=14499, "Automatic Update (DT: Olivine-3-1; HV: 2.2; Time: 1/10/2020 1:00:10 AM)"=14500, "Automatic Update (DT: Olivine-3-1; HV: 2.2; Time: 1/10/2020 1:00:11 AM)"=14501, "Automatic Update (DT: Olivine-3-1; HV: 2.2; Time: 1/10/2020 1:00:12 AM)"=14502, "Automatic Update (DT: Olivine-3-1; HV: 2.2; Time: 1/10/2020 1:00:13 AM)"=14503, "Automatic Update (DT: Olivine-3-1; HV: 2.2; Time: 1/10/2020 1:00:14 AM)"=14504, "Automatic Update (DT: Olivine-3-1; HV: 2.2; Time: 1/10/2020 1:18:29 AM)"=14505, "Automatic Update (DT: Olivine-3-1; HV: 2.2; Time: 1/15/2020 10:09:50 AM)"=14506, "Automatic Update (DT: Olivine-3-1; HV: 2.2; Time: 1/15/2020 10:09:52 AM)"=14507, "Automatic Update (DT: Olivine-3-1; HV: 2.2; Time: 1/15/2020 10:09:54 AM)"=14508, "Automatic Update (DT: Olivine-3-1; HV: 2.2; Time: 1/15/2020 10:09:55 AM)"=14509, "Automatic Update (DT: Olivine-3-1; HV: 2.2; Time: 1/15/2020 10:09:57 AM)"=14510, "Automatic Update (DT: Olivine-3-1; HV: 2.2; Time: 1/15/2020 10:09:59 AM)"=14511, "Automatic Update (DT: Olivine-3-1; HV: 2.2; Time: 1/15/2020 10:10:01 AM)"=14512, "Automatic Update (DT: Olivine-3-1; HV: 2.2; Time: 1/15/2020 10:10:02 AM)"=14513, "Automatic Update (DT: Olivine-3-1; HV: 2.2; Time: 1/15/2020 10:10:13 AM)"=14514, "Automatic Update (DT: Olivine-3-1; HV: 2.2; Time: 1/15/2020 10:10:18 AM)"=14515, "Automatic Update (DT: Olivine-3-1; HV: 2.2; Time: 1/15/2020 10:10:20 AM)"=14516, "Automatic Update (DT: Olivine-3-1; HV: 2.2; Time: 1/15/2020 10:10:26 AM)"=14517, "Automatic Update (DT: Olivine-3-1; HV: 2.2; Time: 1/15/2020 10:10:35 AM)"=14518, "Automatic Update (DT: Olivine-3-1; HV: 2.2; Time: 1/15/2020 10:10:40 AM)"=14519, "Automatic Update (DT: Olivine-3-1; HV: 2.2; Time: 1/15/2020 10:10:42 AM)"=14520, "Automatic Update (DT: Olivine-3-1; HV: 2.2; Time: 1/15/2020 10:10:46 AM)"=14521, "Automatic Update (DT: Olivine-3-1; HV: 2.2; Time: 1/15/2020 10:10:48 AM)"=14522, "Automatic Update (DT: Olivine-3-1; HV: 2.2; Time: 1/15/2020 10:10:50 AM)"=14523, "Automatic Update (DT: Olivine-3-1; HV: 2.2; Time: 1/15/2020 10:10:52 AM)"=14524, "Automatic Update (DT: Olivine-3-1; HV: 2.2; Time: 1/15/2020 10:10:55 AM)"=14525, "Automatic Update (DT: Olivine-3-1; HV: 2.2; Time: 1/15/2020 10:10:56 AM)"=14526, "Automatic Update (DT: Olivine-3-1; HV: 2.2; Time: 1/15/2020 10:10:58 AM)"=14527, "Automatic Update (DT: Olivine-3-1; HV: 2.2; Time: 1/15/2020 10:16:39 AM)"=14528, "Automatic Update (DT: Olivine-3-1; HV: 2.2; Time: 1/15/2020 10:16:40 AM)"=14529, "Automatic Update (DT: Olivine-3-1; HV: 2.2; Time: 1/15/2020 10:16:41 AM)"=14530, "Automatic Update (DT: Olivine-3-1; HV: 2.2; Time: 1/15/2020 10:16:45 AM)"=14531, "Automatic Update (DT: Olivine-3-1; HV: 2.2; Time: 1/15/2020 10:16:46 AM)"=14532, "Automatic Update (DT: Olivine-3-1; HV: 2.2; Time: 1/15/2020 10:16:48 AM)"=14533, "Automatic Update (DT: Olivine-3-1; HV: 2.2; Time: 1/15/2020 10:16:49 AM)"=14534, "Automatic Update (DT: Olivine-3-1; HV: 2.2; Time: 1/15/2020 10:16:50 AM)"=14535, "Automatic Update (DT: Olivine-3-1; HV: 2.2; Time: 1/15/2020 10:16:51 AM)"=14536, "Automatic Update (DT: Olivine-3-1; HV: 2.2; Time: 1/15/2020 10:16:54 AM)"=14537, "Automatic Update (DT: Olivine-3-1; HV: 2.2; Time: 1/15/2020 10:16:55 AM)"=14538, "Automatic Update (DT: Olivine-3-1; HV: 2.2; Time: 1/15/2020 10:16:56 AM)"=14539, "Automatic Update (DT: Olivine-3-1; HV: 2.2; Time: 1/15/2020 10:16:57 AM)"=14540, "Automatic Update (DT: Olivine-3-1; HV: 2.2; Time: 1/15/2020 10:16:59 AM)"=14541, "Automatic Update (DT: Olivine-3-1; HV: 2.2; Time: 1/15/2020 10:17:00 AM)"=14542, "Automatic Update (DT: Olivine-3-1; HV: 2.2; Time: 1/15/2020 10:17:03 AM)"=14543, "Automatic Update (DT: Olivine-3-1; HV: 2.2; Time: 1/15/2020 10:17:04 AM)"=14544, "Automatic Update (DT: Olivine-3-1; HV: 2.2; Time: 1/15/2020 10:17:05 AM)"=14545, "Automatic Update (DT: Olivine-3-1; HV: 2.2; Time: 1/15/2020 10:17:06 AM)"=14546, "Automatic Update (DT: Olivine-3-1; HV: 2.2; Time: 1/15/2020 10:17:08 AM)"=14547, "Automatic Update (DT: Olivine-3-1; HV: 2.2; Time: 1/15/2020 10:17:12 AM)"=14548, "Automatic Update (DT: Olivine-3-1; HV: 2.2; Time: 1/15/2020 10:17:13 AM)"=14549, "Automatic Update (DT: Olivine-3-1; HV: 2.2; Time: 1/15/2020 10:17:14 AM)"=14550, "Automatic Update (DT: Olivine-3-1; HV: 2.2; Time: 1/15/2020 10:17:15 AM)"=14551, "Automatic Update (DT: Olivine-3-1; HV: 2.2; Time: 1/15/2020 10:17:16 AM)"=14552, "Automatic Update (DT: Olivine-3-1; HV: 2.2; Time: 1/15/2020 10:17:17 AM)"=14553, "Automatic Update (DT: Olivine-3-1; HV: 2.2; Time: 1/15/2020 10:17:21 AM)"=14554, "Automatic Update (DT: Olivine-3-1; HV: 2.2; Time: 1/15/2020 10:17:23 AM)"=14555, "Automatic Update (DT: Olivine-3-1; HV: 2.2; Time: 1/15/2020 10:17:25 AM)"=14556, "Automatic Update (DT: Olivine-3-1; HV: 2.2; Time: 1/15/2020 10:17:26 AM)"=14557, "Automatic Update (DT: Olivine-3-1; HV: 2.2; Time: 1/15/2020 10:17:30 AM)"=14558, "Automatic Update (DT: Olivine-3-1; HV: 2.2; Time: 1/15/2020 10:17:31 AM)"=14559, "Automatic Update (DT: Olivine-3-1; HV: 2.2; Time: 1/15/2020 10:17:32 AM)"=14560, "Automatic Update (DT: Olivine-3-1; HV: 2.2; Time: 1/15/2020 10:17:33 AM)"=14561, "Automatic Update (DT: Olivine-3-1; HV: 2.2; Time: 1/15/2020 10:17:34 AM)"=14562, "Automatic Update (DT: Olivine-3-1; HV: 2.2; Time: 1/15/2020 10:17:35 AM)"=14563, "Automatic Update (DT: Olivine-3-1; HV: 2.2; Time: 1/15/2020 10:17:38 AM)"=14564, "Automatic Update (DT: Olivine-3-1; HV: 2.2; Time: 1/15/2020 10:17:39 AM)"=14565, "Automatic Update (DT: Olivine-3-1; HV: 2.2; Time: 1/15/2020 10:17:41 AM)"=14566, "Automatic Update (DT: Olivine-3-1; HV: 2.2; Time: 1/15/2020 10:17:43 AM)"=14567, "Automatic Update (DT: Olivine-3-1; HV: 2.2; Time: 1/15/2020 10:17:44 AM)"=14568, "Automatic Update (DT: Olivine-3-1; HV: 2.2; Time: 1/15/2020 10:17:47 AM)"=14569, "Automatic Update (DT: Olivine-3-1; HV: 2.2; Time: 1/15/2020 10:17:48 AM)"=14570, "Automatic Update (DT: Olivine-3-1; HV: 2.2; Time: 1/15/2020 10:17:51 AM)"=14571, "Automatic Update (DT: Olivine-3-1; HV: 2.2; Time: 1/15/2020 10:17:52 AM)"=14572, "Automatic Update (DT: Olivine-3-1; HV: 2.2; Time: 1/15/2020 10:17:56 AM)"=14573, "Automatic Update (DT: Olivine-3-1; HV: 2.2; Time: 1/15/2020 10:17:57 AM)"=14574, "Automatic Update (DT: Olivine-3-1; HV: 2.2; Time: 1/15/2020 10:17:59 AM)"=14575, "Automatic Update (DT: Olivine-3-1; HV: 2.2; Time: 1/15/2020 10:18:00 AM)"=14576, "Automatic Update (DT: Olivine-3-1; HV: 2.2; Time: 1/15/2020 10:18:09 AM)"=14577, "Automatic Update (DT: Olivine-3-1; HV: 2.2; Time: 1/15/2020 10:18:14 AM)"=14578, "Automatic Update (DT: Olivine-3-1; HV: 2.2; Time: 1/15/2020 10:18:25 AM)"=14579, "Automatic Update (DT: Olivine-3-1; HV: 2.2; Time: 1/15/2020 10:18:26 AM)"=14580, "Automatic Update (DT: Olivine-3-1; HV: 2.2; Time: 1/15/2020 10:18:28 AM)"=14581, "Automatic Update (DT: Olivine-3-1; HV: 2.2; Time: 1/15/2020 10:18:32 AM)"=14582, "Automatic Update (DT: Olivine-3-1; HV: 2.2; Time: 1/15/2020 10:18:35 AM)"=14583, "Automatic Update (DT: Olivine-3-1; HV: 2.2; Time: 1/15/2020 10:18:36 AM)"=14584, "Automatic Update (DT: Olivine-3-1; HV: 2.2; Time: 1/15/2020 10:18:37 AM)"=14585, "Automatic Update (DT: Olivine-3-1; HV: 2.2; Time: 1/15/2020 10:18:40 AM)"=14586, "Automatic Update (DT: Olivine-3-1; HV: 2.2; Time: 1/15/2020 10:18:41 AM)"=14587, "Automatic Update (DT: Olivine-3-1; HV: 2.2; Time: 1/15/2020 10:18:44 AM)"=14588, "Automatic Update (DT: Olivine-3-1; HV: 2.2; Time: 1/15/2020 10:18:46 AM)"=14589, "Automatic Update (DT: Olivine-3-1; HV: 2.2; Time: 1/15/2020 10:18:49 AM)"=14590, "Automatic Update (DT: Olivine-3-1; HV: 2.2; Time: 1/15/2020 10:19:11 AM)"=14591, "Automatic Update (DT: Olivine-3-1; HV: 2.2; Time: 1/15/2020 10:19:16 AM)"=14592, "Automatic Update (DT: Olivine-3-1; HV: 2.2; Time: 1/15/2020 10:19:17 AM)"=14593, "Automatic Update (DT: Olivine-3-1; HV: 2.2; Time: 1/15/2020 10:19:18 AM)"=14594, "Automatic Update (DT: Olivine-3-1; HV: 2.2; Time: 1/15/2020 10:19:20 AM)"=14595, "Automatic Update (DT: Olivine-3-1; HV: 2.2; Time: 1/15/2020 10:19:21 AM)"=14596, "Automatic Update (DT: Olivine-3-1; HV: 2.2; Time: 1/15/2020 10:19:24 AM)"=14597, "Automatic Update (DT: Olivine-3-1; HV: 2.2; Time: 1/15/2020 10:19:26 AM)"=14598, "Automatic Update (DT: Olivine-3-1; HV: 2.2; Time: 1/15/2020 10:19:27 AM)"=14599, "Automatic Update (DT: Olivine-3-1; HV: 2.2; Time: 1/15/2020 10:19:29 AM)"=14600, "Automatic Update (DT: Olivine-3-1; HV: 2.2; Time: 1/15/2020 10:19:30 AM)"=14601, "Automatic Update (DT: Olivine-3-1; HV: 2.2; Time: 1/15/2020 10:19:33 AM)"=14602, "Automatic Update (DT: Olivine-3-1; HV: 2.2; Time: 1/15/2020 10:20:50 AM)"=14603, "Automatic Update (DT: Olivine-3-1; HV: 2.2; Time: 1/15/2020 10:20:54 AM)"=14604, "Automatic Update (DT: Olivine-3-1; HV: 2.2; Time: 1/15/2020 10:20:55 AM)"=14605, "Automatic Update (DT: Olivine-3-1; HV: 2.2; Time: 1/15/2020 10:20:56 AM)"=14606, "Automatic Update (DT: Olivine-3-1; HV: 2.2; Time: 1/15/2020 10:20:57 AM)"=14607, "Automatic Update (DT: Olivine-3-1; HV: 2.2; Time: 1/15/2020 10:20:58 AM)"=14608, "Automatic Update (DT: Olivine-3-1; HV: 2.2; Time: 1/15/2020 10:20:59 AM)"=14609, "Automatic Update (DT: Olivine-3-1; HV: 2.2; Time: 1/15/2020 10:21:03 AM)"=14610, "Automatic Update (DT: Olivine-3-1; HV: 2.2; Time: 1/15/2020 10:21:05 AM)"=14611, "Automatic Update (DT: Olivine-3-1; HV: 2.2; Time: 1/15/2020 10:21:06 AM)"=14612, "Automatic Update (DT: Olivine-3-1; HV: 2.2; Time: 1/15/2020 10:21:07 AM)"=14613, "Automatic Update (DT: Olivine-3-1; HV: 2.2; Time: 1/15/2020 10:21:08 AM)"=14614, "Automatic Update (DT: Olivine-3-1; HV: 2.2; Time: 1/15/2020 10:21:12 AM)"=14615, "Automatic Update (DT: Olivine-3-1; HV: 2.2; Time: 1/15/2020 10:21:13 AM)"=14616, "Automatic Update (DT: Olivine-3-1; HV: 2.2; Time: 1/15/2020 10:21:15 AM)"=14617, "Automatic Update (DT: Olivine-3-1; HV: 2.2; Time: 1/15/2020 10:21:16 AM)"=14618, "Automatic Update (DT: Olivine-3-1; HV: 2.2; Time: 1/15/2020 10:21:17 AM)"=14619, "Automatic Update (DT: Olivine-3-1; HV: 2.2; Time: 1/15/2020 10:21:18 AM)"=14620, "Automatic Update (DT: Olivine-3-1; HV: 2.2; Time: 1/15/2020 10:21:21 AM)"=14621, "Automatic Update (DT: Olivine-3-1; HV: 2.2; Time: 1/15/2020 10:21:22 AM)"=14622, "Automatic Update (DT: Olivine-3-1; HV: 2.2; Time: 1/15/2020 10:21:28 AM)"=14623, "Automatic Update (DT: Olivine-3-1; HV: 2.2; Time: 1/15/2020 10:21:30 AM)"=14624, "Automatic Update (DT: Olivine-3-1; HV: 2.2; Time: 1/15/2020 10:21:31 AM)"=14625, "Automatic Update (DT: Olivine-3-1; HV: 2.2; Time: 1/15/2020 10:21:33 AM)"=14626, "Automatic Update (DT: Olivine-3-1; HV: 2.2; Time: 1/15/2020 10:21:34 AM)"=14627, "Automatic Update (DT: Olivine-3-1; HV: 2.2; Time: 1/15/2020 10:21:39 AM)"=14628, "Automatic Update (DT: Olivine-3-1; HV: 2.2; Time: 1/15/2020 10:21:40 AM)"=14629, "Automatic Update (DT: Olivine-3-1; HV: 2.2; Time: 1/15/2020 10:21:41 AM)"=14630, "Automatic Update (DT: Olivine-3-1; HV: 2.2; Time: 1/15/2020 10:21:42 AM)"=14631, "Automatic Update (DT: Olivine-3-1; HV: 2.2; Time: 1/15/2020 10:21:45 AM)"=14632, "Automatic Update (DT: Olivine-3-1; HV: 2.2; Time: 1/15/2020 10:21:50 AM)"=14633, "Automatic Update (DT: Olivine-3-1; HV: 2.2; Time: 1/15/2020 10:21:51 AM)"=14634, "Automatic Update (DT: Olivine-3-1; HV: 2.2; Time: 1/15/2020 10:22:02 AM)"=14635, "Automatic Update (DT: Olivine-3-1; HV: 2.2; Time: 1/15/2020 10:22:03 AM)"=14636, "Automatic Update (DT: Olivine-3-1; HV: 2.2; Time: 1/15/2020 10:22:06 AM)"=14637, "Automatic Update (DT: Olivine-3-1; HV: 2.2; Time: 1/15/2020 10:22:07 AM)"=14638, "Automatic Update (DT: Olivine-3-1; HV: 2.2; Time: 1/15/2020 10:22:09 AM)"=14639, "Automatic Update (DT: Olivine-3-1; HV: 2.2; Time: 1/15/2020 10:22:11 AM)"=14640, "Automatic Update (DT: Olivine-3-1; HV: 2.2; Time: 1/15/2020 10:22:12 AM)"=14641, "Automatic Update (DT: Olivine-3-1; HV: 2.2; Time: 1/15/2020 10:22:16 AM)"=14642, "Automatic Update (DT: Olivine-3-1; HV: 2.2; Time: 1/15/2020 10:22:20 AM)"=14643, "Automatic Update (DT: Olivine-3-1; HV: 2.2; Time: 1/15/2020 10:22:22 AM)"=14644, "Automatic Update (DT: Olivine-3-1; HV: 2.2; Time: 1/15/2020 10:22:25 AM)"=14645, "Automatic Update (DT: Olivine-3-1; HV: 2.2; Time: 1/15/2020 10:22:27 AM)"=14646, "Automatic Update (DT: Olivine-3-1; HV: 2.2; Time: 1/15/2020 10:22:28 AM)"=14647, "Automatic Update (DT: Olivine-3-1; HV: 2.2; Time: 1/15/2020 10:22:29 AM)"=14648, "Automatic Update (DT: Olivine-3-1; HV: 2.2; Time: 1/15/2020 10:22:30 AM)"=14649, "Automatic Update (DT: Olivine-3-1; HV: 2.2; Time: 1/15/2020 10:22:34 AM)"=14650, "Automatic Update (DT: Olivine-3-1; HV: 2.2; Time: 1/15/2020 10:22:35 AM)"=14651, "Automatic Update (DT: Olivine-3-1; HV: 2.2; Time: 1/15/2020 10:22:36 AM)"=14652, "Automatic Update (DT: Olivine-3-1; HV: 2.2; Time: 1/15/2020 10:22:37 AM)"=14653, "Automatic Update (DT: Olivine-3-1; HV: 2.2; Time: 1/15/2020 10:22:40 AM)"=14654, "Automatic Update (DT: Olivine-3-1; HV: 2.2; Time: 1/15/2020 10:22:43 AM)"=14655, "Automatic Update (DT: Olivine-3-1; HV: 2.2; Time: 1/15/2020 10:22:44 AM)"=14656, "Automatic Update (DT: Olivine-3-1; HV: 2.2; Time: 1/15/2020 10:22:51 AM)"=14657, "Automatic Update (DT: Olivine-3-1; HV: 2.2; Time: 1/15/2020 10:22:52 AM)"=14658, "Automatic Update (DT: Olivine-3-1; HV: 2.2; Time: 1/15/2020 10:22:53 AM)"=14659, "Automatic Update (DT: Olivine-3-1; HV: 2.2; Time: 1/15/2020 10:22:54 AM)"=14660, "Automatic Update (DT: Olivine-3-1; HV: 2.2; Time: 1/15/2020 10:22:59 AM)"=14661, "Automatic Update (DT: Olivine-3-1; HV: 2.2; Time: 1/15/2020 10:23:01 AM)"=14662, "Automatic Update (DT: Olivine-3-1; HV: 2.2; Time: 1/15/2020 10:23:02 AM)"=14663, "Automatic Update (DT: Olivine-3-1; HV: 2.2; Time: 1/15/2020 10:23:03 AM)"=14664, "Automatic Update (DT: Olivine-3-1; HV: 2.2; Time: 1/15/2020 10:23:04 AM)"=14665, "Automatic Update (DT: Olivine-3-1; HV: 2.2; Time: 1/15/2020 10:23:05 AM)"=14666, "Automatic Update (DT: Olivine-3-1; HV: 2.2; Time: 1/15/2020 10:23:06 AM)"=14667, "Automatic Update (DT: Olivine-3-1; HV: 2.2; Time: 1/15/2020 10:23:10 AM)"=14668, "Automatic Update (DT: Olivine-3-1; HV: 2.2; Time: 1/15/2020 10:23:11 AM)"=14669, "Automatic Update (DT: Olivine-3-1; HV: 2.2; Time: 1/15/2020 10:23:12 AM)"=14670, "Automatic Update (DT: Olivine-3-1; HV: 2.2; Time: 1/15/2020 10:23:15 AM)"=14671, "Automatic Update (DT: Olivine-3-1; HV: 2.2; Time: 1/15/2020 10:23:19 AM)"=14672, "Automatic Update (DT: Olivine-3-1; HV: 2.2; Time: 1/15/2020 10:23:20 AM)"=14673, "Automatic Update (DT: Olivine-3-1; HV: 2.2; Time: 1/15/2020 10:23:21 AM)"=14674, "Automatic Update (DT: Olivine-3-1; HV: 2.2; Time: 1/15/2020 10:23:22 AM)"=14675, "Automatic Update (DT: Olivine-3-1; HV: 2.2; Time: 1/15/2020 10:23:23 AM)"=14676, "Automatic Update (DT: Olivine-3-1; HV: 2.2; Time: 1/15/2020 10:23:24 AM)"=14677, "Automatic Update (DT: Olivine-3-1; HV: 2.2; Time: 1/15/2020 10:23:28 AM)"=14678, "Automatic Update (DT: Olivine-3-1; HV: 2.2; Time: 1/15/2020 10:23:29 AM)"=14679, "Automatic Update (DT: Olivine-3-1; HV: 2.2; Time: 1/15/2020 10:23:30 AM)"=14680, "Automatic Update (DT: Olivine-3-1; HV: 2.2; Time: 1/15/2020 10:23:31 AM)"=14681, "Automatic Update (DT: Olivine-3-1; HV: 2.2; Time: 1/15/2020 10:23:32 AM)"=14682, "Automatic Update (DT: Olivine-3-1; HV: 2.2; Time: 1/15/2020 10:23:33 AM)"=14683, "Automatic Update (DT: Olivine-3-1; HV: 2.2; Time: 1/15/2020 10:23:37 AM)"=14684, "Automatic Update (DT: Olivine-3-1; HV: 2.2; Time: 1/15/2020 10:23:40 AM)"=14685, "Automatic Update (DT: Olivine-3-1; HV: 2.2; Time: 1/15/2020 10:23:41 AM)"=14686, "Automatic Update (DT: Olivine-3-1; HV: 2.2; Time: 1/15/2020 10:23:42 AM)"=14687, "Automatic Update (DT: Olivine-3-1; HV: 2.2; Time: 1/15/2020 10:23:46 AM)"=14688, "Automatic Update (DT: Olivine-3-1; HV: 2.2; Time: 1/15/2020 10:23:47 AM)"=14689, "Automatic Update (DT: Olivine-3-1; HV: 2.2; Time: 1/15/2020 10:23:48 AM)"=14690, "Automatic Update (DT: Olivine-3-1; HV: 2.2; Time: 1/15/2020 10:23:49 AM)"=14691, "Automatic Update (DT: Olivine-3-1; HV: 2.2; Time: 1/15/2020 10:23:50 AM)"=14692, "Automatic Update (DT: Olivine-3-1; HV: 2.2; Time: 1/15/2020 10:23:51 AM)"=14693, "Automatic Update (DT: Olivine-3-1; HV: 2.2; Time: 1/15/2020 10:23:55 AM)"=14694, "Automatic Update (DT: Olivine-3-1; HV: 2.2; Time: 1/15/2020 10:23:56 AM)"=14695, "Automatic Update (DT: Olivine-3-1; HV: 2.2; Time: 1/15/2020 10:23:57 AM)"=14696, "Automatic Update (DT: Olivine-3-1; HV: 2.2; Time: 1/15/2020 10:23:58 AM)"=14697, "Automatic Update (DT: Olivine-3-1; HV: 2.2; Time: 1/15/2020 10:23:59 AM)"=14698, "Automatic Update (DT: Olivine-3-1; HV: 2.2; Time: 1/15/2020 10:24:00 AM)"=14699, "Automatic Update (DT: Olivine-3-1; HV: 2.2; Time: 1/15/2020 10:24:04 AM)"=14700, "Automatic Update (DT: Olivine-3-1; HV: 2.2; Time: 1/15/2020 10:24:05 AM)"=14701, "Automatic Update (DT: Olivine-3-1; HV: 2.2; Time: 1/15/2020 10:24:08 AM)"=14702, "Automatic Update (DT: Olivine-3-1; HV: 2.2; Time: 1/15/2020 10:24:09 AM)"=14703, "Automatic Update (DT: Olivine-3-1; HV: 2.2; Time: 1/15/2020 10:24:17 AM)"=14704, "Automatic Update (DT: Olivine-3-1; HV: 2.2; Time: 1/15/2020 10:24:18 AM)"=14705, "Automatic Update (DT: Olivine-3-1; HV: 2.2; Time: 1/15/2020 10:24:22 AM)"=14706, "Automatic Update (DT: Olivine-3-1; HV: 2.2; Time: 1/15/2020 10:24:23 AM)"=14707, "Automatic Update (DT: Olivine-3-1; HV: 2.2; Time: 1/15/2020 10:24:24 AM)"=14708, "Automatic Update (DT: Olivine-3-1; HV: 2.2; Time: 1/15/2020 10:24:25 AM)"=14709, "Automatic Update (DT: Olivine-3-1; HV: 2.2; Time: 1/15/2020 10:24:26 AM)"=14710, "Automatic Update (DT: Olivine-3-1; HV: 2.2; Time: 1/15/2020 10:24:27 AM)"=14711, "Automatic Update (DT: Olivine-3-1; HV: 2.2; Time: 1/15/2020 10:25:01 AM)"=14712, "Automatic Update (DT: Olivine-3-1; HV: 2.2; Time: 1/15/2020 10:25:02 AM)"=14713, "Automatic Update (DT: Olivine-3-1; HV: 2.2; Time: 1/15/2020 10:25:06 AM)"=14714, "Automatic Update (DT: Olivine-3-1; HV: 2.2; Time: 1/15/2020 10:25:08 AM)"=14715, "Automatic Update (DT: Olivine-3-1; HV: 2.2; Time: 1/15/2020 10:25:23 AM)"=14716, "Automatic Update (DT: Olivine-3-1; HV: 2.2; Time: 1/15/2020 10:25:25 AM)"=14717, "Automatic Update (DT: Olivine-3-1; HV: 2.2; Time: 1/15/2020 10:25:30 AM)"=14718, "Automatic Update (DT: Olivine-3-1; HV: 2.2; Time: 1/15/2020 10:26:51 AM)"=14719, "Automatic Update (DT: Olivine-3-1; HV: 2.2; Time: 1/15/2020 10:26:56 AM)"=14720, "Automatic Update (DT: Olivine-3-1; HV: 2.2; Time: 1/15/2020 10:29:53 AM)"=14721, "Automatic Update (DT: Olivine-3-1; HV: 2.2; Time: 1/15/2020 10:29:57 AM)"=14722, "Automatic Update (DT: Olivine-3-1; HV: 2.2; Time: 1/15/2020 10:29:58 AM)"=14723, "Automatic Update (DT: Olivine-3-1; HV: 2.2; Time: 1/15/2020 10:29:59 AM)"=14724, "Automatic Update (DT: Olivine-3-1; HV: 2.2; Time: 1/15/2020 10:30:00 AM)"=14725, "Automatic Update (DT: Olivine-3-1; HV: 2.2; Time: 1/15/2020 10:30:05 AM)"=14726, "Automatic Update (DT: Olivine-3-1; HV: 2.2; Time: 1/15/2020 10:30:06 AM)"=14727, "Automatic Update (DT: Olivine-3-1; HV: 2.2; Time: 1/15/2020 10:30:09 AM)"=14728, "Automatic Update (DT: Olivine-3-1; HV: 2.2; Time: 1/15/2020 10:30:10 AM)"=14729, "Automatic Update (DT: Olivine-3-1; HV: 2.2; Time: 1/15/2020 10:30:15 AM)"=14730, "Automatic Update (DT: Olivine-3-1; HV: 2.2; Time: 1/15/2020 10:30:23 AM)"=14731, "Automatic Update (DT: Olivine-3-1; HV: 2.2; Time: 1/15/2020 10:30:24 AM)"=14732, "Automatic Update (DT: Olivine-3-1; HV: 2.2; Time: 1/15/2020 10:30:25 AM)"=14733, "Automatic Update (DT: Olivine-3-1; HV: 2.2; Time: 1/15/2020 10:30:27 AM)"=14734, "Automatic Update (DT: Olivine-3-1; HV: 2.2; Time: 1/15/2020 10:30:28 AM)"=14735, "Automatic Update (DT: Olivine-3-1; HV: 2.2; Time: 1/15/2020 10:30:41 AM)"=14736, "Automatic Update (DT: Olivine-3-1; HV: 2.2; Time: 1/15/2020 10:30:42 AM)"=14737, "Automatic Update (DT: Olivine-3-1; HV: 2.2; Time: 1/15/2020 10:30:49 AM)"=14738, "Automatic Update (DT: Olivine-3-1; HV: 2.2; Time: 1/15/2020 10:31:03 AM)"=14739, "Automatic Update (DT: Olivine-3-1; HV: 2.2; Time: 1/15/2020 10:31:05 AM)"=14740, "Automatic Update (DT: Olivine-3-1; HV: 2.2; Time: 1/15/2020 10:31:10 AM)"=14741, "Automatic Update (DT: Olivine-3-1; HV: 2.2; Time: 1/15/2020 10:31:11 AM)"=14742, "Automatic Update (DT: Olivine-3-1; HV: 2.2; Time: 1/15/2020 10:31:12 AM)"=14743, "Automatic Update (DT: Olivine-3-1; HV: 2.2; Time: 1/15/2020 10:31:14 AM)"=14744, "Automatic Update (DT: Olivine-3-1; HV: 2.2; Time: 1/15/2020 10:31:15 AM)"=14745, "Automatic Update (DT: Olivine-3-1; HV: 2.2; Time: 1/15/2020 10:31:19 AM)"=14746, "Automatic Update (DT: Olivine-3-1; HV: 2.2; Time: 1/15/2020 10:31:20 AM)"=14747, "Automatic Update (DT: Olivine-3-1; HV: 2.2; Time: 1/15/2020 10:31:22 AM)"=14748, "Automatic Update (DT: Olivine-3-1; HV: 2.2; Time: 1/15/2020 10:31:23 AM)"=14749, "Automatic Update (DT: Olivine-3-1; HV: 2.2; Time: 1/15/2020 10:31:24 AM)"=14750, "Automatic Update (DT: Olivine-3-1; HV: 2.2; Time: 1/15/2020 10:31:29 AM)"=14751, "Automatic Update (DT: Olivine-3-1; HV: 2.2; Time: 1/15/2020 10:31:30 AM)"=14752, "Automatic Update (DT: Olivine-3-1; HV: 2.2; Time: 1/15/2020 10:31:46 AM)"=14753, "Automatic Update (DT: Olivine-3-1; HV: 2.2; Time: 1/15/2020 10:31:47 AM)"=14754, "Automatic Update (DT: Olivine-3-1; HV: 2.2; Time: 1/15/2020 10:31:48 AM)"=14755, "Automatic Update (DT: Olivine-3-1; HV: 2.2; Time: 1/15/2020 10:31:50 AM)"=14756, "Automatic Update (DT: Olivine-3-1; HV: 2.2; Time: 1/15/2020 10:32:29 AM)"=14757, "Automatic Update (DT: Olivine-3-1; HV: 2.2; Time: 1/15/2020 10:32:30 AM)"=14758, "Automatic Update (DT: Olivine-3-1; HV: 2.2; Time: 1/15/2020 10:32:34 AM)"=14759, "Automatic Update (DT: Olivine-3-1; HV: 2.2; Time: 1/15/2020 10:33:00 AM)"=14760, "Automatic Update (DT: Olivine-3-1; HV: 2.2; Time: 1/15/2020 10:33:01 AM)"=14761, "Automatic Update (DT: Olivine-3-1; HV: 2.2; Time: 1/15/2020 10:33:02 AM)"=14762, "Automatic Update (DT: Olivine-3-1; HV: 2.2; Time: 1/15/2020 10:33:03 AM)"=14763, "Automatic Update (DT: Olivine-3-1; HV: 2.2; Time: 1/15/2020 10:33:04 AM)"=14764, "Automatic Update (DT: Olivine-3-1; HV: 2.2; Time: 1/15/2020 10:33:29 AM)"=14765, "Automatic Update (DT: Olivine-3-1; HV: 2.2; Time: 1/15/2020 10:33:30 AM)"=14766, "Automatic Update (DT: Olivine-3-1; HV: 2.2; Time: 1/15/2020 10:33:31 AM)"=14767, "Automatic Update (DT: Olivine-3-1; HV: 2.2; Time: 1/15/2020 10:33:32 AM)"=14768, "Automatic Update (DT: Olivine-3-1; HV: 2.2; Time: 1/15/2020 10:33:49 AM)"=14769, "Automatic Update (DT: Olivine-3-1; HV: 2.2; Time: 1/15/2020 10:33:50 AM)"=14770, "Automatic Update (DT: Olivine-3-1; HV: 2.2; Time: 1/15/2020 10:33:51 AM)"=14771, "Automatic Update (DT: Olivine-3-1; HV: 2.2; Time: 1/15/2020 10:33:54 AM)"=14772, "Automatic Update (DT: Olivine-3-1; HV: 2.2; Time: 1/15/2020 10:33:56 AM)"=14773, "Automatic Update (DT: Olivine-3-1; HV: 2.2; Time: 1/15/2020 10:33:57 AM)"=14774, "Automatic Update (DT: Olivine-3-1; HV: 2.2; Time: 1/15/2020 10:33:59 AM)"=14775, "Automatic Update (DT: Olivine-3-1; HV: 2.2; Time: 1/15/2020 10:34:04 AM)"=14776, "Automatic Update (DT: Olivine-3-1; HV: 2.2; Time: 1/15/2020 10:34:06 AM)"=14777, "Automatic Update (DT: Olivine-3-1; HV: 2.2; Time: 1/15/2020 10:34:07 AM)"=14778, "Automatic Update (DT: Olivine-3-1; HV: 2.2; Time: 1/15/2020 10:34:08 AM)"=14779, "Automatic Update (DT: Olivine-3-1; HV: 2.2; Time: 1/15/2020 10:34:15 AM)"=14780, "Automatic Update (DT: Olivine-3-1; HV: 2.2; Time: 1/15/2020 10:34:23 AM)"=14781, "Automatic Update (DT: Olivine-3-1; HV: 2.2; Time: 1/15/2020 10:34:24 AM)"=14782, "Automatic Update (DT: Olivine-3-1; HV: 2.2; Time: 1/15/2020 10:34:25 AM)"=14783, "Automatic Update (DT: Olivine-3-1; HV: 2.2; Time: 1/15/2020 10:34:29 AM)"=14784, "Automatic Update (DT: Olivine-3-1; HV: 2.2; Time: 1/15/2020 10:34:31 AM)"=14785, "Automatic Update (DT: Olivine-3-1; HV: 2.2; Time: 1/15/2020 10:34:35 AM)"=14786, "Automatic Update (DT: Olivine-3-1; HV: 2.2; Time: 1/15/2020 10:34:36 AM)"=14787, "Automatic Update (DT: Olivine-3-1; HV: 2.2; Time: 1/15/2020 10:34:40 AM)"=14788, "Automatic Update (DT: Olivine-3-1; HV: 2.2; Time: 1/15/2020 10:34:46 AM)"=14789, "Automatic Update (DT: Olivine-3-1; HV: 2.2; Time: 1/15/2020 10:34:49 AM)"=14790, "Automatic Update (DT: Olivine-3-1; HV: 2.2; Time: 1/15/2020 10:34:50 AM)"=14791, "Automatic Update (DT: Olivine-3-1; HV: 2.2; Time: 1/15/2020 10:34:51 AM)"=14792, "Automatic Update (DT: Olivine-3-1; HV: 2.2; Time: 1/15/2020 10:34:52 AM)"=14793, "Automatic Update (DT: Olivine-3-1; HV: 2.2; Time: 1/15/2020 10:34:53 AM)"=14794, "Automatic Update (DT: Olivine-3-1; HV: 2.2; Time: 1/15/2020 10:34:54 AM)"=14795, "Automatic Update (DT: Olivine-3-1; HV: 2.2; Time: 1/15/2020 10:34:58 AM)"=14796, "Automatic Update (DT: Olivine-3-1; HV: 2.2; Time: 1/15/2020 10:34:59 AM)"=14797, "Automatic Update (DT: Olivine-3-1; HV: 2.2; Time: 1/15/2020 10:35:00 AM)"=14798, "Automatic Update (DT: Olivine-3-1; HV: 2.2; Time: 1/15/2020 10:35:01 AM)"=14799, "Automatic Update (DT: Olivine-3-1; HV: 2.2; Time: 1/15/2020 10:35:02 AM)"=14800, "Automatic Update (DT: Olivine-3-1; HV: 2.2; Time: 1/15/2020 10:35:03 AM)"=14801, "Automatic Update (DT: Olivine-3-1; HV: 2.2; Time: 1/15/2020 10:35:07 AM)"=14802, "Automatic Update (DT: Olivine-3-1; HV: 2.2; Time: 1/15/2020 10:35:08 AM)"=14803, "Automatic Update (DT: Olivine-3-1; HV: 2.2; Time: 1/15/2020 10:35:09 AM)"=14804, "Automatic Update (DT: Olivine-3-1; HV: 2.2; Time: 1/15/2020 10:35:10 AM)"=14805, "Automatic Update (DT: Olivine-3-1; HV: 2.2; Time: 1/15/2020 10:35:11 AM)"=14806, "Automatic Update (DT: Olivine-3-1; HV: 2.2; Time: 1/15/2020 10:35:12 AM)"=14807, "Automatic Update (DT: Olivine-3-1; HV: 2.2; Time: 1/15/2020 10:35:16 AM)"=14808, "Automatic Update (DT: Olivine-3-1; HV: 2.2; Time: 1/15/2020 10:35:24 AM)"=14809, "Automatic Update (DT: Olivine-3-1; HV: 2.2; Time: 1/15/2020 10:35:25 AM)"=14810, "Automatic Update (DT: Olivine-3-1; HV: 2.2; Time: 1/15/2020 10:35:26 AM)"=14811, "Automatic Update (DT: Olivine-3-1; HV: 2.2; Time: 1/15/2020 10:35:27 AM)"=14812, "Automatic Update (DT: Olivine-3-1; HV: 2.2; Time: 1/15/2020 10:35:29 AM)"=14813, "Automatic Update (DT: Olivine-3-1; HV: 2.2; Time: 1/15/2020 10:35:30 AM)"=14814, "Automatic Update (DT: Olivine-3-1; HV: 2.2; Time: 1/15/2020 10:35:34 AM)"=14815, "Automatic Update (DT: Olivine-3-1; HV: 2.2; Time: 1/15/2020 10:35:37 AM)"=14816, "Automatic Update (DT: Olivine-3-1; HV: 2.2; Time: 1/15/2020 10:35:38 AM)"=14817, "Automatic Update (DT: Olivine-3-1; HV: 2.2; Time: 1/15/2020 10:35:39 AM)"=14818, "Automatic Update (DT: Olivine-3-1; HV: 2.2; Time: 1/15/2020 10:35:44 AM)"=14819, "Automatic Update (DT: Olivine-3-1; HV: 2.2; Time: 1/15/2020 10:35:45 AM)"=14820, "Automatic Update (DT: Olivine-3-1; HV: 2.2; Time: 1/15/2020 10:35:46 AM)"=14821, "Automatic Update (DT: Olivine-3-1; HV: 2.2; Time: 1/15/2020 10:35:47 AM)"=14822, "Automatic Update (DT: Olivine-3-1; HV: 2.2; Time: 1/15/2020 10:35:48 AM)"=14823, "Automatic Update (DT: Olivine-3-1; HV: 2.2; Time: 1/15/2020 10:35:52 AM)"=14824, "Automatic Update (DT: Olivine-3-1; HV: 2.2; Time: 1/15/2020 10:35:53 AM)"=14825, "Automatic Update (DT: Olivine-3-1; HV: 2.2; Time: 1/15/2020 10:35:54 AM)"=14826, "Automatic Update (DT: Olivine-3-1; HV: 2.2; Time: 1/15/2020 10:35:55 AM)"=14827, "Automatic Update (DT: Olivine-3-1; HV: 2.2; Time: 1/15/2020 10:35:56 AM)"=14828, "Automatic Update (DT: Olivine-3-1; HV: 2.2; Time: 1/15/2020 10:35:58 AM)"=14829, "Automatic Update (DT: Olivine-3-1; HV: 2.2; Time: 1/15/2020 10:36:01 AM)"=14830, "Automatic Update (DT: Olivine-3-1; HV: 2.2; Time: 1/15/2020 10:36:02 AM)"=14831, "Automatic Update (DT: Olivine-3-1; HV: 2.2; Time: 1/15/2020 10:36:03 AM)"=14832, "Automatic Update (DT: Olivine-3-1; HV: 2.2; Time: 1/15/2020 10:36:04 AM)"=14833, "Automatic Update (DT: Olivine-3-1; HV: 2.2; Time: 1/15/2020 10:36:06 AM)"=14834, "Automatic Update (DT: Olivine-3-1; HV: 2.2; Time: 1/15/2020 10:36:10 AM)"=14835, "Automatic Update (DT: Olivine-3-1; HV: 2.2; Time: 1/15/2020 10:36:11 AM)"=14836, "Automatic Update (DT: Olivine-3-1; HV: 2.2; Time: 1/15/2020 10:36:12 AM)"=14837, "Automatic Update (DT: Olivine-3-1; HV: 2.2; Time: 1/15/2020 10:36:14 AM)"=14838, "Automatic Update (DT: Olivine-3-1; HV: 2.2; Time: 1/15/2020 10:36:15 AM)"=14839, "Automatic Update (DT: Olivine-3-1; HV: 2.2; Time: 1/15/2020 10:36:19 AM)"=14840, "Automatic Update (DT: Olivine-3-1; HV: 2.2; Time: 1/15/2020 10:36:23 AM)"=14841, "Automatic Update (DT: Olivine-3-1; HV: 2.2; Time: 1/15/2020 10:36:24 AM)"=14842, "Automatic Update (DT: Olivine-3-1; HV: 2.2; Time: 1/15/2020 10:36:29 AM)"=14843, "Automatic Update (DT: Olivine-3-1; HV: 2.2; Time: 1/15/2020 10:36:30 AM)"=14844, "Automatic Update (DT: Olivine-3-1; HV: 2.2; Time: 1/15/2020 10:36:32 AM)"=14845, "Automatic Update (DT: Olivine-3-1; HV: 2.2; Time: 1/15/2020 10:36:33 AM)"=14846, "Automatic Update (DT: Olivine-3-1; HV: 2.2; Time: 1/15/2020 10:36:34 AM)"=14847, "Automatic Update (DT: Olivine-3-1; HV: 2.2; Time: 1/15/2020 10:36:36 AM)"=14848, "Automatic Update (DT: Olivine-3-1; HV: 2.2; Time: 1/15/2020 10:36:38 AM)"=14849, "Automatic Update (DT: Olivine-3-1; HV: 2.2; Time: 1/15/2020 10:36:39 AM)"=14850, "Automatic Update (DT: Olivine-3-1; HV: 2.2; Time: 1/15/2020 10:36:40 AM)"=14851, "Automatic Update (DT: Olivine-3-1; HV: 2.2; Time: 1/15/2020 10:36:41 AM)"=14852, "Automatic Update (DT: Olivine-3-1; HV: 2.2; Time: 1/15/2020 10:36:43 AM)"=14853, "Automatic Update (DT: Olivine-3-1; HV: 2.2; Time: 1/15/2020 10:36:44 AM)"=14854, "Automatic Update (DT: Olivine-3-1; HV: 2.2; Time: 1/15/2020 10:36:47 AM)"=14855, "Automatic Update (DT: Olivine-3-1; HV: 2.2; Time: 1/15/2020 10:36:48 AM)"=14856, "Automatic Update (DT: Olivine-3-1; HV: 2.2; Time: 1/15/2020 10:36:49 AM)"=14857, "Automatic Update (DT: Olivine-3-1; HV: 2.2; Time: 1/15/2020 10:36:50 AM)"=14858, "Automatic Update (DT: Olivine-3-1; HV: 2.2; Time: 1/15/2020 10:36:51 AM)"=14859, "Automatic Update (DT: Olivine-3-1; HV: 2.2; Time: 1/15/2020 10:36:55 AM)"=14860, "Automatic Update (DT: Olivine-3-1; HV: 2.2; Time: 1/15/2020 10:36:57 AM)"=14861, "Automatic Update (DT: Olivine-3-1; HV: 2.2; Time: 1/15/2020 10:37:08 AM)"=14862, "Automatic Update (DT: Olivine-3-1; HV: 2.2; Time: 1/15/2020 10:39:08 AM)"=14863, "Automatic Update (DT: Olivine-3-1; HV: 2.2; Time: 1/15/2020 10:39:12 AM)"=14864, "Automatic Update (DT: Olivine-3-1; HV: 2.2; Time: 1/15/2020 10:39:18 AM)"=14865, "Automatic Update (DT: Olivine-3-1; HV: 2.2; Time: 1/15/2020 10:39:21 AM)"=14866, "Automatic Update (DT: Olivine-3-1; HV: 2.2; Time: 1/15/2020 10:39:32 AM)"=14867, "Automatic Update (DT: Olivine-3-1; HV: 2.2; Time: 1/15/2020 10:39:42 AM)"=14868, "Automatic Update (DT: Olivine-3-1; HV: 2.2; Time: 1/15/2020 10:39:43 AM)"=14869, "Automatic Update (DT: Olivine-3-1; HV: 2.2; Time: 1/15/2020 10:39:44 AM)"=14870, "Automatic Update (DT: Olivine-3-1; HV: 2.2; Time: 1/15/2020 10:39:48 AM)"=14871, "Automatic Update (DT: Olivine-3-1; HV: 2.2; Time: 1/15/2020 10:41:08 AM)"=14872, "Automatic Update (DT: Olivine-3-1; HV: 2.2; Time: 1/15/2020 10:41:11 AM)"=14873, "Automatic Update (DT: Olivine-3-1; HV: 2.2; Time: 1/15/2020 10:41:12 AM)"=14874, "Automatic Update (DT: Olivine-3-1; HV: 2.2; Time: 1/15/2020 10:41:15 AM)"=14875, "Automatic Update (DT: Olivine-3-1; HV: 2.2; Time: 1/15/2020 10:41:16 AM)"=14876, "Automatic Update (DT: Olivine-3-1; HV: 2.2; Time: 1/15/2020 10:41:49 AM)"=14877, "Automatic Update (DT: Olivine-3-1; HV: 2.2; Time: 1/15/2020 10:41:50 AM)"=14878, "Automatic Update (DT: Olivine-3-1; HV: 2.2; Time: 1/15/2020 10:41:51 AM)"=14879, "Automatic Update (DT: Olivine-3-1; HV: 2.2; Time: 1/15/2020 10:41:53 AM)"=14880, "Automatic Update (DT: Olivine-3-1; HV: 2.2; Time: 1/15/2020 10:41:56 AM)"=14881, "Automatic Update (DT: Olivine-3-1; HV: 2.2; Time: 1/15/2020 10:41:58 AM)"=14882, "Automatic Update (DT: Olivine-3-1; HV: 2.2; Time: 1/15/2020 10:42:00 AM)"=14883, "Automatic Update (DT: Olivine-3-1; HV: 2.2; Time: 1/15/2020 10:42:19 AM)"=14884, "Automatic Update (DT: Olivine-3-1; HV: 2.2; Time: 1/15/2020 10:42:20 AM)"=14885, "Automatic Update (DT: Olivine-3-1; HV: 2.2; Time: 1/15/2020 10:42:24 AM)"=14886, "Automatic Update (DT: Olivine-3-1; HV: 2.2; Time: 1/15/2020 10:42:34 AM)"=14887, "Automatic Update (DT: Olivine-3-1; HV: 2.2; Time: 1/15/2020 10:42:51 AM)"=14888, "Automatic Update (DT: Olivine-3-1; HV: 2.2; Time: 1/15/2020 10:42:52 AM)"=14889, "Automatic Update (DT: Olivine-3-1; HV: 2.2; Time: 1/15/2020 10:43:02 AM)"=14890, "Automatic Update (DT: Olivine-3-1; HV: 2.2; Time: 1/15/2020 10:43:10 AM)"=14891, "Automatic Update (DT: Olivine-3-1; HV: 2.2; Time: 1/15/2020 10:43:12 AM)"=14892, "Automatic Update (DT: Olivine-3-1; HV: 2.2; Time: 1/15/2020 10:43:13 AM)"=14893, "Automatic Update (DT: Olivine-3-1; HV: 2.2; Time: 1/15/2020 10:43:14 AM)"=14894, "Automatic Update (DT: Olivine-3-1; HV: 2.2; Time: 1/15/2020 10:43:18 AM)"=14895, "Automatic Update (DT: Olivine-3-1; HV: 2.2; Time: 1/15/2020 10:43:19 AM)"=14896, "Automatic Update (DT: Olivine-3-1; HV: 2.2; Time: 1/15/2020 10:43:20 AM)"=14897, "Automatic Update (DT: Olivine-3-1; HV: 2.2; Time: 1/15/2020 10:43:30 AM)"=14898, "Automatic Update (DT: Olivine-3-1; HV: 2.2; Time: 1/15/2020 10:43:31 AM)"=14899, "Automatic Update (DT: Olivine-3-1; HV: 2.2; Time: 1/15/2020 10:43:34 AM)"=14900, "Automatic Update (DT: Olivine-3-1; HV: 2.2; Time: 1/15/2020 10:43:36 AM)"=14901, "Automatic Update (DT: Olivine-3-1; HV: 2.2; Time: 1/15/2020 10:43:38 AM)"=14902, "Automatic Update (DT: Olivine-3-1; HV: 2.2; Time: 1/15/2020 10:43:41 AM)"=14903, "Automatic Update (DT: Olivine-3-1; HV: 2.2; Time: 1/15/2020 10:43:45 AM)"=14904, "Automatic Update (DT: Olivine-3-1; HV: 2.2; Time: 1/15/2020 10:43:47 AM)"=14905, "Automatic Update (DT: Olivine-3-1; HV: 2.2; Time: 1/15/2020 10:43:49 AM)"=14906, "Automatic Update (DT: Olivine-3-1; HV: 2.2; Time: 1/15/2020 10:43:51 AM)"=14907, "Automatic Update (DT: Olivine-3-1; HV: 2.2; Time: 1/15/2020 10:43:54 AM)"=14908, "Automatic Update (DT: Olivine-3-1; HV: 2.2; Time: 1/15/2020 10:43:55 AM)"=14909, "Automatic Update (DT: Olivine-3-1; HV: 2.2; Time: 1/15/2020 10:43:57 AM)"=14910, "Automatic Update (DT: Olivine-3-1; HV: 2.2; Time: 1/15/2020 10:43:59 AM)"=14911, "Automatic Update (DT: Olivine-3-1; HV: 2.2; Time: 1/15/2020 10:44:00 AM)"=14912, "Automatic Update (DT: Olivine-3-1; HV: 2.2; Time: 1/15/2020 10:44:03 AM)"=14913, "Automatic Update (DT: Olivine-3-1; HV: 2.2; Time: 1/15/2020 10:44:05 AM)"=14914, "Automatic Update (DT: Olivine-3-1; HV: 2.2; Time: 1/15/2020 10:44:06 AM)"=14915, "Automatic Update (DT: Olivine-3-1; HV: 2.2; Time: 1/15/2020 10:44:07 AM)"=14916, "Automatic Update (DT: Olivine-3-1; HV: 2.2; Time: 1/15/2020 10:44:08 AM)"=14917, "Automatic Update (DT: Olivine-3-1; HV: 2.2; Time: 1/15/2020 10:44:09 AM)"=14918, "Automatic Update (DT: Olivine-3-1; HV: 2.2; Time: 1/15/2020 10:44:13 AM)"=14919, "Automatic Update (DT: Olivine-3-1; HV: 2.2; Time: 1/15/2020 10:44:17 AM)"=14920, "Automatic Update (DT: Olivine-3-1; HV: 2.2; Time: 1/15/2020 10:44:18 AM)"=14921, "Automatic Update (DT: Olivine-3-1; HV: 2.2; Time: 1/15/2020 10:44:22 AM)"=14922, "Automatic Update (DT: Olivine-3-1; HV: 2.2; Time: 1/15/2020 10:44:23 AM)"=14923, "Automatic Update (DT: Olivine-3-1; HV: 2.2; Time: 1/15/2020 10:44:25 AM)"=14924, "Automatic Update (DT: Olivine-3-1; HV: 2.2; Time: 1/15/2020 10:44:26 AM)"=14925, "Automatic Update (DT: Olivine-3-1; HV: 2.2; Time: 1/15/2020 10:44:30 AM)"=14926, "Automatic Update (DT: Olivine-3-1; HV: 2.2; Time: 1/15/2020 10:44:31 AM)"=14927, "Automatic Update (DT: Olivine-3-1; HV: 2.2; Time: 1/15/2020 10:44:36 AM)"=14928, "Automatic Update (DT: Olivine-3-1; HV: 2.2; Time: 1/15/2020 10:45:18 AM)"=14929, "Automatic Update (DT: Olivine-3-1; HV: 2.2; Time: 1/15/2020 10:45:19 AM)"=14930, "Automatic Update (DT: Olivine-3-1; HV: 2.2; Time: 1/15/2020 10:45:20 AM)"=14931, "Automatic Update (DT: Olivine-3-1; HV: 2.2; Time: 1/15/2020 10:45:22 AM)"=14932, "Automatic Update (DT: Olivine-3-1; HV: 2.2; Time: 1/15/2020 10:45:25 AM)"=14933, "Automatic Update (DT: Olivine-3-1; HV: 2.2; Time: 1/15/2020 10:45:26 AM)"=14934, "Automatic Update (DT: Olivine-3-1; HV: 2.2; Time: 1/15/2020 10:45:29 AM)"=14935, "Automatic Update (DT: Olivine-3-1; HV: 2.2; Time: 1/15/2020 10:45:30 AM)"=14936, "Automatic Update (DT: Olivine-3-1; HV: 2.2; Time: 1/15/2020 10:45:34 AM)"=14937, "Automatic Update (DT: Olivine-3-1; HV: 2.2; Time: 1/15/2020 10:45:40 AM)"=14938, "Automatic Update (DT: Olivine-3-1; HV: 2.2; Time: 1/15/2020 10:45:43 AM)"=14939, "Automatic Update (DT: Olivine-3-1; HV: 2.2; Time: 1/15/2020 10:45:44 AM)"=14940, "Automatic Update (DT: Olivine-3-1; HV: 2.2; Time: 1/15/2020 10:45:48 AM)"=14941, "Automatic Update (DT: Olivine-3-1; HV: 2.2; Time: 1/15/2020 10:45:52 AM)"=14942, "Automatic Update (DT: Olivine-3-1; HV: 2.2; Time: 1/15/2020 10:45:57 AM)"=14943, "Automatic Update (DT: Olivine-3-1; HV: 2.2; Time: 1/15/2020 10:46:01 AM)"=14944, "Automatic Update (DT: Olivine-3-1; HV: 2.2; Time: 1/15/2020 10:46:03 AM)"=14945, "Automatic Update (DT: Olivine-3-1; HV: 2.2; Time: 1/15/2020 10:46:04 AM)"=14946, "Automatic Update (DT: Olivine-3-1; HV: 2.2; Time: 1/15/2020 10:46:06 AM)"=14947, "Automatic Update (DT: Olivine-3-1; HV: 2.2; Time: 1/15/2020 10:46:10 AM)"=14948, "Automatic Update (DT: Olivine-3-1; HV: 2.2; Time: 1/15/2020 10:46:12 AM)"=14949, "Automatic Update (DT: Olivine-3-1; HV: 2.2; Time: 1/15/2020 10:46:13 AM)"=14950, "Automatic Update (DT: Olivine-3-1; HV: 2.2; Time: 1/15/2020 10:46:16 AM)"=14951, "Automatic Update (DT: Olivine-3-1; HV: 2.2; Time: 1/15/2020 10:47:10 AM)"=14952, "Automatic Update (DT: Olivine-3-1; HV: 2.2; Time: 1/15/2020 10:47:13 AM)"=14953, "Automatic Update (DT: Olivine-3-1; HV: 2.2; Time: 1/15/2020 10:47:15 AM)"=14954, "Automatic Update (DT: Olivine-3-1; HV: 2.2; Time: 1/15/2020 10:48:31 AM)"=14955, "Automatic Update (DT: Olivine-3-1; HV: 2.2; Time: 1/15/2020 10:48:32 AM)"=14956, "Automatic Update (DT: Olivine-3-1; HV: 2.2; Time: 1/15/2020 10:48:38 AM)"=14957, "Automatic Update (DT: Olivine-3-1; HV: 2.2; Time: 1/15/2020 10:48:39 AM)"=14958, "Automatic Update (DT: Olivine-3-1; HV: 2.2; Time: 1/15/2020 10:48:48 AM)"=14959, "Automatic Update (DT: Olivine-3-1; HV: 2.2; Time: 1/15/2020 10:48:49 AM)"=14960, "Automatic Update (DT: Olivine-3-1; HV: 2.2; Time: 1/15/2020 10:48:50 AM)"=14961, "Automatic Update (DT: Olivine-3-1; HV: 2.2; Time: 1/15/2020 10:48:58 AM)"=14962, "Automatic Update (DT: Olivine-3-1; HV: 2.2; Time: 1/15/2020 10:48:59 AM)"=14963, "Automatic Update (DT: Olivine-3-1; HV: 2.2; Time: 1/15/2020 10:49:03 AM)"=14964, "Automatic Update (DT: Olivine-3-1; HV: 2.2; Time: 1/15/2020 10:49:06 AM)"=14965, "Automatic Update (DT: Olivine-3-1; HV: 2.2; Time: 1/15/2020 10:49:07 AM)"=14966, "Automatic Update (DT: Olivine-3-1; HV: 2.2; Time: 1/15/2020 10:49:09 AM)"=14967, "Automatic Update (DT: Olivine-3-1; HV: 2.2; Time: 1/15/2020 10:49:13 AM)"=14968, "Automatic Update (DT: Olivine-3-1; HV: 2.2; Time: 1/15/2020 10:49:14 AM)"=14969, "Automatic Update (DT: Olivine-3-1; HV: 2.2; Time: 1/15/2020 10:49:15 AM)"=14970, "Automatic Update (DT: Olivine-3-1; HV: 2.2; Time: 1/15/2020 10:49:16 AM)"=14971, "Automatic Update (DT: Olivine-3-1; HV: 2.2; Time: 1/15/2020 10:49:19 AM)"=14972, "Automatic Update (DT: Olivine-3-1; HV: 2.2; Time: 1/15/2020 10:49:21 AM)"=14973, "Automatic Update (DT: Olivine-3-1; HV: 2.2; Time: 1/15/2020 10:49:22 AM)"=14974, "Automatic Update (DT: Olivine-3-1; HV: 2.2; Time: 1/15/2020 10:49:23 AM)"=14975, "Automatic Update (DT: Olivine-3-1; HV: 2.2; Time: 1/15/2020 10:49:24 AM)"=14976, "Automatic Update (DT: Olivine-3-1; HV: 2.2; Time: 1/15/2020 10:49:29 AM)"=14977, "Automatic Update (DT: Olivine-3-1; HV: 2.2; Time: 1/15/2020 10:49:30 AM)"=14978, "Automatic Update (DT: Olivine-3-1; HV: 2.2; Time: 1/15/2020 10:49:31 AM)"=14979, "Automatic Update (DT: Olivine-3-1; HV: 2.2; Time: 1/15/2020 10:49:33 AM)"=14980, "Automatic Update (DT: Olivine-3-1; HV: 2.2; Time: 1/15/2020 10:49:34 AM)"=14981, "Automatic Update (DT: Olivine-3-1; HV: 2.2; Time: 1/15/2020 10:49:39 AM)"=14982, "Automatic Update (DT: Olivine-3-1; HV: 2.2; Time: 1/15/2020 10:49:42 AM)"=14983, "Automatic Update (DT: Olivine-3-1; HV: 2.2; Time: 1/15/2020 10:49:43 AM)"=14984, "Automatic Update (DT: Olivine-3-1; HV: 2.2; Time: 1/15/2020 10:49:44 AM)"=14985, "Automatic Update (DT: Olivine-3-1; HV: 2.2; Time: 1/15/2020 10:49:48 AM)"=14986, "Automatic Update (DT: Olivine-3-1; HV: 2.2; Time: 1/15/2020 10:49:51 AM)"=14987, "Automatic Update (DT: Olivine-3-1; HV: 2.2; Time: 1/15/2020 10:49:53 AM)"=14988, "Automatic Update (DT: Olivine-3-1; HV: 2.2; Time: 1/15/2020 10:49:57 AM)"=14989, "Automatic Update (DT: Olivine-3-1; HV: 2.2; Time: 1/15/2020 10:49:58 AM)"=14990, "Automatic Update (DT: Olivine-3-1; HV: 2.2; Time: 1/15/2020 10:49:59 AM)"=14991, "Automatic Update (DT: Olivine-3-1; HV: 2.2; Time: 1/15/2020 10:50:03 AM)"=14992, "Automatic Update (DT: Olivine-3-1; HV: 2.2; Time: 1/15/2020 10:50:08 AM)"=14993, "Automatic Update (DT: Olivine-3-1; HV: 2.2; Time: 1/15/2020 10:50:09 AM)"=14994, "Automatic Update (DT: Olivine-3-1; HV: 2.2; Time: 1/15/2020 10:50:10 AM)"=14995, "Automatic Update (DT: Olivine-3-1; HV: 2.2; Time: 1/15/2020 10:50:11 AM)"=14996, "Automatic Update (DT: Olivine-3-1; HV: 2.2; Time: 1/15/2020 10:50:18 AM)"=14997, "Automatic Update (DT: Olivine-3-1; HV: 2.2; Time: 1/15/2020 10:50:19 AM)"=14998, "Automatic Update (DT: Olivine-3-1; HV: 2.2; Time: 1/15/2020 10:50:20 AM)"=14999, "Automatic Update (DT: Olivine-3-1; HV: 2.2; Time: 1/15/2020 10:50:24 AM)"=15000, "Automatic Update (DT: Olivine-3-1; HV: 2.2; Time: 1/15/2020 10:50:40 AM)"=15001, "Automatic Update (DT: Olivine-3-1; HV: 2.2; Time: 1/15/2020 10:50:42 AM)"=15002, "Automatic Update (DT: Olivine-3-1; HV: 2.2; Time: 1/15/2020 10:53:39 AM)"=15003, "Automatic Update (DT: Olivine-3-1; HV: 2.2; Time: 1/15/2020 10:53:40 AM)"=15004, "Automatic Update (DT: Olivine-3-1; HV: 2.2; Time: 1/15/2020 10:55:10 AM)"=15005, "Automatic Update (DT: Olivine-3-1; HV: 2.2; Time: 1/15/2020 10:55:11 AM)"=15006, "Automatic Update (DT: Olivine-3-1; HV: 2.2; Time: 1/15/2020 10:55:16 AM)"=15007, "Automatic Update (DT: Olivine-3-1; HV: 2.2; Time: 1/15/2020 10:55:17 AM)"=15008, "Automatic Update (DT: Olivine-3-1; HV: 2.2; Time: 1/15/2020 10:55:18 AM)"=15009, "Automatic Update (DT: Olivine-3-1; HV: 2.2; Time: 1/15/2020 10:55:19 AM)"=15010, "Automatic Update (DT: Olivine-3-1; HV: 2.2; Time: 1/15/2020 10:55:20 AM)"=15011, "Automatic Update (DT: Olivine-3-1; HV: 2.2; Time: 1/15/2020 10:55:21 AM)"=15012, "Automatic Update (DT: Olivine-3-1; HV: 2.2; Time: 1/15/2020 10:55:25 AM)"=15013, "Automatic Update (DT: Olivine-3-1; HV: 2.2; Time: 1/15/2020 10:55:26 AM)"=15014, "Automatic Update (DT: Olivine-3-1; HV: 2.2; Time: 1/15/2020 10:55:27 AM)"=15015, "Automatic Update (DT: Olivine-3-1; HV: 2.2; Time: 1/15/2020 10:55:28 AM)"=15016, "Automatic Update (DT: Olivine-3-1; HV: 2.2; Time: 1/15/2020 10:55:29 AM)"=15017, "Automatic Update (DT: Olivine-3-1; HV: 2.2; Time: 1/15/2020 10:55:30 AM)"=15018, "Automatic Update (DT: Olivine-3-1; HV: 2.2; Time: 1/15/2020 10:55:34 AM)"=15019, "Automatic Update (DT: Olivine-3-1; HV: 2.2; Time: 1/15/2020 10:55:35 AM)"=15020, "Automatic Update (DT: Olivine-3-1; HV: 2.2; Time: 1/15/2020 10:55:52 AM)"=15021, "Automatic Update (DT: Olivine-3-1; HV: 2.2; Time: 1/15/2020 10:56:09 AM)"=15022, "Automatic Update (DT: Olivine-3-1; HV: 2.2; Time: 1/15/2020 10:56:10 AM)"=15023, "Automatic Update (DT: Olivine-3-1; HV: 2.2; Time: 1/15/2020 10:57:08 AM)"=15024, "Automatic Update (DT: Olivine-3-1; HV: 2.2; Time: 1/15/2020 10:57:11 AM)"=15025, "Automatic Update (DT: Olivine-3-1; HV: 2.2; Time: 1/15/2020 10:57:13 AM)"=15026, "Automatic Update (DT: Olivine-3-1; HV: 2.2; Time: 1/15/2020 11:14:00 AM)"=15027, "Automatic Update (DT: Olivine-3-1; HV: 2.2; Time: 1/15/2020 11:14:03 AM)"=15028, "Automatic Update (DT: Olivine-3-1; HV: 2.2; Time: 1/15/2020 11:14:14 AM)"=15029, "Automatic Update (DT: Olivine-3-1; HV: 2.2; Time: 1/15/2020 11:14:21 AM)"=15030, "Automatic Update (DT: Olivine-3-1; HV: 2.2; Time: 1/15/2020 11:33:21 AM)"=15031, "Automatic Update (DT: Olivine-3-1; HV: 2.2; Time: 1/15/2020 11:33:22 AM)"=15032, "Automatic Update (DT: Olivine-3-1; HV: 2.2; Time: 1/15/2020 11:33:24 AM)"=15033, "Automatic Update (DT: Olivine-3-1; HV: 2.2; Time: 1/15/2020 11:33:28 AM)"=15034, "Automatic Update (DT: Olivine-3-1; HV: 2.2; Time: 1/15/2020 11:33:29 AM)"=15035, "Automatic Update (DT: Olivine-3-1; HV: 2.2; Time: 1/15/2020 11:35:34 AM)"=15036, "Automatic Update (DT: Olivine-3-1; HV: 2.2; Time: 1/15/2020 11:35:49 AM)"=15037, "Automatic Update (DT: Olivine-3-1; HV: 2.2; Time: 1/15/2020 11:35:53 AM)"=15038, "Automatic Update (DT: Olivine-3-1; HV: 2.2; Time: 1/15/2020 11:36:02 AM)"=15039, "Automatic Update (DT: Olivine-3-1; HV: 2.2; Time: 1/15/2020 11:36:05 AM)"=15040, "Automatic Update (DT: Olivine-3-1; HV: 2.2; Time: 1/15/2020 11:36:10 AM)"=15041, "Automatic Update (DT: Olivine-3-1; HV: 2.2; Time: 1/15/2020 11:36:15 AM)"=15042, "Automatic Update (DT: Olivine-3-1; HV: 2.2; Time: 1/15/2020 11:36:23 AM)"=15043, "Automatic Update (DT: Olivine-3-1; HV: 2.2; Time: 1/15/2020 11:36:25 AM)"=15044, "Automatic Update (DT: Olivine-3-1; HV: 2.2; Time: 1/15/2020 11:36:41 AM)"=15045, "Automatic Update (DT: Olivine-3-1; HV: 2.2; Time: 1/15/2020 11:37:06 AM)"=15046, "Automatic Update (DT: Olivine-3-1; HV: 2.2; Time: 1/15/2020 11:37:11 AM)"=15047, "Automatic Update (DT: Olivine-3-1; HV: 2.2; Time: 1/15/2020 11:37:20 AM)"=15048, "Automatic Update (DT: Olivine-3-1; HV: 2.2; Time: 1/15/2020 11:37:21 AM)"=15049, "Automatic Update (DT: Olivine-3-1; HV: 2.2; Time: 1/15/2020 11:37:33 AM)"=15050, "Automatic Update (DT: Olivine-3-1; HV: 2.2; Time: 1/15/2020 11:37:39 AM)"=15051, "Automatic Update (DT: Olivine-3-1; HV: 2.2; Time: 1/15/2020 11:37:41 AM)"=15052, "Automatic Update (DT: Olivine-3-1; HV: 2.2; Time: 1/15/2020 11:37:43 AM)"=15053, "Automatic Update (DT: Olivine-3-1; HV: 2.2; Time: 1/15/2020 11:37:44 AM)"=15054, "Automatic Update (DT: Olivine-3-1; HV: 2.2; Time: 1/15/2020 11:37:49 AM)"=15055, "Automatic Update (DT: Olivine-3-1; HV: 2.2; Time: 1/15/2020 11:37:50 AM)"=15056, "Automatic Update (DT: Olivine-3-1; HV: 2.2; Time: 1/15/2020 11:37:52 AM)"=15057, "Automatic Update (DT: Olivine-3-1; HV: 2.2; Time: 1/15/2020 11:37:53 AM)"=15058, "Automatic Update (DT: Olivine-3-1; HV: 2.2; Time: 1/15/2020 11:37:54 AM)"=15059, "Automatic Update (DT: Olivine-3-1; HV: 2.2; Time: 1/15/2020 11:37:59 AM)"=15060, "Automatic Update (DT: Olivine-3-1; HV: 2.2; Time: 1/15/2020 11:38:05 AM)"=15061, "Automatic Update (DT: Olivine-3-1; HV: 2.2; Time: 1/15/2020 11:38:09 AM)"=15062, "Automatic Update (DT: Olivine-3-1; HV: 2.2; Time: 1/15/2020 11:38:10 AM)"=15063, "Automatic Update (DT: Olivine-3-1; HV: 2.2; Time: 1/15/2020 11:38:11 AM)"=15064, "Automatic Update (DT: Olivine-3-1; HV: 2.2; Time: 1/15/2020 11:38:12 AM)"=15065, "Automatic Update (DT: Olivine-3-1; HV: 2.2; Time: 1/15/2020 11:38:13 AM)"=15066, "Automatic Update (DT: Olivine-3-1; HV: 2.2; Time: 1/15/2020 11:38:14 AM)"=15067, "Automatic Update (DT: Olivine-3-1; HV: 2.2; Time: 1/15/2020 11:38:18 AM)"=15068, "Automatic Update (DT: Olivine-3-1; HV: 2.2; Time: 1/15/2020 11:38:22 AM)"=15069, "Automatic Update (DT: Olivine-3-1; HV: 2.2; Time: 1/15/2020 11:38:23 AM)"=15070, "Automatic Update (DT: Olivine-3-1; HV: 2.2; Time: 1/15/2020 11:38:24 AM)"=15071, "Automatic Update (DT: Olivine-3-1; HV: 2.2; Time: 1/15/2020 11:38:28 AM)"=15072, "Automatic Update (DT: Olivine-3-1; HV: 2.2; Time: 1/15/2020 11:38:29 AM)"=15073, "Automatic Update (DT: Olivine-3-1; HV: 2.2; Time: 1/15/2020 11:38:31 AM)"=15074, "Automatic Update (DT: Olivine-3-1; HV: 2.2; Time: 1/15/2020 11:38:32 AM)"=15075, "Automatic Update (DT: Olivine-3-1; HV: 2.2; Time: 1/15/2020 11:38:33 AM)"=15076, "Automatic Update (DT: Olivine-3-1; HV: 2.2; Time: 1/15/2020 11:38:34 AM)"=15077, "Automatic Update (DT: Olivine-3-1; HV: 2.2; Time: 1/15/2020 11:38:39 AM)"=15078, "Automatic Update (DT: Olivine-3-1; HV: 2.2; Time: 1/15/2020 11:38:40 AM)"=15079, "Automatic Update (DT: Olivine-3-1; HV: 2.2; Time: 1/15/2020 11:38:41 AM)"=15080, "Automatic Update (DT: Olivine-3-1; HV: 2.2; Time: 1/15/2020 11:38:42 AM)"=15081, "Automatic Update (DT: Olivine-3-1; HV: 2.2; Time: 1/15/2020 11:38:43 AM)"=15082, "Automatic Update (DT: Olivine-3-1; HV: 2.2; Time: 1/15/2020 11:38:45 AM)"=15083, "Automatic Update (DT: Olivine-3-1; HV: 2.2; Time: 1/15/2020 11:38:49 AM)"=15084, "Automatic Update (DT: Olivine-3-1; HV: 2.2; Time: 1/15/2020 11:38:50 AM)"=15085, "Automatic Update (DT: Olivine-3-1; HV: 2.2; Time: 1/15/2020 11:38:51 AM)"=15086, "Automatic Update (DT: Olivine-3-1; HV: 2.2; Time: 1/15/2020 11:38:52 AM)"=15087, "Automatic Update (DT: Olivine-3-1; HV: 2.2; Time: 1/15/2020 11:38:53 AM)"=15088, "Automatic Update (DT: Olivine-3-1; HV: 2.2; Time: 1/15/2020 11:38:54 AM)"=15089, "Automatic Update (DT: Olivine-3-1; HV: 2.2; Time: 1/15/2020 11:38:59 AM)"=15090, "Automatic Update (DT: Olivine-3-1; HV: 2.2; Time: 1/15/2020 11:39:01 AM)"=15091, "Automatic Update (DT: Olivine-3-1; HV: 2.2; Time: 1/15/2020 11:39:04 AM)"=15092, "Automatic Update (DT: Olivine-3-1; HV: 2.2; Time: 1/15/2020 11:39:09 AM)"=15093, "Automatic Update (DT: Olivine-3-1; HV: 2.2; Time: 1/15/2020 11:39:13 AM)"=15094, "Automatic Update (DT: Olivine-3-1; HV: 2.2; Time: 1/15/2020 11:39:14 AM)"=15095, "Automatic Update (DT: Olivine-3-1; HV: 2.2; Time: 1/15/2020 11:39:20 AM)"=15096, "Automatic Update (DT: Olivine-3-1; HV: 2.2; Time: 1/15/2020 11:39:29 AM)"=15097, "Automatic Update (DT: Olivine-3-1; HV: 2.2; Time: 1/15/2020 11:39:30 AM)"=15098, "Automatic Update (DT: Olivine-3-1; HV: 2.2; Time: 1/15/2020 11:39:31 AM)"=15099, "Automatic Update (DT: Olivine-3-1; HV: 2.2; Time: 1/15/2020 11:39:32 AM)"=15100, "Automatic Update (DT: Olivine-3-1; HV: 2.2; Time: 1/15/2020 11:39:43 AM)"=15101, "Automatic Update (DT: Olivine-3-1; HV: 2.2; Time: 1/15/2020 11:39:45 AM)"=15102, "Automatic Update (DT: Olivine-3-1; HV: 2.2; Time: 1/15/2020 11:39:49 AM)"=15103, "Automatic Update (DT: Olivine-3-1; HV: 2.2; Time: 1/15/2020 11:39:53 AM)"=15104, "Automatic Update (DT: Olivine-3-1; HV: 2.2; Time: 1/15/2020 11:39:54 AM)"=15105, "Automatic Update (DT: Olivine-3-1; HV: 2.2; Time: 1/15/2020 11:39:59 AM)"=15106, "Automatic Update (DT: Olivine-3-1; HV: 2.2; Time: 1/15/2020 11:40:01 AM)"=15107, "Automatic Update (DT: Olivine-3-1; HV: 2.2; Time: 1/15/2020 11:40:02 AM)"=15108, "Automatic Update (DT: Olivine-3-1; HV: 2.2; Time: 1/15/2020 11:40:03 AM)"=15109, "Automatic Update (DT: Olivine-3-1; HV: 2.2; Time: 1/15/2020 11:40:04 AM)"=15110, "Automatic Update (DT: Olivine-3-1; HV: 2.2; Time: 1/15/2020 11:40:05 AM)"=15111, "Automatic Update (DT: Olivine-3-1; HV: 2.2; Time: 1/15/2020 11:40:09 AM)"=15112, "Automatic Update (DT: Olivine-3-1; HV: 2.2; Time: 1/15/2020 11:40:10 AM)"=15113, "Automatic Update (DT: Olivine-3-1; HV: 2.2; Time: 1/15/2020 11:40:11 AM)"=15114, "Automatic Update (DT: Olivine-3-1; HV: 2.2; Time: 1/15/2020 11:40:12 AM)"=15115, "Automatic Update (DT: Olivine-3-1; HV: 2.2; Time: 1/15/2020 11:40:13 AM)"=15116, "Automatic Update (DT: Olivine-3-1; HV: 2.2; Time: 1/15/2020 11:40:16 AM)"=15117, "Automatic Update (DT: Olivine-3-1; HV: 2.2; Time: 1/15/2020 11:40:19 AM)"=15118, "Automatic Update (DT: Olivine-3-1; HV: 2.2; Time: 1/15/2020 11:40:21 AM)"=15119, "Automatic Update (DT: Olivine-3-1; HV: 2.2; Time: 1/15/2020 11:40:39 AM)"=15120, "Automatic Update (DT: Olivine-3-1; HV: 2.2; Time: 1/15/2020 12:08:34 PM)"=15121, "Automatic Update (DT: Olivine-3-1; HV: 2.2; Time: 1/15/2020 12:08:37 PM)"=15122, "Automatic Update (DT: Olivine-3-1; HV: 2.2; Time: 1/15/2020 12:08:38 PM)"=15123, "Automatic Update (DT: Olivine-3-1; HV: 2.2; Time: 1/15/2020 12:08:42 PM)"=15124, "Automatic Update (DT: Olivine-3-1; HV: 2.2; Time: 1/15/2020 12:12:50 PM)"=15125, "Automatic Update (DT: Olivine-3-1; HV: 2.2; Time: 1/15/2020 12:12:54 PM)"=15126, "Automatic Update (DT: Olivine-3-1; HV: 2.2; Time: 1/15/2020 12:13:02 PM)"=15127, "Automatic Update (DT: Olivine-3-1; HV: 2.2; Time: 1/15/2020 12:13:08 PM)"=15128, "Automatic Update (DT: Olivine-3-1; HV: 2.2; Time: 1/15/2020 12:13:13 PM)"=15129, "Automatic Update (DT: Olivine-3-1; HV: 2.2; Time: 1/15/2020 12:13:15 PM)"=15130, "Automatic Update (DT: Olivine-3-1; HV: 2.2; Time: 1/15/2020 12:13:16 PM)"=15131, "Automatic Update (DT: Olivine-3-1; HV: 2.2; Time: 1/15/2020 12:13:18 PM)"=15132, "Automatic Update (DT: Olivine-3-1; HV: 2.2; Time: 1/15/2020 12:13:21 PM)"=15133, "Automatic Update (DT: Olivine-3-1; HV: 2.2; Time: 1/15/2020 12:13:22 PM)"=15134, "Automatic Update (DT: Olivine-3-1; HV: 2.2; Time: 1/15/2020 12:13:23 PM)"=15135, "Automatic Update (DT: Olivine-3-1; HV: 2.2; Time: 1/15/2020 12:13:25 PM)"=15136, "Automatic Update (DT: Olivine-3-1; HV: 2.2; Time: 1/15/2020 12:13:27 PM)"=15137, "Automatic Update (DT: Olivine-3-1; HV: 2.2; Time: 1/15/2020 12:13:31 PM)"=15138, "Automatic Update (DT: Olivine-3-1; HV: 2.2; Time: 1/15/2020 12:13:48 PM)"=15139, "Automatic Update (DT: Olivine-3-1; HV: 2.2; Time: 1/15/2020 12:13:50 PM)"=15140, "Automatic Update (DT: Olivine-3-1; HV: 2.2; Time: 1/15/2020 12:13:51 PM)"=15141, "Automatic Update (DT: Olivine-3-1; HV: 2.2; Time: 1/15/2020 12:13:52 PM)"=15142, "Automatic Update (DT: Olivine-3-1; HV: 2.2; Time: 1/15/2020 12:13:53 PM)"=15143, "Automatic Update (DT: Olivine-3-1; HV: 2.2; Time: 1/15/2020 12:13:54 PM)"=15144, "Automatic Update (DT: Olivine-3-1; HV: 2.2; Time: 1/15/2020 12:13:55 PM)"=15145, "Automatic Update (DT: Olivine-3-1; HV: 2.2; Time: 1/15/2020 12:13:59 PM)"=15146, "Automatic Update (DT: Olivine-3-1; HV: 2.2; Time: 1/15/2020 12:14:00 PM)"=15147, "Automatic Update (DT: Olivine-3-1; HV: 2.2; Time: 1/15/2020 12:14:01 PM)"=15148, "Automatic Update (DT: Olivine-3-1; HV: 2.2; Time: 1/15/2020 12:14:02 PM)"=15149, "Automatic Update (DT: Olivine-3-1; HV: 2.2; Time: 1/15/2020 12:14:03 PM)"=15150, "Automatic Update (DT: Olivine-3-1; HV: 2.2; Time: 1/15/2020 12:14:04 PM)"=15151, "Automatic Update (DT: Olivine-3-1; HV: 2.2; Time: 1/15/2020 12:14:09 PM)"=15152, "Automatic Update (DT: Olivine-3-1; HV: 2.2; Time: 1/15/2020 12:14:10 PM)"=15153, "Automatic Update (DT: Olivine-3-1; HV: 2.2; Time: 1/15/2020 12:14:11 PM)"=15154, "Automatic Update (DT: Olivine-3-1; HV: 2.2; Time: 1/15/2020 12:14:12 PM)"=15155, "Automatic Update (DT: Olivine-3-1; HV: 2.2; Time: 1/15/2020 12:14:13 PM)"=15156, "Automatic Update (DT: Olivine-3-1; HV: 2.2; Time: 1/15/2020 12:14:14 PM)"=15157, "Automatic Update (DT: Olivine-3-1; HV: 2.2; Time: 1/15/2020 12:14:18 PM)"=15158, "Automatic Update (DT: Olivine-3-1; HV: 2.2; Time: 1/15/2020 12:14:19 PM)"=15159, "Automatic Update (DT: Olivine-3-1; HV: 2.2; Time: 1/15/2020 12:14:20 PM)"=15160, "Automatic Update (DT: Olivine-3-1; HV: 2.2; Time: 1/15/2020 12:14:21 PM)"=15161, "Automatic Update (DT: Olivine-3-1; HV: 2.2; Time: 1/15/2020 12:14:22 PM)"=15162, "Automatic Update (DT: Olivine-3-1; HV: 2.2; Time: 1/15/2020 12:14:28 PM)"=15163, "Automatic Update (DT: Olivine-3-1; HV: 2.2; Time: 1/15/2020 12:14:29 PM)"=15164, "Automatic Update (DT: Olivine-3-1; HV: 2.2; Time: 1/15/2020 12:14:30 PM)"=15165, "Automatic Update (DT: Olivine-3-1; HV: 2.2; Time: 1/15/2020 12:14:32 PM)"=15166, "Automatic Update (DT: Olivine-3-1; HV: 2.2; Time: 1/15/2020 12:14:37 PM)"=15167, "Automatic Update (DT: Olivine-3-1; HV: 2.2; Time: 1/15/2020 12:16:34 PM)"=15168, "Automatic Update (DT: Olivine-3-1; HV: 2.2; Time: 1/15/2020 12:16:35 PM)"=15169, "Automatic Update (DT: Olivine-3-1; HV: 2.2; Time: 1/15/2020 12:16:38 PM)"=15170, "Automatic Update (DT: Olivine-3-1; HV: 2.2; Time: 1/15/2020 12:16:41 PM)"=15171, "Automatic Update (DT: Olivine-3-1; HV: 2.2; Time: 1/15/2020 12:16:42 PM)"=15172, "Automatic Update (DT: Olivine-3-1; HV: 2.2; Time: 1/15/2020 12:17:21 PM)"=15173, "Automatic Update (DT: Olivine-3-1; HV: 2.2; Time: 1/15/2020 12:17:23 PM)"=15174, "Automatic Update (DT: Olivine-3-1; HV: 2.2; Time: 1/15/2020 12:17:24 PM)"=15175, "Automatic Update (DT: Olivine-3-1; HV: 2.2; Time: 1/15/2020 12:17:25 PM)"=15176, "Automatic Update (DT: Olivine-3-1; HV: 2.2; Time: 1/15/2020 12:17:35 PM)"=15177, "Automatic Update (DT: Olivine-3-1; HV: 2.2; Time: 1/15/2020 12:17:39 PM)"=15178, "Automatic Update (DT: Olivine-3-1; HV: 2.2; Time: 1/15/2020 12:17:55 PM)"=15179, "Automatic Update (DT: Olivine-3-1; HV: 2.2; Time: 1/15/2020 12:17:58 PM)"=15180, "Automatic Update (DT: Olivine-3-1; HV: 2.2; Time: 1/15/2020 12:18:00 PM)"=15181, "Automatic Update (DT: Olivine-3-1; HV: 2.2; Time: 1/15/2020 12:18:01 PM)"=15182, "Automatic Update (DT: Olivine-3-1; HV: 2.2; Time: 1/15/2020 12:18:03 PM)"=15183, "Automatic Update (DT: Olivine-3-1; HV: 2.2; Time: 1/15/2020 12:18:07 PM)"=15184, "Automatic Update (DT: Olivine-3-1; HV: 2.2; Time: 1/15/2020 12:18:17 PM)"=15185, "Automatic Update (DT: Olivine-3-1; HV: 2.2; Time: 1/15/2020 12:18:18 PM)"=15186, "Automatic Update (DT: Olivine-3-1; HV: 2.2; Time: 1/15/2020 12:22:00 PM)"=15187, "Automatic Update (DT: Olivine-3-1; HV: 2.2; Time: 1/15/2020 12:22:01 PM)"=15188, "Automatic Update (DT: Olivine-3-1; HV: 2.2; Time: 1/15/2020 12:22:02 PM)"=15189, "Automatic Update (DT: Olivine-3-1; HV: 2.2; Time: 1/15/2020 12:22:06 PM)"=15190, "Automatic Update (DT: Olivine-3-1; HV: 2.2; Time: 1/15/2020 12:22:07 PM)"=15191, "Automatic Update (DT: Olivine-3-1; HV: 2.2; Time: 1/15/2020 12:22:09 PM)"=15192, "Automatic Update (DT: Olivine-3-1; HV: 2.2; Time: 1/15/2020 12:22:10 PM)"=15193, "Automatic Update (DT: Olivine-3-1; HV: 2.2; Time: 1/15/2020 12:22:13 PM)"=15194, "Automatic Update (DT: Olivine-3-1; HV: 2.2; Time: 1/15/2020 12:22:16 PM)"=15195, "Automatic Update (DT: Olivine-3-1; HV: 2.2; Time: 1/15/2020 12:22:17 PM)"=15196, "Automatic Update (DT: Olivine-3-1; HV: 2.2; Time: 1/15/2020 12:22:18 PM)"=15197, "Automatic Update (DT: Olivine-3-1; HV: 2.2; Time: 1/15/2020 12:22:19 PM)"=15198, "Automatic Update (DT: Olivine-3-1; HV: 2.2; Time: 1/15/2020 12:22:21 PM)"=15199, "Automatic Update (DT: Olivine-3-1; HV: 2.2; Time: 1/15/2020 12:22:22 PM)"=15200, "Automatic Update (DT: Olivine-3-1; HV: 2.2; Time: 1/15/2020 12:22:26 PM)"=15201, "Automatic Update (DT: Olivine-3-1; HV: 2.2; Time: 1/15/2020 12:22:32 PM)"=15202, "Automatic Update (DT: Olivine-3-1; HV: 2.2; Time: 1/15/2020 12:22:35 PM)"=15203, "Automatic Update (DT: Olivine-3-1; HV: 2.2; Time: 1/15/2020 12:22:37 PM)"=15204, "Automatic Update (DT: Olivine-3-1; HV: 2.2; Time: 1/15/2020 12:22:38 PM)"=15205, "Automatic Update (DT: Olivine-3-1; HV: 2.2; Time: 1/15/2020 12:22:41 PM)"=15206, "Automatic Update (DT: Olivine-3-1; HV: 2.2; Time: 1/15/2020 12:22:45 PM)"=15207, "Automatic Update (DT: Olivine-3-1; HV: 2.2; Time: 1/15/2020 12:22:59 PM)"=15208, "Automatic Update (DT: Olivine-3-1; HV: 2.2; Time: 1/15/2020 12:23:03 PM)"=15209, "Automatic Update (DT: Olivine-3-1; HV: 2.2; Time: 1/15/2020 12:23:04 PM)"=15210, "Automatic Update (DT: Olivine-3-1; HV: 2.2; Time: 1/15/2020 12:37:17 PM)"=15211, "Automatic Update (DT: Olivine-3-1; HV: 2.2; Time: 1/15/2020 12:37:19 PM)"=15212, "Automatic Update (DT: Olivine-3-1; HV: 2.2; Time: 1/15/2020 12:48:35 PM)"=15213, "Automatic Update (DT: Olivine-3-1; HV: 2.2; Time: 1/15/2020 12:48:36 PM)"=15214, "Automatic Update (DT: Olivine-3-1; HV: 2.2; Time: 1/15/2020 12:50:10 PM)"=15215, "Automatic Update (DT: Olivine-3-1; HV: 2.2; Time: 1/15/2020 12:50:12 PM)"=15216, "Automatic Update (DT: Olivine-3-1; HV: 2.2; Time: 1/15/2020 12:50:18 PM)"=15217, "Automatic Update (DT: Olivine-3-1; HV: 2.2; Time: 1/15/2020 12:50:21 PM)"=15218, "Automatic Update (DT: Olivine-3-1; HV: 2.2; Time: 1/15/2020 12:50:31 PM)"=15219, "Automatic Update (DT: Olivine-3-1; HV: 2.2; Time: 1/15/2020 1:12:14 PM)"=15220, "Automatic Update (DT: Olivine-3-1; HV: 2.2; Time: 1/15/2020 1:12:17 PM)"=15221, "Automatic Update (DT: Olivine-3-1; HV: 2.2; Time: 1/15/2020 1:26:43 PM)"=15222, "Automatic Update (DT: Olivine-3-1; HV: 2.2; Time: 1/15/2020 1:26:45 PM)"=15223, "Automatic Update (DT: Olivine-3-1; HV: 2.2; Time: 1/15/2020 1:43:04 PM)"=15224, "Automatic Update (DT: Olivine-3-1; HV: 2.2; Time: 1/15/2020 1:43:09 PM)"=15225, "Automatic Update (DT: Olivine-3-1; HV: 2.2; Time: 1/15/2020 1:50:45 PM)"=15226, "Automatic Update (DT: Olivine-3-1; HV: 2.2; Time: 1/16/2020 9:44:51 AM)"=15227, "Automatic Update (DT: Olivine-3-1; HV: 2.2; Time: 1/16/2020 9:45:01 AM)"=15228, "Automatic Update (DT: Olivine-3-1; HV: 2.2; Time: 1/16/2020 9:45:10 AM)"=15229, "Automatic Update (DT: Olivine-3-1; HV: 2.2; Time: 1/16/2020 9:45:20 AM)"=15230, "Automatic Update (DT: Olivine-3-1; HV: 2.2; Time: 1/16/2020 9:45:23 AM)"=15231, "Automatic Update (DT: Olivine-3-1; HV: 2.2; Time: 1/16/2020 9:45:36 AM)"=15232, "Automatic Update (DT: Olivine-3-1; HV: 2.2; Time: 1/16/2020 9:45:38 AM)"=15233, "Automatic Update (DT: Olivine-3-1; HV: 2.2; Time: 1/16/2020 9:45:42 AM)"=15234, "Automatic Update (DT: Olivine-3-1; HV: 2.2; Time: 1/16/2020 9:45:44 AM)"=15235, "Automatic Update (DT: Olivine-3-1; HV: 2.2; Time: 1/16/2020 9:45:46 AM)"=15236, "Automatic Update (DT: Olivine-3-1; HV: 2.2; Time: 1/16/2020 9:45:48 AM)"=15237, "Automatic Update (DT: Olivine-3-1; HV: 2.2; Time: 1/16/2020 9:45:51 AM)"=15238, "Automatic Update (DT: Olivine-3-1; HV: 2.2; Time: 1/16/2020 9:45:52 AM)"=15239, "Automatic Update (DT: Olivine-3-1; HV: 2.2; Time: 1/16/2020 9:45:53 AM)"=15240, "Automatic Update (DT: Olivine-3-1; HV: 2.2; Time: 1/16/2020 9:45:56 AM)"=15241, "Automatic Update (DT: Olivine-3-1; HV: 2.2; Time: 1/16/2020 9:46:00 AM)"=15242, "Automatic Update (DT: Olivine-3-1; HV: 2.2; Time: 1/16/2020 9:46:13 AM)"=15243, "Automatic Update (DT: Olivine-3-1; HV: 2.2; Time: 1/16/2020 9:46:17 AM)"=15244, "Automatic Update (DT: Olivine-3-1; HV: 2.2; Time: 1/16/2020 9:46:18 AM)"=15245, "Automatic Update (DT: Olivine-3-1; HV: 2.2; Time: 1/16/2020 9:46:20 AM)"=15246, "Automatic Update (DT: Olivine-3-1; HV: 2.2; Time: 1/16/2020 9:46:21 AM)"=15247, "Automatic Update (DT: Olivine-3-1; HV: 2.2; Time: 1/16/2020 9:46:23 AM)"=15248, "Automatic Update (DT: Olivine-3-1; HV: 2.2; Time: 1/16/2020 9:46:26 AM)"=15249, "Automatic Update (DT: Olivine-3-1; HV: 2.2; Time: 1/16/2020 9:46:27 AM)"=15250, "Automatic Update (DT: Olivine-3-1; HV: 2.2; Time: 1/16/2020 9:46:28 AM)"=15251, "Automatic Update (DT: Olivine-3-1; HV: 2.2; Time: 1/16/2020 9:46:29 AM)"=15252, "Automatic Update (DT: Olivine-3-1; HV: 2.2; Time: 1/16/2020 9:46:30 AM)"=15253, "Automatic Update (DT: Olivine-3-1; HV: 2.2; Time: 1/16/2020 9:46:31 AM)"=15254, "Automatic Update (DT: Olivine-3-1; HV: 2.2; Time: 1/16/2020 9:46:35 AM)"=15255, "Automatic Update (DT: Olivine-3-1; HV: 2.2; Time: 1/16/2020 9:46:36 AM)"=15256, "Automatic Update (DT: Olivine-3-1; HV: 2.2; Time: 1/16/2020 9:46:37 AM)"=15257, "Automatic Update (DT: Olivine-3-1; HV: 2.2; Time: 1/16/2020 9:46:38 AM)"=15258, "Automatic Update (DT: Olivine-3-1; HV: 2.2; Time: 1/16/2020 9:46:39 AM)"=15259, "Automatic Update (DT: Olivine-3-1; HV: 2.2; Time: 1/16/2020 9:46:40 AM)"=15260, "Automatic Update (DT: Olivine-3-1; HV: 2.2; Time: 1/16/2020 9:46:44 AM)"=15261, "Automatic Update (DT: Olivine-3-1; HV: 2.2; Time: 1/16/2020 9:46:45 AM)"=15262, "Automatic Update (DT: Olivine-3-1; HV: 2.2; Time: 1/16/2020 9:46:47 AM)"=15263, "Automatic Update (DT: Olivine-3-1; HV: 2.2; Time: 1/16/2020 9:46:48 AM)"=15264, "Automatic Update (DT: Olivine-3-1; HV: 2.2; Time: 1/16/2020 9:46:49 AM)"=15265, "Automatic Update (DT: Olivine-3-1; HV: 2.2; Time: 1/16/2020 9:46:52 AM)"=15266, "Automatic Update (DT: Olivine-3-1; HV: 2.2; Time: 1/16/2020 9:46:53 AM)"=15267, "Automatic Update (DT: Olivine-3-1; HV: 2.2; Time: 1/16/2020 9:46:54 AM)"=15268, "Automatic Update (DT: Olivine-3-1; HV: 2.2; Time: 1/16/2020 9:46:56 AM)"=15269, "Automatic Update (DT: Olivine-3-1; HV: 2.2; Time: 1/16/2020 9:46:57 AM)"=15270, "Automatic Update (DT: Olivine-3-1; HV: 2.2; Time: 1/16/2020 9:46:58 AM)"=15271, "Automatic Update (DT: Olivine-3-1; HV: 2.2; Time: 1/16/2020 9:47:01 AM)"=15272, "Automatic Update (DT: Olivine-3-1; HV: 2.2; Time: 1/16/2020 9:47:07 AM)"=15273, "Automatic Update (DT: Olivine-3-1; HV: 2.2; Time: 1/16/2020 9:47:10 AM)"=15274, "Automatic Update (DT: Olivine-3-1; HV: 2.2; Time: 1/16/2020 9:47:11 AM)"=15275, "Automatic Update (DT: Olivine-3-1; HV: 2.2; Time: 1/16/2020 9:47:12 AM)"=15276, "Automatic Update (DT: Olivine-3-1; HV: 2.2; Time: 1/16/2020 9:47:13 AM)"=15277, "Automatic Update (DT: Olivine-3-1; HV: 2.2; Time: 1/16/2020 9:47:14 AM)"=15278, "Automatic Update (DT: Olivine-3-1; HV: 2.2; Time: 1/16/2020 9:47:18 AM)"=15279, "Automatic Update (DT: Olivine-3-1; HV: 2.2; Time: 1/16/2020 9:47:19 AM)"=15280, "Automatic Update (DT: Olivine-3-1; HV: 2.2; Time: 1/16/2020 9:47:21 AM)"=15281, "Automatic Update (DT: Olivine-3-1; HV: 2.2; Time: 1/16/2020 9:47:24 AM)"=15282, "Automatic Update (DT: Olivine-3-1; HV: 2.2; Time: 1/16/2020 9:47:28 AM)"=15283, "Automatic Update (DT: Olivine-3-1; HV: 2.2; Time: 1/16/2020 9:47:33 AM)"=15284, "Automatic Update (DT: Olivine-3-1; HV: 2.2; Time: 1/16/2020 9:47:37 AM)"=15285, "Automatic Update (DT: Olivine-3-1; HV: 2.2; Time: 1/16/2020 9:47:38 AM)"=15286, "Automatic Update (DT: Olivine-3-1; HV: 2.2; Time: 1/16/2020 9:50:56 AM)"=15287, "Automatic Update (DT: Olivine-3-1; HV: 2.2; Time: 1/16/2020 9:50:57 AM)"=15288, "Automatic Update (DT: Olivine-3-1; HV: 2.2; Time: 1/16/2020 9:50:58 AM)"=15289, "Automatic Update (DT: Olivine-3-1; HV: 2.2; Time: 1/16/2020 9:51:02 AM)"=15290, "Automatic Update (DT: Olivine-3-1; HV: 2.2; Time: 1/16/2020 9:51:03 AM)"=15291, "Automatic Update (DT: Olivine-3-1; HV: 2.2; Time: 1/16/2020 9:51:05 AM)"=15292, "Automatic Update (DT: Olivine-3-1; HV: 2.2; Time: 1/16/2020 9:51:06 AM)"=15293, "Automatic Update (DT: Olivine-3-1; HV: 2.2; Time: 1/16/2020 9:51:07 AM)"=15294, "Automatic Update (DT: Olivine-3-1; HV: 2.2; Time: 1/16/2020 9:51:11 AM)"=15295, "Automatic Update (DT: Olivine-3-1; HV: 2.2; Time: 1/16/2020 9:51:12 AM)"=15296, "Automatic Update (DT: Olivine-3-1; HV: 2.2; Time: 1/16/2020 9:51:13 AM)"=15297, "Automatic Update (DT: Olivine-3-1; HV: 2.2; Time: 1/16/2020 9:51:14 AM)"=15298, "Automatic Update (DT: Olivine-3-1; HV: 2.2; Time: 1/16/2020 9:51:16 AM)"=15299, "Automatic Update (DT: Olivine-3-1; HV: 2.2; Time: 1/16/2020 9:51:17 AM)"=15300, "Automatic Update (DT: Olivine-3-1; HV: 2.2; Time: 1/16/2020 9:51:20 AM)"=15301, "Automatic Update (DT: Olivine-3-1; HV: 2.2; Time: 1/16/2020 9:51:21 AM)"=15302, "Automatic Update (DT: Olivine-3-1; HV: 2.2; Time: 1/16/2020 9:51:22 AM)"=15303, "Automatic Update (DT: Olivine-3-1; HV: 2.2; Time: 1/16/2020 9:51:23 AM)"=15304, "Automatic Update (DT: Olivine-3-1; HV: 2.2; Time: 1/16/2020 9:51:24 AM)"=15305, "Automatic Update (DT: Olivine-3-1; HV: 2.2; Time: 1/16/2020 9:51:26 AM)"=15306, "Automatic Update (DT: Olivine-3-1; HV: 2.2; Time: 1/16/2020 9:51:29 AM)"=15307, "Automatic Update (DT: Olivine-3-1; HV: 2.2; Time: 1/16/2020 9:51:30 AM)"=15308, "Automatic Update (DT: Olivine-3-1; HV: 2.2; Time: 1/16/2020 9:51:31 AM)"=15309, "Automatic Update (DT: Olivine-3-1; HV: 2.2; Time: 1/16/2020 9:51:32 AM)"=15310, "Automatic Update (DT: Olivine-3-1; HV: 2.2; Time: 1/16/2020 9:51:34 AM)"=15311, "Automatic Update (DT: Olivine-3-1; HV: 2.2; Time: 1/16/2020 9:51:38 AM)"=15312, "Automatic Update (DT: Olivine-3-1; HV: 2.2; Time: 1/16/2020 9:51:39 AM)"=15313, "Automatic Update (DT: Olivine-3-1; HV: 2.2; Time: 1/16/2020 9:51:40 AM)"=15314, "Automatic Update (DT: Olivine-3-1; HV: 2.2; Time: 1/16/2020 9:51:41 AM)"=15315, "Automatic Update (DT: Olivine-3-1; HV: 2.2; Time: 1/16/2020 9:51:42 AM)"=15316, "Automatic Update (DT: Olivine-3-1; HV: 2.2; Time: 1/16/2020 9:51:43 AM)"=15317, "Automatic Update (DT: Olivine-3-1; HV: 2.2; Time: 1/16/2020 9:51:47 AM)"=15318, "Automatic Update (DT: Olivine-3-1; HV: 2.2; Time: 1/16/2020 9:51:48 AM)"=15319, "Automatic Update (DT: Olivine-3-1; HV: 2.2; Time: 1/16/2020 9:51:49 AM)"=15320, "Automatic Update (DT: Olivine-3-1; HV: 2.2; Time: 1/16/2020 9:51:50 AM)"=15321, "Automatic Update (DT: Olivine-3-1; HV: 2.2; Time: 1/16/2020 9:51:51 AM)"=15322, "Automatic Update (DT: Olivine-3-1; HV: 2.2; Time: 1/16/2020 9:51:52 AM)"=15323, "Automatic Update (DT: Olivine-3-1; HV: 2.2; Time: 1/16/2020 9:51:56 AM)"=15324, "Automatic Update (DT: Olivine-3-1; HV: 2.2; Time: 1/16/2020 9:51:57 AM)"=15325, "Automatic Update (DT: Olivine-3-1; HV: 2.2; Time: 1/16/2020 9:51:58 AM)"=15326, "Automatic Update (DT: Olivine-3-1; HV: 2.2; Time: 1/16/2020 9:51:59 AM)"=15327, "Automatic Update (DT: Olivine-3-1; HV: 2.2; Time: 1/16/2020 9:52:00 AM)"=15328, "Automatic Update (DT: Olivine-3-1; HV: 2.2; Time: 1/16/2020 9:52:02 AM)"=15329, "Automatic Update (DT: Olivine-3-1; HV: 2.2; Time: 1/16/2020 9:52:04 AM)"=15330, "Automatic Update (DT: Olivine-3-1; HV: 2.2; Time: 1/16/2020 9:52:06 AM)"=15331, "Automatic Update (DT: Olivine-3-1; HV: 2.2; Time: 1/16/2020 9:52:07 AM)"=15332, "Automatic Update (DT: Olivine-3-1; HV: 2.2; Time: 1/16/2020 9:52:09 AM)"=15333, "Automatic Update (DT: Olivine-3-1; HV: 2.2; Time: 1/16/2020 9:52:10 AM)"=15334, "Automatic Update (DT: Olivine-3-1; HV: 2.2; Time: 1/16/2020 9:52:13 AM)"=15335, "Automatic Update (DT: Olivine-3-1; HV: 2.2; Time: 1/16/2020 9:54:06 AM)"=15336, "Automatic Update (DT: Olivine-3-1; HV: 2.2; Time: 1/16/2020 9:54:07 AM)"=15337, "Automatic Update (DT: Olivine-3-1; HV: 2.2; Time: 1/16/2020 10:08:11 AM)"=15338, "Automatic Update (DT: Olivine-3-1; HV: 2.2; Time: 1/16/2020 10:08:14 AM)"=15339, "Automatic Update (DT: Olivine-3-1; HV: 2.2; Time: 1/16/2020 10:13:37 AM)"=15340, "Automatic Update (DT: Olivine-3-1; HV: 2.2; Time: 1/16/2020 10:16:59 AM)"=15341, "Automatic Update (DT: Olivine-3-1; HV: 2.2; Time: 1/16/2020 10:17:09 AM)"=15342, "Automatic Update (DT: Olivine-3-1; HV: 2.2; Time: 1/16/2020 10:17:15 AM)"=15343, "Automatic Update (DT: Olivine-3-1; HV: 2.2; Time: 1/16/2020 10:17:21 AM)"=15344, "Automatic Update (DT: Olivine-3-1; HV: 2.2; Time: 1/16/2020 10:17:26 AM)"=15345, "Automatic Update (DT: Olivine-3-1; HV: 2.2; Time: 1/16/2020 10:17:33 AM)"=15346, "Automatic Update (DT: Olivine-3-1; HV: 2.2; Time: 1/16/2020 10:17:37 AM)"=15347, "Automatic Update (DT: Olivine-3-1; HV: 2.2; Time: 1/16/2020 10:17:38 AM)"=15348, "Automatic Update (DT: Olivine-3-1; HV: 2.2; Time: 1/16/2020 10:17:39 AM)"=15349, "Automatic Update (DT: Olivine-3-1; HV: 2.2; Time: 1/16/2020 10:17:40 AM)"=15350, "Automatic Update (DT: Olivine-3-1; HV: 2.2; Time: 1/16/2020 10:17:42 AM)"=15351, "Automatic Update (DT: Olivine-3-1; HV: 2.2; Time: 1/16/2020 10:17:45 AM)"=15352, "Automatic Update (DT: Olivine-3-1; HV: 2.2; Time: 1/16/2020 10:17:47 AM)"=15353, "Automatic Update (DT: Olivine-3-1; HV: 2.2; Time: 1/16/2020 10:17:48 AM)"=15354, "Automatic Update (DT: Olivine-3-1; HV: 2.2; Time: 1/16/2020 10:17:49 AM)"=15355, "Automatic Update (DT: Olivine-3-1; HV: 2.2; Time: 1/16/2020 10:17:50 AM)"=15356, "Automatic Update (DT: Olivine-3-1; HV: 2.2; Time: 1/16/2020 10:17:54 AM)"=15357, "Automatic Update (DT: Olivine-3-1; HV: 2.2; Time: 1/16/2020 10:17:55 AM)"=15358, "Automatic Update (DT: Olivine-3-1; HV: 2.2; Time: 1/16/2020 10:17:56 AM)"=15359, "Automatic Update (DT: Olivine-3-1; HV: 2.2; Time: 1/16/2020 10:17:57 AM)"=15360, "Automatic Update (DT: Olivine-3-1; HV: 2.2; Time: 1/16/2020 10:17:59 AM)"=15361, "Automatic Update (DT: Olivine-3-1; HV: 2.2; Time: 1/16/2020 10:18:00 AM)"=15362, "Automatic Update (DT: Olivine-3-1; HV: 2.2; Time: 1/16/2020 10:18:03 AM)"=15363, "Automatic Update (DT: Olivine-3-1; HV: 2.2; Time: 1/16/2020 10:18:06 AM)"=15364, "Automatic Update (DT: Olivine-3-1; HV: 2.2; Time: 1/16/2020 10:18:07 AM)"=15365, "Automatic Update (DT: Olivine-3-1; HV: 2.2; Time: 1/16/2020 10:18:08 AM)"=15366, "Automatic Update (DT: Olivine-3-1; HV: 2.2; Time: 1/16/2020 10:18:09 AM)"=15367, "Automatic Update (DT: Olivine-3-1; HV: 2.2; Time: 1/16/2020 10:18:13 AM)"=15368, "Automatic Update (DT: Olivine-3-1; HV: 2.2; Time: 1/16/2020 10:18:20 AM)"=15369, "Automatic Update (DT: Olivine-3-1; HV: 2.2; Time: 1/16/2020 10:18:22 AM)"=15370, "Automatic Update (DT: Olivine-3-1; HV: 2.2; Time: 1/16/2020 10:18:23 AM)"=15371, "Automatic Update (DT: Olivine-3-1; HV: 2.2; Time: 1/16/2020 10:18:24 AM)"=15372, "Automatic Update (DT: Olivine-3-1; HV: 2.2; Time: 1/16/2020 10:18:25 AM)"=15373, "Automatic Update (DT: Olivine-3-1; HV: 2.2; Time: 1/16/2020 10:18:26 AM)"=15374, "Automatic Update (DT: Olivine-3-1; HV: 2.2; Time: 1/16/2020 10:18:27 AM)"=15375, "Automatic Update (DT: Olivine-3-1; HV: 2.2; Time: 1/16/2020 10:18:31 AM)"=15376, "Automatic Update (DT: Olivine-3-1; HV: 2.2; Time: 1/16/2020 10:18:32 AM)"=15377, "Automatic Update (DT: Olivine-3-1; HV: 2.2; Time: 1/16/2020 10:18:33 AM)"=15378, "Automatic Update (DT: Olivine-3-1; HV: 2.2; Time: 1/16/2020 10:18:40 AM)"=15379, "Automatic Update (DT: Olivine-3-1; HV: 2.2; Time: 1/16/2020 10:18:42 AM)"=15380, "Automatic Update (DT: Olivine-3-1; HV: 2.2; Time: 1/16/2020 10:18:44 AM)"=15381, "Automatic Update (DT: Olivine-3-1; HV: 2.2; Time: 1/16/2020 10:18:47 AM)"=15382, "Automatic Update (DT: Olivine-3-1; HV: 2.2; Time: 1/16/2020 10:18:52 AM)"=15383, "Automatic Update (DT: Olivine-3-1; HV: 2.2; Time: 1/16/2020 10:18:57 AM)"=15384, "Automatic Update (DT: Olivine-3-1; HV: 2.2; Time: 1/16/2020 10:19:03 AM)"=15385, "Automatic Update (DT: Olivine-3-1; HV: 2.2; Time: 1/16/2020 10:19:04 AM)"=15386, "Automatic Update (DT: Olivine-3-1; HV: 2.2; Time: 1/16/2020 10:19:08 AM)"=15387, "Automatic Update (DT: Olivine-3-1; HV: 2.2; Time: 1/16/2020 10:19:10 AM)"=15388, "Automatic Update (DT: Olivine-3-1; HV: 2.2; Time: 1/16/2020 10:19:12 AM)"=15389, "Automatic Update (DT: Olivine-3-1; HV: 2.2; Time: 1/16/2020 10:19:13 AM)"=15390, "Automatic Update (DT: Olivine-3-1; HV: 2.2; Time: 1/16/2020 10:19:14 AM)"=15391, "Automatic Update (DT: Olivine-3-1; HV: 2.2; Time: 1/16/2020 10:19:25 AM)"=15392, "Automatic Update (DT: Olivine-3-1; HV: 2.2; Time: 1/16/2020 10:19:27 AM)"=15393, "Automatic Update (DT: Olivine-3-1; HV: 2.2; Time: 1/16/2020 10:19:43 AM)"=15394, "Automatic Update (DT: Olivine-3-1; HV: 2.2; Time: 1/16/2020 10:20:50 AM)"=15395, "Automatic Update (DT: Olivine-3-1; HV: 2.2; Time: 1/16/2020 10:30:26 AM)"=15396, "Automatic Update (DT: Olivine-3-1; HV: 2.2; Time: 1/16/2020 10:30:28 AM)"=15397, "Automatic Update (DT: Olivine-3-1; HV: 2.2; Time: 1/16/2020 10:30:30 AM)"=15398, "Automatic Update (DT: Olivine-3-1; HV: 2.2; Time: 1/16/2020 10:30:33 AM)"=15399, "Automatic Update (DT: Olivine-3-1; HV: 2.2; Time: 1/16/2020 10:30:34 AM)"=15400, "Automatic Update (DT: Olivine-3-1; HV: 2.2; Time: 1/16/2020 10:30:38 AM)"=15401, "Automatic Update (DT: Olivine-3-1; HV: 2.2; Time: 1/16/2020 10:30:42 AM)"=15402, "Automatic Update (DT: Olivine-3-1; HV: 2.2; Time: 1/16/2020 10:30:43 AM)"=15403, "Automatic Update (DT: Olivine-3-1; HV: 2.2; Time: 1/16/2020 10:30:50 AM)"=15404, "Automatic Update (DT: Olivine-3-1; HV: 2.2; Time: 1/16/2020 10:30:51 AM)"=15405, "Automatic Update (DT: Olivine-3-1; HV: 2.2; Time: 1/16/2020 10:30:52 AM)"=15406, "Automatic Update (DT: Olivine-3-1; HV: 2.2; Time: 1/16/2020 10:30:53 AM)"=15407, "Automatic Update (DT: Olivine-3-1; HV: 2.2; Time: 1/16/2020 10:30:55 AM)"=15408, "Automatic Update (DT: Olivine-3-1; HV: 2.2; Time: 1/16/2020 10:30:59 AM)"=15409, "Automatic Update (DT: Olivine-3-1; HV: 2.2; Time: 1/16/2020 10:31:00 AM)"=15410, "Automatic Update (DT: Olivine-3-1; HV: 2.2; Time: 1/16/2020 10:31:01 AM)"=15411, "Automatic Update (DT: Olivine-3-1; HV: 2.2; Time: 1/16/2020 10:31:02 AM)"=15412, "Automatic Update (DT: Olivine-3-1; HV: 2.2; Time: 1/16/2020 10:31:04 AM)"=15413, "Automatic Update (DT: Olivine-3-1; HV: 2.2; Time: 1/16/2020 10:31:09 AM)"=15414, "Automatic Update (DT: Olivine-3-1; HV: 2.2; Time: 1/16/2020 10:31:15 AM)"=15415, "Automatic Update (DT: Olivine-3-1; HV: 2.2; Time: 1/16/2020 10:31:18 AM)"=15416, "Automatic Update (DT: Olivine-3-1; HV: 2.2; Time: 1/16/2020 10:31:22 AM)"=15417, "Automatic Update (DT: Olivine-3-1; HV: 2.2; Time: 1/16/2020 10:31:23 AM)"=15418, "Automatic Update (DT: Olivine-3-1; HV: 2.2; Time: 1/16/2020 10:31:27 AM)"=15419, "Automatic Update (DT: Olivine-3-1; HV: 2.2; Time: 1/16/2020 10:31:57 AM)"=15420, "Automatic Update (DT: Olivine-3-1; HV: 2.2; Time: 1/16/2020 10:31:58 AM)"=15421, "Automatic Update (DT: Olivine-3-1; HV: 2.2; Time: 1/16/2020 10:32:05 AM)"=15422, "Automatic Update (DT: Olivine-3-1; HV: 2.2; Time: 1/16/2020 10:32:06 AM)"=15423, "Automatic Update (DT: Olivine-3-1; HV: 2.2; Time: 1/16/2020 10:32:10 AM)"=15424, "Automatic Update (DT: Olivine-3-1; HV: 2.2; Time: 1/16/2020 10:32:13 AM)"=15425, "Automatic Update (DT: Olivine-3-1; HV: 2.2; Time: 1/16/2020 10:32:14 AM)"=15426, "Automatic Update (DT: Olivine-3-1; HV: 2.2; Time: 1/16/2020 10:32:15 AM)"=15427, "Automatic Update (DT: Olivine-3-1; HV: 2.2; Time: 1/16/2020 10:32:17 AM)"=15428, "Automatic Update (DT: Olivine-3-1; HV: 2.2; Time: 1/16/2020 10:32:18 AM)"=15429, "Automatic Update (DT: Olivine-3-1; HV: 2.2; Time: 1/16/2020 10:32:19 AM)"=15430, "Automatic Update (DT: Olivine-3-1; HV: 2.2; Time: 1/16/2020 10:32:23 AM)"=15431, "Automatic Update (DT: Olivine-3-1; HV: 2.2; Time: 1/16/2020 10:32:24 AM)"=15432, "Automatic Update (DT: Olivine-3-1; HV: 2.2; Time: 1/16/2020 10:49:31 AM)"=15433, "Automatic Update (DT: Olivine-3-1; HV: 2.2; Time: 1/16/2020 10:49:42 AM)"=15434, "Automatic Update (DT: Olivine-3-1; HV: 2.2; Time: 1/16/2020 10:49:43 AM)"=15435, "Automatic Update (DT: Olivine-3-1; HV: 2.2; Time: 1/16/2020 10:49:44 AM)"=15436, "Automatic Update (DT: Olivine-3-1; HV: 2.2; Time: 1/16/2020 10:49:45 AM)"=15437, "Automatic Update (DT: Olivine-3-1; HV: 2.2; Time: 1/16/2020 10:49:49 AM)"=15438, "Automatic Update (DT: Olivine-3-1; HV: 2.2; Time: 1/16/2020 10:50:09 AM)"=15439, "Automatic Update (DT: Olivine-3-1; HV: 2.2; Time: 1/16/2020 10:50:11 AM)"=15440, "Automatic Update (DT: Olivine-3-1; HV: 2.2; Time: 1/16/2020 10:50:14 AM)"=15441, "Automatic Update (DT: Olivine-3-1; HV: 2.2; Time: 1/16/2020 10:50:15 AM)"=15442, "Automatic Update (DT: Olivine-3-1; HV: 2.2; Time: 1/16/2020 10:50:16 AM)"=15443, "Automatic Update (DT: Olivine-3-1; HV: 2.2; Time: 1/16/2020 11:13:54 AM)"=15444, "Automatic Update (DT: Olivine-3-1; HV: 2.2; Time: 1/16/2020 11:13:55 AM)"=15445, "Automatic Update (DT: Olivine-3-1; HV: 2.2; Time: 1/16/2020 11:14:13 AM)"=15446, "Automatic Update (DT: Olivine-3-1; HV: 2.2; Time: 1/16/2020 11:25:36 AM)"=15447, "Automatic Update (DT: Olivine-3-1; HV: 2.2; Time: 1/16/2020 11:25:40 AM)"=15448, "Automatic Update (DT: Olivine-3-1; HV: 2.2; Time: 1/16/2020 11:25:41 AM)"=15449, "Automatic Update (DT: Olivine-3-1; HV: 2.2; Time: 1/16/2020 11:25:42 AM)"=15450, "Automatic Update (DT: Olivine-3-1; HV: 2.2; Time: 1/16/2020 11:25:43 AM)"=15451, "Automatic Update (DT: Olivine-3-1; HV: 2.2; Time: 1/16/2020 11:25:44 AM)"=15452, "Automatic Update (DT: Olivine-3-1; HV: 2.2; Time: 1/16/2020 11:25:46 AM)"=15453, "Automatic Update (DT: Olivine-3-1; HV: 2.2; Time: 1/16/2020 11:25:49 AM)"=15454, "Automatic Update (DT: Olivine-3-1; HV: 2.2; Time: 1/16/2020 11:25:50 AM)"=15455, "Automatic Update (DT: Olivine-3-1; HV: 2.2; Time: 1/16/2020 11:25:52 AM)"=15456, "Automatic Update (DT: Olivine-3-1; HV: 2.2; Time: 1/16/2020 11:25:53 AM)"=15457, "Automatic Update (DT: Olivine-3-1; HV: 2.2; Time: 1/16/2020 11:25:54 AM)"=15458, "Automatic Update (DT: Olivine-3-1; HV: 2.2; Time: 1/16/2020 11:25:58 AM)"=15459, "Automatic Update (DT: Olivine-3-1; HV: 2.2; Time: 1/16/2020 11:25:59 AM)"=15460, "Automatic Update (DT: Olivine-3-1; HV: 2.2; Time: 1/16/2020 11:26:00 AM)"=15461, "Automatic Update (DT: Olivine-3-1; HV: 2.2; Time: 1/16/2020 11:26:01 AM)"=15462, "Automatic Update (DT: Olivine-3-1; HV: 2.2; Time: 1/16/2020 11:26:02 AM)"=15463, "Automatic Update (DT: Olivine-3-1; HV: 2.2; Time: 1/16/2020 11:26:09 AM)"=15464, "Automatic Update (DT: Olivine-3-1; HV: 2.2; Time: 1/16/2020 11:26:10 AM)"=15465, "Automatic Update (DT: Olivine-3-1; HV: 2.2; Time: 1/16/2020 11:26:11 AM)"=15466, "Automatic Update (DT: Olivine-3-1; HV: 2.2; Time: 1/16/2020 11:26:13 AM)"=15467, "Automatic Update (DT: Olivine-3-1; HV: 2.2; Time: 1/16/2020 11:26:14 AM)"=15468, "Automatic Update (DT: Olivine-3-1; HV: 2.2; Time: 1/16/2020 11:26:18 AM)"=15469, "Automatic Update (DT: Olivine-3-1; HV: 2.2; Time: 1/16/2020 11:26:19 AM)"=15470, "Automatic Update (DT: Olivine-3-1; HV: 2.2; Time: 1/16/2020 11:26:20 AM)"=15471, "Automatic Update (DT: Olivine-3-1; HV: 2.2; Time: 1/16/2020 11:26:29 AM)"=15472, "Automatic Update (DT: Olivine-3-1; HV: 2.2; Time: 1/16/2020 11:26:30 AM)"=15473, "Automatic Update (DT: Olivine-3-1; HV: 2.2; Time: 1/16/2020 11:26:31 AM)"=15474, "Automatic Update (DT: Olivine-3-1; HV: 2.2; Time: 1/16/2020 11:26:32 AM)"=15475, "Automatic Update (DT: Olivine-3-1; HV: 2.2; Time: 1/16/2020 11:26:36 AM)"=15476, "Automatic Update (DT: Olivine-3-1; HV: 2.2; Time: 1/16/2020 11:26:37 AM)"=15477, "Automatic Update (DT: Olivine-3-1; HV: 2.2; Time: 1/16/2020 11:26:38 AM)"=15478, "Automatic Update (DT: Olivine-3-1; HV: 2.2; Time: 1/16/2020 11:26:39 AM)"=15479, "Automatic Update (DT: Olivine-3-1; HV: 2.2; Time: 1/16/2020 11:26:41 AM)"=15480, "Automatic Update (DT: Olivine-3-1; HV: 2.2; Time: 1/16/2020 11:26:42 AM)"=15481, "Automatic Update (DT: Olivine-3-1; HV: 2.2; Time: 1/16/2020 11:26:46 AM)"=15482, "Automatic Update (DT: Olivine-3-1; HV: 2.2; Time: 1/16/2020 11:26:47 AM)"=15483, "Automatic Update (DT: Olivine-3-1; HV: 2.2; Time: 1/16/2020 11:26:48 AM)"=15484, "Automatic Update (DT: Olivine-3-1; HV: 2.2; Time: 1/16/2020 11:26:49 AM)"=15485, "Automatic Update (DT: Olivine-3-1; HV: 2.2; Time: 1/16/2020 11:26:50 AM)"=15486, "Automatic Update (DT: Olivine-3-1; HV: 2.2; Time: 1/16/2020 11:26:51 AM)"=15487, "Automatic Update (DT: Olivine-3-1; HV: 2.2; Time: 1/16/2020 11:26:55 AM)"=15488, "Automatic Update (DT: Olivine-3-1; HV: 2.2; Time: 1/16/2020 11:26:57 AM)"=15489, "Automatic Update (DT: Olivine-3-1; HV: 2.2; Time: 1/16/2020 11:26:58 AM)"=15490, "Automatic Update (DT: Olivine-3-1; HV: 2.2; Time: 1/16/2020 11:26:59 AM)"=15491, "Automatic Update (DT: Olivine-3-1; HV: 2.2; Time: 1/16/2020 11:27:01 AM)"=15492, "Automatic Update (DT: Olivine-3-1; HV: 2.2; Time: 1/16/2020 11:27:05 AM)"=15493, "Automatic Update (DT: Olivine-3-1; HV: 2.2; Time: 1/16/2020 11:58:25 AM)"=15494, "Automatic Update (DT: Olivine-3-1; HV: 2.2; Time: 1/16/2020 11:58:26 AM)"=15495, "Automatic Update (DT: Olivine-3-1; HV: 2.2; Time: 1/16/2020 11:58:38 AM)"=15496, "Automatic Update (DT: Olivine-3-1; HV: 2.2; Time: 1/16/2020 11:58:44 AM)"=15497, "Automatic Update (DT: Olivine-3-1; HV: 2.2; Time: 1/16/2020 11:58:45 AM)"=15498, "Automatic Update (DT: Olivine-3-1; HV: 2.2; Time: 1/16/2020 11:58:46 AM)"=15499, "Automatic Update (DT: Olivine-3-1; HV: 2.2; Time: 1/16/2020 11:58:49 AM)"=15500, "Automatic Update (DT: Olivine-3-1; HV: 2.2; Time: 1/16/2020 11:58:53 AM)"=15501, "Automatic Update (DT: Olivine-3-1; HV: 2.2; Time: 1/16/2020 11:58:54 AM)"=15502, "Automatic Update (DT: Olivine-3-1; HV: 2.2; Time: 1/16/2020 11:58:55 AM)"=15503, "Automatic Update (DT: Olivine-3-1; HV: 2.2; Time: 1/16/2020 11:58:56 AM)"=15504, "Automatic Update (DT: Olivine-3-1; HV: 2.2; Time: 1/16/2020 11:58:57 AM)"=15505, "Automatic Update (DT: Olivine-3-1; HV: 2.2; Time: 1/16/2020 11:58:59 AM)"=15506, "Automatic Update (DT: Olivine-3-1; HV: 2.2; Time: 1/16/2020 11:59:03 AM)"=15507, "Automatic Update (DT: Olivine-3-1; HV: 2.2; Time: 1/16/2020 11:59:06 AM)"=15508, "Automatic Update (DT: Olivine-3-1; HV: 2.2; Time: 1/16/2020 11:59:07 AM)"=15509, "Automatic Update (DT: Olivine-3-1; HV: 2.2; Time: 1/16/2020 11:59:08 AM)"=15510, "Automatic Update (DT: Olivine-3-1; HV: 2.2; Time: 1/16/2020 11:59:12 AM)"=15511, "Automatic Update (DT: Olivine-3-1; HV: 2.2; Time: 1/16/2020 11:59:14 AM)"=15512, "Automatic Update (DT: Olivine-3-1; HV: 2.2; Time: 1/16/2020 11:59:15 AM)"=15513, "Automatic Update (DT: Olivine-3-1; HV: 2.2; Time: 1/16/2020 11:59:16 AM)"=15514, "Automatic Update (DT: Olivine-3-1; HV: 2.2; Time: 1/16/2020 11:59:17 AM)"=15515, "Automatic Update (DT: Olivine-3-1; HV: 2.2; Time: 1/16/2020 11:59:21 AM)"=15516, "Automatic Update (DT: Olivine-3-1; HV: 2.2; Time: 1/16/2020 11:59:22 AM)"=15517, "Automatic Update (DT: Olivine-3-1; HV: 2.2; Time: 1/16/2020 11:59:23 AM)"=15518, "Automatic Update (DT: Olivine-3-1; HV: 2.2; Time: 1/16/2020 11:59:24 AM)"=15519, "Automatic Update (DT: Olivine-3-1; HV: 2.2; Time: 1/16/2020 11:59:26 AM)"=15520, "Automatic Update (DT: Olivine-3-1; HV: 2.2; Time: 1/16/2020 11:59:27 AM)"=15521, "Automatic Update (DT: Olivine-3-1; HV: 2.2; Time: 1/16/2020 11:59:31 AM)"=15522, "Automatic Update (DT: Olivine-3-1; HV: 2.2; Time: 1/16/2020 11:59:38 AM)"=15523, "Automatic Update (DT: Olivine-3-1; HV: 2.2; Time: 1/16/2020 12:17:39 PM)"=15524, "Automatic Update (DT: Olivine-3-1; HV: 2.2; Time: 1/16/2020 12:17:40 PM)"=15525, "Automatic Update (DT: Olivine-3-1; HV: 2.2; Time: 1/16/2020 12:17:41 PM)"=15526, "Automatic Update (DT: Olivine-3-1; HV: 2.2; Time: 1/16/2020 12:17:45 PM)"=15527, "Automatic Update (DT: Olivine-3-1; HV: 2.2; Time: 1/16/2020 12:17:46 PM)"=15528, "Automatic Update (DT: Olivine-3-1; HV: 2.2; Time: 1/16/2020 12:17:47 PM)"=15529, "Automatic Update (DT: Olivine-3-1; HV: 2.2; Time: 1/16/2020 12:17:48 PM)"=15530, "Automatic Update (DT: Olivine-3-1; HV: 2.2; Time: 1/16/2020 12:17:49 PM)"=15531, "Automatic Update (DT: Olivine-3-1; HV: 2.2; Time: 1/16/2020 12:17:50 PM)"=15532, "Automatic Update (DT: Olivine-3-1; HV: 2.2; Time: 1/16/2020 12:17:55 PM)"=15533, "Automatic Update (DT: Olivine-3-1; HV: 2.2; Time: 1/16/2020 12:17:56 PM)"=15534, "Automatic Update (DT: Olivine-3-1; HV: 2.2; Time: 1/16/2020 12:17:58 PM)"=15535, "Automatic Update (DT: Olivine-3-1; HV: 2.2; Time: 1/16/2020 12:17:59 PM)"=15536, "Automatic Update (DT: Olivine-3-1; HV: 2.2; Time: 1/16/2020 12:18:00 PM)"=15537, "Automatic Update (DT: Olivine-3-1; HV: 2.2; Time: 1/16/2020 12:18:04 PM)"=15538, "Automatic Update (DT: Olivine-3-1; HV: 2.2; Time: 1/16/2020 12:18:06 PM)"=15539, "Automatic Update (DT: Olivine-3-1; HV: 2.2; Time: 1/16/2020 12:18:08 PM)"=15540, "Automatic Update (DT: Olivine-3-1; HV: 2.2; Time: 1/16/2020 12:18:09 PM)"=15541, "Automatic Update (DT: Olivine-3-1; HV: 2.2; Time: 1/16/2020 12:18:14 PM)"=15542, "Automatic Update (DT: Olivine-3-1; HV: 2.2; Time: 1/16/2020 12:18:15 PM)"=15543, "Automatic Update (DT: Olivine-3-1; HV: 2.2; Time: 1/16/2020 12:18:16 PM)"=15544, "Automatic Update (DT: Olivine-3-1; HV: 2.2; Time: 1/16/2020 12:19:00 PM)"=15545, "Automatic Update (DT: Olivine-3-1; HV: 2.2; Time: 1/16/2020 12:19:02 PM)"=15546, "Automatic Update (DT: Olivine-3-1; HV: 2.2; Time: 1/16/2020 12:19:03 PM)"=15547, "Automatic Update (DT: Olivine-3-1; HV: 2.2; Time: 1/16/2020 12:19:15 PM)"=15548, "Automatic Update (DT: Olivine-3-1; HV: 2.2; Time: 1/16/2020 12:19:19 PM)"=15549, "Automatic Update (DT: Olivine-3-1; HV: 2.2; Time: 1/16/2020 12:19:27 PM)"=15550, "Automatic Update (DT: Olivine-3-1; HV: 2.2; Time: 1/16/2020 12:19:28 PM)"=15551, "Automatic Update (DT: Olivine-3-1; HV: 2.2; Time: 1/16/2020 12:19:40 PM)"=15552, "Automatic Update (DT: Olivine-3-1; HV: 2.2; Time: 1/16/2020 12:19:41 PM)"=15553, "Automatic Update (DT: Olivine-3-1; HV: 2.2; Time: 1/16/2020 12:19:42 PM)"=15554, "Automatic Update (DT: Olivine-3-1; HV: 2.2; Time: 1/16/2020 12:19:45 PM)"=15555, "Automatic Update (DT: Olivine-3-1; HV: 2.2; Time: 1/16/2020 12:19:47 PM)"=15556, "Automatic Update (DT: Olivine-3-1; HV: 2.2; Time: 1/16/2020 12:20:02 PM)"=15557, "Automatic Update (DT: Olivine-3-1; HV: 2.2; Time: 1/16/2020 12:20:06 PM)"=15558, "Automatic Update (DT: Olivine-3-1; HV: 2.2; Time: 1/16/2020 12:20:11 PM)"=15559, "Automatic Update (DT: Olivine-3-1; HV: 2.2; Time: 1/16/2020 12:20:15 PM)"=15560, "Automatic Update (DT: Olivine-3-1; HV: 2.2; Time: 1/16/2020 12:20:16 PM)"=15561, "Automatic Update (DT: Olivine-3-1; HV: 2.2; Time: 1/16/2020 12:20:17 PM)"=15562, "Automatic Update (DT: Olivine-3-1; HV: 2.2; Time: 1/16/2020 12:20:20 PM)"=15563, "Automatic Update (DT: Olivine-3-1; HV: 2.2; Time: 1/16/2020 12:20:24 PM)"=15564, "Automatic Update (DT: Olivine-3-1; HV: 2.2; Time: 1/16/2020 12:20:25 PM)"=15565, "Automatic Update (DT: Olivine-3-1; HV: 2.2; Time: 1/16/2020 12:20:26 PM)"=15566, "Automatic Update (DT: Olivine-3-1; HV: 2.2; Time: 1/16/2020 12:20:27 PM)"=15567, "Automatic Update (DT: Olivine-3-1; HV: 2.2; Time: 1/16/2020 12:20:32 PM)"=15568, "Automatic Update (DT: Olivine-3-1; HV: 2.2; Time: 1/16/2020 12:20:34 PM)"=15569, "Automatic Update (DT: Olivine-3-1; HV: 2.2; Time: 1/16/2020 12:20:36 PM)"=15570, "Automatic Update (DT: Olivine-3-1; HV: 2.2; Time: 1/16/2020 12:20:37 PM)"=15571, "Automatic Update (DT: Olivine-3-1; HV: 2.2; Time: 1/16/2020 12:20:47 PM)"=15572, "Automatic Update (DT: Olivine-3-1; HV: 2.2; Time: 1/16/2020 12:20:48 PM)"=15573, "Automatic Update (DT: Olivine-3-1; HV: 2.2; Time: 1/16/2020 12:20:52 PM)"=15574, "Automatic Update (DT: Olivine-3-1; HV: 2.2; Time: 1/16/2020 12:21:00 PM)"=15575, "Automatic Update (DT: Olivine-3-1; HV: 2.2; Time: 1/16/2020 12:21:02 PM)"=15576, "Automatic Update (DT: Olivine-3-1; HV: 2.2; Time: 1/16/2020 12:21:15 PM)"=15577, "Automatic Update (DT: Olivine-3-1; HV: 2.2; Time: 1/16/2020 12:21:16 PM)"=15578, "Automatic Update (DT: Olivine-3-1; HV: 2.2; Time: 1/16/2020 12:21:17 PM)"=15579, "Automatic Update (DT: Olivine-3-1; HV: 2.2; Time: 1/16/2020 12:21:21 PM)"=15580, "Automatic Update (DT: Olivine-3-1; HV: 2.2; Time: 1/16/2020 12:21:28 PM)"=15581, "Automatic Update (DT: Olivine-3-1; HV: 2.2; Time: 1/16/2020 12:21:30 PM)"=15582, "Automatic Update (DT: Olivine-3-1; HV: 2.2; Time: 1/16/2020 12:21:31 PM)"=15583, "Automatic Update (DT: Olivine-3-1; HV: 2.2; Time: 1/16/2020 12:21:32 PM)"=15584, "Automatic Update (DT: Olivine-3-1; HV: 2.2; Time: 1/16/2020 12:21:33 PM)"=15585, "Automatic Update (DT: Olivine-3-1; HV: 2.2; Time: 1/16/2020 12:21:34 PM)"=15586, "Automatic Update (DT: Olivine-3-1; HV: 2.2; Time: 1/16/2020 12:21:35 PM)"=15587, "Automatic Update (DT: Olivine-3-1; HV: 2.2; Time: 1/16/2020 12:21:39 PM)"=15588, "Automatic Update (DT: Olivine-3-1; HV: 2.2; Time: 1/16/2020 12:21:40 PM)"=15589, "Automatic Update (DT: Olivine-3-1; HV: 2.2; Time: 1/16/2020 12:21:41 PM)"=15590, "Automatic Update (DT: Olivine-3-1; HV: 2.2; Time: 1/16/2020 12:21:42 PM)"=15591, "Automatic Update (DT: Olivine-3-1; HV: 2.2; Time: 1/16/2020 12:21:44 PM)"=15592, "Automatic Update (DT: Olivine-3-1; HV: 2.2; Time: 1/16/2020 12:21:45 PM)"=15593, "Automatic Update (DT: Olivine-3-1; HV: 2.2; Time: 1/16/2020 12:21:49 PM)"=15594, "Automatic Update (DT: Olivine-3-1; HV: 2.2; Time: 1/16/2020 12:21:51 PM)"=15595, "Automatic Update (DT: Olivine-3-1; HV: 2.2; Time: 1/16/2020 12:21:52 PM)"=15596, "Automatic Update (DT: Olivine-3-1; HV: 2.2; Time: 1/16/2020 12:21:54 PM)"=15597, "Automatic Update (DT: Olivine-3-1; HV: 2.2; Time: 1/16/2020 12:21:58 PM)"=15598, "Automatic Update (DT: Olivine-3-1; HV: 2.2; Time: 1/16/2020 12:21:59 PM)"=15599, "Automatic Update (DT: Olivine-3-1; HV: 2.2; Time: 1/16/2020 12:22:00 PM)"=15600, "Automatic Update (DT: Olivine-3-1; HV: 2.2; Time: 1/16/2020 12:22:01 PM)"=15601, "Automatic Update (DT: Olivine-3-1; HV: 2.2; Time: 1/16/2020 12:22:02 PM)"=15602, "Automatic Update (DT: Olivine-3-1; HV: 2.2; Time: 1/16/2020 12:22:03 PM)"=15603, "Automatic Update (DT: Olivine-3-1; HV: 2.2; Time: 1/16/2020 12:22:07 PM)"=15604, "Automatic Update (DT: Olivine-3-1; HV: 2.2; Time: 1/16/2020 12:22:08 PM)"=15605, "Automatic Update (DT: Olivine-3-1; HV: 2.2; Time: 1/16/2020 12:22:09 PM)"=15606, "Automatic Update (DT: Olivine-3-1; HV: 2.2; Time: 1/16/2020 12:22:11 PM)"=15607, "Automatic Update (DT: Olivine-3-1; HV: 2.2; Time: 1/16/2020 12:22:12 PM)"=15608, "Automatic Update (DT: Olivine-3-1; HV: 2.2; Time: 1/16/2020 12:22:13 PM)"=15609, "Automatic Update (DT: Olivine-3-1; HV: 2.2; Time: 1/16/2020 12:22:17 PM)"=15610, "Automatic Update (DT: Olivine-3-1; HV: 2.2; Time: 1/16/2020 12:22:18 PM)"=15611, "Automatic Update (DT: Olivine-3-1; HV: 2.2; Time: 1/16/2020 12:22:19 PM)"=15612, "Automatic Update (DT: Olivine-3-1; HV: 2.2; Time: 1/16/2020 12:22:20 PM)"=15613, "Automatic Update (DT: Olivine-3-1; HV: 2.2; Time: 1/16/2020 12:22:21 PM)"=15614, "Automatic Update (DT: Olivine-3-1; HV: 2.2; Time: 1/16/2020 12:22:23 PM)"=15615, "Automatic Update (DT: Olivine-3-1; HV: 2.2; Time: 1/16/2020 12:23:05 PM)"=15616, "Automatic Update (DT: Olivine-3-1; HV: 2.2; Time: 1/16/2020 12:23:37 PM)"=15617, "Automatic Update (DT: Olivine-3-1; HV: 2.2; Time: 1/16/2020 12:23:41 PM)"=15618, "Automatic Update (DT: Olivine-3-1; HV: 2.2; Time: 1/16/2020 12:23:42 PM)"=15619, "Automatic Update (DT: Olivine-3-1; HV: 2.2; Time: 1/16/2020 12:23:43 PM)"=15620, "Automatic Update (DT: Olivine-3-1; HV: 2.2; Time: 1/16/2020 12:23:44 PM)"=15621, "Automatic Update (DT: Olivine-3-1; HV: 2.2; Time: 1/16/2020 12:23:45 PM)"=15622, "Automatic Update (DT: Olivine-3-1; HV: 2.2; Time: 1/16/2020 12:23:47 PM)"=15623, "Automatic Update (DT: Olivine-3-1; HV: 2.2; Time: 1/16/2020 12:23:50 PM)"=15624, "Automatic Update (DT: Olivine-3-1; HV: 2.2; Time: 1/16/2020 12:23:51 PM)"=15625, "Automatic Update (DT: Olivine-3-1; HV: 2.2; Time: 1/16/2020 12:23:52 PM)"=15626, "Automatic Update (DT: Olivine-3-1; HV: 2.2; Time: 1/16/2020 12:23:55 PM)"=15627, "Automatic Update (DT: Olivine-3-1; HV: 2.2; Time: 1/16/2020 12:23:57 PM)"=15628, "Automatic Update (DT: Olivine-3-1; HV: 2.2; Time: 1/16/2020 12:24:00 PM)"=15629, "Automatic Update (DT: Olivine-3-1; HV: 2.2; Time: 1/16/2020 12:24:01 PM)"=15630, "Automatic Update (DT: Olivine-3-1; HV: 2.2; Time: 1/16/2020 12:24:03 PM)"=15631, "Automatic Update (DT: Olivine-3-1; HV: 2.2; Time: 1/16/2020 12:24:04 PM)"=15632, "Automatic Update (DT: Olivine-3-1; HV: 2.2; Time: 1/16/2020 12:24:05 PM)"=15633, "Automatic Update (DT: Olivine-3-1; HV: 2.2; Time: 1/16/2020 12:24:09 PM)"=15634, "Automatic Update (DT: Olivine-3-1; HV: 2.2; Time: 1/16/2020 12:24:14 PM)"=15635, "Automatic Update (DT: Olivine-3-1; HV: 2.2; Time: 1/16/2020 12:25:19 PM)"=15636, "Automatic Update (DT: Olivine-3-1; HV: 2.2; Time: 1/16/2020 12:25:22 PM)"=15637, "Automatic Update (DT: Olivine-3-1; HV: 2.2; Time: 1/16/2020 12:25:30 PM)"=15638, "Automatic Update (DT: Olivine-3-1; HV: 2.2; Time: 1/16/2020 12:25:33 PM)"=15639, "Automatic Update (DT: Olivine-3-1; HV: 2.2; Time: 1/16/2020 12:25:37 PM)"=15640, "Automatic Update (DT: Olivine-3-1; HV: 2.2; Time: 1/16/2020 12:25:38 PM)"=15641, "Automatic Update (DT: Olivine-3-1; HV: 2.2; Time: 1/16/2020 12:25:42 PM)"=15642, "Automatic Update (DT: Olivine-3-1; HV: 2.2; Time: 1/16/2020 12:25:44 PM)"=15643, "Automatic Update (DT: Olivine-3-1; HV: 2.2; Time: 1/16/2020 12:25:45 PM)"=15644, "Automatic Update (DT: Olivine-3-1; HV: 2.2; Time: 1/16/2020 12:25:46 PM)"=15645, "Automatic Update (DT: Olivine-3-1; HV: 2.2; Time: 1/16/2020 12:25:47 PM)"=15646, "Automatic Update (DT: Olivine-3-1; HV: 2.2; Time: 1/16/2020 12:29:50 PM)"=15647, "Automatic Update (DT: Olivine-3-1; HV: 2.2; Time: 1/16/2020 12:29:51 PM)"=15648, "Automatic Update (DT: Olivine-3-1; HV: 2.2; Time: 1/16/2020 12:29:55 PM)"=15649, "Automatic Update (DT: Olivine-3-1; HV: 2.2; Time: 1/16/2020 12:29:56 PM)"=15650, "Automatic Update (DT: Olivine-3-1; HV: 2.2; Time: 1/16/2020 12:29:57 PM)"=15651, "Automatic Update (DT: Olivine-3-1; HV: 2.2; Time: 1/16/2020 12:29:58 PM)"=15652, "Automatic Update (DT: Olivine-3-1; HV: 2.2; Time: 1/16/2020 12:29:59 PM)"=15653, "Automatic Update (DT: Olivine-3-1; HV: 2.2; Time: 1/16/2020 12:30:00 PM)"=15654, "Automatic Update (DT: Olivine-3-1; HV: 2.2; Time: 1/16/2020 12:30:04 PM)"=15655, "Automatic Update (DT: Olivine-3-1; HV: 2.2; Time: 1/16/2020 12:30:05 PM)"=15656, "Automatic Update (DT: Olivine-3-1; HV: 2.2; Time: 1/16/2020 12:30:06 PM)"=15657, "Automatic Update (DT: Olivine-3-1; HV: 2.2; Time: 1/16/2020 12:30:07 PM)"=15658, "Automatic Update (DT: Olivine-3-1; HV: 2.2; Time: 1/16/2020 12:30:08 PM)"=15659, "Automatic Update (DT: Olivine-3-1; HV: 2.2; Time: 1/16/2020 12:30:09 PM)"=15660, "Automatic Update (DT: Olivine-3-1; HV: 2.2; Time: 1/16/2020 12:30:13 PM)"=15661, "Automatic Update (DT: Olivine-3-1; HV: 2.2; Time: 1/16/2020 12:30:15 PM)"=15662, "Automatic Update (DT: Olivine-3-1; HV: 2.2; Time: 1/16/2020 12:30:17 PM)"=15663, "Automatic Update (DT: Olivine-3-1; HV: 2.2; Time: 1/16/2020 12:30:18 PM)"=15664, "Automatic Update (DT: Olivine-3-1; HV: 2.2; Time: 1/16/2020 12:30:19 PM)"=15665, "Automatic Update (DT: Olivine-3-1; HV: 2.2; Time: 1/16/2020 12:30:23 PM)"=15666, "Automatic Update (DT: Olivine-3-1; HV: 2.2; Time: 1/16/2020 12:30:27 PM)"=15667, "Automatic Update (DT: Olivine-3-1; HV: 2.2; Time: 1/16/2020 12:30:28 PM)"=15668, "Automatic Update (DT: Olivine-3-1; HV: 2.2; Time: 1/16/2020 12:30:32 PM)"=15669, "Automatic Update (DT: Olivine-3-1; HV: 2.2; Time: 1/16/2020 12:30:33 PM)"=15670, "Automatic Update (DT: Olivine-3-1; HV: 2.2; Time: 1/16/2020 12:30:41 PM)"=15671, "Automatic Update (DT: Olivine-3-1; HV: 2.2; Time: 1/16/2020 12:30:43 PM)"=15672, "Automatic Update (DT: Olivine-3-1; HV: 2.2; Time: 1/16/2020 12:30:44 PM)"=15673, "Automatic Update (DT: Olivine-3-1; HV: 2.2; Time: 1/16/2020 12:30:45 PM)"=15674, "Automatic Update (DT: Olivine-3-1; HV: 2.2; Time: 1/16/2020 12:30:46 PM)"=15675, "Automatic Update (DT: Olivine-3-1; HV: 2.2; Time: 1/16/2020 12:30:47 PM)"=15676, "Automatic Update (DT: Olivine-3-1; HV: 2.2; Time: 1/16/2020 12:30:51 PM)"=15677, "Automatic Update (DT: Olivine-3-1; HV: 2.2; Time: 1/16/2020 12:30:52 PM)"=15678, "Automatic Update (DT: Olivine-3-1; HV: 2.2; Time: 1/16/2020 12:30:53 PM)"=15679, "Automatic Update (DT: Olivine-3-1; HV: 2.2; Time: 1/16/2020 12:30:54 PM)"=15680, "Automatic Update (DT: Olivine-3-1; HV: 2.2; Time: 1/16/2020 12:30:55 PM)"=15681, "Automatic Update (DT: Olivine-3-1; HV: 2.2; Time: 1/16/2020 12:30:56 PM)"=15682, "Automatic Update (DT: Olivine-3-1; HV: 2.2; Time: 1/16/2020 12:31:00 PM)"=15683, "Automatic Update (DT: Olivine-3-1; HV: 2.2; Time: 1/16/2020 12:31:01 PM)"=15684, "Automatic Update (DT: Olivine-3-1; HV: 2.2; Time: 1/16/2020 12:31:02 PM)"=15685, "Automatic Update (DT: Olivine-3-1; HV: 2.2; Time: 1/16/2020 12:31:03 PM)"=15686, "Automatic Update (DT: Olivine-3-1; HV: 2.2; Time: 1/16/2020 12:31:04 PM)"=15687, "Automatic Update (DT: Olivine-3-1; HV: 2.2; Time: 1/16/2020 12:31:05 PM)"=15688, "Automatic Update (DT: Olivine-3-1; HV: 2.2; Time: 1/16/2020 12:31:18 PM)"=15689, "Automatic Update (DT: Olivine-3-1; HV: 2.2; Time: 1/16/2020 12:31:19 PM)"=15690, "Automatic Update (DT: Olivine-3-1; HV: 2.2; Time: 1/16/2020 12:31:20 PM)"=15691, "Automatic Update (DT: Olivine-3-1; HV: 2.2; Time: 1/16/2020 12:31:21 PM)"=15692, "Automatic Update (DT: Olivine-3-1; HV: 2.2; Time: 1/16/2020 12:31:23 PM)"=15693, "Automatic Update (DT: Olivine-3-1; HV: 2.2; Time: 1/16/2020 12:31:24 PM)"=15694, "Automatic Update (DT: Olivine-3-1; HV: 2.2; Time: 1/16/2020 12:31:28 PM)"=15695, "Automatic Update (DT: Olivine-3-1; HV: 2.2; Time: 1/16/2020 12:31:38 PM)"=15696, "Automatic Update (DT: Olivine-3-1; HV: 2.2; Time: 1/16/2020 12:31:39 PM)"=15697, "Automatic Update (DT: Olivine-3-1; HV: 2.2; Time: 1/16/2020 12:31:42 PM)"=15698, "Automatic Update (DT: Olivine-3-1; HV: 2.2; Time: 1/16/2020 12:31:43 PM)"=15699, "Automatic Update (DT: Olivine-3-1; HV: 2.2; Time: 1/16/2020 12:31:47 PM)"=15700, "Automatic Update (DT: Olivine-3-1; HV: 2.2; Time: 1/16/2020 12:31:49 PM)"=15701, "Automatic Update (DT: Olivine-3-1; HV: 2.2; Time: 1/16/2020 12:31:50 PM)"=15702, "Automatic Update (DT: Olivine-3-1; HV: 2.2; Time: 1/16/2020 12:31:51 PM)"=15703, "Automatic Update (DT: Olivine-3-1; HV: 2.2; Time: 1/16/2020 12:31:52 PM)"=15704, "Automatic Update (DT: Olivine-3-1; HV: 2.2; Time: 1/16/2020 12:31:56 PM)"=15705, "Automatic Update (DT: Olivine-3-1; HV: 2.2; Time: 1/16/2020 12:32:00 PM)"=15706, "Automatic Update (DT: Olivine-3-1; HV: 2.2; Time: 1/16/2020 12:32:01 PM)"=15707, "Automatic Update (DT: Olivine-3-1; HV: 2.2; Time: 1/16/2020 12:32:02 PM)"=15708, "Automatic Update (DT: Olivine-3-1; HV: 2.2; Time: 1/16/2020 12:32:06 PM)"=15709, "Automatic Update (DT: Olivine-3-1; HV: 2.2; Time: 1/16/2020 12:32:07 PM)"=15710, "Automatic Update (DT: Olivine-3-1; HV: 2.2; Time: 1/16/2020 12:32:08 PM)"=15711, "Automatic Update (DT: Olivine-3-1; HV: 2.2; Time: 1/16/2020 12:32:09 PM)"=15712, "Automatic Update (DT: Olivine-3-1; HV: 2.2; Time: 1/16/2020 12:32:10 PM)"=15713, "Automatic Update (DT: Olivine-3-1; HV: 2.2; Time: 1/16/2020 12:32:11 PM)"=15714, "Automatic Update (DT: Olivine-3-1; HV: 2.2; Time: 1/16/2020 12:32:15 PM)"=15715, "Automatic Update (DT: Olivine-3-1; HV: 2.2; Time: 1/16/2020 12:32:17 PM)"=15716, "Automatic Update (DT: Olivine-3-1; HV: 2.2; Time: 1/16/2020 12:32:20 PM)"=15717, "Automatic Update (DT: Olivine-3-1; HV: 2.2; Time: 1/16/2020 12:32:24 PM)"=15718, "Automatic Update (DT: Olivine-3-1; HV: 2.2; Time: 1/16/2020 12:32:27 PM)"=15719, "Automatic Update (DT: Olivine-3-1; HV: 2.2; Time: 1/16/2020 12:32:28 PM)"=15720, "Automatic Update (DT: Olivine-3-1; HV: 2.2; Time: 1/16/2020 12:32:33 PM)"=15721, "Automatic Update (DT: Olivine-3-1; HV: 2.2; Time: 1/16/2020 12:32:34 PM)"=15722, "Automatic Update (DT: Olivine-3-1; HV: 2.2; Time: 1/16/2020 12:32:35 PM)"=15723, "Automatic Update (DT: Olivine-3-1; HV: 2.2; Time: 1/16/2020 12:32:36 PM)"=15724, "Automatic Update (DT: Olivine-3-1; HV: 2.2; Time: 1/16/2020 12:32:37 PM)"=15725, "Automatic Update (DT: Olivine-3-1; HV: 2.2; Time: 1/16/2020 12:32:38 PM)"=15726, "Automatic Update (DT: Olivine-3-1; HV: 2.2; Time: 1/16/2020 12:32:39 PM)"=15727, "Automatic Update (DT: Olivine-3-1; HV: 2.2; Time: 1/16/2020 12:32:43 PM)"=15728, "Automatic Update (DT: Olivine-3-1; HV: 2.2; Time: 1/16/2020 12:32:44 PM)"=15729, "Automatic Update (DT: Olivine-3-1; HV: 2.2; Time: 1/16/2020 12:32:46 PM)"=15730, "Automatic Update (DT: Olivine-3-1; HV: 2.2; Time: 1/16/2020 12:34:04 PM)"=15731, "Automatic Update (DT: Olivine-3-1; HV: 2.2; Time: 1/16/2020 12:34:07 PM)"=15732, "Automatic Update (DT: Olivine-3-1; HV: 2.2; Time: 1/16/2020 12:34:08 PM)"=15733, "Automatic Update (DT: Olivine-3-1; HV: 2.2; Time: 1/16/2020 12:34:09 PM)"=15734, "Automatic Update (DT: Olivine-3-1; HV: 2.2; Time: 1/16/2020 12:34:11 PM)"=15735, "Automatic Update (DT: Olivine-3-1; HV: 2.2; Time: 1/16/2020 12:34:12 PM)"=15736, "Automatic Update (DT: Olivine-3-1; HV: 2.2; Time: 1/16/2020 12:34:16 PM)"=15737, "Automatic Update (DT: Olivine-3-1; HV: 2.2; Time: 1/16/2020 12:34:17 PM)"=15738, "Automatic Update (DT: Olivine-3-1; HV: 2.2; Time: 1/16/2020 12:34:18 PM)"=15739, "Automatic Update (DT: Olivine-3-1; HV: 2.2; Time: 1/16/2020 12:34:19 PM)"=15740, "Automatic Update (DT: Olivine-3-1; HV: 2.2; Time: 1/16/2020 12:34:20 PM)"=15741, "Automatic Update (DT: Olivine-3-1; HV: 2.2; Time: 1/16/2020 12:34:22 PM)"=15742, "Automatic Update (DT: Olivine-3-1; HV: 2.2; Time: 1/16/2020 12:34:25 PM)"=15743, "Automatic Update (DT: Olivine-3-1; HV: 2.2; Time: 1/16/2020 12:34:27 PM)"=15744, "Automatic Update (DT: Olivine-3-1; HV: 2.2; Time: 1/16/2020 12:34:30 PM)"=15745, "Automatic Update (DT: Olivine-3-1; HV: 2.2; Time: 1/16/2020 12:34:31 PM)"=15746, "Automatic Update (DT: Olivine-3-1; HV: 2.2; Time: 1/16/2020 12:34:35 PM)"=15747, "Automatic Update (DT: Olivine-3-1; HV: 2.2; Time: 1/16/2020 12:34:39 PM)"=15748, "Automatic Update (DT: Olivine-3-1; HV: 2.2; Time: 1/16/2020 12:34:40 PM)"=15749, "Automatic Update (DT: Olivine-3-1; HV: 2.2; Time: 1/16/2020 12:34:44 PM)"=15750, "Automatic Update (DT: Olivine-3-1; HV: 2.2; Time: 1/16/2020 12:34:45 PM)"=15751, "Automatic Update (DT: Olivine-3-1; HV: 2.2; Time: 1/16/2020 12:34:54 PM)"=15752, "Automatic Update (DT: Olivine-3-1; HV: 2.2; Time: 1/16/2020 12:34:56 PM)"=15753, "Automatic Update (DT: Olivine-3-1; HV: 2.2; Time: 1/16/2020 12:34:57 PM)"=15754, "Automatic Update (DT: Olivine-3-1; HV: 2.2; Time: 1/16/2020 12:34:58 PM)"=15755, "Automatic Update (DT: Olivine-3-1; HV: 2.2; Time: 1/16/2020 12:34:59 PM)"=15756, "Automatic Update (DT: Olivine-3-1; HV: 2.2; Time: 1/16/2020 12:35:03 PM)"=15757, "Automatic Update (DT: Olivine-3-1; HV: 2.2; Time: 1/16/2020 12:35:04 PM)"=15758, "Automatic Update (DT: Olivine-3-1; HV: 2.2; Time: 1/16/2020 12:35:36 PM)"=15759, "Automatic Update (DT: Olivine-3-1; HV: 2.2; Time: 1/16/2020 12:35:40 PM)"=15760, "Automatic Update (DT: Olivine-3-1; HV: 2.2; Time: 1/16/2020 12:35:47 PM)"=15761, "Automatic Update (DT: Olivine-3-1; HV: 2.2; Time: 1/16/2020 12:35:50 PM)"=15762, "Automatic Update (DT: Olivine-3-1; HV: 2.2; Time: 1/16/2020 12:35:51 PM)"=15763, "Automatic Update (DT: Olivine-3-1; HV: 2.2; Time: 1/16/2020 12:35:52 PM)"=15764, "Automatic Update (DT: Olivine-3-1; HV: 2.2; Time: 1/16/2020 12:35:54 PM)"=15765, "Automatic Update (DT: Olivine-3-1; HV: 2.2; Time: 1/16/2020 12:35:55 PM)"=15766, "Automatic Update (DT: Olivine-3-1; HV: 2.2; Time: 1/16/2020 12:35:59 PM)"=15767, "Automatic Update (DT: Olivine-3-1; HV: 2.2; Time: 1/16/2020 12:36:00 PM)"=15768, "Automatic Update (DT: Olivine-3-1; HV: 2.2; Time: 1/16/2020 12:36:01 PM)"=15769, "Automatic Update (DT: Olivine-3-1; HV: 2.2; Time: 1/16/2020 12:36:02 PM)"=15770, "Automatic Update (DT: Olivine-3-1; HV: 2.2; Time: 1/16/2020 12:36:03 PM)"=15771, "Automatic Update (DT: Olivine-3-1; HV: 2.2; Time: 1/16/2020 12:36:04 PM)"=15772, "Automatic Update (DT: Olivine-3-1; HV: 2.2; Time: 1/16/2020 12:36:09 PM)"=15773, "Automatic Update (DT: Olivine-3-1; HV: 2.2; Time: 1/16/2020 12:36:10 PM)"=15774, "Automatic Update (DT: Olivine-3-1; HV: 2.2; Time: 1/16/2020 12:36:11 PM)"=15775, "Automatic Update (DT: Olivine-3-1; HV: 2.2; Time: 1/16/2020 12:36:12 PM)"=15776, "Automatic Update (DT: Olivine-3-1; HV: 2.2; Time: 1/16/2020 12:36:55 PM)"=15777, "Automatic Update (DT: Olivine-3-1; HV: 2.2; Time: 1/16/2020 12:36:56 PM)"=15778, "Automatic Update (DT: Olivine-3-1; HV: 2.2; Time: 1/16/2020 12:37:06 PM)"=15779, "Automatic Update (DT: Olivine-3-1; HV: 2.2; Time: 1/16/2020 12:37:07 PM)"=15780, "Automatic Update (DT: Olivine-3-1; HV: 2.2; Time: 1/16/2020 12:37:08 PM)"=15781, "Automatic Update (DT: Olivine-3-1; HV: 2.2; Time: 1/16/2020 12:37:12 PM)"=15782, "Automatic Update (DT: Olivine-3-1; HV: 2.2; Time: 1/16/2020 12:37:14 PM)"=15783, "Automatic Update (DT: Olivine-3-1; HV: 2.2; Time: 1/16/2020 12:37:15 PM)"=15784, "Automatic Update (DT: Olivine-3-1; HV: 2.2; Time: 1/16/2020 12:37:16 PM)"=15785, "Automatic Update (DT: Olivine-3-1; HV: 2.2; Time: 1/16/2020 12:37:19 PM)"=15786, "Automatic Update (DT: Olivine-3-1; HV: 2.2; Time: 1/16/2020 12:37:23 PM)"=15787, "Automatic Update (DT: Olivine-3-1; HV: 2.2; Time: 1/16/2020 12:37:28 PM)"=15788, "Automatic Update (DT: Olivine-3-1; HV: 2.2; Time: 1/16/2020 12:37:29 PM)"=15789, "Automatic Update (DT: Olivine-3-1; HV: 2.2; Time: 1/16/2020 12:37:33 PM)"=15790, "Automatic Update (DT: Olivine-3-1; HV: 2.2; Time: 1/16/2020 12:37:39 PM)"=15791, "Automatic Update (DT: Olivine-3-1; HV: 2.2; Time: 1/16/2020 12:37:42 PM)"=15792, "Automatic Update (DT: Olivine-3-1; HV: 2.2; Time: 1/16/2020 12:37:44 PM)"=15793, "Automatic Update (DT: Olivine-3-1; HV: 2.2; Time: 1/16/2020 12:37:46 PM)"=15794, "Automatic Update (DT: Olivine-3-1; HV: 2.2; Time: 1/16/2020 12:37:47 PM)"=15795, "Automatic Update (DT: Olivine-3-1; HV: 2.2; Time: 1/16/2020 12:37:51 PM)"=15796, "Automatic Update (DT: Olivine-3-1; HV: 2.2; Time: 1/16/2020 12:37:54 PM)"=15797, "Automatic Update (DT: Olivine-3-1; HV: 2.2; Time: 1/16/2020 12:37:56 PM)"=15798, "Automatic Update (DT: Olivine-3-1; HV: 2.2; Time: 1/16/2020 12:38:01 PM)"=15799, "Automatic Update (DT: Olivine-3-1; HV: 2.2; Time: 1/16/2020 12:38:02 PM)"=15800, "Automatic Update (DT: Olivine-3-1; HV: 2.2; Time: 1/16/2020 12:38:05 PM)"=15801, "Automatic Update (DT: Olivine-3-1; HV: 2.2; Time: 1/16/2020 12:38:06 PM)"=15802, "Automatic Update (DT: Olivine-3-1; HV: 2.2; Time: 1/16/2020 12:38:10 PM)"=15803, "Automatic Update (DT: Olivine-3-1; HV: 2.2; Time: 1/16/2020 12:38:11 PM)"=15804, "Automatic Update (DT: Olivine-3-1; HV: 2.2; Time: 1/16/2020 12:38:12 PM)"=15805, "Automatic Update (DT: Olivine-3-1; HV: 2.2; Time: 1/16/2020 12:38:13 PM)"=15806, "Automatic Update (DT: Olivine-3-1; HV: 2.2; Time: 1/16/2020 12:38:14 PM)"=15807, "Automatic Update (DT: Olivine-3-1; HV: 2.2; Time: 1/16/2020 12:38:16 PM)"=15808, "Automatic Update (DT: Olivine-3-1; HV: 2.2; Time: 1/16/2020 12:38:20 PM)"=15809, "Automatic Update (DT: Olivine-3-1; HV: 2.2; Time: 1/16/2020 12:38:21 PM)"=15810, "Automatic Update (DT: Olivine-3-1; HV: 2.2; Time: 1/16/2020 12:38:24 PM)"=15811, "Automatic Update (DT: Olivine-3-1; HV: 2.2; Time: 1/16/2020 12:38:25 PM)"=15812, "Automatic Update (DT: Olivine-3-1; HV: 2.2; Time: 1/16/2020 12:38:29 PM)"=15813, "Automatic Update (DT: Olivine-3-1; HV: 2.2; Time: 1/16/2020 12:38:30 PM)"=15814, "Automatic Update (DT: Olivine-3-1; HV: 2.2; Time: 1/16/2020 12:38:31 PM)"=15815, "Automatic Update (DT: Olivine-3-1; HV: 2.2; Time: 1/16/2020 12:38:32 PM)"=15816, "Automatic Update (DT: Olivine-3-1; HV: 2.2; Time: 1/16/2020 12:38:33 PM)"=15817, "Automatic Update (DT: Olivine-3-1; HV: 2.2; Time: 1/16/2020 12:38:36 PM)"=15818, "Automatic Update (DT: Olivine-3-1; HV: 2.2; Time: 1/16/2020 12:38:38 PM)"=15819, "Automatic Update (DT: Olivine-3-1; HV: 2.2; Time: 1/16/2020 12:38:39 PM)"=15820, "Automatic Update (DT: Olivine-3-1; HV: 2.2; Time: 1/16/2020 12:38:46 PM)"=15821, "Automatic Update (DT: Olivine-3-1; HV: 2.2; Time: 1/16/2020 12:38:48 PM)"=15822, "Automatic Update (DT: Olivine-3-1; HV: 2.2; Time: 1/16/2020 12:38:49 PM)"=15823, "Automatic Update (DT: Olivine-3-1; HV: 2.2; Time: 1/16/2020 12:38:51 PM)"=15824, "Automatic Update (DT: Olivine-3-1; HV: 2.2; Time: 1/16/2020 12:38:52 PM)"=15825, "Automatic Update (DT: Olivine-3-1; HV: 2.2; Time: 1/16/2020 12:38:53 PM)"=15826, "Automatic Update (DT: Olivine-3-1; HV: 2.2; Time: 1/16/2020 12:38:57 PM)"=15827, "Automatic Update (DT: Olivine-3-1; HV: 2.2; Time: 1/16/2020 12:38:58 PM)"=15828, "Automatic Update (DT: Olivine-3-1; HV: 2.2; Time: 1/16/2020 12:38:59 PM)"=15829, "Automatic Update (DT: Olivine-3-1; HV: 2.2; Time: 1/16/2020 12:39:01 PM)"=15830, "Automatic Update (DT: Olivine-3-1; HV: 2.2; Time: 1/16/2020 12:39:02 PM)"=15831, "Automatic Update (DT: Olivine-3-1; HV: 2.2; Time: 1/16/2020 12:39:06 PM)"=15832, "Automatic Update (DT: Olivine-3-1; HV: 2.2; Time: 1/16/2020 12:39:09 PM)"=15833, "Automatic Update (DT: Olivine-3-1; HV: 2.2; Time: 1/16/2020 12:39:10 PM)"=15834, "Automatic Update (DT: Olivine-3-1; HV: 2.2; Time: 1/16/2020 12:39:11 PM)"=15835, "Automatic Update (DT: Olivine-3-1; HV: 2.2; Time: 1/16/2020 12:39:12 PM)"=15836, "Automatic Update (DT: Olivine-3-1; HV: 2.2; Time: 1/16/2020 12:39:16 PM)"=15837, "Automatic Update (DT: Olivine-3-1; HV: 2.2; Time: 1/16/2020 12:39:17 PM)"=15838, "Automatic Update (DT: Olivine-3-1; HV: 2.2; Time: 1/16/2020 12:39:18 PM)"=15839, "Automatic Update (DT: Olivine-3-1; HV: 2.2; Time: 1/16/2020 12:39:20 PM)"=15840, "Automatic Update (DT: Olivine-3-1; HV: 2.2; Time: 1/16/2020 12:39:21 PM)"=15841, "Automatic Update (DT: Olivine-3-1; HV: 2.2; Time: 1/16/2020 12:39:25 PM)"=15842, "Automatic Update (DT: Olivine-3-1; HV: 2.2; Time: 1/16/2020 12:39:31 PM)"=15843, "Automatic Update (DT: Olivine-3-1; HV: 2.2; Time: 1/16/2020 12:39:35 PM)"=15844, "Automatic Update (DT: Olivine-3-1; HV: 2.2; Time: 1/16/2020 12:39:39 PM)"=15845, "Automatic Update (DT: Olivine-3-1; HV: 2.2; Time: 1/16/2020 12:39:40 PM)"=15846, "Automatic Update (DT: Olivine-3-1; HV: 2.2; Time: 1/16/2020 12:39:44 PM)"=15847, "Automatic Update (DT: Olivine-3-1; HV: 2.2; Time: 1/16/2020 12:39:45 PM)"=15848, "Automatic Update (DT: Olivine-3-1; HV: 2.2; Time: 1/16/2020 12:39:46 PM)"=15849, "Automatic Update (DT: Olivine-3-1; HV: 2.2; Time: 1/16/2020 12:39:52 PM)"=15850, "Automatic Update (DT: Olivine-3-1; HV: 2.2; Time: 1/16/2020 12:39:54 PM)"=15851, "Automatic Update (DT: Olivine-3-1; HV: 2.2; Time: 1/16/2020 12:39:55 PM)"=15852, "Automatic Update (DT: Olivine-3-1; HV: 2.2; Time: 1/16/2020 12:39:57 PM)"=15853, "Automatic Update (DT: Olivine-3-1; HV: 2.2; Time: 1/16/2020 12:39:58 PM)"=15854, "Automatic Update (DT: Olivine-3-1; HV: 2.2; Time: 1/16/2020 12:39:59 PM)"=15855, "Automatic Update (DT: Olivine-3-1; HV: 2.2; Time: 1/16/2020 12:40:03 PM)"=15856, "Automatic Update (DT: Olivine-3-1; HV: 2.2; Time: 1/16/2020 12:40:04 PM)"=15857, "Automatic Update (DT: Olivine-3-1; HV: 2.2; Time: 1/16/2020 12:40:05 PM)"=15858, "Automatic Update (DT: Olivine-3-1; HV: 2.2; Time: 1/16/2020 12:40:06 PM)"=15859, "Automatic Update (DT: Olivine-3-1; HV: 2.2; Time: 1/16/2020 12:40:07 PM)"=15860, "Automatic Update (DT: Olivine-3-1; HV: 2.2; Time: 1/16/2020 12:40:11 PM)"=15861, "Automatic Update (DT: Olivine-3-1; HV: 2.2; Time: 1/16/2020 12:40:13 PM)"=15862, "Automatic Update (DT: Olivine-3-1; HV: 2.2; Time: 1/16/2020 12:40:14 PM)"=15863, "Automatic Update (DT: Olivine-3-1; HV: 2.2; Time: 1/16/2020 12:40:15 PM)"=15864, "Automatic Update (DT: Olivine-3-1; HV: 2.2; Time: 1/16/2020 12:40:16 PM)"=15865, "Automatic Update (DT: Olivine-3-1; HV: 2.2; Time: 1/16/2020 12:40:17 PM)"=15866, "Automatic Update (DT: Olivine-3-1; HV: 2.2; Time: 1/16/2020 12:40:18 PM)"=15867, "Automatic Update (DT: Olivine-3-1; HV: 2.2; Time: 1/16/2020 12:40:25 PM)"=15868, "Automatic Update (DT: Olivine-3-1; HV: 2.2; Time: 1/16/2020 12:40:26 PM)"=15869, "Automatic Update (DT: Olivine-3-1; HV: 2.2; Time: 1/16/2020 12:40:27 PM)"=15870, "Automatic Update (DT: Olivine-3-1; HV: 2.2; Time: 1/16/2020 12:40:31 PM)"=15871, "Automatic Update (DT: Olivine-3-1; HV: 2.2; Time: 1/16/2020 12:40:32 PM)"=15872, "Automatic Update (DT: Olivine-3-1; HV: 2.2; Time: 1/16/2020 12:40:33 PM)"=15873, "Automatic Update (DT: Olivine-3-1; HV: 2.2; Time: 1/16/2020 12:40:34 PM)"=15874, "Automatic Update (DT: Olivine-3-1; HV: 2.2; Time: 1/16/2020 12:40:35 PM)"=15875, "Automatic Update (DT: Olivine-3-1; HV: 2.2; Time: 1/16/2020 12:41:40 PM)"=15876, "Automatic Update (DT: Olivine-3-1; HV: 2.2; Time: 1/16/2020 1:21:38 PM)"=15877, "Automatic Update (DT: Olivine-3-1; HV: 2.2; Time: 1/16/2020 1:21:42 PM)"=15878, "Automatic Update (DT: Olivine-3-1; HV: 2.2; Time: 1/16/2020 1:21:43 PM)"=15879, "Automatic Update (DT: Olivine-3-1; HV: 2.2; Time: 1/16/2020 1:21:44 PM)"=15880, "Automatic Update (DT: Olivine-3-1; HV: 2.2; Time: 1/16/2020 1:21:45 PM)"=15881, "Automatic Update (DT: Olivine-3-1; HV: 2.2; Time: 1/16/2020 1:21:46 PM)"=15882, "Automatic Update (DT: Olivine-3-1; HV: 2.2; Time: 1/16/2020 1:21:47 PM)"=15883, "Automatic Update (DT: Olivine-3-1; HV: 2.2; Time: 1/16/2020 1:21:52 PM)"=15884, "Automatic Update (DT: Olivine-3-1; HV: 2.2; Time: 1/16/2020 1:21:55 PM)"=15885, "Automatic Update (DT: Olivine-3-1; HV: 2.2; Time: 1/16/2020 1:21:56 PM)"=15886, "Automatic Update (DT: Olivine-3-1; HV: 2.2; Time: 1/16/2020 1:21:57 PM)"=15887, "Automatic Update (DT: Olivine-3-1; HV: 2.2; Time: 1/16/2020 1:22:01 PM)"=15888, "Automatic Update (DT: Olivine-3-1; HV: 2.2; Time: 1/16/2020 1:22:02 PM)"=15889, "Automatic Update (DT: Olivine-3-1; HV: 2.2; Time: 1/16/2020 1:22:03 PM)"=15890, "Automatic Update (DT: Olivine-3-1; HV: 2.2; Time: 1/16/2020 1:22:04 PM)"=15891, "Automatic Update (DT: Olivine-3-1; HV: 2.2; Time: 1/16/2020 1:22:05 PM)"=15892, "Automatic Update (DT: Olivine-3-1; HV: 2.2; Time: 1/16/2020 1:22:06 PM)"=15893, "Automatic Update (DT: Olivine-3-1; HV: 2.2; Time: 1/16/2020 1:22:10 PM)"=15894, "Automatic Update (DT: Olivine-3-1; HV: 2.2; Time: 1/16/2020 1:23:27 PM)"=15895, "Automatic Update (DT: Olivine-3-1; HV: 2.2; Time: 1/16/2020 1:23:28 PM)"=15896, "Automatic Update (DT: Olivine-3-1; HV: 2.2; Time: 1/16/2020 1:23:29 PM)"=15897, "Automatic Update (DT: Olivine-3-1; HV: 2.2; Time: 1/16/2020 1:23:30 PM)"=15898, "Automatic Update (DT: Olivine-3-1; HV: 2.2; Time: 1/16/2020 1:23:31 PM)"=15899, "Automatic Update (DT: Olivine-3-1; HV: 2.2; Time: 1/16/2020 1:23:35 PM)"=15900, "Automatic Update (DT: Olivine-3-1; HV: 2.2; Time: 1/16/2020 1:23:36 PM)"=15901, "Automatic Update (DT: Olivine-3-1; HV: 2.2; Time: 1/16/2020 1:23:37 PM)"=15902, "Automatic Update (DT: Olivine-3-1; HV: 2.2; Time: 1/16/2020 1:23:38 PM)"=15903, "Automatic Update (DT: Olivine-3-1; HV: 2.2; Time: 1/16/2020 1:23:39 PM)"=15904, "Automatic Update (DT: Olivine-3-1; HV: 2.2; Time: 1/16/2020 1:23:40 PM)"=15905, "Automatic Update (DT: Olivine-3-1; HV: 2.2; Time: 1/16/2020 1:23:45 PM)"=15906, "Automatic Update (DT: Olivine-3-1; HV: 2.2; Time: 1/16/2020 1:25:03 PM)"=15907]
  in  "Lower Timestamp Range":timestamp
  in  "Upper Timestamp Range":timestamp
  in  "Einzel Voltage":dbl
  in  "Needle Voltage":dbl
  in  "Frequency":dbl
  in  "Width (ms) : 0.1":dbl
  in  "Desired Amplitude (V)":dbl
  in  "X Voltage":dbl
  in  "Y Voltage":dbl
  out "Settings to be loaded":string
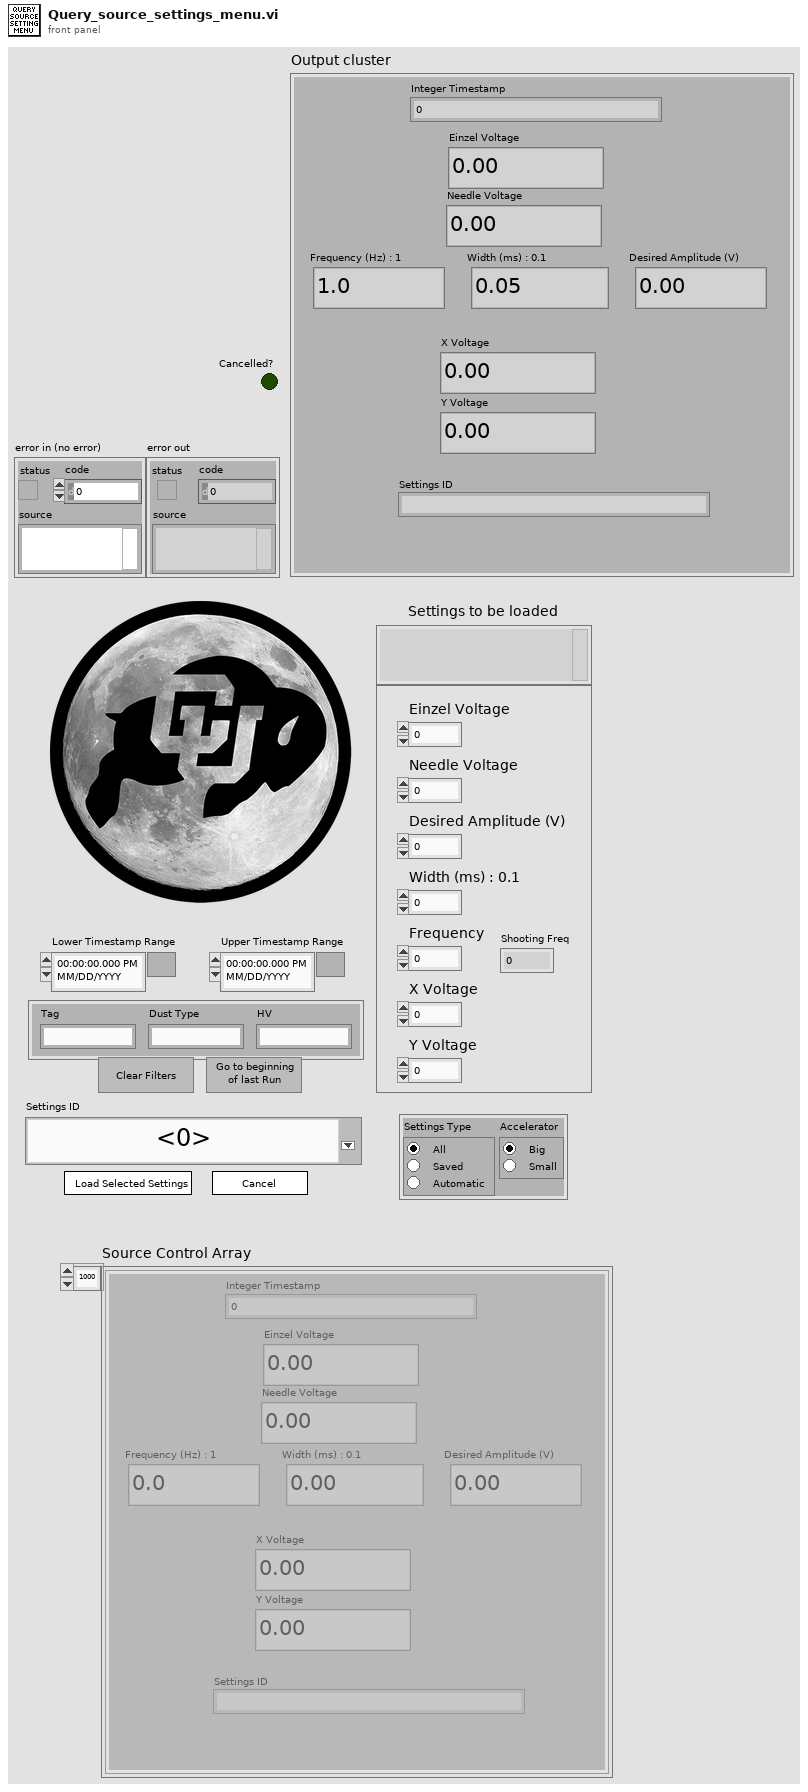
[diagram p1: front panel]
types:
  T1 = typedef "dust_source_control.ctl" = cluster{"Integer Timestamp":u64, "Einzel Voltage":dbl, "Needle Voltage":dbl, "Frequency":dbl, "Width (ms) : 0.1 ":dbl, "Desired Amplitude (V)":dbl, "X Voltage":dbl, "Y Voltage":dbl, "Settings ID":string, "ID#":i32}
  T2 = typedef "Source_settings_select.ctl" = cluster{"Settings Type":enum32{"All", "Saved", "Automatic"}, "Accelerator":enum32{"Big", "Small"}}
  T3 = cluster{"Tag":string, "Dust Type":string, "HV":string}
  T4 = typedef "LVPointTypeDef.ctl" = cluster{"Horizontal":i16, "Vertical":i16}
  T5 = enum8{"Enabled", "Disabled", "Disabled and Grayed Out"}
  T6 = typedef "dust_soruce_control.ctl" = cluster{"Integer Timestamp":u64, "Einzel Voltage":dbl, "Needle Voltage":dbl, "Frequency":dbl, "Width (ms) : 0.1 ":dbl, "Desired Amplitude (V)":dbl, "X Voltage":dbl, "Y Voltage":dbl, "Settings ID":string, "ID#":i32}
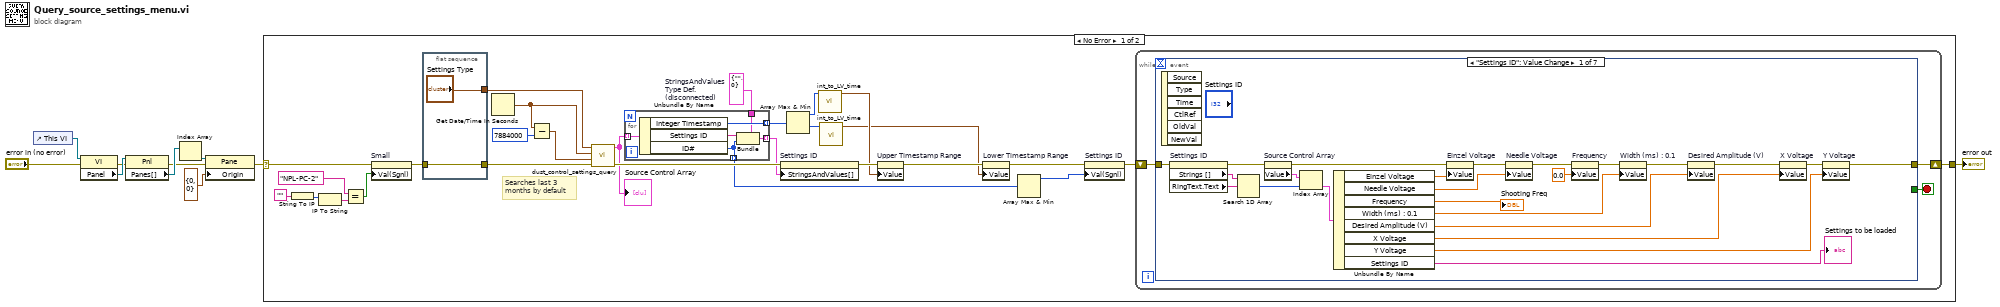
[diagram p0: block diagram]
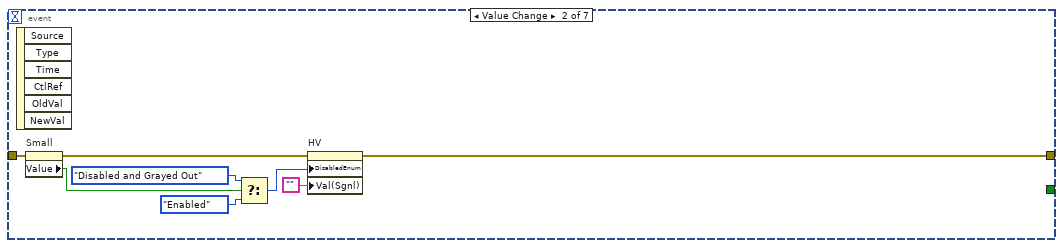
[diagram p2: hidden frame]
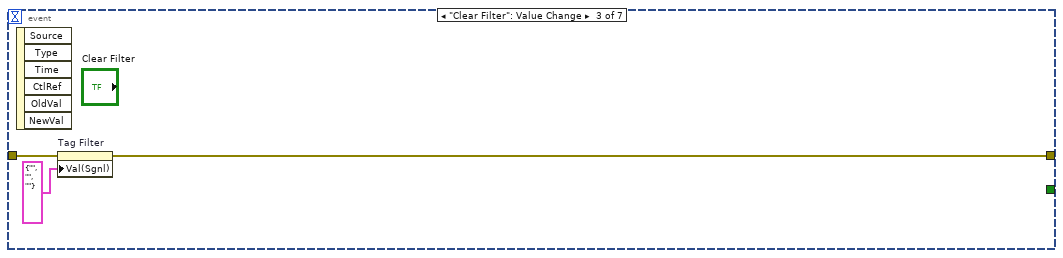
[diagram p3: hidden frame]
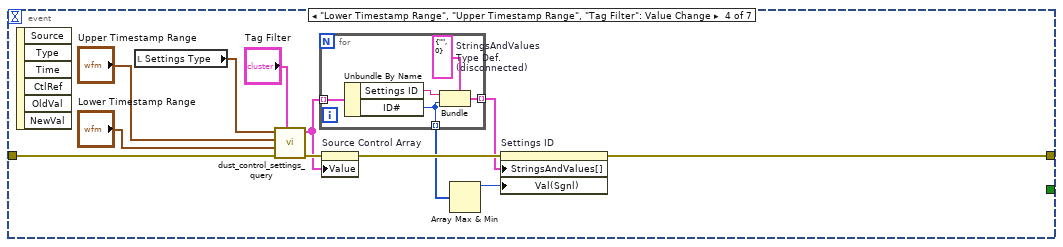
[diagram p4: hidden frame]
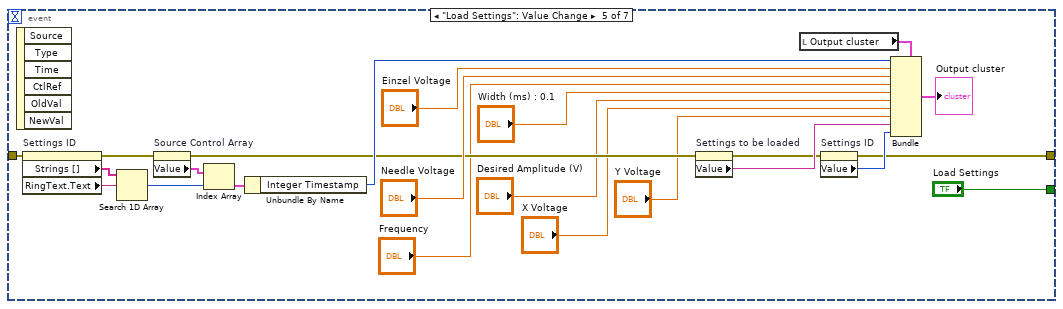
[diagram p5: hidden frame]
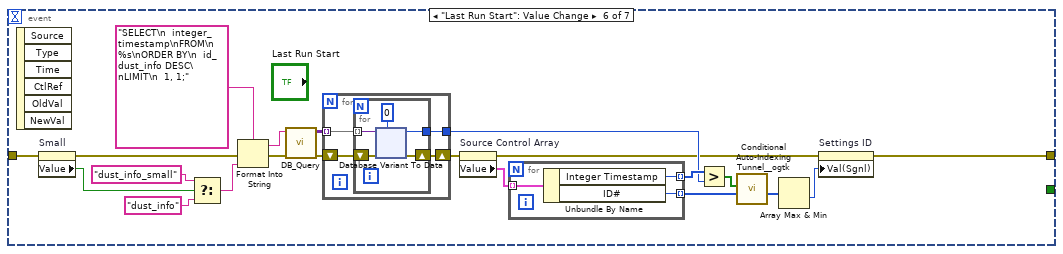
[diagram p6: hidden frame]
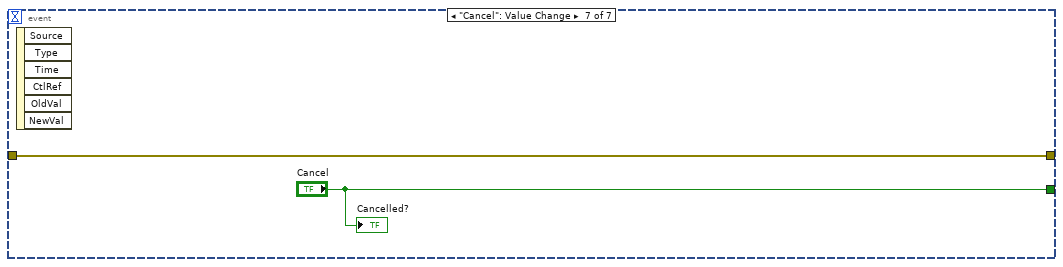
[diagram p7: hidden frame]
diagram:
  n1 = control-ref of="This VI"() -> (w3:refnum<vi>)
  n2 = property class="VI"(reference=w3, error in="error in (no error)") -> (error out=w4:errorcluster, "Panel"=w5:refnum<vi>)  [unwired: 1 out]
  n3 = property class="Pnl"(reference=w5, error in=w4) -> (error out=w6:errorcluster, "Panes[]"=w7:refnum<vi>[])  [unwired: 1 out]
  n4 = Index Array(array=w7) -> (element=w8:refnum<vi>)  [unwired: 1 in]
  n5 = property class="Pane"(reference=w8, error in=w6, "Origin"=T4 {"Horizontal"=0, "Vertical"=0}) -> (error out=w1:errorcluster)  [unwired: 1 out]
  n6 = case shown="No Error" w1 {
    selector: w1 -> [w14 w192]
    tunnel: [w22 w192] -> w10
    frame No Error {
      w36 = cluster{"String":string, "Value":i32} {"String"="", "Value"=0}  # StringsAndValues Type Def. (disconnected)
      # "Searches last 3\nmonths by default"
      n7 = String To IP(1:"") -> (0:w20:u32)
      n8 = IP To String(2:w20) -> (0:w19:string)  [unwired: 1 in]
      n9 = Equal?(x="NPL-PC-2", y=w19) -> (x = y?=w17:bool)
      n10 = property on="Small" class="Bool (strict)"(error in=w14, "Val(Sgnl)"=w17) -> (error out=w15:errorcluster)  [unwired: 1 in, 1 out]
      n11 = flat-sequence {
        tunnel: ["Settings Type"] -> w27
        tunnel: [w39] -> w16
        tunnel: w15 -> [w39]
        frame #0 {
        }
      }
      n12 = Get Date/Time In Seconds() -> (seconds since 1Jan1904=w13:timestamp)
      n13 = Subtract(x=w13, y=7884000) -> (x-y=w11:timestamp)
      n14 = call "dust_control_settings_query.vi"("error in (no error)"=w16, "Lower Timestamp Range"=w11, "Upper Timestamp Range"=w13, "Settings Type"=w27) -> ("error out"=w37:errorcluster, "Source Control Array"=w28:T1[])  [unwired: 6 in]
      "Source Control Array" <- w28
      n15 = for {
        tunnel: w28 -> [w191] mode=indexing
        tunnel: [w190] -> w38 mode=indexing
        tunnel: w36 -> [w189]
        tunnel: [w187] -> w35 mode=indexing
        tunnel: [w186] -> w24 mode=indexing
        n16 = Unbundle By Name(w191) -> ("Integer Timestamp"=w190:u64, "Settings ID"=w188:string, "ID#"=w186:i32)
        n17 = Bundle(cluster=w189, "String"=w188, "Value"=w186) -> (w187:cluster{"String":string, "Value":i32})
      }
      n18 = property on="Settings ID" class="Ring (strict)"(error in=w37, "StringsAndValues[]"=w35) -> (error out=w32:errorcluster)  [unwired: 1 in, 1 out]
      n19 = Array Max & Min(array=w38) -> (max value=w34:u64, min value=w33:u64)  [unwired: 2 out]
      n20 = call "int_to_LV_time.vi"("Integer Timestamp"=w34) -> ("time stamp"=w31:timestamp)  [unwired: 8 in, 1 out]
      n21 = call "int_to_LV_time.vi"("Integer Timestamp"=w33) -> ("time stamp"=w29:timestamp)  [unwired: 8 in, 1 out]
      n22 = property on="Upper Timestamp Range" class="AbsTime (strict)"(error in=w32, "Value"=w31) -> (error out=w30:errorcluster)  [unwired: 1 in, 1 out]
      n23 = property on="Lower Timestamp Range" class="AbsTime (strict)"(error in=w30, "Value"=w29) -> (error out=w26:errorcluster)  [unwired: 1 in, 1 out]
      n24 = Array Max & Min(array=w24) -> (max value=w23:i32)  [unwired: 3 out]
      n25 = property on="Settings ID" class="Ring (strict)"(error in=w26, "Val(Sgnl)"=w23) -> (error out=w25:errorcluster)  [unwired: 1 in, 1 out]
      n26 = while {
        shift-right: [w43] -> w22
        shift-left: w25 -> [w42]
        stop <- w41 stop-if-true
        n27 = event shown="[0] \"Settings ID\": Value Change" {
          selector: _ -> [_ _ _ _ _ _ _]
          dyn-events: _ -> [_ _ _ _ _ _ _]
          timeout: _ -> [_ _ _ _ _ _ _]
          tunnel: [w47 w69 w76 w81 w115 w132 w185] -> w43
          tunnel: w42 -> [w67 w75 w78 w90 w113 w131 w185]
          tunnel: [_ _ _ _ "Load Settings" _ "Cancel"] -> w41
          event "Settings ID": Value Change {
            n28 = event-data() -> ()  [unwired: 1 in, 6 out]
            n29 = property on="Settings ID" class="Ring (strict)"(error in=w67) -> (error out=w62:errorcluster, "Strings []"=w63:string[], "RingText.Text"=w66:string)  [unwired: 1 in, 1 out]
            n30 = Search 1D Array(1D array=w63, element=w66) -> (index of element=w64:i32)  [unwired: 1 in]
            n31 = property on="Source Control Array" class="Arr (strict)"(error in=w62) -> (error out=w60:errorcluster, "Value"=w65:T6[])  [unwired: 1 in, 1 out]
            n32 = Index Array(array=w65, index=w64) -> (element=w61:T6)
            n33 = Unbundle By Name(w61) -> ("Einzel Voltage"=w59:dbl, "Needle Voltage"=w58:dbl, "Frequency"=→"Shooting Freq":dbl, "Width (ms) : 0.1"=w57:dbl, "Desired Amplitude (V)"=w56:dbl, "X Voltage"=w55:dbl, "Y Voltage"=w54:dbl, "Settings ID"=→"Settings to be loaded":string)
            n34 = property on="Einzel Voltage" class="DigNum (strict)"(error in=w60, "Value"=w59) -> (error out=w53:errorcluster)  [unwired: 1 in, 1 out]
            n35 = property on="Needle Voltage" class="DigNum (strict)"(error in=w53, "Value"=w58) -> (error out=w52:errorcluster)  [unwired: 1 in, 1 out]
            n36 = property on="Frequency" class="DigNum (strict)"(error in=w52, "Value"=0.0 ("Frequency")) -> (error out=w51:errorcluster)  [unwired: 1 in, 1 out]
            n37 = property on="Width (ms) : 0.1" class="DigNum (strict)"(error in=w51, "Value"=w57) -> (error out=w50:errorcluster)  [unwired: 1 in, 1 out]
            n38 = property on="Desired Amplitude (V)" class="DigNum (strict)"(error in=w50, "Value"=w56) -> (error out=w49:errorcluster)  [unwired: 1 in, 1 out]
            n39 = property on="X Voltage" class="DigNum (strict)"(error in=w49, "Value"=w55) -> (error out=w48:errorcluster)  [unwired: 1 in, 1 out]
            n40 = property on="Y Voltage" class="DigNum (strict)"(error in=w48, "Value"=w54) -> (error out=w47:errorcluster)  [unwired: 1 in, 1 out]
          }
          event Value Change {
            n41 = event-data() -> ()  [unwired: 1 in, 6 out]
            n42 = property on="Small" class="Bool (strict)"(error in=w75) -> (error out=w74:errorcluster, "Value"=w70:bool)  [unwired: 1 in, 1 out]
            n43 = Select(t=T5."Disabled and Grayed Out" ("Disabled"), s=w70, f=T5."Enabled" ("Disabled")) -> (s? t:f=w72:T5)
            n44 = property on="HV" class="Str"(error in=w74, "DisabledEnum"=w72, "Val(Sgnl)"="" ("Value (Signaling)")) -> (error out=w69:errorcluster)  [unwired: 1 in, 1 out]
          }
          event "Clear Filter": Value Change {
            n45 = event-data() -> ()  [unwired: 1 in, 6 out]
            n46 = property on="Tag Filter" class="Clust (strict)"(error in=w78, "Val(Sgnl)"=T3 {"Tag"="", "Dust Type"="", "HV"=""} ("Value (Signaling)")) -> (error out=w76:errorcluster)  [unwired: 1 in, 1 out]
          }
          event "Lower Timestamp Range", "Upper Timestamp Range", "Tag Filter": Value Change {
            n47 = event-data() -> ()  [unwired: 1 in, 6 out]
            n48 = local read "Settings Type"() -> (w89:T2)
            n49 = call "dust_control_settings_query.vi"("Query Cluster"="Tag Filter", "error in (no error)"=w90, "Lower Timestamp Range"="Lower Timestamp Range", "Upper Timestamp Range"="Upper Timestamp Range", "Settings Type"=w89) -> ("error out"=w85:errorcluster, "Source Control Array"=w84:T1[])  [unwired: 5 in]
            n50 = for {
              tunnel: w84 -> [w95] mode=indexing
              tunnel: [w92] -> w82 mode=indexing
              tunnel: [w91] -> w80 mode=indexing
              w93 = cluster{"String":string, "Value":i32} {"String"="", "Value"=0}  # StringsAndValues Type Def. (disconnected)
              n51 = Unbundle By Name(w95) -> ("Settings ID"=w94:string, "ID#"=w91:i32)
              n52 = Bundle(cluster=w93, "String"=w94, "Value"=w91) -> (w92:cluster{"String":string, "Value":i32})
            }
            n53 = property on="Source Control Array" class="Arr (strict)"(error in=w85, "Value"=w84) -> (error out=w83:errorcluster)  [unwired: 1 in, 1 out]
            n54 = Array Max & Min(array=w80) -> (max value=w79:i32)  [unwired: 3 out]
            n55 = property on="Settings ID" class="Ring (strict)"(error in=w83, "StringsAndValues[]"=w82, "Val(Sgnl)"=w79) -> (error out=w81:errorcluster)  [unwired: 1 in, 1 out]
          }
          event "Load Settings": Value Change {
            n56 = event-data() -> ()  [unwired: 1 in, 6 out]
            n57 = property on="Settings ID" class="Ring (strict)"(error in=w113) -> (error out=w110:errorcluster, "Strings []"=w112:string[], "RingText.Text"=w111:string)  [unwired: 1 in, 1 out]
            n58 = Search 1D Array(1D array=w112, element=w111) -> (index of element=w109:i32)  [unwired: 1 in]
            n59 = property on="Source Control Array" class="Arr (strict)"(error in=w110) -> (error out=w101:errorcluster, "Value"=w108:T6[])  [unwired: 1 in, 1 out]
            n60 = Index Array(array=w108, index=w109) -> (element=w107:T6)
            n61 = Unbundle By Name(w107) -> ("Integer Timestamp"=w106:u64)
            n62 = property on="Settings to be loaded" class="Str"(error in=w101) -> (error out=w104:errorcluster, "Value"=w105:string)  [unwired: 1 in, 1 out]
            n63 = local read "Output cluster"() -> (w117:T1)
            n64 = property on="Settings ID" class="Ring (strict)"(error in=w104) -> (error out=w115:errorcluster, "Value"=w116:i32)  [unwired: 1 in, 1 out]
            n65 = Bundle(cluster=w117, "Integer Timestamp"=w106, "Einzel Voltage"="Einzel Voltage", "Needle Voltage"="Needle Voltage", "Frequency"="Frequency", "Width (ms) : 0.1"="Width (ms) : 0.1", "Desired Amplitude (V)"="Desired Amplitude (V)", "X Voltage"="X Voltage", "Y Voltage"="Y Voltage", "Settings ID"=w105, "ID#"=w116) -> (→"Output cluster":T1)
          }
          event "Last Run Start": Value Change {
            n66 = event-data() -> ()  [unwired: 1 in, 6 out]
            n67 = property on="Small" class="Bool (strict)"(error in=w131) -> (error out=w129:errorcluster, "Value"=w126:bool)  [unwired: 1 in, 1 out]
            n68 = Select(t="dust_info_small" ("input 1"), s=w126, f="dust_info" ("input 1")) -> (s? t:f=w125:string)
            n69 = Format Into String(format string="SELECT\n  integer_timestamp\nFROM\n  %s\nORDER BY\n  id_dust_info DESC\nLIMIT\n  1, 1;" ("Parameterized Query"), error in=w129, w125) -> (resulting string=w123:string, error out=w124:errorcluster)  [unwired: 1 in]
            n70 = call "DB_Query.vi"("error in (no error)"=w124, "Parameterized Query"=w123) -> ("error out"=w139:errorcluster, "Results"=w138:variant[][])  [unwired: 7 in, 1 out]
            n71 = for {
              shift-right: [w145] -> w137
              shift-left: w139 -> [w146]
              tunnel: w138 -> [w144] mode=indexing
              tunnel: [w143] -> w134
              n72 = for {
                shift-right: [w150] -> w145
                shift-left: w146 -> [w151]
                tunnel: w144 -> [w149] mode=indexing
                tunnel: [w148] -> w143
                n73 = xnode "Database Variant To Data"("database variant"=w149, "error in (no error)"=w151, "type"=i64 0) -> ("data"=w148:i64, "error out"=w150:errorcluster)
              }
            }
            n74 = property on="Source Control Array" class="Arr (strict)"(error in=w137) -> (error out=w120:errorcluster, "Value"=w136:T6[])  [unwired: 1 in, 1 out]
            n75 = for {
              tunnel: w136 -> [w142] mode=indexing
              tunnel: [w141] -> w135 mode=indexing
              tunnel: [w140] -> w121 mode=indexing
              n76 = Unbundle By Name(w142) -> ("Integer Timestamp"=w141:u64, "ID#"=w140:i32)
            }
            n77 = Greater?(x=w135, y=w134) -> (0:w122:bool[])
            n78 = call-poly <userlib>:"Conditional Auto-Indexing Tunnel__ogtk.vi"("Array in"=w121, "Elements to keep"=w122) -> ("Filtered Array out"=w133:i32[])  [unwired: 5 in]
            n79 = Array Max & Min(array=w133) -> (min value=w119:i32)  [unwired: 3 out]
            n80 = property on="Settings ID" class="Ring (strict)"(error in=w120, "Val(Sgnl)"=w119) -> (error out=w132:errorcluster)  [unwired: 1 in, 1 out]
          }
          event "Cancel": Value Change {
            n81 = event-data() -> ()  [unwired: 1 in, 6 out]
            "Cancelled?" <- "Cancel"
          }
        }
      }
    }
    frame Error {
    }
  }
  "error out" <- w10
